vi "LS Durability Main (RT).vi"() -> ()   [LabVIEW 2018]
uses:
  Type Defs/App Config.ctl
  Type Defs/Controller Names.ctl
  SubVIs/Data Logger/Data Log Init.ctl
  Controls/Alarm Config.ctl
  Controls/Alarm Definition.ctl
  Controls/Alarm Profile Config.ctl
  Type Defs/Controller List.ctl
  Controls/Tank CMDs.ctl
  Controls/Controller Config.ctl
  Controls/Pump Data.ctl
  Controls/Tank Data.ctl
  Controls/HMI Cluster.ctl
  Controls/HMI Header.ctl
  Controls/HMI Tog Buttons.ctl
  Controls/HMI Mom Buttons.ctl
  Type Defs/LS Data.ctl
  Type Defs/Sequence States.ctl
  Controls/App Global Mode.ctl
  Controls/RPi HMI Mode.ctl
  Controls/Email Mode.ctl
  Type Defs/Pump Data Mode.ctl
  SubVIs/Watlow Modbus/Modbus Mode.ctl
  SubVIs/Watlow Modbus/Modbus Variable.ctl
  Controls/HMI Global Mode.ctl
  <vilib>/FPGAPlugInAG/sbRIO-9627/niLvFpga_Open_sbRIO-9627.vi
  <vilib>/Utility/error.llb/Error Cluster From Error Code.vi
  <vilib>/rvi/errors/niLvFpgaAdjustHostInterfaceError.vi
  <vilib>/Utility/file.llb/Write To Spreadsheet File (string).vi
  <vilib>/rvi/interface/nirviOpenFPGA/nirviOpenFPGA.xnode
  Controls/FPGA_Reference.ctl
  FPGA Bitfiles/LS_Durability_FPGA_9627.lvbitx
  <vilib>/rvi/interface/nirviReadWriteControl/nirviReadWriteControl.xnode
  <vilib>/Utility/config.llb/NI_LVConfig.lvlib
  Controls/Power Supply Global Mode.ctl
  SubVIs/Data Logger/Data Logger Mode.ctl
  SubVIs/Data Logger/Data Log Start.ctl
  NiFpgaLv.dll
  <vilib>/rvi/errors/niLvFpgaMergeErrorWithErrorCode.vi
panel:
  in  "pb.Run Profile":bool
  in  "Bank 2":T1={"7"=TRUE, "8"=TRUE, "9"=TRUE, "10"=TRUE, "11"=TRUE, "11 2"=TRUE}
  in  "Bank 1":T2={"1"=TRUE, "2"=TRUE, "3"=TRUE, "4"=TRUE, "5"=TRUE, "5 2"=TRUE} caption="Present"
  out "Email Alarms Disabled":bool
  out "Recording":bool
  in  "Disable Alarm Email":bool
  in  "Temp Tolerance":dbl=3.0 min=0.0 max=999999.0 step=1.0
  in  "Thermocouple":enum16{"2 TC/2 Tanks", "1 TC/1 Tank"}(ring)
  out "ADC Errors":i32
  in  "pb.Tare Pressure":bool
  in  "Data Log Enabled":bool=TRUE
  in  "RPMhyst":fxp<+,25,6>=1.0
  in  "pb.FuelChange":bool
  in  "Controller Type:":T3
  in  "Target Pressure:":dbl
  in  "Target Voltage:":dbl
  in  "Tank 1 Fuel Type:":string
  in  "Tank 2 Fuel Type:":string
  in  "Stagger Time (ms):":i32
  out "Cycles Completed:":u32=17
  in  "pb.Cycle Reset":bool
  in  "Serial Numbers":T4
  out "Read Inputs (ms)":u32
  out "Update Screen (ms)":u32
  out "Run Step (ms)":u32
  in  "Fuel Change Tab":enum32{"Page 1", "Page 2"}(tab)
  in  "pb.Fuel Change OK":bool
  in  "Reset Tab":enum32{"Page 1", "Page 2"}(tab)
  in  "pb.Reset OK":bool
  in  "pb.Reset Cancel":bool
  in  "Save As Tab":enum32{"Page 1", "Page 2"}(tab)
  in  "New Profile Name:":string
  in  "pb.Save As OK":bool
  in  "pb.Save As Cancel":bool
  in  "Alarm Tab":enum32{"Page 1", "Page 2"}(tab)
  out "Alarm Message":string
  in  "pb.Alarm OK":bool
  in  "Set Time Tab":enum32{"Page 1", "Page 2"}(tab)
  in  "pb.Set Time OK":bool
  in  "pb.Set Time Cancel":bool
  in  "New Time":dbl format="%<%H:%M:%S>t"
  in  "Pump Timers Tab":enum32{"Page 1", "Page 2"}(tab)=enum."Page 2"
  in  "Stop Time Enable":bool
  in  "Stop Time:":dbl format="%<%H:%M:%S>t"
  in  "pb.Time Reset All":bool
  out "Elapsed Time:":dbl[](array[numeric]) format="%<%H:%M:%S>t"
  in  "pb.Resets":bool[](array[boolean])=[FALSE, FALSE, FALSE, FALSE, FALSE, FALSE]
  in  "pb.Sets":bool[](array[boolean])=[FALSE, FALSE, FALSE, FALSE, FALSE, FALSE]
  in  "LS Serial Numbers":T5 caption="Serial Numbers"
  out "CPU Usage:":dbl=7.74131899555212 format="%.1f"
  in  "Live Data Tab":enum32{"Page 1", "Page 2", "Page 3"}(tab)=enum."Page 2"
  in  "Controller\nCMD":dbl[](array[numeric])=[0.0, 0.0, 0.0, 0.0, 0.0, 0.0] format="%#.2f"
  out "Speed":dbl[](array[numeric]) caption="Speed\n(RPM)" format="%#.0f"
  out "ControllerCurrent":dbl[](array[numeric])=[0.015201568603515625, 0.00335693359375, 0.003021240234375, 0.12260055541992188, 0.06085968017578125, 0.052234649658203125] caption="Controller\nCurrent\n(DC)" format="%.1f"
  out "PumpCurrent":dbl[](array[numeric])=[0.015201568603515625, 0.00335693359375, 0.003021240234375, 0.12260055541992188, 0.06085968017578125, 0.052234649658203125] caption="Pump\nCurrent\n(RMS)" format="%.1f"
  out "Flow":dbl[](array[numeric])=[0.0, 0.0, 0.0, 0.125, 0.0625, 0.0625] caption="Flow\n(L/H)" format="%#.0f"
  out "Pressure":dbl[](array[numeric])=[0.015201568603515625, 0.00335693359375, 0.003021240234375, 0.12260055541992188, 0.06085968017578125, 0.052234649658203125] caption="Pressure\n(kPa)" format="%#.0f"
  out "Ave. Speed":dbl=7.74131899555212 format="%.1f"
  out "Voltages":dbl[](array[numeric])=[0.015201568603515625, 0.00335693359375, 0.003021240234375, 0.12260055541992188, 0.06085968017578125, 0.052234649658203125] caption="Pump\nVoltage\n(V)" format="%.1f"
  in  "Reset Anomalies":bool
  in  "Reset Total Cycles":bool
  out "Anomalies (Last Cycle)":i32[](array[numeric]) caption="Anomalies\n(Last Cycle)" format="%#.0f"
  out "Anomalies/Cycle":i32[](array[numeric]) caption="Anomalies/\nCycle" format="%#.0f"
  out "Cycles":u32[](array[numeric]) caption="Powered\nCycles" format="%#.0f"
  out "Anomalies Total":i32[](array[numeric]) caption="Anomalies\nTotal" format="%#.0f"
  out "Steps":u32[](array[numeric]) format="%#.0f"
  out "Total Cycles":u32[](array[numeric]) caption="Total\nPowered\nCycles" format="%#.0f"
  in  "Reset Opens":bool
  out "Opens":i32[](array[numeric]) format="%#.0f"
  in  "App Config":T6={"Location"="Tanks 162-163", "Profiles Path"=path "c:/Profiles", "Current Profile"="", "CA Number"="", "Cycles Completed"=0, "Controller Type:"=enum."Kuhnke", "Stagger Time (ms)"=0, "Tank 1 Fuel"="", "Tank 2 Fuel"="", "Serial Numbers"={"Position 1 SN"="", "Position 2 SN"="", "Poaition 3 SN"="", "Position 4 SN"="", "Position 5 SN"="", "Position 6 SN"=""}, "Pumps Present"={"Pump 1"=FALSE, "Pump 2"=FALSE, "Pump 3"=FALSE, "Pump 4"=FALSE, "Pump 5"=FALSE, "Pump 6"=FALSE}, "VoltCtrlRef"="", "VoltageSelect"=FALSE, "Watlow Present"=TRUE, "Temp 1"=0.0, "Temp 2"=0.0, "V_Run PI?"=FALSE, "Voltage Limits"={"V_Step"=1e-05, "V_CmdMax"=0.0, "V_CmdMin"=0.0}, "Voltage Far PI"={"V_FarSlew"=10.0, "V_FarKp"=0.0, "V_FarKi"=0.0}, "Voltage Mid PI"={"V_MidSlew"=10.0, "V_MidKp"=0.0, "V_MidKi"=0.0}, "Voltage Close PI"={"V_CloseSlew"=10.0, "V_CloseKp"=0.0, "V_CloseKi"=0.0}, "Voltage Scale"={"V_FFm"=0.0, "V_FFb"=0.0}, "Voltage Cutoffs"={"V_MidCutoff"=0.0, "V_CloseCutoff"=0.0}, "Pressure Scale"={"Pres_FFm"=1e-05, "Pres_FFb"=0.0}, "Temp Format"=0, "Temp Tolerance"=0.0, "Target Voltage"=0.0, "Target Pressure"=0.0, "Data Log Init"={"Data Path"=path "u:/Data", "Data Log Rate (S/s)"=1, "AKLH Rate (Hours/S)"=0.1, "Sync Time Offset (min)"=180, "IP Last 3"=0, "WebDAV IP"="10.31.176.36"}, "Email Handler IP"="10.30.189.34", "ADC Check"=FALSE, "3 Pump Tank"=TRUE, "Cycle Threshold:"=3.0, "Cycle Pts to Avg:"=3, "Anomaly Threshold:"=3.0, "Normal Steps:"=3, "Step Threshold:"=3.0, "Network Drive IP"="", "Network Drive Password"="", "Bank 1 Offset"=0.0, "Bank 2 Offset"=0.0} {"Bank 2 Offset" min=0.0 max=999999.0 step=1.0; "Bank 1 Offset" min=0.0 max=999999.0 step=1.0; "Step Threshold:" min=0.0 max=999999.0 step=1.0; "Normal Steps:" max=999999 step=1; "Anomaly Threshold:" min=0.0 max=999999.0 step=1.0; "Cycle Pts to Avg:" max=999999 step=1; "Cycle Threshold:" min=0.0 max=999999.0 step=1.0}
  in  "Monitoring Tab":enum32{"Page 1", "Page 2"}(tab)
  out "Avg Press:":dbl=7.74131899555212
  in  "pb.E Stop":bool
  in  "Ignition Relay":T8
  in  "Power Relay":T8
  out "Temp2":dbl caption="Tank 2 Temp (C):" format="%.1f"
  out "Temp1":dbl caption="Tank 1 Temp (C):" format="%.1f"
  out "PS Actual (V):":dbl format="%.2f"
  in  "Power Supply Cmd:":dbl min=0.0 max=20.0 format="%#.2f"
  in  "PressureCMD":dbl caption="Pressure Cmd:" min=0.0 max=825.0 format="%#.2f"
  in  "Pumps Present":T8={"Pump 1"=TRUE, "Pump 2"=TRUE, "Pump 3"=TRUE, "Pump 4"=TRUE, "Pump 5"=TRUE, "Pump 6"=TRUE}
  in  "Tank 1 Temp Cmd:":dbl caption="deg C"
  in  "Tank 2 Temp Cmd:":dbl caption="deg C"
  in  "Title Tab":enum32{"Page 1", "Page 2"}(tab)
  out "Title":string="LS-12 Durability Tester, v2.0"
  out "Time/Date":string
  in  "Login":bool
  in  "pb.Stop Profile":bool
  in  "Main Tab":T9(tab)
  out "ARclock":i32 caption="Auto-resume\nClock"
  in  "ARtiming":i32=1800 caption="Auto-resume\nTime (s)"
  in  "pb.Pause/Resume":bool
  out "Transferring":bool
  in  "Recording\nFrequency (Hz): 2":i32=1000
  in  "Recording\nDuration (s): 2":i32=3600
  in  "Record Constant":bool
  in  "Detection Mode:":u16(ring) items=["Anomalies", "Opens"]
  in  "Record During Profile":bool
  in  "Recording\nFrequency (Hz):":i32=1000
  in  "Recording\nDuration (s):":i32=10
  in  "Interval Between\nRecordings (s):":i32=600
  in  "LS Cycle Time (ms):":dbl=244.0 min=0.1 max=1000.0 step=0.1
  in  "LS On Time (ms):":dbl=4.0 min=0.0 max=1000.0 step=0.01
  in  "Bank 2 Power State:":u16(ring) items=["0 - Off", "1 - On", "2 - Pulsing"]
  in  "Bank 1 Power State:":u16(ring) items=["0 - Off", "1 - On", "2 - Pulsing"]
  in  "CA Number:":string
  in  "Profile Name:":string(combo)="test"
  in  "pb.Save As":bool
  out "Location:":string
  in  "Profile:":string[][](table)=[["1", "216000", "1", "2", "244", "4", "1", "67.6"], ["2", "1800", "0", "0", "244", "4", "1", "10.0"], ["3", "39600", "0", "0", "244", "4", "0", ""], ["4", "1800", "0", "0", "244", "4", "1", ""]]
  out "Recording":bool
  in  "Data File Name:":string
  out "Step:":i32=2
  out "Time Left:":dbl=0.21101045608520508
  out "Waveform Chart":dbl(graph)
  in  "Pause":bool
  in  "Position":i32=1 min=1 max=13 step=1
  in  "Bank 2 Voltage Offset:":dbl
  in  "Bank 1 Voltage Offset:":dbl
  in  "Voltage(T)/Resistance(F)":bool=TRUE
  in  "Bias Resistances":dbl[](array[numeric])=[681.0, 681.0, 681.0, 681.0, 681.0, 681.0, 681.0, 681.0, 681.0, 681.0, 681.0, 681.0] caption="Total\nCycles"
  in  "Anomaly Threshold:":dbl=3.0 min=0.0 max=999999.0 step=1.0
  in  "Normal Steps:":u32=3 max=999999 step=1
  in  "Step Threshold:":dbl=3.0 min=0.0 max=999999.0 step=1.0
  in  "Cycle Pts to Avg:":i32=20 min=0 max=999999 step=1
  in  "Cycle Threshold:":dbl=1.6 min=0.0 max=999999.0 step=1.0
  in  "Note Tab":enum32{"Page 1", "Page 2"}(tab)
  in  "Stop Profile Note":string
  in  "pb.Note OK":bool
  in  "pb.Note Cancel":bool
  in  "Alarm Config":T10
  in  "WebDAV Push":bool
  in  "Concat Data":bool
  in  "Cutoffs":cluster{"Mid Range":dbl, "Close Range":dbl} {"Close Range" min=-100000.0 max=100000.0 step=1e-05 format="%#.5f"; "Mid Range" min=-100000.0 max=100000.0 step=1e-05 format="%#.5f"}
  in  "Mid PI":cluster{"Slew Rate":dbl, "Kp":dbl, "Ki":dbl}={"Slew Rate"=10.0, "Kp"=0.0, "Ki"=0.0} {"Ki" min=-100000.0 max=100000.0 step=1e-05 format="%#.5f"; "Kp" min=-100000.0 max=100000.0 step=1e-05 format="%#.5f"; "Slew Rate" min=0.0 max=1000000.0 step=0.01 format="%#.5f"}
  in  "Close PI":cluster{"Slew Rate":dbl, "Kp":dbl, "Ki":dbl}={"Slew Rate"=10.0, "Kp"=0.0, "Ki"=0.0} {"Ki" min=-100000.0 max=100000.0 step=1e-05 format="%#.5f"; "Kp" min=-100000.0 max=100000.0 step=1e-05 format="%#.5f"; "Slew Rate" min=0.0 max=1000000.0 step=0.01 format="%#.5f"}
  in  "Pressure Scale":cluster{"M":dbl, "B":dbl}={"M"=1e-05, "B"=0.0} {"B" min=-100000.0 max=100000.0 step=1e-05 format="%#.5f"; "M" min=-100000.0 max=100000.0 step=1e-05 format="%#.5f"}
  in  "Closed Loop Voltage":bool
  in  "Voltage Limits":cluster{"Step":dbl, "Max":dbl, "Min":dbl}={"Step"=1e-05, "Max"=0.0, "Min"=0.0} {"Min" min=0.0 max=10.0 step=1e-05 format="%#.5f"; "Max" min=0.0 max=10.0 step=1e-05 format="%#.5f"; "Step" min=0.0 max=100.0 step=1e-05 format="%#.5f"}
  in  "Far PI":cluster{"Slew Rate":dbl, "Kp":dbl, "Ki":dbl}={"Slew Rate"=10.0, "Kp"=0.0, "Ki"=0.0} {"Ki" min=-100000.0 max=100000.0 step=1e-05 format="%#.5f"; "Kp" min=-100000.0 max=100000.0 step=1e-05 format="%#.5f"; "Slew Rate" min=0.0 max=1000000.0 step=0.01 format="%#.5f"}
  in  "Voltage Scale":cluster{"M":dbl, "B":dbl} {"B" min=-100000.0 max=100000.0 step=1e-05 format="%#.5f"; "M" min=-100000.0 max=100000.0 step=1e-05 format="%#.5f"}
  # "Fuel Change was logged."
  # "Are you sure you want to reset?"
  # "Enter a new elapsed time."
  # "Pump Timers"
  # "Live Data"
  # "Level Sensor Monitor"
  # "Level Sensor Monitor"
  # "Manual Control"
  # "V"
  # "kPa"
  # "degC"
  # "degC"
  # "Data file note as to reason for stopping profile:"
  # "Voltage Control"
  # "Pressure Control"
  # "Data Server"
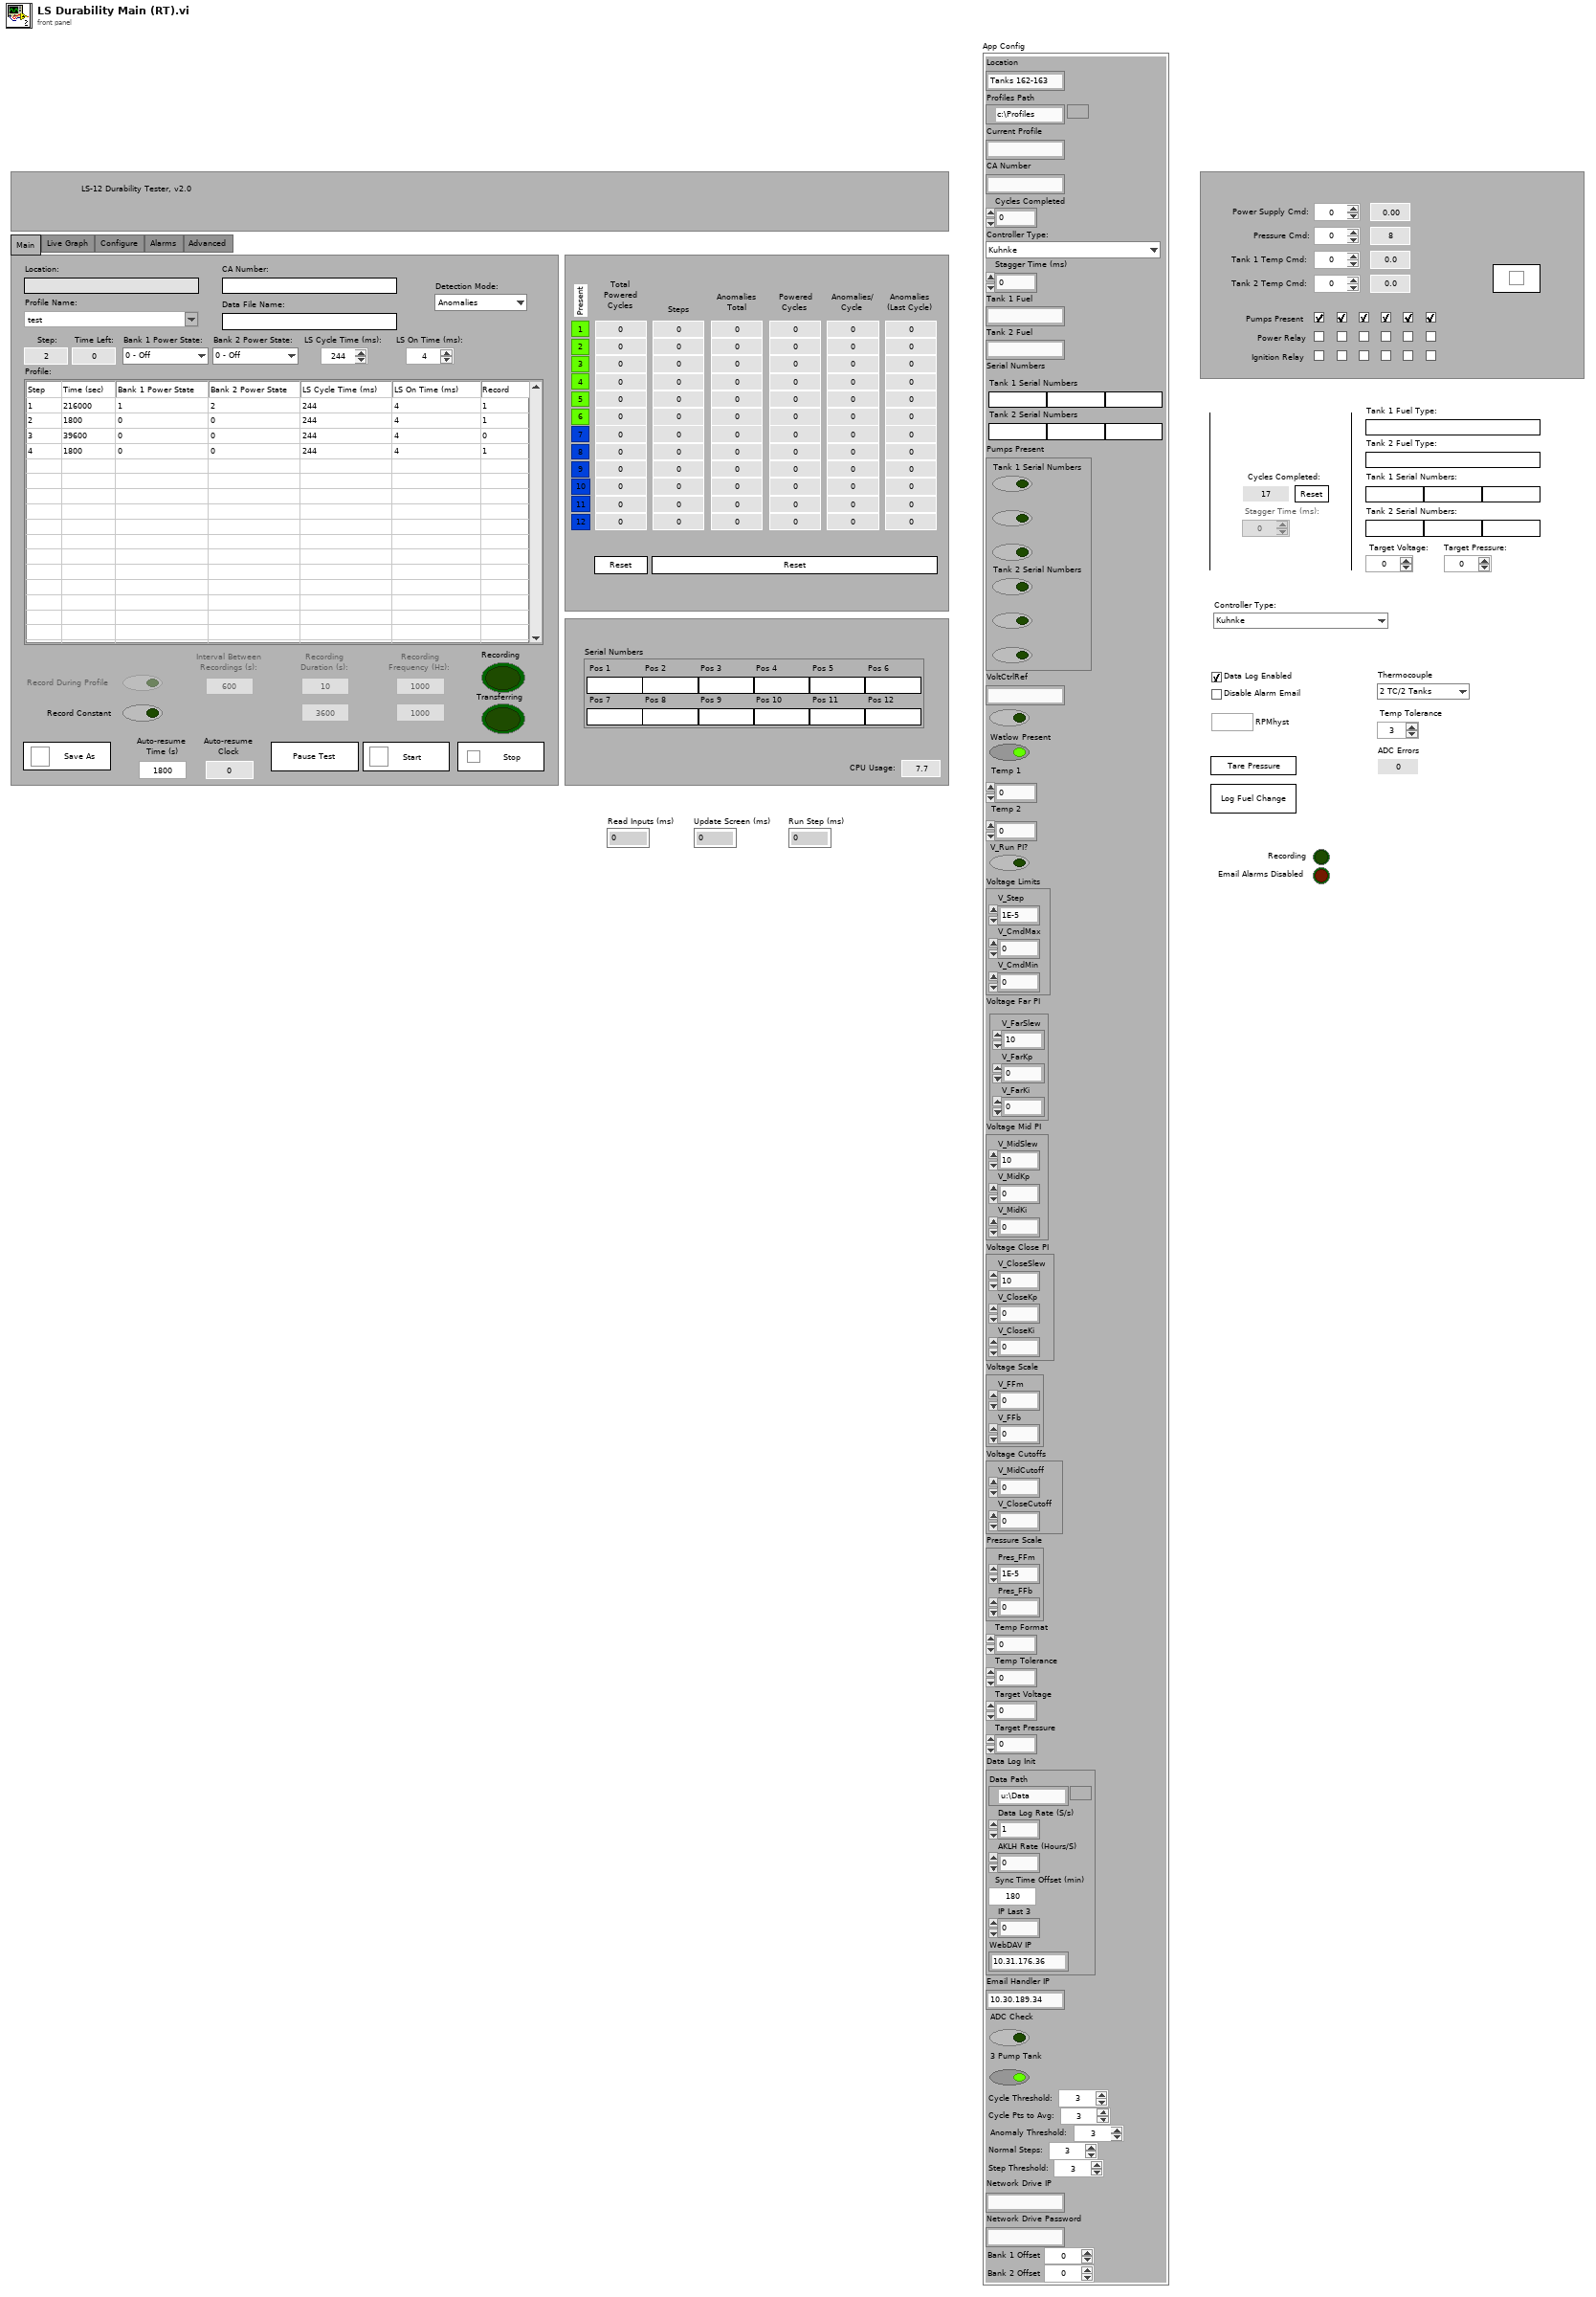
[diagram p1: front panel]
types:
  T1 = cluster{"7":bool, "8":bool, "9":bool, "10":bool, "11":bool, "11 2":bool}
  T2 = cluster{"1":bool, "2":bool, "3":bool, "4":bool, "5":bool, "5 2":bool}
  T3 = typedef "Controller Names.ctl" = enum16{"Kuhnke", "Helbako BLDC", "Conti", "Hella BLDC OL PWM", "Hella BLDC Turbine OL PWM", "Hella BLDC Pressure", "Helbako (old)", "TI PWM", "PSA", "Hella Gas", "Hella Diesel", "8 Comm", "10 Comm", "8 Comm Hella", "10 Comm Hella", "8 Comm Omron", "10 Comm Omron", "8 Comm Nissan", "10 Comm Nissan"}
  T4 = cluster{"Position 1 SN":string, "Position 2 SN":string, "Position 3 SN":string, "Position 4 SN":string, "Position 5 SN":string, "Position 6 SN":string}
  T5 = cluster{"Pos 1":string, "Pos 2":string, "Pos 3":string, "Pos 4":string, "Pos 5":string, "Pos 6":string, "Pos 7":string, "Pos 8":string, "Pos 9":string, "Pos 10":string, "Pos 11":string, "Pos 12":string}
  T6 = typedef "App Config.ctl" = cluster{"Location":string, "Profiles Path":path, "Current Profile":string, "CA Number":string, "Cycles Completed":u32, "Controller Type:":T3, "Stagger Time (ms)":i32, "Tank 1 Fuel":string, "Tank 2 Fuel":string, "Serial Numbers":cluster{"Position 1 SN":string, "Position 2 SN":string, "Poaition 3 SN":string, "Position 4 SN":string, "Position 5 SN":string, "Position 6 SN":string}, "Pumps Present":cluster{"Pump 1":bool, "Pump 2":bool, "Pump 3":bool, "Pump 4":bool, "Pump 5":bool, "Pump 6":bool}, "VoltCtrlRef":string, "VoltageSelect":bool, "Watlow Present":bool, "Temp 1":dbl, "Temp 2":dbl, "V_Run PI?":bool, "Voltage Limits":cluster{"V_Step":dbl, "V_CmdMax":dbl, "V_CmdMin":dbl}, "Voltage Far PI":cluster{"V_FarSlew":dbl, "V_FarKp":dbl, "V_FarKi":dbl}, "Voltage Mid PI":cluster{"V_MidSlew":dbl, "V_MidKp":dbl, "V_MidKi":dbl}, "Voltage Close PI":cluster{"V_CloseSlew":dbl, "V_CloseKp":dbl, "V_CloseKi":dbl}, "Voltage Scale":cluster{"V_FFm":dbl, "V_FFb":dbl}, "Voltage Cutoffs":cluster{"V_MidCutoff":dbl, "V_CloseCutoff":dbl}, "Pressure Scale":cluster{"Pres_FFm":dbl, "Pres_FFb":dbl}, "Temp Format":i32, "Temp Tolerance":dbl, "Target Voltage":dbl, "Target Pressure":dbl, "Data Log Init":T7, "Email Handler IP":string, "ADC Check":bool, "3 Pump Tank":bool, "Cycle Threshold:":dbl, "Cycle Pts to Avg:":i32, "Anomaly Threshold:":dbl, "Normal Steps:":u32, "Step Threshold:":dbl, "Network Drive IP":string, "Network Drive Password":string, "Bank 1 Offset":dbl, "Bank 2 Offset":dbl}
  T7 = typedef "Data Log Init.ctl" = cluster{"Data Path":path, "Data Log Rate (S/s)":u32, "AKLH Rate (Hours/S)":dbl, "Sync Time Offset (min)":i32, "IP Last 3":i32, "WebDAV IP":string}
  T8 = cluster{"Pump 1":bool, "Pump 2":bool, "Pump 3":bool, "Pump 4":bool, "Pump 5":bool, "Pump 6":bool}
  T9 = enum32{"Main", "Live Graph", "Configure", "Alarms", "Advanced"}
  T10 = typedef "Alarm Config.ctl" = cluster{"Alarms:":T11[], "Profile Sync:":T12}
  T11 = typedef "Alarm Definition.ctl" = cluster{"Description:":string, "Enabled:":bool, "Data Index:":i32, "Data Type:":string, "Low Limit:":dbl, "High Limit:":dbl, "Trip Time:":u32, "Profile Sync:":bool}
  T12 = typedef "Alarm Profile Config.ctl" = cluster{"Trip Time:":u32, "Consecutive Trips:":i32}
  T13 = cluster{"LS Power (Freq):":dbl, "LS Power (Duty):":dbl, "Bank 1 Present":cluster{"1":bool, "2":bool, "3":bool, "4":bool, "5":bool, "5 2":bool}, "Bank 2 Present":cluster{"7":bool, "8":bool, "9":bool, "10":bool, "11":bool, "11 2":bool}, "Data File Name:":string, "Record Bursts":bool, "RecInterval(s)":i32, "RecDuration(s)":i32, "RecFrequeny (Hz)":i32, "DetectionMode":i32, "Serial Numbers":string[], "Record Constant":bool, "2nd Step Check":bool, "Bias Resistances":dbl[], "Voltage(T)/Resistance(F)":bool}
  T14 = typedef "Sequence States.ctl" = enum16{"Main", "Init Files", "Init", "Unused", "Save As", "Start Profile", "Check Step Time", "Alarm", "Alarm Dismiss", "Run Step", "Stop Profile", "Cycle Reset", "Time Reset", "Time Reset All", "Time Set", "Tare CTs", "Save Profile", "Open Profile", "Get Profiles", "Update Screen", "Update Controls", "Save App Config", "Write Outputs", "Disable Background", "Enable Background", "Get/Release Control", "Log Fuel Change", "Fuel Change Popup", "Read Inputs", "Remote Timer Reset", "Controller Change", "Get Alarms", "Init Alarms", "Save Alarms", "Voltage Selection", "Set Watlow Temp 1", "Set Watlow Temp 2", "Get Pressure", "Write Tare Pressure", "Adjust Controls", "Reinit ADC", "Write Initial Times", "Write Pumps Present", "HMI Command", "Save Pump Times", "Check Pump Stop Time", "Save LS App Config", "Init Data File", "Reset LS Cycles", "Reset Anomalies", "Reset Opens", "Save LS Data", "Save LS Test Data", "Check Serial Numbers", "Main Tab", "Allow Data Note", "Resume Profile", "Pause Profile", "Allow Pause Note", "Clear Graph"}
  T15 = typedef "LS Data.ctl" = cluster{"Total Cycles":u32[], "Steps":u32[], "Anomalies Total":i32[], "Cycles":u32[], "Anomalies/Cycle":i32[], "Anomalies (Last Cycle)":i32[], "Opens":i32[]}
  T16 = typedef "HMI Cluster.ctl" = cluster{"Error":errorcluster, "COM Ref":refnum<visa-resource-name>, "Pump Data":T17, "Tank Data":cluster{"PS Actual (V):":dbl, "Temp1":dbl, "Temp2":dbl}, "Power Relays":cluster{"Pump 1":bool, "Pump 2":bool, "Pump 3":bool, "Pump 4":bool, "Pump 5":bool, "Pump 6":bool}, "Pump CMDs":dbl[], "HMI Header":T18, "Tank CMDs":T19, "HMI Tog Buttons":T20, "In Test":bool, "HMI Command":bool, "HMI Mom Buttons":T21, "Controller Config":T22, "Alarm":bool, "Alarm Message 1":string, "Alarm Message 2":string, "Recording":bool, "Serial Numbers":string[], "Pumps Present":bool[]}
  T17 = typedef "Pump Data.ctl" = cluster{"Voltages":dbl[], "PumpCurrent":dbl[], "Speed":dbl[], "ControllerCurrent":dbl[], "Pressure":dbl[], "Flow":dbl[], "Elapsed Time (Display)":dbl[], "Avg Pressure":dbl, "Avg Speed":dbl, "Elapsed Time":dbl[]}
  T18 = typedef "HMI Header.ctl" = cluster{"Line 1":string, "Line 2":string, "Line 3":string, "Line 4":string}
  T19 = typedef "Tank CMDs.ctl" = cluster{"PS CMD":dbl, "Press CMD":dbl, "Temp 1 CMD":dbl, "Temp 2 CMD":dbl}
  T20 = typedef "HMI Tog Buttons.ctl" = cluster{"Start Test":bool, "Toggle Spare 1":bool, "Toggle Spare 2":bool, "Toggle Spare 3":bool, "Toggle Spare 4":bool, "Toggle Spare 5":bool}
  T21 = typedef "HMI Mom Buttons.ctl" = cluster{"Stop":bool, "Reset Timers":bool, "Log Fuel Change":bool, "Alarm Dismiss":bool}
  T22 = typedef "Controller Config.ctl" = cluster{"Controller Name":T3, "CommSeg":i32, "PWM?":bool, "Frequency":i32, "Low Command":dbl, "High Command":dbl, "Stop Command":dbl, "Command Step":dbl, "Solenoid Stop?":bool, "Controller?":bool, "Invert PWM":bool}
  T23 = typedef "Tank Data.ctl" = cluster{"PS Actual (V):":dbl, "Temp1":dbl, "Temp2":dbl}
  T24 = typedef "Controller List.ctl" = cluster{"Controller Name":T3, "CommSeg":i32, "PWM?":bool, "Frequency":i32, "Low Command":dbl, "High Command":dbl, "Stop Command":dbl, "Command Step":dbl, "Solenoid Stop?":bool, "Controller?":bool, "Invert PWM":bool}[]
  T25 = cluster{"Error":errorcluster, "Profile":string[][], "App Config":T6, "Profiles":string[], "Current Step":i32, "Step Time Left":dbl, "Run Profile":bool, "Step Start Time":dbl, "Step Time":dbl, " # of Steps":i32, "Screen Timer":u32, "Last Profile Time":dbl, "Controller CMDs":dbl[], "Client?":bool, "pb.Run Profile":bool, "pb.Resets":bool[], "pb.Sets":bool[], "Initial Times":dbl[], "Pressure Offsets":dbl[], "Login":bool, "Stagger Counter":i32, "New Step":bool, "Inputs Timer":u32, "Tank Data":T23, "Voltage Enable":bool, "Power Relay":cluster{"Pump 1":bool, "Pump 2":bool, "Pump 3":bool, "Pump 4":bool, "Pump 5":bool, "Pump 6":bool}, "Ignition Relay":cluster{"Pump 1":bool, "Pump 2":bool, "Pump 3":bool, "Pump 4":bool, "Pump 5":bool, "Pump 6":bool}, "Controller List":T24, "Alarm Config":T10, "Alarm Config Path":path, "Trip Counters":i32[], "Previous Times":u32[], "Alarm Message 1":string, "Alarm Message 2":string, "Prev ON Times":u32[], "CalArray":dbl[][], "Tank CMDs":T19, "Controller Config":T22, "Fuel Log Path":path, "Pump Data":T17, "Alarm Latch":bool, "Time/Date":string, "Recording":bool, "HMI":T16, "WebDAV Push":bool, "Email Alarms Disabled":bool, "Concat Data":bool, "LS Data":T15, "Main Tab":enum32{"Main", "Live Graph", "Configure", "Alarms", "Advanced"}, "LS App Config":cluster{"LS Power (Freq):":dbl, "LS Power (Duty):":dbl, "Bank 1 Present":cluster{"1":bool, "2":bool, "3":bool, "4":bool, "5":bool, "5 2":bool}, "Bank 2 Present":cluster{"7":bool, "8":bool, "9":bool, "10":bool, "11":bool, "11 2":bool}, "Data File Name:":string, "Record Bursts":bool, "RecInterval(s)":i32, "RecDuration(s)":i32, "RecFrequeny (Hz)":i32, "DetectionMode":i32, "Serial Numbers":string[], "Record Constant":bool, "2nd Step Check":bool, "Bias Resistances":dbl[], "Voltage(T)/Resistance(F)":bool}, "Bank 1 State:":u16, "Bank 2 State:":u16, "LS Data Filepath":path, "Initial LS Data":T15, "day of month":i32, "Pause Test":bool, "ProfileMinute":i32, "ARtime":dbl, "ARactive":bool}
  T26 = typedef "FPGA_Reference.ctl" = refnum<k20>
  T27 = typedef "App Global Mode.ctl" = enum16{"Read", "Write Client", "Write Login"}
  T28 = enum16{"Read", "Engine Writes", "Main Writes", "Write Anomalies", "Write Init Data"}
  T29 = typedef "Data Logger Mode.ctl" = enum16{"Init", "Main", "Start", "Stop"}
  T30 = cluster{"Running?":bool, "Profile Record":bool, "RecordInterval":i32, "RecordDuration":i32, "RecordFreq":i32, "Data Filepath":path, "Hr Record":bool, "Serial Numbers":string[]}
  T31 = enum8{"Enabled", "Disabled", "Disabled and Grayed Out"}
  T32 = enum16{"open", "replace", "create", "open or create", "replace or create", "replace or create with confirmation"}
  T33 = typedef "Data Log Start.ctl" = cluster{"App Config":T6, "Profile":string[][], "Controller Type":string, "Tank CMDs":T19}
  T34 = typedef "Power Supply Global Mode.ctl" = enum16{"Write Setpoint", "Write FreezePID", "Read"}
  T35 = typedef "RPi HMI Mode.ctl" = enum16{"Init", "Write Data", "Read from RPi", "Write to RPi"}
  T36 = typedef "Email Mode.ctl" = enum16{"Trigger Email", "Send Email"}
  T37 = typedef "Pump Data Mode.ctl" = enum16{"Read", "Write Data", "Write Cal", "Write Watlow Data", "Write Pressure Offsets", "Write Initial Times", "Write Pumps Present"}
  T38 = typedef "Modbus Variable.ctl" = enum16{"Temperature", "Setpoint"}
  T39 = typedef "Modbus Mode.ctl" = enum16{"Init", "Tank 1 Write", "Tank 2 Write", "Tank 1 Read", "Tank 2 Read"}
  T40 = typedef "HMI Global Mode.ctl" = enum16{"Read", "Write Cluster", "Reset Cmd"}
  T41 = cluster{"Position 1 SN":string, "Position 2 SN":string, "Poaition 3 SN":string, "Position 4 SN":string, "Position 5 SN":string, "Position 6 SN":string}
  T42 = cluster{"V_Step":dbl, "V_CmdMax":dbl, "V_CmdMin":dbl}
  T43 = cluster{"V_FarSlew":dbl, "V_FarKp":dbl, "V_FarKi":dbl}
  T44 = cluster{"V_MidSlew":dbl, "V_MidKp":dbl, "V_MidKi":dbl}
  T45 = cluster{"V_CloseSlew":dbl, "V_CloseKp":dbl, "V_CloseKi":dbl}
  T46 = typedef "LVDateTimeRec.ctl" = cluster{"fractional second":dbl, "second":i32, "minute":i32, "hour":i32, "day of month":i32, "month":i32, "year":i32, "day of week":i32, "day of year":i32, "DST":i32}
  T47 = typedef "NI_LVConfig.lvlib/Config Data RefNum.ctl" = refnum<k1>
  T48 = cluster{"LS Power (Freq):":dbl, "LS Power (Duty):":dbl, "Bank 1 Present":cluster{"1":bool, "2":bool, "3":bool, "4":bool, "5":bool, "6":bool}, "Bank 2 Present":cluster{"7":bool, "8":bool, "9":bool, "10":bool, "11":bool, "12":bool}, "Data File Name:":string, "Record Bursts":bool, "RecInterval(s)":i32, "RecDuration(s)":i32, "RecFrequeny (Hz)":i32, "DetectionMode":i32, "Serial Numbers":string[], "Record Constant":bool, "2nd Step Check":bool, "Bias Resistances":dbl[], "Voltage(T)/Resistance(F)":bool}
  T49 = cluster{"Serial Numbers[0]":string, "Serial Numbers[1]":string, "Serial Numbers[2]":string, "Serial Numbers[3]":string, "Serial Numbers[4]":string, "Serial Numbers[5]":string, "Serial Numbers[6]":string, "Serial Numbers[7]":string, "Serial Numbers[8]":string, "Serial Numbers[9]":string, "Serial Numbers[10]":string, "Serial Numbers[11]":string}
  T50 = cluster{"Controller Name":T3, "CommSeg":i32, "PWM?":bool, "Frequency":i32, "Low Command":dbl, "High Command":dbl, "Stop Command":dbl, "Command Step":dbl, "Solenoid Stop?":bool, "Controller?":bool, "Invert PWM":bool}
  T51 = cluster{"[0]":bool, "[1]":bool, "[2]":bool, "[3]":bool, "[4]":bool, "[5]":bool}
  T52 = cluster{"[0]":string, "[1]":string, "[2]":string, "[3]":string, "[4]":string, "[5]":string, "[6]":string, "[7]":string, "[8]":string, "[9]":string, "[10]":string, "[11]":string}
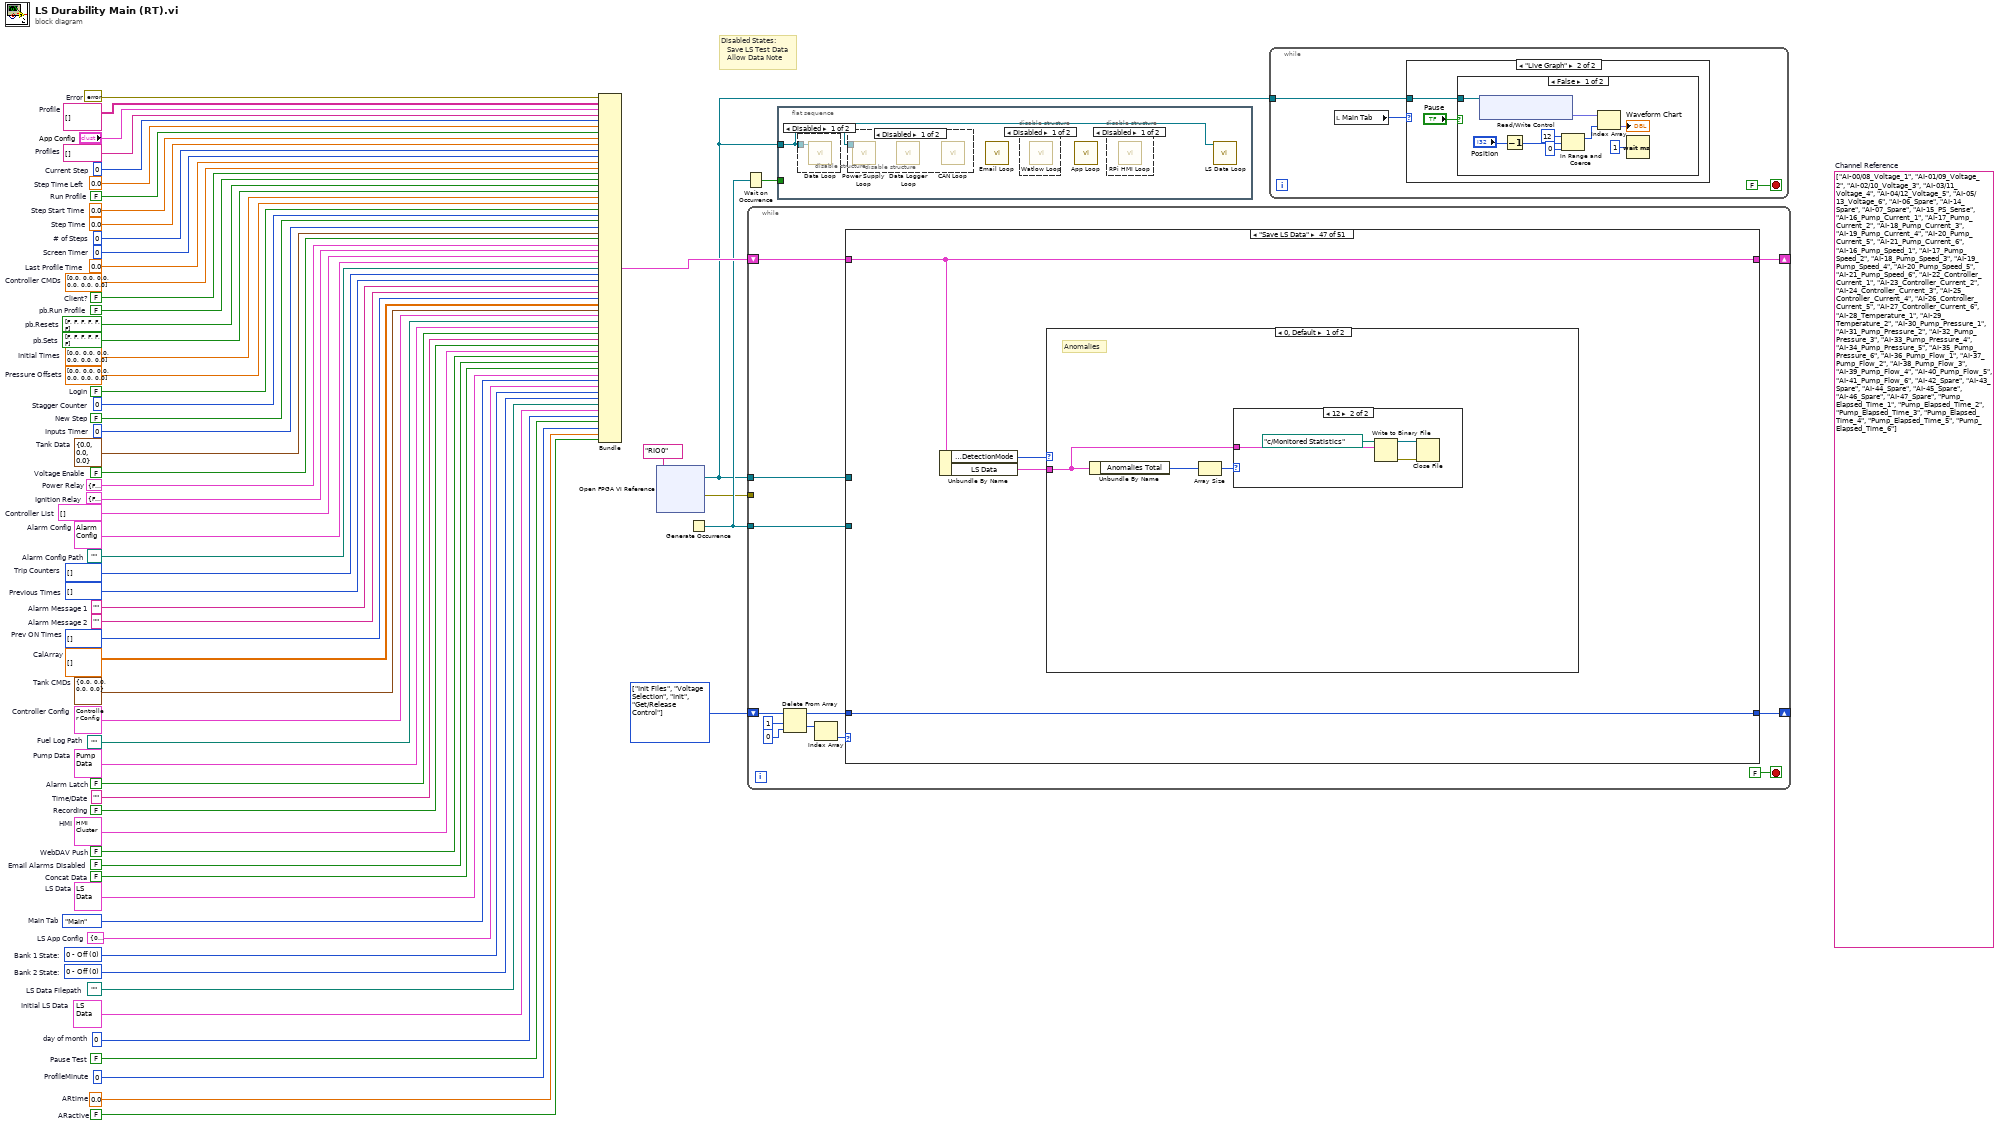
[diagram p0: block diagram]
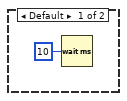
[diagram p2: hidden frame]
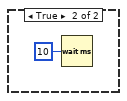
[diagram p3: hidden frame]
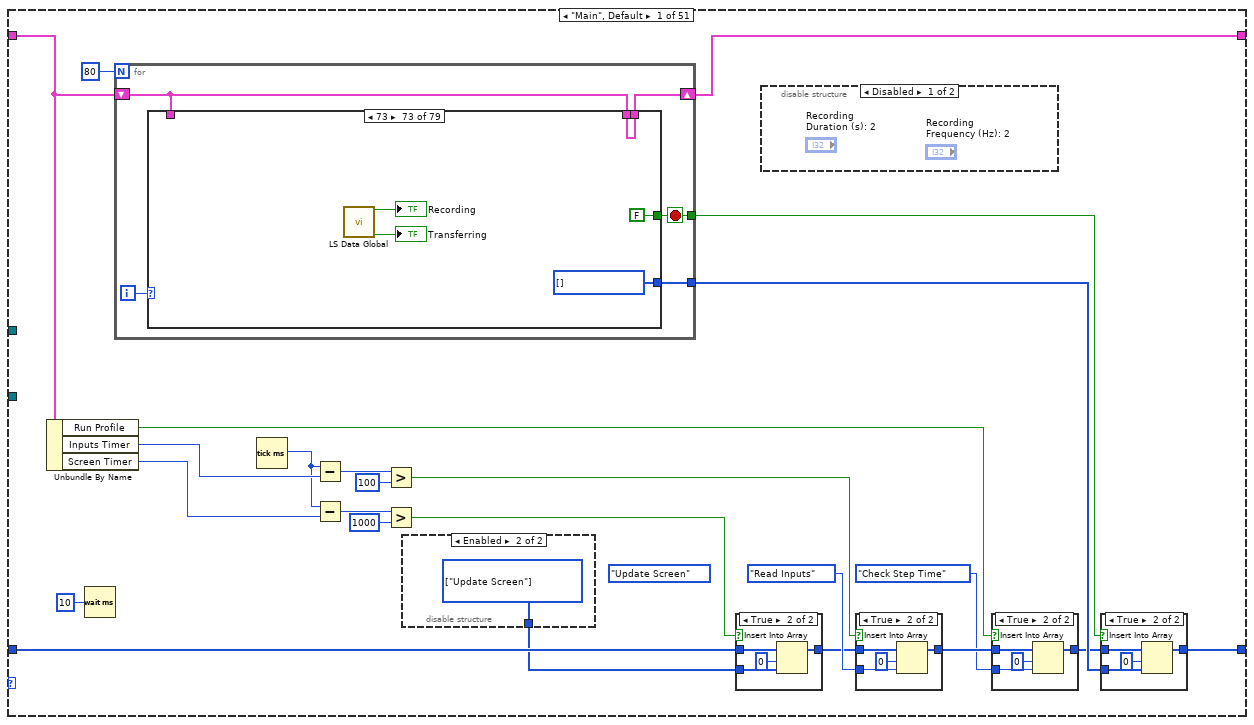
[diagram p8: hidden frame]
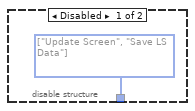
[diagram p9: hidden frame]
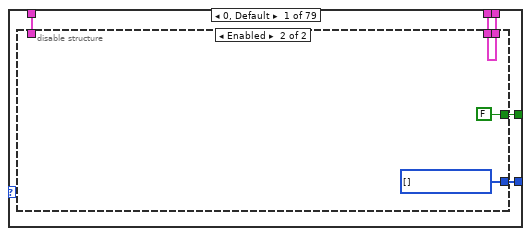
[diagram p15: hidden frame]
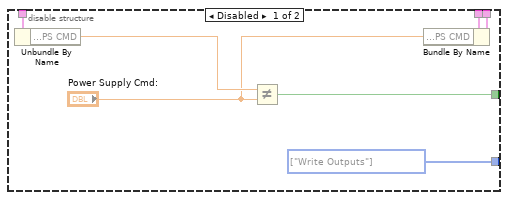
[diagram p16: hidden frame]
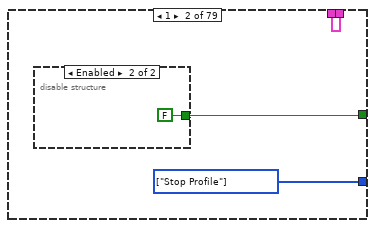
[diagram p17: hidden frame]
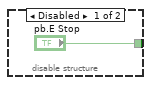
[diagram p18: hidden frame]
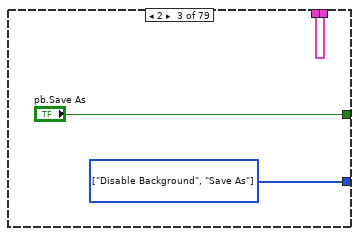
[diagram p19: hidden frame]
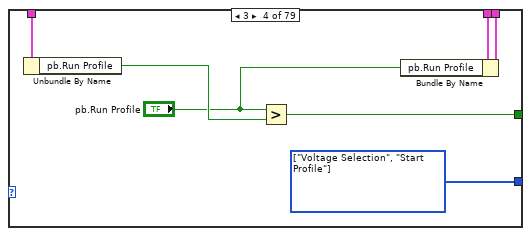
[diagram p20: hidden frame]
diagram:
  w5 = 0.0  # ARtime
  w4 = FALSE  # ARactive
  w6 = 0  # ProfileMinute
  w7 = FALSE  # Pause Test
  w8 = T13 {"LS Power (Freq):"=0.0, "LS Power (Duty):"=0.0, "Bank 1 Present"={"1"=TRUE, "2"=TRUE, "3"=TRUE, "4"=TRUE, "5"=TRUE, "5 2"=TRUE}, "Bank 2 Present"={"7"=TRUE, "8"=TRUE, "9"=TRUE, "10"=TRUE, "11"=TRUE, "11 2"=TRUE}, "Data File Name:"="", "Record Bursts"=FALSE, "RecInterval(s)"=600, "RecDuration(s)"=10, "RecFrequeny (Hz)"=1000, "DetectionMode"=0, "Serial Numbers"=["", "", "", "", "", "", "", "", "", "", "", " "], "Record Constant"=FALSE, "2nd Step Check"=FALSE, "Bias Resistances"=[681.0, 681.0, 681.0, 681.0, 681.0, 681.0, 681.0, 681.0, 681.0, 681.0, 681.0, 681.0], "Voltage(T)/Resistance(F)"=TRUE}  # LS App Config
  w9 = 0  # day of month
  (unwired) string[] ["AI-00/08_Voltage_1", "AI-01/09_Voltage_2", "AI-02/10_Voltage_3", "AI-03/11_Voltage_4", "AI-04/12_Voltage_5", "AI-05/13_Voltage_6", "AI-06_Spare", "AI-14_Spare", "AI-07_Spare", "AI-15_PS_Sense", "AI-16_Pump_Current_1", "AI-17_Pump_Current_2", "AI-18_Pump_Current_3", "AI-19_Pump_Current_4", "AI-20_Pump_Current_5", "AI-21_Pump_Current_6", "AI-16_Pump_Speed_1", "AI-17_Pump_Speed_2", "AI-18_Pump_Speed_3", "AI-19_Pump_Speed_4", "AI-20_Pump_Speed_5", "AI-21_Pump_Speed_6", "AI-22_Controller_Current_1", "AI-23_Controller_Current_2", "AI-24_Controller_Current_3", "AI-25_Controller_Current_4", "AI-26_Controller_Current_5", "AI-27_Controller_Current_6", "AI-28_Temperature_1", "AI-29_Temperature_2", "AI-30_Pump_Pressure_1", "AI-31_Pump_Pressure_2", "AI-32_Pump_Pressure_3", "AI-33_Pump_Pressure_4", "AI-34_Pump_Pressure_5", "AI-35_Pump_Pressure_6", "AI-36_Pump_Flow_1", "AI-37_Pump_Flow_2", "AI-38_Pump_Flow_3", "AI-39_Pump_Flow_4", "AI-40_Pump_Flow_5", "AI-41_Pump_Flow_6", "AI-42_Spare", "AI-43_Spare", "AI-44_Spare", "AI-45_Spare", "AI-46_Spare", "AI-47_Spare", "Pump_Elapsed_Time_1", "Pump_Elapsed_Time_2", "Pump_Elapsed_Time_3", "Pump_Elapsed_Time_4", "Pump_Elapsed_Time_5", "Pump_Elapsed_Time_6"]  # Channel Reference
  w12 = T14[] [enum."Init Files", enum."Voltage Selection", enum."Init", enum."Get/Release Control"] items=["Main", "Init Files", "Init", "Unused", "Save As", "Start Profile", "Check Step Time", "Alarm", "Alarm Dismiss", "Run Step", "Stop Profile", "Cycle Reset", "Time Reset", "Time Reset All", "Time Set", "Tare CTs", "Save Profile", "Open Profile", "Get Profiles", "Update Screen", "Update Controls", "Save App Config", "Write Outputs", "Disable Background", "Enable Background", "Get/Release Control", "Log Fuel Change", "Fuel Change Popup", "Read Inputs", "Remote Timer Reset", "Controller Change", "Get Alarms", "Init Alarms", "Save Alarms", "Voltage Selection", "Set Watlow Temp 1", "Set Watlow Temp 2", "Get Pressure", "Write Tare Pressure", "Adjust Controls", "Reinit ADC", "Write Initial Times", "Write Pumps Present", "HMI Command", "Save Pump Times", "Check Pump Stop Time", "Save LS App Config", "Init Data File", "Reset LS Cycles", "Reset Anomalies", "Reset Opens", "Save LS Data", "Save LS Test Data", "Check Serial Numbers", "Main Tab", "Allow Data Note", "Resume Profile", "Pause Profile", "Allow Pause Note", "Clear Graph"]
  w13 = T15 {"Total Cycles"=[0, 0, 0, 0, 0, 0, 0, 0, 0, 0, 0, 0], "Steps"=[0, 0, 0, 0, 0, 0, 0, 0, 0, 0, 0, 0], "Anomalies Total"=[0, 0, 0, 0, 0, 0, 0, 0, 0, 0, 0, 0], "Cycles"=[0, 0, 0, 0, 0, 0, 0, 0, 0, 0, 0, 0], "Anomalies/Cycle"=[0, 0, 0, 0, 0, 0, 0, 0, 0, 0, 0, 0], "Anomalies (Last Cycle)"=[0, 0, 0, 0, 0, 0, 0, 0, 0, 0, 0, 0], "Opens"=[0, 0, 0, 0, 0, 0, 0, 0, 0, 0, 0, 0]}  # Initial LS Data
  w14 = path ""  # LS Data Filepath
  w16 = u16 0 items=["0 - Off", "1 - On", "2 - Pulsing"]  # Bank 1 State:
  w15 = u16 0 items=["0 - Off", "1 - On", "2 - Pulsing"]  # Bank 2 State:
  w17 = T9."Main"  # Main Tab
  w18 = T15 {"Total Cycles"=[0, 0, 0, 0, 0, 0, 0, 0, 0, 0, 0, 0], "Steps"=[0, 0, 0, 0, 0, 0, 0, 0, 0, 0, 0, 0], "Anomalies Total"=[0, 0, 0, 0, 0, 0, 0, 0, 0, 0, 0, 0], "Cycles"=[0, 0, 0, 0, 0, 0, 0, 0, 0, 0, 0, 0], "Anomalies/Cycle"=[0, 0, 0, 0, 0, 0, 0, 0, 0, 0, 0, 0], "Anomalies (Last Cycle)"=[0, 0, 0, 0, 0, 0, 0, 0, 0, 0, 0, 0], "Opens"=[]}  # LS Data
  w19 = FALSE  # Concat Data
  w20 = FALSE  # Email Alarms Disabled
  w21 = FALSE  # WebDAV Push
  w22 = T16 {"Error"={"status"=FALSE, "code"=0, "source"=""}, "COM Ref"="", "Pump Data"={"Voltages"=[], "PumpCurrent"=[], "Speed"=[], "ControllerCurrent"=[], "Pressure"=[], "Flow"=[], "Elapsed Time (Display)"=[], "Avg Pressure"=0.0, "Avg Speed"=0.0, "Elapsed Time"=[]}, "Tank Data"={"PS Actual (V):"=0.0, "Temp1"=0.0, "Temp2"=0.0}, "Power Relays"={"Pump 1"=FALSE, "Pump 2"=FALSE, "Pump 3"=FALSE, "Pump 4"=FALSE, "Pump 5"=FALSE, "Pump 6"=FALSE}, "Pump CMDs"=[], "HMI Header"={"Line 1"="", "Line 2"="", "Line 3"="", "Line 4"=""}, "Tank CMDs"={"PS CMD"=0.0, "Press CMD"=0.0, "Temp 1 CMD"=0.0, "Temp 2 CMD"=0.0}, "HMI Tog Buttons"={"Start Test"=FALSE, "Toggle Spare 1"=FALSE, "Toggle Spare 2"=FALSE, "Toggle Spare 3"=FALSE, "Toggle Spare 4"=FALSE, "Toggle Spare 5"=FALSE}, "In Test"=FALSE, "HMI Command"=FALSE, "HMI Mom Buttons"={"Stop"=FALSE, "Reset Timers"=FALSE, "Log Fuel Change"=FALSE, "Alarm Dismiss"=FALSE}, "Controller Config"={"Controller Name"=enum."Kuhnke", "CommSeg"=0, "PWM?"=FALSE, "Frequency"=0, "Low Command"=0.0, "High Command"=0.0, "Stop Command"=0.0, "Command Step"=0.0, "Solenoid Stop?"=FALSE, "Controller?"=FALSE, "Invert PWM"=FALSE}, "Alarm"=FALSE, "Alarm Message 1"="", "Alarm Message 2"="", "Recording"=FALSE, "Serial Numbers"=[], "Pumps Present"=[]}  # HMI
  w23 = T23 {"PS Actual (V):"=0.0, "Temp1"=0.0, "Temp2"=0.0}  # Tank Data
  w24 = FALSE  # Recording
  w25 = ""  # Time/Date
  w26 = ""  # Alarm Message 2
  w27 = FALSE  # Alarm Latch
  w28 = T17 {"Voltages"=[0.015201568603515625, 0.00335693359375, 0.003021240234375, 0.12260055541992188, 0.06085968017578125, 0.052234649658203125], "PumpCurrent"=[0.015201568603515625, 0.00335693359375, 0.003021240234375, 0.12260055541992188, 0.06085968017578125, 0.052234649658203125], "Speed"=[0.0, 0.0, 0.0, 0.0, 0.0, 0.0], "ControllerCurrent"=[0.015201568603515625, 0.00335693359375, 0.003021240234375, 0.12260055541992188, 0.06085968017578125, 0.052234649658203125], "Pressure"=[0.015201568603515625, 0.00335693359375, 0.003021240234375, 0.12260055541992188, 0.06085968017578125, 0.052234649658203125], "Flow"=[0.0, 0.0, 0.0, 0.125, 0.0625, 0.0625], "Elapsed Time (Display)"=[7.1, 7.1, 7.1, 458133.45, 458138.85000000003, 458126.75], "Avg Pressure"=0.0, "Avg Speed"=0.0, "Elapsed Time"=[]}  # Pump Data
  w29 = path ""  # Fuel Log Path
  w30 = T22 {"Controller Name"=enum."Kuhnke", "CommSeg"=0, "PWM?"=FALSE, "Frequency"=0, "Low Command"=0.0, "High Command"=0.0, "Stop Command"=0.0, "Command Step"=0.0, "Solenoid Stop?"=FALSE, "Controller?"=FALSE, "Invert PWM"=FALSE}  # Controller Config
  w31 = T19 {"PS CMD"=0.0, "Press CMD"=0.0, "Temp 1 CMD"=0.0, "Temp 2 CMD"=0.0}  # Tank CMDs
  w32 = dbl[][] []  # CalArray
  w33 = u32[] []  # Prev ON Times
  w34 = ""  # Alarm Message 1
  w35 = u32[] []  # Previous Times
  w36 = i32[] []  # Trip Counters
  w37 = path ""  # Alarm Config Path
  w38 = T10 {"Alarms:"=[{"Description:"="", "Enabled:"=FALSE, "Data Index:"=0, "Data Type:"="", "Low Limit:"=0.0, "High Limit:"=0.0, "Trip Time:"=0, "Profile Sync:"=FALSE}, {"Description:"="", "Enabled:"=FALSE, "Data Index:"=0, "Data Type:"="", "Low Limit:"=0.0, "High Limit:"=0.0, "Trip Time:"=0, "Profile Sync:"=FALSE}, {"Description:"="", "Enabled:"=FALSE, "Data Index:"=0, "Data Type:"="", "Low Limit:"=0.0, "High Limit:"=0.0, "Trip Time:"=0, "Profile Sync:"=FALSE}, {"Description:"="", "Enabled:"=FALSE, "Data Index:"=0, "Data Type:"="", "Low Limit:"=0.0, "High Limit:"=0.0, "Trip Time:"=0, "Profile Sync:"=FALSE}, {"Description:"="", "Enabled:"=FALSE, "Data Index:"=0, "Data Type:"="", "Low Limit:"=0.0, "High Limit:"=0.0, "Trip Time:"=0, "Profile Sync:"=FALSE}, {"Description:"="", "Enabled:"=FALSE, "Data Index:"=0, "Data Type:"="", "Low Limit:"=0.0, "High Limit:"=0.0, "Trip Time:"=0, "Profile Sync:"=FALSE}, {"Description:"="", "Enabled:"=FALSE, "Data Index:"=0, "Data Type:"="", "Low Limit:"=0.0, "High Limit:"=0.0, "Trip Time:"=0, "Profile Sync:"=FALSE}, {"Description:"="", "Enabled:"=FALSE, "Data Index:"=0, "Data Type:"="", "Low Limit:"=0.0, "High Limit:"=0.0, "Trip Time:"=0, "Profile Sync:"=FALSE}], "Profile Sync:"={"Trip Time:"=0, "Consecutive Trips:"=0}}  # Alarm Config
  w39 = T24 []  # Controller List
  w40 = T8 {"Pump 1"=FALSE, "Pump 2"=FALSE, "Pump 3"=FALSE, "Pump 4"=FALSE, "Pump 5"=FALSE, "Pump 6"=FALSE}  # Ignition Relay
  w41 = T8 {"Pump 1"=FALSE, "Pump 2"=FALSE, "Pump 3"=FALSE, "Pump 4"=FALSE, "Pump 5"=FALSE, "Pump 6"=FALSE}  # Power Relay
  w42 = FALSE  # Voltage Enable
  w43 = u32 0  # Inputs Timer
  w44 = dbl[] [0.0, 0.0, 0.0, 0.0, 0.0, 0.0]  # Pressure Offsets
  w46 = FALSE  # New Step
  w47 = 0  # Stagger Counter
  w48 = FALSE  # Login
  w49 = dbl[] [0.0, 0.0, 0.0, 0.0, 0.0, 0.0]  # Initial Times
  w50 = bool[] [FALSE, FALSE, FALSE, FALSE, FALSE, FALSE]  # pb.Sets
  w51 = bool[] [FALSE, FALSE, FALSE, FALSE, FALSE, FALSE]  # pb.Resets
  w52 = FALSE  # pb.Run Profile
  w53 = FALSE  # Client?
  w54 = dbl[] [0.0, 0.0, 0.0, 0.0, 0.0, 0.0]  # Controller CMDs
  w55 = 0.0  # Last Profile Time
  w56 = u32 0  # Screen Timer
  w57 = 0  # # of Steps
  w58 = 0.0  # Step Time
  w59 = 0.0  # Step Start Time
  w60 = FALSE  # Run Profile
  w62 = 0  # Current Step
  w61 = 0.0  # Step Time Left
  w63 = string[] []  # Profiles
  w65 = string[][] []  # Profile
  w66 = errorcluster {"status"=FALSE, "code"=0, "source"=""}  # Error
  # "Disabled States:\n   Save LS Test Data\n   Allow Data Note"
  n1 = Bundle("Error"=w66, "Profile"=w65, "App Config"="App Config", "Profiles"=w63, "Current Step"=w62, "Step Time Left"=w61, "Run Profile"=w60, "Step Start Time"=w59, "Step Time"=w58, "# of Steps"=w57, "Screen Timer"=w56, "Last Profile Time"=w55, "Controller CMDs"=w54, "Client?"=w53, "pb.Run Profile"=w52, "pb.Resets"=w51, "pb.Sets"=w50, "Initial Times"=w49, "Pressure Offsets"=w44, "Login"=w48, "Stagger Counter"=w47, "New Step"=w46, "Inputs Timer"=w43, "Tank Data"=w23, "Voltage Enable"=w42, "Power Relay"=w41, "Ignition Relay"=w40, "Controller List"=w39, "Alarm Config"=w38, "Alarm Config Path"=w37, "Trip Counters"=w36, "Previous Times"=w35, "Alarm Message 1"=w34, "Alarm Message 2"=w26, "Prev ON Times"=w33, "CalArray"=w32, "Tank CMDs"=w31, "Controller Config"=w30, "Fuel Log Path"=w29, "Pump Data"=w28, "Alarm Latch"=w27, "Time/Date"=w25, "Recording"=w24, "HMI"=w22, "WebDAV Push"=w21, "Email Alarms Disabled"=w20, "Concat Data"=w19, "LS Data"=w18, "Main Tab"=w17, "LS App Config"=w8, "Bank 1 State:"=w16, "Bank 2 State:"=w15, "LS Data Filepath"=w14, "Initial LS Data"=w13, "day of month"=w9, "Pause Test"=w7, "ProfileMinute"=w6, "ARtime"=w5, "ARactive"=w4) -> (w45:T25)  [unwired: 1 in]
  n2 = xnode "Open FPGA VI Reference"("resource name"=tag "RIO0") -> ("FPGA VI Reference Out"=w3:T26, "error out"=w1:errorcluster)  [unwired: 1 in]
  n3 = Generate Occurrence() -> (w11:refnum<k4>)
  n4 = Wait on Occurrence(2:w11) -> (0:w10:bool)  [unwired: 2 in]
  n5 = while {
    shift-right: [w75] -> _
    shift-left: w12 -> [w73]
    shift-right: [w76] -> _
    shift-left: w45 -> [w77]
    tunnel: w3 -> [w74]
    tunnel: w11 -> [w68]
    tunnel: w1 -> [_]
    stop <- FALSE stop-if-true
    n6 = Delete From Array(array=w73, length=1, index=0 ("length")) -> (deleted portion=w69:T14[], array with subset deleted=w72:T14[])
    n7 = Index Array(array=w69) -> (element=w67:T14)  [unwired: 1 in]
    n8 = case shown="\"Save LS Data\"" w67 {
      selector: w67 -> [_ _ _ _ _ _ _ _ _ _ _ _ _ _ _ _ _ _ _ _ _ _ _ _ _ _ _ w1926 _ _ _ _ _ _ _ _ _ w2183 _ _ _ _ _ _ _ _ _ _ _ _ _]
      tunnel: [w83 w953 w1081 w1116 w1123 w1145 w1165 w1173 w1188 w1202 w1239 w1291 w1322 w1384 w1445 w1539 w1610 w1688 w1723 w1752 w1788 w1809 w1836 w1868 w1898 w1906 w1911 w1917 w2000 w2026 w2038 w2075 w2087 w2098 w2101 w2111 w2168 w2188 w2206 w2220 w2229 w2238 w2246 w2251 w2268 w2296 w2387 w2403 w2471 w2478 w2484] -> w76
      tunnel: w77 -> [w102 w954 w1080 w1116 w1124 w1146 w1165 w1174 w1189 w1203 w1218 w1273 w1323 w1349 w1446 w1564 w1611 w1688 w1723 w1758 w1794 w1810 w1836 w1868 w1898 w1906 w1911 w1927 w2000 w2027 w2037 w2073 w2087 w2098 w2101 w2112 w2168 w2188 w2205 w2220 w2229 w2238 w2246 w2252 w2269 w2297 w2387 w2403 w2472 w2478 w2484]
      tunnel: [w96 w937 w1062 w1115 w1120 w1149 w1166 w1167 w1178 w1198 w1232 w1286 w1292 w1364 w1433 w1534 w1588 w1701 w1719 w1761 w1797 w1804 w1837 w1867 w1899 w1905 w1909 w1924 w2006 w2028 w2032 w2069 w2086 w2097 w2102 w2109 w2167 w2189 w2209 w2221 w2230 w2237 w2241 w2260 w2265 w2298 w2386 w2402 w2470 w2479 w2487] -> w75
      tunnel: w74 -> [_ _ w1036 _ _ _ _ _ _ _ _ _ _ _ w1409 w1517 _ _ _ _ _ _ w1828 _ _ _ w1910 w1928 _ _ w2036 w2074 _ _ _ w2113 _ _ _ _ _ w2233 _ _ _ _ _ _ _ _ _]
      tunnel: w72 -> [w90 w935 w1065 w1115 w1119 w1149 w1166 w1168 w1179 w1198 w1233 w1287 w1304 w1380 w1401 w1549 w1631 w1700 w1720 w1762 w1798 w1805 w1837 w1867 w1899 w1905 w1909 w1925 w2007 w2029 w2033 w2068 w2086 w2097 w2103 w2110 w2167 w2189 w2210 w2221 w2230 w2237 w2242 w2261 w2277 w2298 w2386 w2402 w2470 w2479 w2488]
      tunnel: w68 -> [_ _ w1074 _ _ _ _ _ _ _ _ _ _ _ _ _ _ _ _ _ _ _ _ _ _ _ _ _ _ _ _ _ _ _ _ _ _ _ _ _ _ _ _ _ _ _ _ _ _ _ _]
      frame "Main", Default {
        (unwired) Sequence_States."Update Screen"
        n9 = Unbundle By Name(w102) -> ("Run Profile"=w82:bool, "Inputs Timer"=w89:u32, "Screen Timer"=w88:u32)
        n10 = Wait (ms)(milliseconds to wait=u32 10) -> ()  [unwired: 1 out]
        n11 = for {
          N: 80 -> [_]
          shift-right: [w129] -> w83
          shift-left: w102 -> [w128]
          tunnel: [w127] -> w98
          tunnel: [w126] -> w97
          i -> [w125]
          stop <- w126 stop-if-true
          n12 = case shown="73" w125 {
            tunnel: w128 -> [w134 w146 w150 w159 w166 w167 w178 w193 w210 w217 w222 w241 w249 w254 w267 w268 w280 w288 w294 w309 w320 w326 w341 w358 w364 w376 w392 w406 w422 w437 w451 w454 w461 w476 w493 w510 w527 w544 w561 w578 w595 w611 w626 w641 w654 w661 w667 w672 w679 w686 w693 w700 w714 w722 w729 w738 w747 w754 w761 w768 w775 w782 w789 w801 w808 w815 w818 w821 w824 w832 w839 w846 w853 w856 w864 w871 w880 w887 w894]
            tunnel: [w133 w146 w150 w158 w166 w167 w177 w192 w209 w216 w221 w240 w248 w253 w267 w268 w279 w287 w293 w308 w320 w325 w340 w357 w363 w375 w391 w405 w421 w436 w451 w454 w460 w475 w492 w509 w526 w543 w560 w577 w594 w610 w625 w640 w654 w660 w666 w671 w678 w685 w692 w699 w713 w721 w728 w737 w746 w753 w760 w767 w774 w781 w788 w800 w807 w814 w818 w821 w824 w831 w838 w845 w853 w856 w863 w870 w879 w886 w893] -> w129
            tunnel: w128 -> [w132 _ _ w157 w164 _ w175 w190 w208 w215 w220 w239 w247 w252 _ _ w277 w285 w291 w307 _ w324 w339 w356 w362 w377 w394 w407 w423 w438 _ _ w462 w477 w494 w511 w528 w545 w562 w579 w596 w612 w624 w639 _ w662 _ _ w677 w684 w691 w698 w715 w723 w730 w739 w748 w755 w762 w769 w776 w783 w790 w802 w809 w816 _ _ _ w830 w840 w847 _ _ w862 w869 w878 w885 w892]
            tunnel: [w131 w147 w151 w156 w161 w169 w174 w189 w205 w211 w219 w237 w243 w250 w266 w270 w276 w284 w290 w306 w322 w327 w342 w359 w361 w379 w399 w409 w424 w439 w452 w455 w458 w474 w490 w507 w524 w541 w558 w576 w593 w609 w627 w642 w656 w663 w668 w673 w680 w687 w694 w701 w710 w720 w727 w736 w745 w752 w759 w766 w773 w780 w787 w799 w806 w813 w819 w822 w825 w827 w835 w842 w851 w855 w860 w867 w872 w881 w889] -> w127
            tunnel: [w130 w145 "pb.Save As" w153 "pb.Stop Profile" w168 w176 w191 w206 w213 w218 w235 w245 w251 FALSE ("pb.Tare Pressure") w269 w278 w286 w292 w305 "pb.FuelChange" w323 w338 w353 w360 w378 w395 w408 w420 w435 "pb.Alarm OK" w453 w459 w473 w491 w508 w525 w542 w559 w575 w592 w608 w623 w638 w653 w657 FALSE ("HMI Command") FALSE ("HMI Command") w676 w683 w690 w697 w709 w717 w725 w731 w741 w750 w757 w764 w771 w778 w785 w794 w803 w811 "Reset Total Cycles" "Reset Anomalies" "Reset Opens" w828 w837 w844 FALSE ("Reset Opens") FALSE ("Reset Opens") w857 w866 w876 w883 w890] -> w126
            frame 0, Default {
              n13 = disable-structure shown="Enabled" {
                disable-tunnel: w134 -> [w141 w144]
                disable-tunnel: [w140 w144] -> w133
                disable-tunnel: w132 -> [w139 _]
                disable-tunnel: [w138 w142] -> w131
                disable-tunnel: [w135 FALSE] -> w130
                frame Disabled {
                  w138 = T14[] [enum."Write Outputs"] items=["Main", "Init Files", "Init", "Unused", "Save As", "Start Profile", "Check Step Time", "Alarm", "Alarm Dismiss", "Run Step", "Stop Profile", "Cycle Reset", "Time Reset", "Time Reset All", "Time Set", "Tare CTs", "Save Profile", "Open Profile", "Get Profiles", "Update Screen", "Update Controls", "Save App Config", "Write Outputs", "Disable Background", "Enable Background", "Get/Release Control", "Log Fuel Change", "Fuel Change Popup", "Read Inputs", "Remote Timer Reset", "Controller Change", "Get Alarms", "Init Alarms", "Save Alarms", "Voltage Selection", "Set Watlow Temp 1", "Set Watlow Temp 2", "Get Pressure", "Write Tare Pressure", "Adjust Controls", "Reinit ADC", "Write Initial Times", "Write Pumps Present", "HMI Command", "Save Pump Times", "Check Pump Stop Time", "Save LS App Config", "Init Data File", "Reset LS Cycles", "Reset Anomalies", "Reset Opens", "Save LS Data", "Save LS Test Data", "Check Serial Numbers", "Main Tab", "Allow Data Note", "Resume Profile", "Pause Profile", "Allow Pause Note", "Clear Graph"]
                  n14 = Unbundle By Name(w139) -> ("Tank CMDs.PS CMD"=w137:dbl)
                  n15 = Not Equal?(x=w137, y="Power Supply Cmd:") -> (x != y?=w135:bool)
                  n16 = Bundle By Name(cluster=w141, "Tank CMDs.PS CMD"="Power Supply Cmd:") -> (w140:T25)
                }
                frame Enabled {
                  w142 = T14[] [] items=["Main", "Init Files", "Init", "Unused", "Save As", "Start Profile", "Check Step Time", "Alarm", "Alarm Dismiss", "Run Step", "Stop Profile", "Cycle Reset", "Time Reset", "Time Reset All", "Time Set", "Tare CTs", "Save Profile", "Open Profile", "Get Profiles", "Update Screen", "Update Controls", "Save App Config", "Write Outputs", "Disable Background", "Enable Background", "Get/Release Control", "Log Fuel Change", "Fuel Change Popup", "Read Inputs", "Remote Timer Reset", "Controller Change", "Get Alarms", "Init Alarms", "Save Alarms", "Voltage Selection", "Set Watlow Temp 1", "Set Watlow Temp 2", "Get Pressure", "Write Tare Pressure", "Adjust Controls", "Reinit ADC", "Write Initial Times", "Write Pumps Present", "HMI Command", "Save Pump Times", "Check Pump Stop Time", "Save LS App Config", "Init Data File", "Reset LS Cycles", "Reset Anomalies", "Reset Opens", "Save LS Data", "Save LS Test Data", "Check Serial Numbers", "Main Tab", "Allow Data Note", "Resume Profile", "Pause Profile", "Allow Pause Note", "Clear Graph"]
                }
              }
            }
            frame 1 {
              w147 = T14[] [enum."Stop Profile"] items=["Main", "Init Files", "Init", "Unused", "Save As", "Start Profile", "Check Step Time", "Alarm", "Alarm Dismiss", "Run Step", "Stop Profile", "Cycle Reset", "Time Reset", "Time Reset All", "Time Set", "Tare CTs", "Save Profile", "Open Profile", "Get Profiles", "Update Screen", "Update Controls", "Save App Config", "Write Outputs", "Disable Background", "Enable Background", "Get/Release Control", "Log Fuel Change", "Fuel Change Popup", "Read Inputs", "Remote Timer Reset", "Controller Change", "Get Alarms", "Init Alarms", "Save Alarms", "Voltage Selection", "Set Watlow Temp 1", "Set Watlow Temp 2", "Get Pressure", "Write Tare Pressure", "Adjust Controls", "Reinit ADC", "Write Initial Times", "Write Pumps Present", "HMI Command", "Save Pump Times", "Check Pump Stop Time", "Save LS App Config", "Init Data File", "Reset LS Cycles", "Reset Anomalies", "Reset Opens", "Save LS Data", "Save LS Test Data", "Check Serial Numbers", "Main Tab", "Allow Data Note", "Resume Profile", "Pause Profile", "Allow Pause Note", "Clear Graph"]
              n17 = disable-structure shown="Enabled" {
                disable-tunnel: ["pb.E Stop" FALSE ("pb.E Stop")] -> w145
                frame Disabled {
                }
                frame Enabled {
                }
              }
            }
            frame 2 {
              w151 = T14[] [enum."Disable Background", enum."Save As"] items=["Main", "Init Files", "Init", "Unused", "Save As", "Start Profile", "Check Step Time", "Alarm", "Alarm Dismiss", "Run Step", "Stop Profile", "Cycle Reset", "Time Reset", "Time Reset All", "Time Set", "Tare CTs", "Save Profile", "Open Profile", "Get Profiles", "Update Screen", "Update Controls", "Save App Config", "Write Outputs", "Disable Background", "Enable Background", "Get/Release Control", "Log Fuel Change", "Fuel Change Popup", "Read Inputs", "Remote Timer Reset", "Controller Change", "Get Alarms", "Init Alarms", "Save Alarms", "Voltage Selection", "Set Watlow Temp 1", "Set Watlow Temp 2", "Get Pressure", "Write Tare Pressure", "Adjust Controls", "Reinit ADC", "Write Initial Times", "Write Pumps Present", "HMI Command", "Save Pump Times", "Check Pump Stop Time", "Save LS App Config", "Init Data File", "Reset LS Cycles", "Reset Anomalies", "Reset Opens", "Save LS Data", "Save LS Test Data", "Check Serial Numbers", "Main Tab", "Allow Data Note", "Resume Profile", "Pause Profile", "Allow Pause Note", "Clear Graph"]
            }
            frame 3 {
              w156 = T14[] [enum."Voltage Selection", enum."Start Profile"] items=["Main", "Init Files", "Init", "Unused", "Save As", "Start Profile", "Check Step Time", "Alarm", "Alarm Dismiss", "Run Step", "Stop Profile", "Cycle Reset", "Time Reset", "Time Reset All", "Time Set", "Tare CTs", "Save Profile", "Open Profile", "Get Profiles", "Update Screen", "Update Controls", "Save App Config", "Write Outputs", "Disable Background", "Enable Background", "Get/Release Control", "Log Fuel Change", "Fuel Change Popup", "Read Inputs", "Remote Timer Reset", "Controller Change", "Get Alarms", "Init Alarms", "Save Alarms", "Voltage Selection", "Set Watlow Temp 1", "Set Watlow Temp 2", "Get Pressure", "Write Tare Pressure", "Adjust Controls", "Reinit ADC", "Write Initial Times", "Write Pumps Present", "HMI Command", "Save Pump Times", "Check Pump Stop Time", "Save LS App Config", "Init Data File", "Reset LS Cycles", "Reset Anomalies", "Reset Opens", "Save LS Data", "Save LS Test Data", "Check Serial Numbers", "Main Tab", "Allow Data Note", "Resume Profile", "Pause Profile", "Allow Pause Note", "Clear Graph"]
              n18 = Unbundle By Name(w157) -> ("pb.Run Profile"=w155:bool)
              n19 = Greater?(x="pb.Run Profile", y=w155) -> (0:w153:bool)
              n20 = Bundle By Name(cluster=w159, "pb.Run Profile"="pb.Run Profile") -> (w158:T25)
            }
            frame 4 {
              w160 = T14[] [enum."Stop Profile", enum."Save LS Data"] items=["Main", "Init Files", "Init", "Unused", "Save As", "Start Profile", "Check Step Time", "Alarm", "Alarm Dismiss", "Run Step", "Stop Profile", "Cycle Reset", "Time Reset", "Time Reset All", "Time Set", "Tare CTs", "Save Profile", "Open Profile", "Get Profiles", "Update Screen", "Update Controls", "Save App Config", "Write Outputs", "Disable Background", "Enable Background", "Get/Release Control", "Log Fuel Change", "Fuel Change Popup", "Read Inputs", "Remote Timer Reset", "Controller Change", "Get Alarms", "Init Alarms", "Save Alarms", "Voltage Selection", "Set Watlow Temp 1", "Set Watlow Temp 2", "Get Pressure", "Write Tare Pressure", "Adjust Controls", "Reinit ADC", "Write Initial Times", "Write Pumps Present", "HMI Command", "Save Pump Times", "Check Pump Stop Time", "Save LS App Config", "Init Data File", "Reset LS Cycles", "Reset Anomalies", "Reset Opens", "Save LS Data", "Save LS Test Data", "Check Serial Numbers", "Main Tab", "Allow Data Note", "Resume Profile", "Pause Profile", "Allow Pause Note", "Clear Graph"]
              w162 = T14[] [enum."Stop Profile", enum."Save LS Data", enum."Allow Data Note"] items=["Main", "Init Files", "Init", "Unused", "Save As", "Start Profile", "Check Step Time", "Alarm", "Alarm Dismiss", "Run Step", "Stop Profile", "Cycle Reset", "Time Reset", "Time Reset All", "Time Set", "Tare CTs", "Save Profile", "Open Profile", "Get Profiles", "Update Screen", "Update Controls", "Save App Config", "Write Outputs", "Disable Background", "Enable Background", "Get/Release Control", "Log Fuel Change", "Fuel Change Popup", "Read Inputs", "Remote Timer Reset", "Controller Change", "Get Alarms", "Init Alarms", "Save Alarms", "Voltage Selection", "Set Watlow Temp 1", "Set Watlow Temp 2", "Get Pressure", "Write Tare Pressure", "Adjust Controls", "Reinit ADC", "Write Initial Times", "Write Pumps Present", "HMI Command", "Save Pump Times", "Check Pump Stop Time", "Save LS App Config", "Init Data File", "Reset LS Cycles", "Reset Anomalies", "Reset Opens", "Save LS Data", "Save LS Test Data", "Check Serial Numbers", "Main Tab", "Allow Data Note", "Resume Profile", "Pause Profile", "Allow Pause Note", "Clear Graph"]
              n21 = Unbundle By Name(w164) -> ("pb.Run Profile"=w163:bool)
              n22 = Select(t=w162, s=w163, f=w160) -> (s? t:f=w161:T14[])
            }
            frame 5 {
              n23 = disable-structure shown="Enabled" {
                disable-tunnel: [w171 w172] -> w169
                disable-tunnel: ["pb.Cycle Reset" FALSE ("pb.Cycle Reset")] -> w168
                frame Disabled {
                  w171 = T14[] [enum."Disable Background", enum."Cycle Reset"] items=["Main", "Init Files", "Init", "Unused", "Save As", "Start Profile", "Check Step Time", "Alarm", "Alarm Dismiss", "Run Step", "Stop Profile", "Cycle Reset", "Time Reset", "Time Reset All", "Time Set", "Tare CTs", "Save Profile", "Open Profile", "Get Profiles", "Update Screen", "Update Controls", "Save App Config", "Write Outputs", "Disable Background", "Enable Background", "Get/Release Control", "Log Fuel Change", "Fuel Change Popup", "Read Inputs", "Remote Timer Reset", "Controller Change", "Get Alarms", "Init Alarms", "Save Alarms", "Voltage Selection", "Set Watlow Temp 1", "Set Watlow Temp 2", "Get Pressure", "Write Tare Pressure", "Adjust Controls", "Reinit ADC", "Write Initial Times", "Write Pumps Present", "HMI Command", "Save Pump Times", "Check Pump Stop Time", "Save LS App Config", "Init Data File", "Reset LS Cycles", "Reset Anomalies", "Reset Opens", "Save LS Data", "Save LS Test Data", "Check Serial Numbers", "Main Tab", "Allow Data Note", "Resume Profile", "Pause Profile", "Allow Pause Note", "Clear Graph"]
                }
                frame Enabled {
                  w172 = T14[] [] items=["Main", "Init Files", "Init", "Unused", "Save As", "Start Profile", "Check Step Time", "Alarm", "Alarm Dismiss", "Run Step", "Stop Profile", "Cycle Reset", "Time Reset", "Time Reset All", "Time Set", "Tare CTs", "Save Profile", "Open Profile", "Get Profiles", "Update Screen", "Update Controls", "Save App Config", "Write Outputs", "Disable Background", "Enable Background", "Get/Release Control", "Log Fuel Change", "Fuel Change Popup", "Read Inputs", "Remote Timer Reset", "Controller Change", "Get Alarms", "Init Alarms", "Save Alarms", "Voltage Selection", "Set Watlow Temp 1", "Set Watlow Temp 2", "Get Pressure", "Write Tare Pressure", "Adjust Controls", "Reinit ADC", "Write Initial Times", "Write Pumps Present", "HMI Command", "Save Pump Times", "Check Pump Stop Time", "Save LS App Config", "Init Data File", "Reset LS Cycles", "Reset Anomalies", "Reset Opens", "Save LS Data", "Save LS Test Data", "Check Serial Numbers", "Main Tab", "Allow Data Note", "Resume Profile", "Pause Profile", "Allow Pause Note", "Clear Graph"]
                }
              }
            }
            frame 6 {
              n24 = disable-structure shown="Enabled" {
                disable-tunnel: w178 -> [w184 w188]
                disable-tunnel: [w183 w188] -> w177
                disable-tunnel: [w182 FALSE] -> w176
                disable-tunnel: w175 -> [w181 _]
                disable-tunnel: [w179 w186] -> w174
                frame Disabled {
                  w179 = T14[] [enum."Disable Background", enum."Time Reset", enum."Update Controls"] items=["Main", "Init Files", "Init", "Unused", "Save As", "Start Profile", "Check Step Time", "Alarm", "Alarm Dismiss", "Run Step", "Stop Profile", "Cycle Reset", "Time Reset", "Time Reset All", "Time Set", "Tare CTs", "Save Profile", "Open Profile", "Get Profiles", "Update Screen", "Update Controls", "Save App Config", "Write Outputs", "Disable Background", "Enable Background", "Get/Release Control", "Log Fuel Change", "Fuel Change Popup", "Read Inputs", "Remote Timer Reset", "Controller Change", "Get Alarms", "Init Alarms", "Save Alarms", "Voltage Selection", "Set Watlow Temp 1", "Set Watlow Temp 2", "Get Pressure", "Write Tare Pressure", "Adjust Controls", "Reinit ADC", "Write Initial Times", "Write Pumps Present", "HMI Command", "Save Pump Times", "Check Pump Stop Time", "Save LS App Config", "Init Data File", "Reset LS Cycles", "Reset Anomalies", "Reset Opens", "Save LS Data", "Save LS Test Data", "Check Serial Numbers", "Main Tab", "Allow Data Note", "Resume Profile", "Pause Profile", "Allow Pause Note", "Clear Graph"]
                  n25 = Unbundle By Name(w181) -> ("pb.Resets"=w185:bool[])
                  n26 = Greater?(x="pb.Resets", y=w185) -> (0:w182:bool)
                  n27 = Bundle By Name(cluster=w184, "pb.Resets"="pb.Resets") -> (w183:T25)
                }
                frame Enabled {
                  w186 = T14[] [] items=["Main", "Init Files", "Init", "Unused", "Save As", "Start Profile", "Check Step Time", "Alarm", "Alarm Dismiss", "Run Step", "Stop Profile", "Cycle Reset", "Time Reset", "Time Reset All", "Time Set", "Tare CTs", "Save Profile", "Open Profile", "Get Profiles", "Update Screen", "Update Controls", "Save App Config", "Write Outputs", "Disable Background", "Enable Background", "Get/Release Control", "Log Fuel Change", "Fuel Change Popup", "Read Inputs", "Remote Timer Reset", "Controller Change", "Get Alarms", "Init Alarms", "Save Alarms", "Voltage Selection", "Set Watlow Temp 1", "Set Watlow Temp 2", "Get Pressure", "Write Tare Pressure", "Adjust Controls", "Reinit ADC", "Write Initial Times", "Write Pumps Present", "HMI Command", "Save Pump Times", "Check Pump Stop Time", "Save LS App Config", "Init Data File", "Reset LS Cycles", "Reset Anomalies", "Reset Opens", "Save LS Data", "Save LS Test Data", "Check Serial Numbers", "Main Tab", "Allow Data Note", "Resume Profile", "Pause Profile", "Allow Pause Note", "Clear Graph"]
                }
              }
            }
            frame 7 {
              n28 = disable-structure shown="Enabled" {
                disable-tunnel: w193 -> [w199 w203]
                disable-tunnel: [w198 w203] -> w192
                disable-tunnel: [w197 FALSE] -> w191
                disable-tunnel: w190 -> [w196 _]
                disable-tunnel: [w194 w201] -> w189
                frame Disabled {
                  w194 = T14[] [enum."Disable Background", enum."Time Set", enum."Update Controls"] items=["Main", "Init Files", "Init", "Unused", "Save As", "Start Profile", "Check Step Time", "Alarm", "Alarm Dismiss", "Run Step", "Stop Profile", "Cycle Reset", "Time Reset", "Time Reset All", "Time Set", "Tare CTs", "Save Profile", "Open Profile", "Get Profiles", "Update Screen", "Update Controls", "Save App Config", "Write Outputs", "Disable Background", "Enable Background", "Get/Release Control", "Log Fuel Change", "Fuel Change Popup", "Read Inputs", "Remote Timer Reset", "Controller Change", "Get Alarms", "Init Alarms", "Save Alarms", "Voltage Selection", "Set Watlow Temp 1", "Set Watlow Temp 2", "Get Pressure", "Write Tare Pressure", "Adjust Controls", "Reinit ADC", "Write Initial Times", "Write Pumps Present", "HMI Command", "Save Pump Times", "Check Pump Stop Time", "Save LS App Config", "Init Data File", "Reset LS Cycles", "Reset Anomalies", "Reset Opens", "Save LS Data", "Save LS Test Data", "Check Serial Numbers", "Main Tab", "Allow Data Note", "Resume Profile", "Pause Profile", "Allow Pause Note", "Clear Graph"]
                  n29 = Unbundle By Name(w196) -> ("pb.Sets"=w200:bool[])
                  n30 = Greater?(x="pb.Sets", y=w200) -> (0:w197:bool)
                  n31 = Bundle By Name(cluster=w199, "pb.Sets"="pb.Sets") -> (w198:T25)
                }
                frame Enabled {
                  w201 = T14[] [] items=["Main", "Init Files", "Init", "Unused", "Save As", "Start Profile", "Check Step Time", "Alarm", "Alarm Dismiss", "Run Step", "Stop Profile", "Cycle Reset", "Time Reset", "Time Reset All", "Time Set", "Tare CTs", "Save Profile", "Open Profile", "Get Profiles", "Update Screen", "Update Controls", "Save App Config", "Write Outputs", "Disable Background", "Enable Background", "Get/Release Control", "Log Fuel Change", "Fuel Change Popup", "Read Inputs", "Remote Timer Reset", "Controller Change", "Get Alarms", "Init Alarms", "Save Alarms", "Voltage Selection", "Set Watlow Temp 1", "Set Watlow Temp 2", "Get Pressure", "Write Tare Pressure", "Adjust Controls", "Reinit ADC", "Write Initial Times", "Write Pumps Present", "HMI Command", "Save Pump Times", "Check Pump Stop Time", "Save LS App Config", "Init Data File", "Reset LS Cycles", "Reset Anomalies", "Reset Opens", "Save LS Data", "Save LS Test Data", "Check Serial Numbers", "Main Tab", "Allow Data Note", "Resume Profile", "Pause Profile", "Allow Pause Note", "Clear Graph"]
                }
              }
            }
            frame 8 {
              w205 = T14[] [enum."Save Profile", enum."Update Controls"] items=["Main", "Init Files", "Init", "Unused", "Save As", "Start Profile", "Check Step Time", "Alarm", "Alarm Dismiss", "Run Step", "Stop Profile", "Cycle Reset", "Time Reset", "Time Reset All", "Time Set", "Tare CTs", "Save Profile", "Open Profile", "Get Profiles", "Update Screen", "Update Controls", "Save App Config", "Write Outputs", "Disable Background", "Enable Background", "Get/Release Control", "Log Fuel Change", "Fuel Change Popup", "Read Inputs", "Remote Timer Reset", "Controller Change", "Get Alarms", "Init Alarms", "Save Alarms", "Voltage Selection", "Set Watlow Temp 1", "Set Watlow Temp 2", "Get Pressure", "Write Tare Pressure", "Adjust Controls", "Reinit ADC", "Write Initial Times", "Write Pumps Present", "HMI Command", "Save Pump Times", "Check Pump Stop Time", "Save LS App Config", "Init Data File", "Reset LS Cycles", "Reset Anomalies", "Reset Opens", "Save LS Data", "Save LS Test Data", "Check Serial Numbers", "Main Tab", "Allow Data Note", "Resume Profile", "Pause Profile", "Allow Pause Note", "Clear Graph"]
              n32 = Unbundle By Name(w208) -> ("Profile"=w207:string[][])
              n33 = Not Equal?(x=w207, y="Profile:") -> (x != y?=w206:bool)
              n34 = Bundle By Name(cluster=w210, "Profile"="Profile:") -> (w209:T25)
            }
            frame 9 {
              w211 = T14[] [enum."Open Profile", enum."Update Controls"] items=["Main", "Init Files", "Init", "Unused", "Save As", "Start Profile", "Check Step Time", "Alarm", "Alarm Dismiss", "Run Step", "Stop Profile", "Cycle Reset", "Time Reset", "Time Reset All", "Time Set", "Tare CTs", "Save Profile", "Open Profile", "Get Profiles", "Update Screen", "Update Controls", "Save App Config", "Write Outputs", "Disable Background", "Enable Background", "Get/Release Control", "Log Fuel Change", "Fuel Change Popup", "Read Inputs", "Remote Timer Reset", "Controller Change", "Get Alarms", "Init Alarms", "Save Alarms", "Voltage Selection", "Set Watlow Temp 1", "Set Watlow Temp 2", "Get Pressure", "Write Tare Pressure", "Adjust Controls", "Reinit ADC", "Write Initial Times", "Write Pumps Present", "HMI Command", "Save Pump Times", "Check Pump Stop Time", "Save LS App Config", "Init Data File", "Reset LS Cycles", "Reset Anomalies", "Reset Opens", "Save LS Data", "Save LS Test Data", "Check Serial Numbers", "Main Tab", "Allow Data Note", "Resume Profile", "Pause Profile", "Allow Pause Note", "Clear Graph"]
              n35 = Unbundle By Name(w215) -> ("App Config.Current Profile"=w214:string)
              n36 = Not Equal?(x=w214, y="Profile Name:") -> (x != y?=w213:bool)
              n37 = Bundle By Name(cluster=w217, "App Config.Current Profile"="Profile Name:") -> (w216:T25)
            }
            frame 10 {
              n38 = disable-structure shown="Enabled" {
                disable-tunnel: w222 -> [w230 w233]
                disable-tunnel: [w229 w233] -> w221
                disable-tunnel: w220 -> [w228 _]
                disable-tunnel: [w227 w231] -> w219
                disable-tunnel: [w223 FALSE] -> w218
                frame Disabled {
                  w227 = T14[] [enum."Write Outputs"] items=["Main", "Init Files", "Init", "Unused", "Save As", "Start Profile", "Check Step Time", "Alarm", "Alarm Dismiss", "Run Step", "Stop Profile", "Cycle Reset", "Time Reset", "Time Reset All", "Time Set", "Tare CTs", "Save Profile", "Open Profile", "Get Profiles", "Update Screen", "Update Controls", "Save App Config", "Write Outputs", "Disable Background", "Enable Background", "Get/Release Control", "Log Fuel Change", "Fuel Change Popup", "Read Inputs", "Remote Timer Reset", "Controller Change", "Get Alarms", "Init Alarms", "Save Alarms", "Voltage Selection", "Set Watlow Temp 1", "Set Watlow Temp 2", "Get Pressure", "Write Tare Pressure", "Adjust Controls", "Reinit ADC", "Write Initial Times", "Write Pumps Present", "HMI Command", "Save Pump Times", "Check Pump Stop Time", "Save LS App Config", "Init Data File", "Reset LS Cycles", "Reset Anomalies", "Reset Opens", "Save LS Data", "Save LS Test Data", "Check Serial Numbers", "Main Tab", "Allow Data Note", "Resume Profile", "Pause Profile", "Allow Pause Note", "Clear Graph"]
                  n39 = Unbundle By Name(w228) -> ("Controller CMDs"=w226:dbl[])
                  n40 = Not Equal?(x="Controller\nCMD", y=w226) -> (x != y?=w224:bool[])
                  n41 = Or Array Elements(Boolean array=w224) -> (logical OR=w223:bool)
                  n42 = Bundle By Name(cluster=w230, "Controller CMDs"="Controller\nCMD") -> (w229:T25)
                }
                frame Enabled {
                  w231 = T14[] [] items=["Main", "Init Files", "Init", "Unused", "Save As", "Start Profile", "Check Step Time", "Alarm", "Alarm Dismiss", "Run Step", "Stop Profile", "Cycle Reset", "Time Reset", "Time Reset All", "Time Set", "Tare CTs", "Save Profile", "Open Profile", "Get Profiles", "Update Screen", "Update Controls", "Save App Config", "Write Outputs", "Disable Background", "Enable Background", "Get/Release Control", "Log Fuel Change", "Fuel Change Popup", "Read Inputs", "Remote Timer Reset", "Controller Change", "Get Alarms", "Init Alarms", "Save Alarms", "Voltage Selection", "Set Watlow Temp 1", "Set Watlow Temp 2", "Get Pressure", "Write Tare Pressure", "Adjust Controls", "Reinit ADC", "Write Initial Times", "Write Pumps Present", "HMI Command", "Save Pump Times", "Check Pump Stop Time", "Save LS App Config", "Init Data File", "Reset LS Cycles", "Reset Anomalies", "Reset Opens", "Save LS Data", "Save LS Test Data", "Check Serial Numbers", "Main Tab", "Allow Data Note", "Resume Profile", "Pause Profile", "Allow Pause Note", "Clear Graph"]
                }
              }
            }
            frame 11 {
              w237 = T14[] [enum."Get/Release Control"] items=["Main", "Init Files", "Init", "Unused", "Save As", "Start Profile", "Check Step Time", "Alarm", "Alarm Dismiss", "Run Step", "Stop Profile", "Cycle Reset", "Time Reset", "Time Reset All", "Time Set", "Tare CTs", "Save Profile", "Open Profile", "Get Profiles", "Update Screen", "Update Controls", "Save App Config", "Write Outputs", "Disable Background", "Enable Background", "Get/Release Control", "Log Fuel Change", "Fuel Change Popup", "Read Inputs", "Remote Timer Reset", "Controller Change", "Get Alarms", "Init Alarms", "Save Alarms", "Voltage Selection", "Set Watlow Temp 1", "Set Watlow Temp 2", "Get Pressure", "Write Tare Pressure", "Adjust Controls", "Reinit ADC", "Write Initial Times", "Write Pumps Present", "HMI Command", "Save Pump Times", "Check Pump Stop Time", "Save LS App Config", "Init Data File", "Reset LS Cycles", "Reset Anomalies", "Reset Opens", "Save LS Data", "Save LS Test Data", "Check Serial Numbers", "Main Tab", "Allow Data Note", "Resume Profile", "Pause Profile", "Allow Pause Note", "Clear Graph"]
              n43 = Unbundle By Name(w239) -> ("Client?"=w236:bool, "Profiles"=w238:string[])
              n44 = call "App Global.vi"() -> ("Client? OUT"=w234:bool)  [unwired: 9 in, 2 out]
              n45 = Greater?(x=w234, y=w236) -> (0:w235:bool)
              n46 = case shown="True" w235 {
                tunnel: w238 -> [_ w242]
                frame False {
                }
                frame True {
                  n47 = property on="Profile Name:" class="CmbBox"("Strings[]"=w242) -> ()  [unwired: 2 in, 2 out]
                }
              }
              n48 = Bundle By Name(cluster=w241, "Client?"=w234) -> (w240:T25)
            }
            frame 13 {
              w243 = T14[] [enum."Init Data File", enum."Save LS App Config", enum."Save App Config"] items=["Main", "Init Files", "Init", "Unused", "Save As", "Start Profile", "Check Step Time", "Alarm", "Alarm Dismiss", "Run Step", "Stop Profile", "Cycle Reset", "Time Reset", "Time Reset All", "Time Set", "Tare CTs", "Save Profile", "Open Profile", "Get Profiles", "Update Screen", "Update Controls", "Save App Config", "Write Outputs", "Disable Background", "Enable Background", "Get/Release Control", "Log Fuel Change", "Fuel Change Popup", "Read Inputs", "Remote Timer Reset", "Controller Change", "Get Alarms", "Init Alarms", "Save Alarms", "Voltage Selection", "Set Watlow Temp 1", "Set Watlow Temp 2", "Get Pressure", "Write Tare Pressure", "Adjust Controls", "Reinit ADC", "Write Initial Times", "Write Pumps Present", "HMI Command", "Save Pump Times", "Check Pump Stop Time", "Save LS App Config", "Init Data File", "Reset LS Cycles", "Reset Anomalies", "Reset Opens", "Save LS Data", "Save LS Test Data", "Check Serial Numbers", "Main Tab", "Allow Data Note", "Resume Profile", "Pause Profile", "Allow Pause Note", "Clear Graph"]
              n49 = Unbundle By Name(w247) -> ("App Config.CA Number"=w246:string)
              n50 = Not Equal?(x=w246, y="CA Number:") -> (x != y?=w245:bool)
              n51 = Bundle By Name(cluster=w249, "App Config.CA Number"="CA Number:") -> (w248:T25)
            }
            frame 14 {
              n52 = disable-structure shown="Enabled" {
                disable-tunnel: w254 -> [w261 w264]
                disable-tunnel: [w260 w264] -> w253
                disable-tunnel: w252 -> [w259 _]
                disable-tunnel: [w257 FALSE] -> w251
                disable-tunnel: [w256 w262] -> w250
                frame Disabled {
                  w256 = T14[] [enum."Save App Config", enum."Controller Change", enum."Write Outputs"] items=["Main", "Init Files", "Init", "Unused", "Save As", "Start Profile", "Check Step Time", "Alarm", "Alarm Dismiss", "Run Step", "Stop Profile", "Cycle Reset", "Time Reset", "Time Reset All", "Time Set", "Tare CTs", "Save Profile", "Open Profile", "Get Profiles", "Update Screen", "Update Controls", "Save App Config", "Write Outputs", "Disable Background", "Enable Background", "Get/Release Control", "Log Fuel Change", "Fuel Change Popup", "Read Inputs", "Remote Timer Reset", "Controller Change", "Get Alarms", "Init Alarms", "Save Alarms", "Voltage Selection", "Set Watlow Temp 1", "Set Watlow Temp 2", "Get Pressure", "Write Tare Pressure", "Adjust Controls", "Reinit ADC", "Write Initial Times", "Write Pumps Present", "HMI Command", "Save Pump Times", "Check Pump Stop Time", "Save LS App Config", "Init Data File", "Reset LS Cycles", "Reset Anomalies", "Reset Opens", "Save LS Data", "Save LS Test Data", "Check Serial Numbers", "Main Tab", "Allow Data Note", "Resume Profile", "Pause Profile", "Allow Pause Note", "Clear Graph"]
                  n53 = Unbundle By Name(w259) -> ("App Config.Controller Type:"=w258:T3)
                  n54 = Not Equal?(x=w258, y="Controller Type:") -> (x != y?=w257:bool)
                  n55 = Bundle By Name(cluster=w261, "App Config.Controller Type:"="Controller Type:") -> (w260:T25)
                }
                frame Enabled {
                  w262 = T14[] [] items=["Main", "Init Files", "Init", "Unused", "Save As", "Start Profile", "Check Step Time", "Alarm", "Alarm Dismiss", "Run Step", "Stop Profile", "Cycle Reset", "Time Reset", "Time Reset All", "Time Set", "Tare CTs", "Save Profile", "Open Profile", "Get Profiles", "Update Screen", "Update Controls", "Save App Config", "Write Outputs", "Disable Background", "Enable Background", "Get/Release Control", "Log Fuel Change", "Fuel Change Popup", "Read Inputs", "Remote Timer Reset", "Controller Change", "Get Alarms", "Init Alarms", "Save Alarms", "Voltage Selection", "Set Watlow Temp 1", "Set Watlow Temp 2", "Get Pressure", "Write Tare Pressure", "Adjust Controls", "Reinit ADC", "Write Initial Times", "Write Pumps Present", "HMI Command", "Save Pump Times", "Check Pump Stop Time", "Save LS App Config", "Init Data File", "Reset LS Cycles", "Reset Anomalies", "Reset Opens", "Save LS Data", "Save LS Test Data", "Check Serial Numbers", "Main Tab", "Allow Data Note", "Resume Profile", "Pause Profile", "Allow Pause Note", "Clear Graph"]
                }
              }
            }
            frame 15 {
              w266 = T14[] [] items=["Main", "Init Files", "Init", "Unused", "Save As", "Start Profile", "Check Step Time", "Alarm", "Alarm Dismiss", "Run Step", "Stop Profile", "Cycle Reset", "Time Reset", "Time Reset All", "Time Set", "Tare CTs", "Save Profile", "Open Profile", "Get Profiles", "Update Screen", "Update Controls", "Save App Config", "Write Outputs", "Disable Background", "Enable Background", "Get/Release Control", "Log Fuel Change", "Fuel Change Popup", "Read Inputs", "Remote Timer Reset", "Controller Change", "Get Alarms", "Init Alarms", "Save Alarms", "Voltage Selection", "Set Watlow Temp 1", "Set Watlow Temp 2", "Get Pressure", "Write Tare Pressure", "Adjust Controls", "Reinit ADC", "Write Initial Times", "Write Pumps Present", "HMI Command", "Save Pump Times", "Check Pump Stop Time", "Save LS App Config", "Init Data File", "Reset LS Cycles", "Reset Anomalies", "Reset Opens", "Save LS Data", "Save LS Test Data", "Check Serial Numbers", "Main Tab", "Allow Data Note", "Resume Profile", "Pause Profile", "Allow Pause Note", "Clear Graph"]
            }
            frame 16 {
              n56 = disable-structure shown="Enabled" {
                disable-tunnel: [w272 w273] -> w270
                disable-tunnel: ["pb.Time Reset All" FALSE ("pb.Time Reset All")] -> w269
                frame Disabled {
                  w272 = T14[] [enum."Disable Background", enum."Time Reset All", enum."Update Controls"] items=["Main", "Init Files", "Init", "Unused", "Save As", "Start Profile", "Check Step Time", "Alarm", "Alarm Dismiss", "Run Step", "Stop Profile", "Cycle Reset", "Time Reset", "Time Reset All", "Time Set", "Tare CTs", "Save Profile", "Open Profile", "Get Profiles", "Update Screen", "Update Controls", "Save App Config", "Write Outputs", "Disable Background", "Enable Background", "Get/Release Control", "Log Fuel Change", "Fuel Change Popup", "Read Inputs", "Remote Timer Reset", "Controller Change", "Get Alarms", "Init Alarms", "Save Alarms", "Voltage Selection", "Set Watlow Temp 1", "Set Watlow Temp 2", "Get Pressure", "Write Tare Pressure", "Adjust Controls", "Reinit ADC", "Write Initial Times", "Write Pumps Present", "HMI Command", "Save Pump Times", "Check Pump Stop Time", "Save LS App Config", "Init Data File", "Reset LS Cycles", "Reset Anomalies", "Reset Opens", "Save LS Data", "Save LS Test Data", "Check Serial Numbers", "Main Tab", "Allow Data Note", "Resume Profile", "Pause Profile", "Allow Pause Note", "Clear Graph"]
                }
                frame Enabled {
                  w273 = T14[] [] items=["Main", "Init Files", "Init", "Unused", "Save As", "Start Profile", "Check Step Time", "Alarm", "Alarm Dismiss", "Run Step", "Stop Profile", "Cycle Reset", "Time Reset", "Time Reset All", "Time Set", "Tare CTs", "Save Profile", "Open Profile", "Get Profiles", "Update Screen", "Update Controls", "Save App Config", "Write Outputs", "Disable Background", "Enable Background", "Get/Release Control", "Log Fuel Change", "Fuel Change Popup", "Read Inputs", "Remote Timer Reset", "Controller Change", "Get Alarms", "Init Alarms", "Save Alarms", "Voltage Selection", "Set Watlow Temp 1", "Set Watlow Temp 2", "Get Pressure", "Write Tare Pressure", "Adjust Controls", "Reinit ADC", "Write Initial Times", "Write Pumps Present", "HMI Command", "Save Pump Times", "Check Pump Stop Time", "Save LS App Config", "Init Data File", "Reset LS Cycles", "Reset Anomalies", "Reset Opens", "Save LS Data", "Save LS Test Data", "Check Serial Numbers", "Main Tab", "Allow Data Note", "Resume Profile", "Pause Profile", "Allow Pause Note", "Clear Graph"]
                }
              }
            }
            frame 17 {
              w276 = T14[] [enum."Save App Config", enum."Write Pumps Present"] items=["Main", "Init Files", "Init", "Unused", "Save As", "Start Profile", "Check Step Time", "Alarm", "Alarm Dismiss", "Run Step", "Stop Profile", "Cycle Reset", "Time Reset", "Time Reset All", "Time Set", "Tare CTs", "Save Profile", "Open Profile", "Get Profiles", "Update Screen", "Update Controls", "Save App Config", "Write Outputs", "Disable Background", "Enable Background", "Get/Release Control", "Log Fuel Change", "Fuel Change Popup", "Read Inputs", "Remote Timer Reset", "Controller Change", "Get Alarms", "Init Alarms", "Save Alarms", "Voltage Selection", "Set Watlow Temp 1", "Set Watlow Temp 2", "Get Pressure", "Write Tare Pressure", "Adjust Controls", "Reinit ADC", "Write Initial Times", "Write Pumps Present", "HMI Command", "Save Pump Times", "Check Pump Stop Time", "Save LS App Config", "Init Data File", "Reset LS Cycles", "Reset Anomalies", "Reset Opens", "Save LS Data", "Save LS Test Data", "Check Serial Numbers", "Main Tab", "Allow Data Note", "Resume Profile", "Pause Profile", "Allow Pause Note", "Clear Graph"]
              n57 = Unbundle By Name(w277) -> ("App Config.Pumps Present"=w281:T8)
              n58 = Not Equal?(x="Pumps Present", y=w281) -> (x != y?=w278:bool)
              n59 = Bundle By Name(cluster=w280, "App Config.Pumps Present"="Pumps Present") -> (w279:T25)
            }
            frame 18 {
              w284 = T14[] [enum."Get/Release Control"] items=["Main", "Init Files", "Init", "Unused", "Save As", "Start Profile", "Check Step Time", "Alarm", "Alarm Dismiss", "Run Step", "Stop Profile", "Cycle Reset", "Time Reset", "Time Reset All", "Time Set", "Tare CTs", "Save Profile", "Open Profile", "Get Profiles", "Update Screen", "Update Controls", "Save App Config", "Write Outputs", "Disable Background", "Enable Background", "Get/Release Control", "Log Fuel Change", "Fuel Change Popup", "Read Inputs", "Remote Timer Reset", "Controller Change", "Get Alarms", "Init Alarms", "Save Alarms", "Voltage Selection", "Set Watlow Temp 1", "Set Watlow Temp 2", "Get Pressure", "Write Tare Pressure", "Adjust Controls", "Reinit ADC", "Write Initial Times", "Write Pumps Present", "HMI Command", "Save Pump Times", "Check Pump Stop Time", "Save LS App Config", "Init Data File", "Reset LS Cycles", "Reset Anomalies", "Reset Opens", "Save LS Data", "Save LS Test Data", "Check Serial Numbers", "Main Tab", "Allow Data Note", "Resume Profile", "Pause Profile", "Allow Pause Note", "Clear Graph"]
              n60 = Unbundle By Name(w285) -> ("Login"=w289:bool)
              n61 = call "App Global.vi"("Mode"=App_Global_Mode."Write Login", "Login"="Login") -> ()  [unwired: 7 in, 3 out]
              n62 = Not Equal?(x="Login", y=w289) -> (x != y?=w286:bool)
              n63 = Bundle By Name(cluster=w288, "Login"="Login") -> (w287:T25)
            }
            frame 19 {
              n64 = disable-structure shown="Enabled" {
                disable-tunnel: w294 -> [w300 w304]
                disable-tunnel: [w299 w304] -> w293
                disable-tunnel: [w298 FALSE] -> w292
                disable-tunnel: w291 -> [w297 _]
                disable-tunnel: [w296 w302] -> w290
                frame Disabled {
                  w296 = T14[] [enum."Save App Config"] items=["Main", "Init Files", "Init", "Unused", "Save As", "Start Profile", "Check Step Time", "Alarm", "Alarm Dismiss", "Run Step", "Stop Profile", "Cycle Reset", "Time Reset", "Time Reset All", "Time Set", "Tare CTs", "Save Profile", "Open Profile", "Get Profiles", "Update Screen", "Update Controls", "Save App Config", "Write Outputs", "Disable Background", "Enable Background", "Get/Release Control", "Log Fuel Change", "Fuel Change Popup", "Read Inputs", "Remote Timer Reset", "Controller Change", "Get Alarms", "Init Alarms", "Save Alarms", "Voltage Selection", "Set Watlow Temp 1", "Set Watlow Temp 2", "Get Pressure", "Write Tare Pressure", "Adjust Controls", "Reinit ADC", "Write Initial Times", "Write Pumps Present", "HMI Command", "Save Pump Times", "Check Pump Stop Time", "Save LS App Config", "Init Data File", "Reset LS Cycles", "Reset Anomalies", "Reset Opens", "Save LS Data", "Save LS Test Data", "Check Serial Numbers", "Main Tab", "Allow Data Note", "Resume Profile", "Pause Profile", "Allow Pause Note", "Clear Graph"]
                  n65 = Unbundle By Name(w297) -> ("App Config.Stagger Time (ms)"=w301:i32)
                  n66 = Not Equal?(x="Stagger Time (ms):", y=w301) -> (x != y?=w298:bool)
                  n67 = Bundle By Name(cluster=w300, "App Config.Stagger Time (ms)"="Stagger Time (ms):") -> (w299:T25)
                }
                frame Enabled {
                  w302 = T14[] [] items=["Main", "Init Files", "Init", "Unused", "Save As", "Start Profile", "Check Step Time", "Alarm", "Alarm Dismiss", "Run Step", "Stop Profile", "Cycle Reset", "Time Reset", "Time Reset All", "Time Set", "Tare CTs", "Save Profile", "Open Profile", "Get Profiles", "Update Screen", "Update Controls", "Save App Config", "Write Outputs", "Disable Background", "Enable Background", "Get/Release Control", "Log Fuel Change", "Fuel Change Popup", "Read Inputs", "Remote Timer Reset", "Controller Change", "Get Alarms", "Init Alarms", "Save Alarms", "Voltage Selection", "Set Watlow Temp 1", "Set Watlow Temp 2", "Get Pressure", "Write Tare Pressure", "Adjust Controls", "Reinit ADC", "Write Initial Times", "Write Pumps Present", "HMI Command", "Save Pump Times", "Check Pump Stop Time", "Save LS App Config", "Init Data File", "Reset LS Cycles", "Reset Anomalies", "Reset Opens", "Save LS Data", "Save LS Test Data", "Check Serial Numbers", "Main Tab", "Allow Data Note", "Resume Profile", "Pause Profile", "Allow Pause Note", "Clear Graph"]
                }
              }
            }
            frame 20 {
              n68 = disable-structure shown="Enabled" {
                disable-tunnel: w309 -> [w316 w319]
                disable-tunnel: [w315 w319] -> w308
                disable-tunnel: w307 -> [w314 _]
                disable-tunnel: [w313 w317] -> w306
                disable-tunnel: [w310 FALSE] -> w305
                frame Disabled {
                  w313 = T14[] [enum."Write Outputs"] items=["Main", "Init Files", "Init", "Unused", "Save As", "Start Profile", "Check Step Time", "Alarm", "Alarm Dismiss", "Run Step", "Stop Profile", "Cycle Reset", "Time Reset", "Time Reset All", "Time Set", "Tare CTs", "Save Profile", "Open Profile", "Get Profiles", "Update Screen", "Update Controls", "Save App Config", "Write Outputs", "Disable Background", "Enable Background", "Get/Release Control", "Log Fuel Change", "Fuel Change Popup", "Read Inputs", "Remote Timer Reset", "Controller Change", "Get Alarms", "Init Alarms", "Save Alarms", "Voltage Selection", "Set Watlow Temp 1", "Set Watlow Temp 2", "Get Pressure", "Write Tare Pressure", "Adjust Controls", "Reinit ADC", "Write Initial Times", "Write Pumps Present", "HMI Command", "Save Pump Times", "Check Pump Stop Time", "Save LS App Config", "Init Data File", "Reset LS Cycles", "Reset Anomalies", "Reset Opens", "Save LS Data", "Save LS Test Data", "Check Serial Numbers", "Main Tab", "Allow Data Note", "Resume Profile", "Pause Profile", "Allow Pause Note", "Clear Graph"]
                  n69 = Unbundle By Name(w314) -> ("Tank CMDs.Press CMD"=w312:dbl)
                  n70 = Not Equal?(x="PressureCMD", y=w312) -> (x != y?=w310:bool)
                  n71 = Bundle By Name(cluster=w316, "Tank CMDs.Press CMD"="PressureCMD") -> (w315:T25)
                }
                frame Enabled {
                  w317 = T14[] [] items=["Main", "Init Files", "Init", "Unused", "Save As", "Start Profile", "Check Step Time", "Alarm", "Alarm Dismiss", "Run Step", "Stop Profile", "Cycle Reset", "Time Reset", "Time Reset All", "Time Set", "Tare CTs", "Save Profile", "Open Profile", "Get Profiles", "Update Screen", "Update Controls", "Save App Config", "Write Outputs", "Disable Background", "Enable Background", "Get/Release Control", "Log Fuel Change", "Fuel Change Popup", "Read Inputs", "Remote Timer Reset", "Controller Change", "Get Alarms", "Init Alarms", "Save Alarms", "Voltage Selection", "Set Watlow Temp 1", "Set Watlow Temp 2", "Get Pressure", "Write Tare Pressure", "Adjust Controls", "Reinit ADC", "Write Initial Times", "Write Pumps Present", "HMI Command", "Save Pump Times", "Check Pump Stop Time", "Save LS App Config", "Init Data File", "Reset LS Cycles", "Reset Anomalies", "Reset Opens", "Save LS Data", "Save LS Test Data", "Check Serial Numbers", "Main Tab", "Allow Data Note", "Resume Profile", "Pause Profile", "Allow Pause Note", "Clear Graph"]
                }
              }
            }
            frame 21 {
              w322 = T14[] [enum."Disable Background", enum."Log Fuel Change", enum."Fuel Change Popup"] items=["Main", "Init Files", "Init", "Unused", "Save As", "Start Profile", "Check Step Time", "Alarm", "Alarm Dismiss", "Run Step", "Stop Profile", "Cycle Reset", "Time Reset", "Time Reset All", "Time Set", "Tare CTs", "Save Profile", "Open Profile", "Get Profiles", "Update Screen", "Update Controls", "Save App Config", "Write Outputs", "Disable Background", "Enable Background", "Get/Release Control", "Log Fuel Change", "Fuel Change Popup", "Read Inputs", "Remote Timer Reset", "Controller Change", "Get Alarms", "Init Alarms", "Save Alarms", "Voltage Selection", "Set Watlow Temp 1", "Set Watlow Temp 2", "Get Pressure", "Write Tare Pressure", "Adjust Controls", "Reinit ADC", "Write Initial Times", "Write Pumps Present", "HMI Command", "Save Pump Times", "Check Pump Stop Time", "Save LS App Config", "Init Data File", "Reset LS Cycles", "Reset Anomalies", "Reset Opens", "Save LS Data", "Save LS Test Data", "Check Serial Numbers", "Main Tab", "Allow Data Note", "Resume Profile", "Pause Profile", "Allow Pause Note", "Clear Graph"]
            }
            frame 22 {
              n72 = disable-structure shown="Enabled" {
                disable-tunnel: [w334 w335] -> w327
                disable-tunnel: w326 -> [w333 w337]
                disable-tunnel: [w332 w337] -> w325
                disable-tunnel: w324 -> [w331 _]
                disable-tunnel: [w328 FALSE] -> w323
                frame Disabled {
                  w334 = T14[] [enum."Save App Config"] items=["Main", "Init Files", "Init", "Unused", "Save As", "Start Profile", "Check Step Time", "Alarm", "Alarm Dismiss", "Run Step", "Stop Profile", "Cycle Reset", "Time Reset", "Time Reset All", "Time Set", "Tare CTs", "Save Profile", "Open Profile", "Get Profiles", "Update Screen", "Update Controls", "Save App Config", "Write Outputs", "Disable Background", "Enable Background", "Get/Release Control", "Log Fuel Change", "Fuel Change Popup", "Read Inputs", "Remote Timer Reset", "Controller Change", "Get Alarms", "Init Alarms", "Save Alarms", "Voltage Selection", "Set Watlow Temp 1", "Set Watlow Temp 2", "Get Pressure", "Write Tare Pressure", "Adjust Controls", "Reinit ADC", "Write Initial Times", "Write Pumps Present", "HMI Command", "Save Pump Times", "Check Pump Stop Time", "Save LS App Config", "Init Data File", "Reset LS Cycles", "Reset Anomalies", "Reset Opens", "Save LS Data", "Save LS Test Data", "Check Serial Numbers", "Main Tab", "Allow Data Note", "Resume Profile", "Pause Profile", "Allow Pause Note", "Clear Graph"]
                  n73 = Unbundle By Name(w331) -> ("App Config.Tank 1 Fuel"=w330:string)
                  n74 = Not Equal?(x=w330, y="Tank 1 Fuel Type:") -> (x != y?=w328:bool)
                  n75 = Bundle By Name(cluster=w333, "App Config.Tank 1 Fuel"="Tank 1 Fuel Type:") -> (w332:T25)
                }
                frame Enabled {
                  w335 = T14[] [] items=["Main", "Init Files", "Init", "Unused", "Save As", "Start Profile", "Check Step Time", "Alarm", "Alarm Dismiss", "Run Step", "Stop Profile", "Cycle Reset", "Time Reset", "Time Reset All", "Time Set", "Tare CTs", "Save Profile", "Open Profile", "Get Profiles", "Update Screen", "Update Controls", "Save App Config", "Write Outputs", "Disable Background", "Enable Background", "Get/Release Control", "Log Fuel Change", "Fuel Change Popup", "Read Inputs", "Remote Timer Reset", "Controller Change", "Get Alarms", "Init Alarms", "Save Alarms", "Voltage Selection", "Set Watlow Temp 1", "Set Watlow Temp 2", "Get Pressure", "Write Tare Pressure", "Adjust Controls", "Reinit ADC", "Write Initial Times", "Write Pumps Present", "HMI Command", "Save Pump Times", "Check Pump Stop Time", "Save LS App Config", "Init Data File", "Reset LS Cycles", "Reset Anomalies", "Reset Opens", "Save LS Data", "Save LS Test Data", "Check Serial Numbers", "Main Tab", "Allow Data Note", "Resume Profile", "Pause Profile", "Allow Pause Note", "Clear Graph"]
                }
              }
            }
            frame 23 {
              n76 = disable-structure shown="Enabled" {
                disable-tunnel: [w349 w350] -> w342
                disable-tunnel: w341 -> [w348 w352]
                disable-tunnel: [w347 w352] -> w340
                disable-tunnel: w339 -> [w346 _]
                disable-tunnel: [w345 FALSE] -> w338
                frame Disabled {
                  w349 = T14[] [enum."Save App Config"] items=["Main", "Init Files", "Init", "Unused", "Save As", "Start Profile", "Check Step Time", "Alarm", "Alarm Dismiss", "Run Step", "Stop Profile", "Cycle Reset", "Time Reset", "Time Reset All", "Time Set", "Tare CTs", "Save Profile", "Open Profile", "Get Profiles", "Update Screen", "Update Controls", "Save App Config", "Write Outputs", "Disable Background", "Enable Background", "Get/Release Control", "Log Fuel Change", "Fuel Change Popup", "Read Inputs", "Remote Timer Reset", "Controller Change", "Get Alarms", "Init Alarms", "Save Alarms", "Voltage Selection", "Set Watlow Temp 1", "Set Watlow Temp 2", "Get Pressure", "Write Tare Pressure", "Adjust Controls", "Reinit ADC", "Write Initial Times", "Write Pumps Present", "HMI Command", "Save Pump Times", "Check Pump Stop Time", "Save LS App Config", "Init Data File", "Reset LS Cycles", "Reset Anomalies", "Reset Opens", "Save LS Data", "Save LS Test Data", "Check Serial Numbers", "Main Tab", "Allow Data Note", "Resume Profile", "Pause Profile", "Allow Pause Note", "Clear Graph"]
                  n77 = Unbundle By Name(w346) -> ("App Config.Tank 2 Fuel"=w344:string)
                  n78 = Not Equal?(x=w344, y="Tank 2 Fuel Type:") -> (x != y?=w345:bool)
                  n79 = Bundle By Name(cluster=w348, "App Config.Tank 2 Fuel"="Tank 2 Fuel Type:") -> (w347:T25)
                }
                frame Enabled {
                  w350 = T14[] [] items=["Main", "Init Files", "Init", "Unused", "Save As", "Start Profile", "Check Step Time", "Alarm", "Alarm Dismiss", "Run Step", "Stop Profile", "Cycle Reset", "Time Reset", "Time Reset All", "Time Set", "Tare CTs", "Save Profile", "Open Profile", "Get Profiles", "Update Screen", "Update Controls", "Save App Config", "Write Outputs", "Disable Background", "Enable Background", "Get/Release Control", "Log Fuel Change", "Fuel Change Popup", "Read Inputs", "Remote Timer Reset", "Controller Change", "Get Alarms", "Init Alarms", "Save Alarms", "Voltage Selection", "Set Watlow Temp 1", "Set Watlow Temp 2", "Get Pressure", "Write Tare Pressure", "Adjust Controls", "Reinit ADC", "Write Initial Times", "Write Pumps Present", "HMI Command", "Save Pump Times", "Check Pump Stop Time", "Save LS App Config", "Init Data File", "Reset LS Cycles", "Reset Anomalies", "Reset Opens", "Save LS Data", "Save LS Test Data", "Check Serial Numbers", "Main Tab", "Allow Data Note", "Resume Profile", "Pause Profile", "Allow Pause Note", "Clear Graph"]
                }
              }
            }
            frame 24 {
              w359 = T14[] [enum."Save App Config"] items=["Main", "Init Files", "Init", "Unused", "Save As", "Start Profile", "Check Step Time", "Alarm", "Alarm Dismiss", "Run Step", "Stop Profile", "Cycle Reset", "Time Reset", "Time Reset All", "Time Set", "Tare CTs", "Save Profile", "Open Profile", "Get Profiles", "Update Screen", "Update Controls", "Save App Config", "Write Outputs", "Disable Background", "Enable Background", "Get/Release Control", "Log Fuel Change", "Fuel Change Popup", "Read Inputs", "Remote Timer Reset", "Controller Change", "Get Alarms", "Init Alarms", "Save Alarms", "Voltage Selection", "Set Watlow Temp 1", "Set Watlow Temp 2", "Get Pressure", "Write Tare Pressure", "Adjust Controls", "Reinit ADC", "Write Initial Times", "Write Pumps Present", "HMI Command", "Save Pump Times", "Check Pump Stop Time", "Save LS App Config", "Init Data File", "Reset LS Cycles", "Reset Anomalies", "Reset Opens", "Save LS Data", "Save LS Test Data", "Check Serial Numbers", "Main Tab", "Allow Data Note", "Resume Profile", "Pause Profile", "Allow Pause Note", "Clear Graph"]
              n80 = Unbundle By Name(w356) -> ("App Config.Serial Numbers"=w355:T41)
              n81 = Not Equal?(x=w355, y="Serial Numbers") -> (x != y?=w353:bool)
              n82 = Bundle By Name(cluster=w358, "App Config.Serial Numbers"="Serial Numbers") -> (w357:T25)
            }
            frame 25 {
              n83 = disable-structure shown="Enabled" {
                disable-tunnel: w364 -> [w371 w374]
                disable-tunnel: [w370 w374] -> w363
                disable-tunnel: w362 -> [w369 _]
                disable-tunnel: [w368 w372] -> w361
                disable-tunnel: [w365 FALSE] -> w360
                frame Disabled {
                  w368 = T14[] [enum."Write Pumps Present", enum."Save App Config"] items=["Main", "Init Files", "Init", "Unused", "Save As", "Start Profile", "Check Step Time", "Alarm", "Alarm Dismiss", "Run Step", "Stop Profile", "Cycle Reset", "Time Reset", "Time Reset All", "Time Set", "Tare CTs", "Save Profile", "Open Profile", "Get Profiles", "Update Screen", "Update Controls", "Save App Config", "Write Outputs", "Disable Background", "Enable Background", "Get/Release Control", "Log Fuel Change", "Fuel Change Popup", "Read Inputs", "Remote Timer Reset", "Controller Change", "Get Alarms", "Init Alarms", "Save Alarms", "Voltage Selection", "Set Watlow Temp 1", "Set Watlow Temp 2", "Get Pressure", "Write Tare Pressure", "Adjust Controls", "Reinit ADC", "Write Initial Times", "Write Pumps Present", "HMI Command", "Save Pump Times", "Check Pump Stop Time", "Save LS App Config", "Init Data File", "Reset LS Cycles", "Reset Anomalies", "Reset Opens", "Save LS Data", "Save LS Test Data", "Check Serial Numbers", "Main Tab", "Allow Data Note", "Resume Profile", "Pause Profile", "Allow Pause Note", "Clear Graph"]
                  n84 = Unbundle By Name(w369) -> ("Power Relay"=w367:T8)
                  n85 = Not Equal?(x="Power Relay", y=w367) -> (x != y?=w365:bool)
                  n86 = Bundle By Name(cluster=w371, "Power Relay"="Power Relay") -> (w370:T25)
                }
                frame Enabled {
                  w372 = T14[] [] items=["Main", "Init Files", "Init", "Unused", "Save As", "Start Profile", "Check Step Time", "Alarm", "Alarm Dismiss", "Run Step", "Stop Profile", "Cycle Reset", "Time Reset", "Time Reset All", "Time Set", "Tare CTs", "Save Profile", "Open Profile", "Get Profiles", "Update Screen", "Update Controls", "Save App Config", "Write Outputs", "Disable Background", "Enable Background", "Get/Release Control", "Log Fuel Change", "Fuel Change Popup", "Read Inputs", "Remote Timer Reset", "Controller Change", "Get Alarms", "Init Alarms", "Save Alarms", "Voltage Selection", "Set Watlow Temp 1", "Set Watlow Temp 2", "Get Pressure", "Write Tare Pressure", "Adjust Controls", "Reinit ADC", "Write Initial Times", "Write Pumps Present", "HMI Command", "Save Pump Times", "Check Pump Stop Time", "Save LS App Config", "Init Data File", "Reset LS Cycles", "Reset Anomalies", "Reset Opens", "Save LS Data", "Save LS Test Data", "Check Serial Numbers", "Main Tab", "Allow Data Note", "Resume Profile", "Pause Profile", "Allow Pause Note", "Clear Graph"]
                }
              }
            }
            frame 26 {
              n87 = disable-structure shown="Enabled" {
                disable-tunnel: [w386 w387] -> w379
                disable-tunnel: [w385 FALSE] -> w378
                disable-tunnel: w377 -> [w384 _]
                disable-tunnel: w376 -> [w383 w389]
                disable-tunnel: [w382 w389] -> w375
                frame Disabled {
                  w386 = T14[] [enum."Write Pumps Present", enum."Save App Config"] items=["Main", "Init Files", "Init", "Unused", "Save As", "Start Profile", "Check Step Time", "Alarm", "Alarm Dismiss", "Run Step", "Stop Profile", "Cycle Reset", "Time Reset", "Time Reset All", "Time Set", "Tare CTs", "Save Profile", "Open Profile", "Get Profiles", "Update Screen", "Update Controls", "Save App Config", "Write Outputs", "Disable Background", "Enable Background", "Get/Release Control", "Log Fuel Change", "Fuel Change Popup", "Read Inputs", "Remote Timer Reset", "Controller Change", "Get Alarms", "Init Alarms", "Save Alarms", "Voltage Selection", "Set Watlow Temp 1", "Set Watlow Temp 2", "Get Pressure", "Write Tare Pressure", "Adjust Controls", "Reinit ADC", "Write Initial Times", "Write Pumps Present", "HMI Command", "Save Pump Times", "Check Pump Stop Time", "Save LS App Config", "Init Data File", "Reset LS Cycles", "Reset Anomalies", "Reset Opens", "Save LS Data", "Save LS Test Data", "Check Serial Numbers", "Main Tab", "Allow Data Note", "Resume Profile", "Pause Profile", "Allow Pause Note", "Clear Graph"]
                  n88 = Unbundle By Name(w384) -> ("Ignition Relay"=w381:T8)
                  n89 = Not Equal?(x="Ignition Relay", y=w381) -> (x != y?=w385:bool)
                  n90 = Bundle By Name(cluster=w383, "Ignition Relay"="Ignition Relay") -> (w382:T25)
                }
                frame Enabled {
                  w387 = T14[] [] items=["Main", "Init Files", "Init", "Unused", "Save As", "Start Profile", "Check Step Time", "Alarm", "Alarm Dismiss", "Run Step", "Stop Profile", "Cycle Reset", "Time Reset", "Time Reset All", "Time Set", "Tare CTs", "Save Profile", "Open Profile", "Get Profiles", "Update Screen", "Update Controls", "Save App Config", "Write Outputs", "Disable Background", "Enable Background", "Get/Release Control", "Log Fuel Change", "Fuel Change Popup", "Read Inputs", "Remote Timer Reset", "Controller Change", "Get Alarms", "Init Alarms", "Save Alarms", "Voltage Selection", "Set Watlow Temp 1", "Set Watlow Temp 2", "Get Pressure", "Write Tare Pressure", "Adjust Controls", "Reinit ADC", "Write Initial Times", "Write Pumps Present", "HMI Command", "Save Pump Times", "Check Pump Stop Time", "Save LS App Config", "Init Data File", "Reset LS Cycles", "Reset Anomalies", "Reset Opens", "Save LS Data", "Save LS Test Data", "Check Serial Numbers", "Main Tab", "Allow Data Note", "Resume Profile", "Pause Profile", "Allow Pause Note", "Clear Graph"]
                }
              }
            }
            frame 27 {
              n91 = Unbundle By Name(w394) -> ("HMI.HMI Mom Buttons"=w393:T21)
              n92 = Cluster To Array(cluster=w393) -> (array=w398:bool[])
              n93 = Search 1D Array(1D array=w398, element=TRUE) -> (index of element=w396:i32)  [unwired: 1 in]
              n94 = case shown="1" w396 {
                tunnel: [w400 w401 w402 w403 w404] -> w399
                frame -1, Default {
                  w400 = T14[] [] items=["Main", "Init Files", "Init", "Unused", "Save As", "Start Profile", "Check Step Time", "Alarm", "Alarm Dismiss", "Run Step", "Stop Profile", "Cycle Reset", "Time Reset", "Time Reset All", "Time Set", "Tare CTs", "Save Profile", "Open Profile", "Get Profiles", "Update Screen", "Update Controls", "Save App Config", "Write Outputs", "Disable Background", "Enable Background", "Get/Release Control", "Log Fuel Change", "Fuel Change Popup", "Read Inputs", "Remote Timer Reset", "Controller Change", "Get Alarms", "Init Alarms", "Save Alarms", "Voltage Selection", "Set Watlow Temp 1", "Set Watlow Temp 2", "Get Pressure", "Write Tare Pressure", "Adjust Controls", "Reinit ADC", "Write Initial Times", "Write Pumps Present", "HMI Command", "Save Pump Times", "Check Pump Stop Time", "Save LS App Config", "Init Data File", "Reset LS Cycles", "Reset Anomalies", "Reset Opens", "Save LS Data", "Save LS Test Data", "Check Serial Numbers", "Main Tab", "Allow Data Note", "Resume Profile", "Pause Profile", "Allow Pause Note", "Clear Graph"]
                }
                frame 0 {
                  w401 = T14[] [enum."Stop Profile"] items=["Main", "Init Files", "Init", "Unused", "Save As", "Start Profile", "Check Step Time", "Alarm", "Alarm Dismiss", "Run Step", "Stop Profile", "Cycle Reset", "Time Reset", "Time Reset All", "Time Set", "Tare CTs", "Save Profile", "Open Profile", "Get Profiles", "Update Screen", "Update Controls", "Save App Config", "Write Outputs", "Disable Background", "Enable Background", "Get/Release Control", "Log Fuel Change", "Fuel Change Popup", "Read Inputs", "Remote Timer Reset", "Controller Change", "Get Alarms", "Init Alarms", "Save Alarms", "Voltage Selection", "Set Watlow Temp 1", "Set Watlow Temp 2", "Get Pressure", "Write Tare Pressure", "Adjust Controls", "Reinit ADC", "Write Initial Times", "Write Pumps Present", "HMI Command", "Save Pump Times", "Check Pump Stop Time", "Save LS App Config", "Init Data File", "Reset LS Cycles", "Reset Anomalies", "Reset Opens", "Save LS Data", "Save LS Test Data", "Check Serial Numbers", "Main Tab", "Allow Data Note", "Resume Profile", "Pause Profile", "Allow Pause Note", "Clear Graph"]
                }
                frame 1 {
                  w402 = T14[] [enum."Remote Timer Reset"] items=["Main", "Init Files", "Init", "Unused", "Save As", "Start Profile", "Check Step Time", "Alarm", "Alarm Dismiss", "Run Step", "Stop Profile", "Cycle Reset", "Time Reset", "Time Reset All", "Time Set", "Tare CTs", "Save Profile", "Open Profile", "Get Profiles", "Update Screen", "Update Controls", "Save App Config", "Write Outputs", "Disable Background", "Enable Background", "Get/Release Control", "Log Fuel Change", "Fuel Change Popup", "Read Inputs", "Remote Timer Reset", "Controller Change", "Get Alarms", "Init Alarms", "Save Alarms", "Voltage Selection", "Set Watlow Temp 1", "Set Watlow Temp 2", "Get Pressure", "Write Tare Pressure", "Adjust Controls", "Reinit ADC", "Write Initial Times", "Write Pumps Present", "HMI Command", "Save Pump Times", "Check Pump Stop Time", "Save LS App Config", "Init Data File", "Reset LS Cycles", "Reset Anomalies", "Reset Opens", "Save LS Data", "Save LS Test Data", "Check Serial Numbers", "Main Tab", "Allow Data Note", "Resume Profile", "Pause Profile", "Allow Pause Note", "Clear Graph"]
                }
                frame 2 {
                  w403 = T14[] [enum."Log Fuel Change"] items=["Main", "Init Files", "Init", "Unused", "Save As", "Start Profile", "Check Step Time", "Alarm", "Alarm Dismiss", "Run Step", "Stop Profile", "Cycle Reset", "Time Reset", "Time Reset All", "Time Set", "Tare CTs", "Save Profile", "Open Profile", "Get Profiles", "Update Screen", "Update Controls", "Save App Config", "Write Outputs", "Disable Background", "Enable Background", "Get/Release Control", "Log Fuel Change", "Fuel Change Popup", "Read Inputs", "Remote Timer Reset", "Controller Change", "Get Alarms", "Init Alarms", "Save Alarms", "Voltage Selection", "Set Watlow Temp 1", "Set Watlow Temp 2", "Get Pressure", "Write Tare Pressure", "Adjust Controls", "Reinit ADC", "Write Initial Times", "Write Pumps Present", "HMI Command", "Save Pump Times", "Check Pump Stop Time", "Save LS App Config", "Init Data File", "Reset LS Cycles", "Reset Anomalies", "Reset Opens", "Save LS Data", "Save LS Test Data", "Check Serial Numbers", "Main Tab", "Allow Data Note", "Resume Profile", "Pause Profile", "Allow Pause Note", "Clear Graph"]
                }
                frame 3 {
                  w404 = T14[] [enum."Alarm Dismiss"] items=["Main", "Init Files", "Init", "Unused", "Save As", "Start Profile", "Check Step Time", "Alarm", "Alarm Dismiss", "Run Step", "Stop Profile", "Cycle Reset", "Time Reset", "Time Reset All", "Time Set", "Tare CTs", "Save Profile", "Open Profile", "Get Profiles", "Update Screen", "Update Controls", "Save App Config", "Write Outputs", "Disable Background", "Enable Background", "Get/Release Control", "Log Fuel Change", "Fuel Change Popup", "Read Inputs", "Remote Timer Reset", "Controller Change", "Get Alarms", "Init Alarms", "Save Alarms", "Voltage Selection", "Set Watlow Temp 1", "Set Watlow Temp 2", "Get Pressure", "Write Tare Pressure", "Adjust Controls", "Reinit ADC", "Write Initial Times", "Write Pumps Present", "HMI Command", "Save Pump Times", "Check Pump Stop Time", "Save LS App Config", "Init Data File", "Reset LS Cycles", "Reset Anomalies", "Reset Opens", "Save LS Data", "Save LS Test Data", "Check Serial Numbers", "Main Tab", "Allow Data Note", "Resume Profile", "Pause Profile", "Allow Pause Note", "Clear Graph"]
                }
              }
              n95 = Greater Or Equal To 0?(x=w396) -> (x >= 0?=w395:bool)
              n96 = Bundle By Name(cluster=w392, "HMI.HMI Mom Buttons"=T21 {"Stop"=FALSE, "Reset Timers"=FALSE, "Log Fuel Change"=FALSE, "Alarm Dismiss"=FALSE}) -> (w391:T25)
            }
            frame 28 {
              n97 = disable-structure shown="Enabled" {
                disable-tunnel: [w416 w417] -> w409
                disable-tunnel: [w415 FALSE] -> w408
                disable-tunnel: w407 -> [w414 _]
                disable-tunnel: w406 -> [w413 w419]
                disable-tunnel: [w412 w419] -> w405
                frame Disabled {
                  w416 = T14[] [enum."Save Alarms"] items=["Main", "Init Files", "Init", "Unused", "Save As", "Start Profile", "Check Step Time", "Alarm", "Alarm Dismiss", "Run Step", "Stop Profile", "Cycle Reset", "Time Reset", "Time Reset All", "Time Set", "Tare CTs", "Save Profile", "Open Profile", "Get Profiles", "Update Screen", "Update Controls", "Save App Config", "Write Outputs", "Disable Background", "Enable Background", "Get/Release Control", "Log Fuel Change", "Fuel Change Popup", "Read Inputs", "Remote Timer Reset", "Controller Change", "Get Alarms", "Init Alarms", "Save Alarms", "Voltage Selection", "Set Watlow Temp 1", "Set Watlow Temp 2", "Get Pressure", "Write Tare Pressure", "Adjust Controls", "Reinit ADC", "Write Initial Times", "Write Pumps Present", "HMI Command", "Save Pump Times", "Check Pump Stop Time", "Save LS App Config", "Init Data File", "Reset LS Cycles", "Reset Anomalies", "Reset Opens", "Save LS Data", "Save LS Test Data", "Check Serial Numbers", "Main Tab", "Allow Data Note", "Resume Profile", "Pause Profile", "Allow Pause Note", "Clear Graph"]
                  n98 = Unbundle By Name(w414) -> ("Alarm Config"=w411:T10)
                  n99 = Not Equal?(x="Alarm Config", y=w411) -> (x != y?=w415:bool)
                  n100 = Bundle By Name(cluster=w413, "Alarm Config"="Alarm Config") -> (w412:T25)
                }
                frame Enabled {
                  w417 = T14[] [] items=["Main", "Init Files", "Init", "Unused", "Save As", "Start Profile", "Check Step Time", "Alarm", "Alarm Dismiss", "Run Step", "Stop Profile", "Cycle Reset", "Time Reset", "Time Reset All", "Time Set", "Tare CTs", "Save Profile", "Open Profile", "Get Profiles", "Update Screen", "Update Controls", "Save App Config", "Write Outputs", "Disable Background", "Enable Background", "Get/Release Control", "Log Fuel Change", "Fuel Change Popup", "Read Inputs", "Remote Timer Reset", "Controller Change", "Get Alarms", "Init Alarms", "Save Alarms", "Voltage Selection", "Set Watlow Temp 1", "Set Watlow Temp 2", "Get Pressure", "Write Tare Pressure", "Adjust Controls", "Reinit ADC", "Write Initial Times", "Write Pumps Present", "HMI Command", "Save Pump Times", "Check Pump Stop Time", "Save LS App Config", "Init Data File", "Reset LS Cycles", "Reset Anomalies", "Reset Opens", "Save LS Data", "Save LS Test Data", "Check Serial Numbers", "Main Tab", "Allow Data Note", "Resume Profile", "Pause Profile", "Allow Pause Note", "Clear Graph"]
                }
              }
            }
            frame 29 {
              n101 = disable-structure shown="Enabled" {
                disable-tunnel: [w431 w432] -> w424
                disable-tunnel: w423 -> [w430 _]
                disable-tunnel: w422 -> [w429 w434]
                disable-tunnel: [w428 w434] -> w421
                disable-tunnel: [w425 FALSE] -> w420
                frame Disabled {
                  w431 = T14[] [enum."Set Watlow Temp 1", enum."Save App Config"] items=["Main", "Init Files", "Init", "Unused", "Save As", "Start Profile", "Check Step Time", "Alarm", "Alarm Dismiss", "Run Step", "Stop Profile", "Cycle Reset", "Time Reset", "Time Reset All", "Time Set", "Tare CTs", "Save Profile", "Open Profile", "Get Profiles", "Update Screen", "Update Controls", "Save App Config", "Write Outputs", "Disable Background", "Enable Background", "Get/Release Control", "Log Fuel Change", "Fuel Change Popup", "Read Inputs", "Remote Timer Reset", "Controller Change", "Get Alarms", "Init Alarms", "Save Alarms", "Voltage Selection", "Set Watlow Temp 1", "Set Watlow Temp 2", "Get Pressure", "Write Tare Pressure", "Adjust Controls", "Reinit ADC", "Write Initial Times", "Write Pumps Present", "HMI Command", "Save Pump Times", "Check Pump Stop Time", "Save LS App Config", "Init Data File", "Reset LS Cycles", "Reset Anomalies", "Reset Opens", "Save LS Data", "Save LS Test Data", "Check Serial Numbers", "Main Tab", "Allow Data Note", "Resume Profile", "Pause Profile", "Allow Pause Note", "Clear Graph"]
                  n102 = Unbundle By Name(w430) -> ("Tank CMDs.Temp 1 CMD"=w427:dbl)
                  n103 = Not Equal?(x="Tank 1 Temp Cmd:", y=w427) -> (x != y?=w425:bool)
                  n104 = Bundle By Name(cluster=w429, "Tank CMDs.Temp 1 CMD"="Tank 1 Temp Cmd:", "App Config.Temp 1"="Tank 1 Temp Cmd:") -> (w428:T25)
                }
                frame Enabled {
                  w432 = T14[] [] items=["Main", "Init Files", "Init", "Unused", "Save As", "Start Profile", "Check Step Time", "Alarm", "Alarm Dismiss", "Run Step", "Stop Profile", "Cycle Reset", "Time Reset", "Time Reset All", "Time Set", "Tare CTs", "Save Profile", "Open Profile", "Get Profiles", "Update Screen", "Update Controls", "Save App Config", "Write Outputs", "Disable Background", "Enable Background", "Get/Release Control", "Log Fuel Change", "Fuel Change Popup", "Read Inputs", "Remote Timer Reset", "Controller Change", "Get Alarms", "Init Alarms", "Save Alarms", "Voltage Selection", "Set Watlow Temp 1", "Set Watlow Temp 2", "Get Pressure", "Write Tare Pressure", "Adjust Controls", "Reinit ADC", "Write Initial Times", "Write Pumps Present", "HMI Command", "Save Pump Times", "Check Pump Stop Time", "Save LS App Config", "Init Data File", "Reset LS Cycles", "Reset Anomalies", "Reset Opens", "Save LS Data", "Save LS Test Data", "Check Serial Numbers", "Main Tab", "Allow Data Note", "Resume Profile", "Pause Profile", "Allow Pause Note", "Clear Graph"]
                }
              }
            }
            frame 30 {
              n105 = disable-structure shown="Enabled" {
                disable-tunnel: [w446 w447] -> w439
                disable-tunnel: w438 -> [w445 _]
                disable-tunnel: w437 -> [w444 w449]
                disable-tunnel: [w443 w449] -> w436
                disable-tunnel: [w440 FALSE] -> w435
                frame Disabled {
                  w446 = T14[] [enum."Set Watlow Temp 2", enum."Save App Config"] items=["Main", "Init Files", "Init", "Unused", "Save As", "Start Profile", "Check Step Time", "Alarm", "Alarm Dismiss", "Run Step", "Stop Profile", "Cycle Reset", "Time Reset", "Time Reset All", "Time Set", "Tare CTs", "Save Profile", "Open Profile", "Get Profiles", "Update Screen", "Update Controls", "Save App Config", "Write Outputs", "Disable Background", "Enable Background", "Get/Release Control", "Log Fuel Change", "Fuel Change Popup", "Read Inputs", "Remote Timer Reset", "Controller Change", "Get Alarms", "Init Alarms", "Save Alarms", "Voltage Selection", "Set Watlow Temp 1", "Set Watlow Temp 2", "Get Pressure", "Write Tare Pressure", "Adjust Controls", "Reinit ADC", "Write Initial Times", "Write Pumps Present", "HMI Command", "Save Pump Times", "Check Pump Stop Time", "Save LS App Config", "Init Data File", "Reset LS Cycles", "Reset Anomalies", "Reset Opens", "Save LS Data", "Save LS Test Data", "Check Serial Numbers", "Main Tab", "Allow Data Note", "Resume Profile", "Pause Profile", "Allow Pause Note", "Clear Graph"]
                  n106 = Unbundle By Name(w445) -> ("Tank CMDs.Temp 2 CMD"=w442:dbl)
                  n107 = Not Equal?(x="Tank 2 Temp Cmd:", y=w442) -> (x != y?=w440:bool)
                  n108 = Bundle By Name(cluster=w444, "Tank CMDs.Temp 2 CMD"="Tank 2 Temp Cmd:", "App Config.Temp 2"="Tank 2 Temp Cmd:") -> (w443:T25)
                }
                frame Enabled {
                  w447 = T14[] [] items=["Main", "Init Files", "Init", "Unused", "Save As", "Start Profile", "Check Step Time", "Alarm", "Alarm Dismiss", "Run Step", "Stop Profile", "Cycle Reset", "Time Reset", "Time Reset All", "Time Set", "Tare CTs", "Save Profile", "Open Profile", "Get Profiles", "Update Screen", "Update Controls", "Save App Config", "Write Outputs", "Disable Background", "Enable Background", "Get/Release Control", "Log Fuel Change", "Fuel Change Popup", "Read Inputs", "Remote Timer Reset", "Controller Change", "Get Alarms", "Init Alarms", "Save Alarms", "Voltage Selection", "Set Watlow Temp 1", "Set Watlow Temp 2", "Get Pressure", "Write Tare Pressure", "Adjust Controls", "Reinit ADC", "Write Initial Times", "Write Pumps Present", "HMI Command", "Save Pump Times", "Check Pump Stop Time", "Save LS App Config", "Init Data File", "Reset LS Cycles", "Reset Anomalies", "Reset Opens", "Save LS Data", "Save LS Test Data", "Check Serial Numbers", "Main Tab", "Allow Data Note", "Resume Profile", "Pause Profile", "Allow Pause Note", "Clear Graph"]
                }
              }
            }
            frame 31 {
              w452 = T14[] [enum."Alarm Dismiss"] items=["Main", "Init Files", "Init", "Unused", "Save As", "Start Profile", "Check Step Time", "Alarm", "Alarm Dismiss", "Run Step", "Stop Profile", "Cycle Reset", "Time Reset", "Time Reset All", "Time Set", "Tare CTs", "Save Profile", "Open Profile", "Get Profiles", "Update Screen", "Update Controls", "Save App Config", "Write Outputs", "Disable Background", "Enable Background", "Get/Release Control", "Log Fuel Change", "Fuel Change Popup", "Read Inputs", "Remote Timer Reset", "Controller Change", "Get Alarms", "Init Alarms", "Save Alarms", "Voltage Selection", "Set Watlow Temp 1", "Set Watlow Temp 2", "Get Pressure", "Write Tare Pressure", "Adjust Controls", "Reinit ADC", "Write Initial Times", "Write Pumps Present", "HMI Command", "Save Pump Times", "Check Pump Stop Time", "Save LS App Config", "Init Data File", "Reset LS Cycles", "Reset Anomalies", "Reset Opens", "Save LS Data", "Save LS Test Data", "Check Serial Numbers", "Main Tab", "Allow Data Note", "Resume Profile", "Pause Profile", "Allow Pause Note", "Clear Graph"]
            }
            frame 32 {
              w455 = T14[] [enum."Get Pressure"] items=["Main", "Init Files", "Init", "Unused", "Save As", "Start Profile", "Check Step Time", "Alarm", "Alarm Dismiss", "Run Step", "Stop Profile", "Cycle Reset", "Time Reset", "Time Reset All", "Time Set", "Tare CTs", "Save Profile", "Open Profile", "Get Profiles", "Update Screen", "Update Controls", "Save App Config", "Write Outputs", "Disable Background", "Enable Background", "Get/Release Control", "Log Fuel Change", "Fuel Change Popup", "Read Inputs", "Remote Timer Reset", "Controller Change", "Get Alarms", "Init Alarms", "Save Alarms", "Voltage Selection", "Set Watlow Temp 1", "Set Watlow Temp 2", "Get Pressure", "Write Tare Pressure", "Adjust Controls", "Reinit ADC", "Write Initial Times", "Write Pumps Present", "HMI Command", "Save Pump Times", "Check Pump Stop Time", "Save LS App Config", "Init Data File", "Reset LS Cycles", "Reset Anomalies", "Reset Opens", "Save LS Data", "Save LS Test Data", "Check Serial Numbers", "Main Tab", "Allow Data Note", "Resume Profile", "Pause Profile", "Allow Pause Note", "Clear Graph"]
              n109 = disable-structure shown="Enabled" {
                disable-tunnel: ["pb.Tare Pressure" FALSE ("pb.Tare Pressure")] -> w453
                frame Disabled {
                }
                frame Enabled {
                }
              }
            }
            frame 33 {
              n110 = disable-structure shown="Enabled" {
                disable-tunnel: w462 -> [w469 _]
                disable-tunnel: w461 -> [w468 w472]
                disable-tunnel: [w467 w472] -> w460
                disable-tunnel: [w465 FALSE] -> w459
                disable-tunnel: [w464 w470] -> w458
                frame Disabled {
                  w464 = T14[] [enum."Save App Config"] items=["Main", "Init Files", "Init", "Unused", "Save As", "Start Profile", "Check Step Time", "Alarm", "Alarm Dismiss", "Run Step", "Stop Profile", "Cycle Reset", "Time Reset", "Time Reset All", "Time Set", "Tare CTs", "Save Profile", "Open Profile", "Get Profiles", "Update Screen", "Update Controls", "Save App Config", "Write Outputs", "Disable Background", "Enable Background", "Get/Release Control", "Log Fuel Change", "Fuel Change Popup", "Read Inputs", "Remote Timer Reset", "Controller Change", "Get Alarms", "Init Alarms", "Save Alarms", "Voltage Selection", "Set Watlow Temp 1", "Set Watlow Temp 2", "Get Pressure", "Write Tare Pressure", "Adjust Controls", "Reinit ADC", "Write Initial Times", "Write Pumps Present", "HMI Command", "Save Pump Times", "Check Pump Stop Time", "Save LS App Config", "Init Data File", "Reset LS Cycles", "Reset Anomalies", "Reset Opens", "Save LS Data", "Save LS Test Data", "Check Serial Numbers", "Main Tab", "Allow Data Note", "Resume Profile", "Pause Profile", "Allow Pause Note", "Clear Graph"]
                  n111 = Unbundle By Name(w469) -> ("App Config.V_Run PI?"=w466:bool)
                  n112 = Not Equal?(x="Closed Loop Voltage", y=w466) -> (x != y?=w465:bool)
                  n113 = Bundle By Name(cluster=w468, "App Config.V_Run PI?"="Closed Loop Voltage") -> (w467:T25)
                }
                frame Enabled {
                  w470 = T14[] [] items=["Main", "Init Files", "Init", "Unused", "Save As", "Start Profile", "Check Step Time", "Alarm", "Alarm Dismiss", "Run Step", "Stop Profile", "Cycle Reset", "Time Reset", "Time Reset All", "Time Set", "Tare CTs", "Save Profile", "Open Profile", "Get Profiles", "Update Screen", "Update Controls", "Save App Config", "Write Outputs", "Disable Background", "Enable Background", "Get/Release Control", "Log Fuel Change", "Fuel Change Popup", "Read Inputs", "Remote Timer Reset", "Controller Change", "Get Alarms", "Init Alarms", "Save Alarms", "Voltage Selection", "Set Watlow Temp 1", "Set Watlow Temp 2", "Get Pressure", "Write Tare Pressure", "Adjust Controls", "Reinit ADC", "Write Initial Times", "Write Pumps Present", "HMI Command", "Save Pump Times", "Check Pump Stop Time", "Save LS App Config", "Init Data File", "Reset LS Cycles", "Reset Anomalies", "Reset Opens", "Save LS Data", "Save LS Test Data", "Check Serial Numbers", "Main Tab", "Allow Data Note", "Resume Profile", "Pause Profile", "Allow Pause Note", "Clear Graph"]
                }
              }
            }
            frame 34 {
              n114 = disable-structure shown="Enabled" {
                disable-tunnel: w477 -> [w486 _]
                disable-tunnel: w476 -> [w485 w489]
                disable-tunnel: [w484 w489] -> w475
                disable-tunnel: [w482 w487] -> w474
                disable-tunnel: [w478 FALSE] -> w473
                frame Disabled {
                  w482 = T14[] [enum."Adjust Controls", enum."Save App Config"] items=["Main", "Init Files", "Init", "Unused", "Save As", "Start Profile", "Check Step Time", "Alarm", "Alarm Dismiss", "Run Step", "Stop Profile", "Cycle Reset", "Time Reset", "Time Reset All", "Time Set", "Tare CTs", "Save Profile", "Open Profile", "Get Profiles", "Update Screen", "Update Controls", "Save App Config", "Write Outputs", "Disable Background", "Enable Background", "Get/Release Control", "Log Fuel Change", "Fuel Change Popup", "Read Inputs", "Remote Timer Reset", "Controller Change", "Get Alarms", "Init Alarms", "Save Alarms", "Voltage Selection", "Set Watlow Temp 1", "Set Watlow Temp 2", "Get Pressure", "Write Tare Pressure", "Adjust Controls", "Reinit ADC", "Write Initial Times", "Write Pumps Present", "HMI Command", "Save Pump Times", "Check Pump Stop Time", "Save LS App Config", "Init Data File", "Reset LS Cycles", "Reset Anomalies", "Reset Opens", "Save LS Data", "Save LS Test Data", "Check Serial Numbers", "Main Tab", "Allow Data Note", "Resume Profile", "Pause Profile", "Allow Pause Note", "Clear Graph"]
                  n115 = Unbundle By Name(w486) -> ("App Config.Voltage Limits"=w483:T42)
                  n116 = Not Equal?(x="Voltage Limits", y=w483) -> (x != y?=w479:cluster{bool, bool, bool})
                  n117 = Cluster To Array(cluster=w479) -> (array=w480:bool[])
                  n118 = Or Array Elements(Boolean array=w480) -> (logical OR=w478:bool)
                  n119 = Bundle By Name(cluster=w485, "App Config.Voltage Limits"="Voltage Limits") -> (w484:T25)
                }
                frame Enabled {
                  w487 = T14[] [] items=["Main", "Init Files", "Init", "Unused", "Save As", "Start Profile", "Check Step Time", "Alarm", "Alarm Dismiss", "Run Step", "Stop Profile", "Cycle Reset", "Time Reset", "Time Reset All", "Time Set", "Tare CTs", "Save Profile", "Open Profile", "Get Profiles", "Update Screen", "Update Controls", "Save App Config", "Write Outputs", "Disable Background", "Enable Background", "Get/Release Control", "Log Fuel Change", "Fuel Change Popup", "Read Inputs", "Remote Timer Reset", "Controller Change", "Get Alarms", "Init Alarms", "Save Alarms", "Voltage Selection", "Set Watlow Temp 1", "Set Watlow Temp 2", "Get Pressure", "Write Tare Pressure", "Adjust Controls", "Reinit ADC", "Write Initial Times", "Write Pumps Present", "HMI Command", "Save Pump Times", "Check Pump Stop Time", "Save LS App Config", "Init Data File", "Reset LS Cycles", "Reset Anomalies", "Reset Opens", "Save LS Data", "Save LS Test Data", "Check Serial Numbers", "Main Tab", "Allow Data Note", "Resume Profile", "Pause Profile", "Allow Pause Note", "Clear Graph"]
                }
              }
            }
            frame 35 {
              n120 = disable-structure shown="Enabled" {
                disable-tunnel: w494 -> [w503 _]
                disable-tunnel: w493 -> [w502 w506]
                disable-tunnel: [w501 w506] -> w492
                disable-tunnel: [w496 FALSE] -> w491
                disable-tunnel: [w495 w504] -> w490
                frame Disabled {
                  w495 = T14[] [enum."Adjust Controls", enum."Save App Config"] items=["Main", "Init Files", "Init", "Unused", "Save As", "Start Profile", "Check Step Time", "Alarm", "Alarm Dismiss", "Run Step", "Stop Profile", "Cycle Reset", "Time Reset", "Time Reset All", "Time Set", "Tare CTs", "Save Profile", "Open Profile", "Get Profiles", "Update Screen", "Update Controls", "Save App Config", "Write Outputs", "Disable Background", "Enable Background", "Get/Release Control", "Log Fuel Change", "Fuel Change Popup", "Read Inputs", "Remote Timer Reset", "Controller Change", "Get Alarms", "Init Alarms", "Save Alarms", "Voltage Selection", "Set Watlow Temp 1", "Set Watlow Temp 2", "Get Pressure", "Write Tare Pressure", "Adjust Controls", "Reinit ADC", "Write Initial Times", "Write Pumps Present", "HMI Command", "Save Pump Times", "Check Pump Stop Time", "Save LS App Config", "Init Data File", "Reset LS Cycles", "Reset Anomalies", "Reset Opens", "Save LS Data", "Save LS Test Data", "Check Serial Numbers", "Main Tab", "Allow Data Note", "Resume Profile", "Pause Profile", "Allow Pause Note", "Clear Graph"]
                  n121 = Unbundle By Name(w503) -> ("App Config.Voltage Far PI"=w500:T43)
                  n122 = Not Equal?(x="Far PI", y=w500) -> (x != y?=w497:cluster{bool, bool, bool})
                  n123 = Cluster To Array(cluster=w497) -> (array=w498:bool[])
                  n124 = Or Array Elements(Boolean array=w498) -> (logical OR=w496:bool)
                  n125 = Bundle By Name(cluster=w502, "App Config.Voltage Far PI"="Far PI") -> (w501:T25)
                }
                frame Enabled {
                  w504 = T14[] [] items=["Main", "Init Files", "Init", "Unused", "Save As", "Start Profile", "Check Step Time", "Alarm", "Alarm Dismiss", "Run Step", "Stop Profile", "Cycle Reset", "Time Reset", "Time Reset All", "Time Set", "Tare CTs", "Save Profile", "Open Profile", "Get Profiles", "Update Screen", "Update Controls", "Save App Config", "Write Outputs", "Disable Background", "Enable Background", "Get/Release Control", "Log Fuel Change", "Fuel Change Popup", "Read Inputs", "Remote Timer Reset", "Controller Change", "Get Alarms", "Init Alarms", "Save Alarms", "Voltage Selection", "Set Watlow Temp 1", "Set Watlow Temp 2", "Get Pressure", "Write Tare Pressure", "Adjust Controls", "Reinit ADC", "Write Initial Times", "Write Pumps Present", "HMI Command", "Save Pump Times", "Check Pump Stop Time", "Save LS App Config", "Init Data File", "Reset LS Cycles", "Reset Anomalies", "Reset Opens", "Save LS Data", "Save LS Test Data", "Check Serial Numbers", "Main Tab", "Allow Data Note", "Resume Profile", "Pause Profile", "Allow Pause Note", "Clear Graph"]
                }
              }
            }
            frame 36 {
              n126 = disable-structure shown="Enabled" {
                disable-tunnel: w511 -> [w520 _]
                disable-tunnel: w510 -> [w519 w523]
                disable-tunnel: [w518 w523] -> w509
                disable-tunnel: [w514 FALSE] -> w508
                disable-tunnel: [w512 w521] -> w507
                frame Disabled {
                  w512 = T14[] [enum."Adjust Controls", enum."Save App Config"] items=["Main", "Init Files", "Init", "Unused", "Save As", "Start Profile", "Check Step Time", "Alarm", "Alarm Dismiss", "Run Step", "Stop Profile", "Cycle Reset", "Time Reset", "Time Reset All", "Time Set", "Tare CTs", "Save Profile", "Open Profile", "Get Profiles", "Update Screen", "Update Controls", "Save App Config", "Write Outputs", "Disable Background", "Enable Background", "Get/Release Control", "Log Fuel Change", "Fuel Change Popup", "Read Inputs", "Remote Timer Reset", "Controller Change", "Get Alarms", "Init Alarms", "Save Alarms", "Voltage Selection", "Set Watlow Temp 1", "Set Watlow Temp 2", "Get Pressure", "Write Tare Pressure", "Adjust Controls", "Reinit ADC", "Write Initial Times", "Write Pumps Present", "HMI Command", "Save Pump Times", "Check Pump Stop Time", "Save LS App Config", "Init Data File", "Reset LS Cycles", "Reset Anomalies", "Reset Opens", "Save LS Data", "Save LS Test Data", "Check Serial Numbers", "Main Tab", "Allow Data Note", "Resume Profile", "Pause Profile", "Allow Pause Note", "Clear Graph"]
                  n127 = Unbundle By Name(w520) -> ("App Config.Voltage Mid PI"=w517:T44)
                  n128 = Not Equal?(x="Mid PI", y=w517) -> (x != y?=w515:cluster{bool, bool, bool})
                  n129 = Cluster To Array(cluster=w515) -> (array=w516:bool[])
                  n130 = Or Array Elements(Boolean array=w516) -> (logical OR=w514:bool)
                  n131 = Bundle By Name(cluster=w519, "App Config.Voltage Mid PI"="Mid PI") -> (w518:T25)
                }
                frame Enabled {
                  w521 = T14[] [] items=["Main", "Init Files", "Init", "Unused", "Save As", "Start Profile", "Check Step Time", "Alarm", "Alarm Dismiss", "Run Step", "Stop Profile", "Cycle Reset", "Time Reset", "Time Reset All", "Time Set", "Tare CTs", "Save Profile", "Open Profile", "Get Profiles", "Update Screen", "Update Controls", "Save App Config", "Write Outputs", "Disable Background", "Enable Background", "Get/Release Control", "Log Fuel Change", "Fuel Change Popup", "Read Inputs", "Remote Timer Reset", "Controller Change", "Get Alarms", "Init Alarms", "Save Alarms", "Voltage Selection", "Set Watlow Temp 1", "Set Watlow Temp 2", "Get Pressure", "Write Tare Pressure", "Adjust Controls", "Reinit ADC", "Write Initial Times", "Write Pumps Present", "HMI Command", "Save Pump Times", "Check Pump Stop Time", "Save LS App Config", "Init Data File", "Reset LS Cycles", "Reset Anomalies", "Reset Opens", "Save LS Data", "Save LS Test Data", "Check Serial Numbers", "Main Tab", "Allow Data Note", "Resume Profile", "Pause Profile", "Allow Pause Note", "Clear Graph"]
                }
              }
            }
            frame 37 {
              n132 = disable-structure shown="Enabled" {
                disable-tunnel: w528 -> [w537 _]
                disable-tunnel: w527 -> [w536 w540]
                disable-tunnel: [w535 w540] -> w526
                disable-tunnel: [w531 FALSE] -> w525
                disable-tunnel: [w529 w538] -> w524
                frame Disabled {
                  w529 = T14[] [enum."Adjust Controls", enum."Save App Config"] items=["Main", "Init Files", "Init", "Unused", "Save As", "Start Profile", "Check Step Time", "Alarm", "Alarm Dismiss", "Run Step", "Stop Profile", "Cycle Reset", "Time Reset", "Time Reset All", "Time Set", "Tare CTs", "Save Profile", "Open Profile", "Get Profiles", "Update Screen", "Update Controls", "Save App Config", "Write Outputs", "Disable Background", "Enable Background", "Get/Release Control", "Log Fuel Change", "Fuel Change Popup", "Read Inputs", "Remote Timer Reset", "Controller Change", "Get Alarms", "Init Alarms", "Save Alarms", "Voltage Selection", "Set Watlow Temp 1", "Set Watlow Temp 2", "Get Pressure", "Write Tare Pressure", "Adjust Controls", "Reinit ADC", "Write Initial Times", "Write Pumps Present", "HMI Command", "Save Pump Times", "Check Pump Stop Time", "Save LS App Config", "Init Data File", "Reset LS Cycles", "Reset Anomalies", "Reset Opens", "Save LS Data", "Save LS Test Data", "Check Serial Numbers", "Main Tab", "Allow Data Note", "Resume Profile", "Pause Profile", "Allow Pause Note", "Clear Graph"]
                  n133 = Unbundle By Name(w537) -> ("App Config.Voltage Close PI"=w534:T45)
                  n134 = Not Equal?(x="Close PI", y=w534) -> (x != y?=w532:cluster{bool, bool, bool})
                  n135 = Cluster To Array(cluster=w532) -> (array=w533:bool[])
                  n136 = Or Array Elements(Boolean array=w533) -> (logical OR=w531:bool)
                  n137 = Bundle By Name(cluster=w536, "App Config.Voltage Close PI"="Close PI") -> (w535:T25)
                }
                frame Enabled {
                  w538 = T14[] [] items=["Main", "Init Files", "Init", "Unused", "Save As", "Start Profile", "Check Step Time", "Alarm", "Alarm Dismiss", "Run Step", "Stop Profile", "Cycle Reset", "Time Reset", "Time Reset All", "Time Set", "Tare CTs", "Save Profile", "Open Profile", "Get Profiles", "Update Screen", "Update Controls", "Save App Config", "Write Outputs", "Disable Background", "Enable Background", "Get/Release Control", "Log Fuel Change", "Fuel Change Popup", "Read Inputs", "Remote Timer Reset", "Controller Change", "Get Alarms", "Init Alarms", "Save Alarms", "Voltage Selection", "Set Watlow Temp 1", "Set Watlow Temp 2", "Get Pressure", "Write Tare Pressure", "Adjust Controls", "Reinit ADC", "Write Initial Times", "Write Pumps Present", "HMI Command", "Save Pump Times", "Check Pump Stop Time", "Save LS App Config", "Init Data File", "Reset LS Cycles", "Reset Anomalies", "Reset Opens", "Save LS Data", "Save LS Test Data", "Check Serial Numbers", "Main Tab", "Allow Data Note", "Resume Profile", "Pause Profile", "Allow Pause Note", "Clear Graph"]
                }
              }
            }
            frame 38 {
              n138 = disable-structure shown="Enabled" {
                disable-tunnel: w545 -> [w554 _]
                disable-tunnel: w544 -> [w553 w557]
                disable-tunnel: [w552 w557] -> w543
                disable-tunnel: [w547 FALSE] -> w542
                disable-tunnel: [w546 w555] -> w541
                frame Disabled {
                  w546 = T14[] [enum."Adjust Controls", enum."Save App Config"] items=["Main", "Init Files", "Init", "Unused", "Save As", "Start Profile", "Check Step Time", "Alarm", "Alarm Dismiss", "Run Step", "Stop Profile", "Cycle Reset", "Time Reset", "Time Reset All", "Time Set", "Tare CTs", "Save Profile", "Open Profile", "Get Profiles", "Update Screen", "Update Controls", "Save App Config", "Write Outputs", "Disable Background", "Enable Background", "Get/Release Control", "Log Fuel Change", "Fuel Change Popup", "Read Inputs", "Remote Timer Reset", "Controller Change", "Get Alarms", "Init Alarms", "Save Alarms", "Voltage Selection", "Set Watlow Temp 1", "Set Watlow Temp 2", "Get Pressure", "Write Tare Pressure", "Adjust Controls", "Reinit ADC", "Write Initial Times", "Write Pumps Present", "HMI Command", "Save Pump Times", "Check Pump Stop Time", "Save LS App Config", "Init Data File", "Reset LS Cycles", "Reset Anomalies", "Reset Opens", "Save LS Data", "Save LS Test Data", "Check Serial Numbers", "Main Tab", "Allow Data Note", "Resume Profile", "Pause Profile", "Allow Pause Note", "Clear Graph"]
                  n139 = Unbundle By Name(w554) -> ("App Config.Voltage Scale"=w551:cluster{"V_FFm":dbl, "V_FFb":dbl})
                  n140 = Not Equal?(x="Voltage Scale", y=w551) -> (x != y?=w549:cluster{bool, bool})
                  n141 = Cluster To Array(cluster=w549) -> (array=w548:bool[])
                  n142 = Or Array Elements(Boolean array=w548) -> (logical OR=w547:bool)
                  n143 = Bundle By Name(cluster=w553, "App Config.Voltage Scale"="Voltage Scale") -> (w552:T25)
                }
                frame Enabled {
                  w555 = T14[] [] items=["Main", "Init Files", "Init", "Unused", "Save As", "Start Profile", "Check Step Time", "Alarm", "Alarm Dismiss", "Run Step", "Stop Profile", "Cycle Reset", "Time Reset", "Time Reset All", "Time Set", "Tare CTs", "Save Profile", "Open Profile", "Get Profiles", "Update Screen", "Update Controls", "Save App Config", "Write Outputs", "Disable Background", "Enable Background", "Get/Release Control", "Log Fuel Change", "Fuel Change Popup", "Read Inputs", "Remote Timer Reset", "Controller Change", "Get Alarms", "Init Alarms", "Save Alarms", "Voltage Selection", "Set Watlow Temp 1", "Set Watlow Temp 2", "Get Pressure", "Write Tare Pressure", "Adjust Controls", "Reinit ADC", "Write Initial Times", "Write Pumps Present", "HMI Command", "Save Pump Times", "Check Pump Stop Time", "Save LS App Config", "Init Data File", "Reset LS Cycles", "Reset Anomalies", "Reset Opens", "Save LS Data", "Save LS Test Data", "Check Serial Numbers", "Main Tab", "Allow Data Note", "Resume Profile", "Pause Profile", "Allow Pause Note", "Clear Graph"]
                }
              }
            }
            frame 39 {
              n144 = disable-structure shown="Enabled" {
                disable-tunnel: w562 -> [w571 _]
                disable-tunnel: w561 -> [w570 w574]
                disable-tunnel: [w569 w574] -> w560
                disable-tunnel: [w565 FALSE] -> w559
                disable-tunnel: [w563 w572] -> w558
                frame Disabled {
                  w563 = T14[] [enum."Adjust Controls", enum."Save App Config"] items=["Main", "Init Files", "Init", "Unused", "Save As", "Start Profile", "Check Step Time", "Alarm", "Alarm Dismiss", "Run Step", "Stop Profile", "Cycle Reset", "Time Reset", "Time Reset All", "Time Set", "Tare CTs", "Save Profile", "Open Profile", "Get Profiles", "Update Screen", "Update Controls", "Save App Config", "Write Outputs", "Disable Background", "Enable Background", "Get/Release Control", "Log Fuel Change", "Fuel Change Popup", "Read Inputs", "Remote Timer Reset", "Controller Change", "Get Alarms", "Init Alarms", "Save Alarms", "Voltage Selection", "Set Watlow Temp 1", "Set Watlow Temp 2", "Get Pressure", "Write Tare Pressure", "Adjust Controls", "Reinit ADC", "Write Initial Times", "Write Pumps Present", "HMI Command", "Save Pump Times", "Check Pump Stop Time", "Save LS App Config", "Init Data File", "Reset LS Cycles", "Reset Anomalies", "Reset Opens", "Save LS Data", "Save LS Test Data", "Check Serial Numbers", "Main Tab", "Allow Data Note", "Resume Profile", "Pause Profile", "Allow Pause Note", "Clear Graph"]
                  n145 = Unbundle By Name(w571) -> ("App Config.Voltage Cutoffs"=w568:cluster{"V_MidCutoff":dbl, "V_CloseCutoff":dbl})
                  n146 = Not Equal?(x="Cutoffs", y=w568) -> (x != y?=w567:cluster{bool, bool})
                  n147 = Cluster To Array(cluster=w567) -> (array=w566:bool[])
                  n148 = Or Array Elements(Boolean array=w566) -> (logical OR=w565:bool)
                  n149 = Bundle By Name(cluster=w570, "App Config.Voltage Cutoffs"="Cutoffs") -> (w569:T25)
                }
                frame Enabled {
                  w572 = T14[] [] items=["Main", "Init Files", "Init", "Unused", "Save As", "Start Profile", "Check Step Time", "Alarm", "Alarm Dismiss", "Run Step", "Stop Profile", "Cycle Reset", "Time Reset", "Time Reset All", "Time Set", "Tare CTs", "Save Profile", "Open Profile", "Get Profiles", "Update Screen", "Update Controls", "Save App Config", "Write Outputs", "Disable Background", "Enable Background", "Get/Release Control", "Log Fuel Change", "Fuel Change Popup", "Read Inputs", "Remote Timer Reset", "Controller Change", "Get Alarms", "Init Alarms", "Save Alarms", "Voltage Selection", "Set Watlow Temp 1", "Set Watlow Temp 2", "Get Pressure", "Write Tare Pressure", "Adjust Controls", "Reinit ADC", "Write Initial Times", "Write Pumps Present", "HMI Command", "Save Pump Times", "Check Pump Stop Time", "Save LS App Config", "Init Data File", "Reset LS Cycles", "Reset Anomalies", "Reset Opens", "Save LS Data", "Save LS Test Data", "Check Serial Numbers", "Main Tab", "Allow Data Note", "Resume Profile", "Pause Profile", "Allow Pause Note", "Clear Graph"]
                }
              }
            }
            frame 40 {
              n150 = disable-structure shown="Enabled" {
                disable-tunnel: w579 -> [w588 _]
                disable-tunnel: w578 -> [w587 w591]
                disable-tunnel: [w586 w591] -> w577
                disable-tunnel: [w584 w589] -> w576
                disable-tunnel: [w581 FALSE] -> w575
                frame Disabled {
                  w584 = T14[] [enum."Save App Config"] items=["Main", "Init Files", "Init", "Unused", "Save As", "Start Profile", "Check Step Time", "Alarm", "Alarm Dismiss", "Run Step", "Stop Profile", "Cycle Reset", "Time Reset", "Time Reset All", "Time Set", "Tare CTs", "Save Profile", "Open Profile", "Get Profiles", "Update Screen", "Update Controls", "Save App Config", "Write Outputs", "Disable Background", "Enable Background", "Get/Release Control", "Log Fuel Change", "Fuel Change Popup", "Read Inputs", "Remote Timer Reset", "Controller Change", "Get Alarms", "Init Alarms", "Save Alarms", "Voltage Selection", "Set Watlow Temp 1", "Set Watlow Temp 2", "Get Pressure", "Write Tare Pressure", "Adjust Controls", "Reinit ADC", "Write Initial Times", "Write Pumps Present", "HMI Command", "Save Pump Times", "Check Pump Stop Time", "Save LS App Config", "Init Data File", "Reset LS Cycles", "Reset Anomalies", "Reset Opens", "Save LS Data", "Save LS Test Data", "Check Serial Numbers", "Main Tab", "Allow Data Note", "Resume Profile", "Pause Profile", "Allow Pause Note", "Clear Graph"]
                  n151 = Unbundle By Name(w588) -> ("App Config.Pressure Scale"=w585:cluster{"Pres_FFm":dbl, "Pres_FFb":dbl})
                  n152 = Not Equal?(x="Pressure Scale", y=w585) -> (x != y?=w583:cluster{bool, bool})
                  n153 = Cluster To Array(cluster=w583) -> (array=w582:bool[])
                  n154 = Or Array Elements(Boolean array=w582) -> (logical OR=w581:bool)
                  n155 = Bundle By Name(cluster=w587, "App Config.Pressure Scale"="Pressure Scale") -> (w586:T25)
                }
                frame Enabled {
                  w589 = T14[] [] items=["Main", "Init Files", "Init", "Unused", "Save As", "Start Profile", "Check Step Time", "Alarm", "Alarm Dismiss", "Run Step", "Stop Profile", "Cycle Reset", "Time Reset", "Time Reset All", "Time Set", "Tare CTs", "Save Profile", "Open Profile", "Get Profiles", "Update Screen", "Update Controls", "Save App Config", "Write Outputs", "Disable Background", "Enable Background", "Get/Release Control", "Log Fuel Change", "Fuel Change Popup", "Read Inputs", "Remote Timer Reset", "Controller Change", "Get Alarms", "Init Alarms", "Save Alarms", "Voltage Selection", "Set Watlow Temp 1", "Set Watlow Temp 2", "Get Pressure", "Write Tare Pressure", "Adjust Controls", "Reinit ADC", "Write Initial Times", "Write Pumps Present", "HMI Command", "Save Pump Times", "Check Pump Stop Time", "Save LS App Config", "Init Data File", "Reset LS Cycles", "Reset Anomalies", "Reset Opens", "Save LS Data", "Save LS Test Data", "Check Serial Numbers", "Main Tab", "Allow Data Note", "Resume Profile", "Pause Profile", "Allow Pause Note", "Clear Graph"]
                }
              }
            }
            frame 41 {
              n156 = disable-structure shown="Enabled" {
                disable-tunnel: w596 -> [w604 _]
                disable-tunnel: w595 -> [w603 w607]
                disable-tunnel: [w602 w607] -> w594
                disable-tunnel: [w600 w605] -> w593
                disable-tunnel: [w599 FALSE] -> w592
                frame Disabled {
                  w600 = T14[] [enum."Save App Config"] items=["Main", "Init Files", "Init", "Unused", "Save As", "Start Profile", "Check Step Time", "Alarm", "Alarm Dismiss", "Run Step", "Stop Profile", "Cycle Reset", "Time Reset", "Time Reset All", "Time Set", "Tare CTs", "Save Profile", "Open Profile", "Get Profiles", "Update Screen", "Update Controls", "Save App Config", "Write Outputs", "Disable Background", "Enable Background", "Get/Release Control", "Log Fuel Change", "Fuel Change Popup", "Read Inputs", "Remote Timer Reset", "Controller Change", "Get Alarms", "Init Alarms", "Save Alarms", "Voltage Selection", "Set Watlow Temp 1", "Set Watlow Temp 2", "Get Pressure", "Write Tare Pressure", "Adjust Controls", "Reinit ADC", "Write Initial Times", "Write Pumps Present", "HMI Command", "Save Pump Times", "Check Pump Stop Time", "Save LS App Config", "Init Data File", "Reset LS Cycles", "Reset Anomalies", "Reset Opens", "Save LS Data", "Save LS Test Data", "Check Serial Numbers", "Main Tab", "Allow Data Note", "Resume Profile", "Pause Profile", "Allow Pause Note", "Clear Graph"]
                  n157 = Unbundle By Name(w604) -> ("App Config.Temp Format"=w601:i32)
                  n158 = To Long Integer(number="Thermocouple") -> (32bit integer=w597:i32)
                  n159 = Not Equal?(x=w597, y=w601) -> (x != y?=w599:bool)
                  n160 = Bundle By Name(cluster=w603, "App Config.Temp Format"=w597) -> (w602:T25)
                }
                frame Enabled {
                  w605 = T14[] [] items=["Main", "Init Files", "Init", "Unused", "Save As", "Start Profile", "Check Step Time", "Alarm", "Alarm Dismiss", "Run Step", "Stop Profile", "Cycle Reset", "Time Reset", "Time Reset All", "Time Set", "Tare CTs", "Save Profile", "Open Profile", "Get Profiles", "Update Screen", "Update Controls", "Save App Config", "Write Outputs", "Disable Background", "Enable Background", "Get/Release Control", "Log Fuel Change", "Fuel Change Popup", "Read Inputs", "Remote Timer Reset", "Controller Change", "Get Alarms", "Init Alarms", "Save Alarms", "Voltage Selection", "Set Watlow Temp 1", "Set Watlow Temp 2", "Get Pressure", "Write Tare Pressure", "Adjust Controls", "Reinit ADC", "Write Initial Times", "Write Pumps Present", "HMI Command", "Save Pump Times", "Check Pump Stop Time", "Save LS App Config", "Init Data File", "Reset LS Cycles", "Reset Anomalies", "Reset Opens", "Save LS Data", "Save LS Test Data", "Check Serial Numbers", "Main Tab", "Allow Data Note", "Resume Profile", "Pause Profile", "Allow Pause Note", "Clear Graph"]
                }
              }
            }
            frame 42 {
              n161 = disable-structure shown="Enabled" {
                disable-tunnel: w612 -> [w619 _]
                disable-tunnel: w611 -> [w618 w622]
                disable-tunnel: [w617 w622] -> w610
                disable-tunnel: [w615 w620] -> w609
                disable-tunnel: [w613 FALSE] -> w608
                frame Disabled {
                  w615 = T14[] [enum."Save App Config"] items=["Main", "Init Files", "Init", "Unused", "Save As", "Start Profile", "Check Step Time", "Alarm", "Alarm Dismiss", "Run Step", "Stop Profile", "Cycle Reset", "Time Reset", "Time Reset All", "Time Set", "Tare CTs", "Save Profile", "Open Profile", "Get Profiles", "Update Screen", "Update Controls", "Save App Config", "Write Outputs", "Disable Background", "Enable Background", "Get/Release Control", "Log Fuel Change", "Fuel Change Popup", "Read Inputs", "Remote Timer Reset", "Controller Change", "Get Alarms", "Init Alarms", "Save Alarms", "Voltage Selection", "Set Watlow Temp 1", "Set Watlow Temp 2", "Get Pressure", "Write Tare Pressure", "Adjust Controls", "Reinit ADC", "Write Initial Times", "Write Pumps Present", "HMI Command", "Save Pump Times", "Check Pump Stop Time", "Save LS App Config", "Init Data File", "Reset LS Cycles", "Reset Anomalies", "Reset Opens", "Save LS Data", "Save LS Test Data", "Check Serial Numbers", "Main Tab", "Allow Data Note", "Resume Profile", "Pause Profile", "Allow Pause Note", "Clear Graph"]
                  n162 = Unbundle By Name(w619) -> ("App Config.Temp Tolerance"=w616:dbl)
                  n163 = Not Equal?(x="Temp Tolerance", y=w616) -> (x != y?=w613:bool)
                  n164 = Bundle By Name(cluster=w618, "App Config.Temp Tolerance"="Temp Tolerance") -> (w617:T25)
                }
                frame Enabled {
                  w620 = T14[] [] items=["Main", "Init Files", "Init", "Unused", "Save As", "Start Profile", "Check Step Time", "Alarm", "Alarm Dismiss", "Run Step", "Stop Profile", "Cycle Reset", "Time Reset", "Time Reset All", "Time Set", "Tare CTs", "Save Profile", "Open Profile", "Get Profiles", "Update Screen", "Update Controls", "Save App Config", "Write Outputs", "Disable Background", "Enable Background", "Get/Release Control", "Log Fuel Change", "Fuel Change Popup", "Read Inputs", "Remote Timer Reset", "Controller Change", "Get Alarms", "Init Alarms", "Save Alarms", "Voltage Selection", "Set Watlow Temp 1", "Set Watlow Temp 2", "Get Pressure", "Write Tare Pressure", "Adjust Controls", "Reinit ADC", "Write Initial Times", "Write Pumps Present", "HMI Command", "Save Pump Times", "Check Pump Stop Time", "Save LS App Config", "Init Data File", "Reset LS Cycles", "Reset Anomalies", "Reset Opens", "Save LS Data", "Save LS Test Data", "Check Serial Numbers", "Main Tab", "Allow Data Note", "Resume Profile", "Pause Profile", "Allow Pause Note", "Clear Graph"]
                }
              }
            }
            frame 43 {
              n165 = disable-structure shown="Enabled" {
                disable-tunnel: [w634 w635] -> w627
                disable-tunnel: w626 -> [w633 w637]
                disable-tunnel: [w632 w637] -> w625
                disable-tunnel: w624 -> [w631 _]
                disable-tunnel: [w629 FALSE] -> w623
                frame Disabled {
                  w634 = T14[] [enum."Save App Config"] items=["Main", "Init Files", "Init", "Unused", "Save As", "Start Profile", "Check Step Time", "Alarm", "Alarm Dismiss", "Run Step", "Stop Profile", "Cycle Reset", "Time Reset", "Time Reset All", "Time Set", "Tare CTs", "Save Profile", "Open Profile", "Get Profiles", "Update Screen", "Update Controls", "Save App Config", "Write Outputs", "Disable Background", "Enable Background", "Get/Release Control", "Log Fuel Change", "Fuel Change Popup", "Read Inputs", "Remote Timer Reset", "Controller Change", "Get Alarms", "Init Alarms", "Save Alarms", "Voltage Selection", "Set Watlow Temp 1", "Set Watlow Temp 2", "Get Pressure", "Write Tare Pressure", "Adjust Controls", "Reinit ADC", "Write Initial Times", "Write Pumps Present", "HMI Command", "Save Pump Times", "Check Pump Stop Time", "Save LS App Config", "Init Data File", "Reset LS Cycles", "Reset Anomalies", "Reset Opens", "Save LS Data", "Save LS Test Data", "Check Serial Numbers", "Main Tab", "Allow Data Note", "Resume Profile", "Pause Profile", "Allow Pause Note", "Clear Graph"]
                  n166 = Unbundle By Name(w631) -> ("App Config.Target Voltage"=w630:dbl)
                  n167 = Not Equal?(x=w630, y="Target Voltage:") -> (x != y?=w629:bool)
                  n168 = Bundle By Name(cluster=w633, "App Config.Target Voltage"="Target Voltage:") -> (w632:T25)
                }
                frame Enabled {
                  w635 = T14[] [] items=["Main", "Init Files", "Init", "Unused", "Save As", "Start Profile", "Check Step Time", "Alarm", "Alarm Dismiss", "Run Step", "Stop Profile", "Cycle Reset", "Time Reset", "Time Reset All", "Time Set", "Tare CTs", "Save Profile", "Open Profile", "Get Profiles", "Update Screen", "Update Controls", "Save App Config", "Write Outputs", "Disable Background", "Enable Background", "Get/Release Control", "Log Fuel Change", "Fuel Change Popup", "Read Inputs", "Remote Timer Reset", "Controller Change", "Get Alarms", "Init Alarms", "Save Alarms", "Voltage Selection", "Set Watlow Temp 1", "Set Watlow Temp 2", "Get Pressure", "Write Tare Pressure", "Adjust Controls", "Reinit ADC", "Write Initial Times", "Write Pumps Present", "HMI Command", "Save Pump Times", "Check Pump Stop Time", "Save LS App Config", "Init Data File", "Reset LS Cycles", "Reset Anomalies", "Reset Opens", "Save LS Data", "Save LS Test Data", "Check Serial Numbers", "Main Tab", "Allow Data Note", "Resume Profile", "Pause Profile", "Allow Pause Note", "Clear Graph"]
                }
              }
            }
            frame 44 {
              n169 = disable-structure shown="Enabled" {
                disable-tunnel: [w649 w650] -> w642
                disable-tunnel: w641 -> [w648 w652]
                disable-tunnel: [w647 w652] -> w640
                disable-tunnel: w639 -> [w646 _]
                disable-tunnel: [w644 FALSE] -> w638
                frame Disabled {
                  w649 = T14[] [enum."Save App Config"] items=["Main", "Init Files", "Init", "Unused", "Save As", "Start Profile", "Check Step Time", "Alarm", "Alarm Dismiss", "Run Step", "Stop Profile", "Cycle Reset", "Time Reset", "Time Reset All", "Time Set", "Tare CTs", "Save Profile", "Open Profile", "Get Profiles", "Update Screen", "Update Controls", "Save App Config", "Write Outputs", "Disable Background", "Enable Background", "Get/Release Control", "Log Fuel Change", "Fuel Change Popup", "Read Inputs", "Remote Timer Reset", "Controller Change", "Get Alarms", "Init Alarms", "Save Alarms", "Voltage Selection", "Set Watlow Temp 1", "Set Watlow Temp 2", "Get Pressure", "Write Tare Pressure", "Adjust Controls", "Reinit ADC", "Write Initial Times", "Write Pumps Present", "HMI Command", "Save Pump Times", "Check Pump Stop Time", "Save LS App Config", "Init Data File", "Reset LS Cycles", "Reset Anomalies", "Reset Opens", "Save LS Data", "Save LS Test Data", "Check Serial Numbers", "Main Tab", "Allow Data Note", "Resume Profile", "Pause Profile", "Allow Pause Note", "Clear Graph"]
                  n170 = Unbundle By Name(w646) -> ("App Config.Target Pressure"=w645:dbl)
                  n171 = Not Equal?(x=w645, y="Target Pressure:") -> (x != y?=w644:bool)
                  n172 = Bundle By Name(cluster=w648, "App Config.Target Pressure"="Target Pressure:") -> (w647:T25)
                }
                frame Enabled {
                  w650 = T14[] [] items=["Main", "Init Files", "Init", "Unused", "Save As", "Start Profile", "Check Step Time", "Alarm", "Alarm Dismiss", "Run Step", "Stop Profile", "Cycle Reset", "Time Reset", "Time Reset All", "Time Set", "Tare CTs", "Save Profile", "Open Profile", "Get Profiles", "Update Screen", "Update Controls", "Save App Config", "Write Outputs", "Disable Background", "Enable Background", "Get/Release Control", "Log Fuel Change", "Fuel Change Popup", "Read Inputs", "Remote Timer Reset", "Controller Change", "Get Alarms", "Init Alarms", "Save Alarms", "Voltage Selection", "Set Watlow Temp 1", "Set Watlow Temp 2", "Get Pressure", "Write Tare Pressure", "Adjust Controls", "Reinit ADC", "Write Initial Times", "Write Pumps Present", "HMI Command", "Save Pump Times", "Check Pump Stop Time", "Save LS App Config", "Init Data File", "Reset LS Cycles", "Reset Anomalies", "Reset Opens", "Save LS Data", "Save LS Test Data", "Check Serial Numbers", "Main Tab", "Allow Data Note", "Resume Profile", "Pause Profile", "Allow Pause Note", "Clear Graph"]
                }
              }
            }
            frame 45 {
              w656 = T14[] [enum."HMI Command"] items=["Main", "Init Files", "Init", "Unused", "Save As", "Start Profile", "Check Step Time", "Alarm", "Alarm Dismiss", "Run Step", "Stop Profile", "Cycle Reset", "Time Reset", "Time Reset All", "Time Set", "Tare CTs", "Save Profile", "Open Profile", "Get Profiles", "Update Screen", "Update Controls", "Save App Config", "Write Outputs", "Disable Background", "Enable Background", "Get/Release Control", "Log Fuel Change", "Fuel Change Popup", "Read Inputs", "Remote Timer Reset", "Controller Change", "Get Alarms", "Init Alarms", "Save Alarms", "Voltage Selection", "Set Watlow Temp 1", "Set Watlow Temp 2", "Get Pressure", "Write Tare Pressure", "Adjust Controls", "Reinit ADC", "Write Initial Times", "Write Pumps Present", "HMI Command", "Save Pump Times", "Check Pump Stop Time", "Save LS App Config", "Init Data File", "Reset LS Cycles", "Reset Anomalies", "Reset Opens", "Save LS Data", "Save LS Test Data", "Check Serial Numbers", "Main Tab", "Allow Data Note", "Resume Profile", "Pause Profile", "Allow Pause Note", "Clear Graph"]
              n173 = call "RPi HMI Global.vi"() -> ("HMI Cluster OUT"=w655:T16)  [unwired: 11 in]
              n174 = Unbundle By Name(w655) -> ("HMI Command"=w653:bool)
            }
            frame 46 {
              w663 = T14[] [enum."Update Controls"] items=["Main", "Init Files", "Init", "Unused", "Save As", "Start Profile", "Check Step Time", "Alarm", "Alarm Dismiss", "Run Step", "Stop Profile", "Cycle Reset", "Time Reset", "Time Reset All", "Time Set", "Tare CTs", "Save Profile", "Open Profile", "Get Profiles", "Update Screen", "Update Controls", "Save App Config", "Write Outputs", "Disable Background", "Enable Background", "Get/Release Control", "Log Fuel Change", "Fuel Change Popup", "Read Inputs", "Remote Timer Reset", "Controller Change", "Get Alarms", "Init Alarms", "Save Alarms", "Voltage Selection", "Set Watlow Temp 1", "Set Watlow Temp 2", "Get Pressure", "Write Tare Pressure", "Adjust Controls", "Reinit ADC", "Write Initial Times", "Write Pumps Present", "HMI Command", "Save Pump Times", "Check Pump Stop Time", "Save LS App Config", "Init Data File", "Reset LS Cycles", "Reset Anomalies", "Reset Opens", "Save LS Data", "Save LS Test Data", "Check Serial Numbers", "Main Tab", "Allow Data Note", "Resume Profile", "Pause Profile", "Allow Pause Note", "Clear Graph"]
              n175 = Unbundle By Name(w662) -> ("Email Alarms Disabled"=w659:bool)
              n176 = Greater?(x="Disable Alarm Email", y=w659) -> (0:w657:bool)
              n177 = Bundle By Name(cluster=w661, "Email Alarms Disabled"="Disable Alarm Email") -> (w660:T25)
            }
            frame 47 {
              w668 = T14[] [] items=["Main", "Init Files", "Init", "Unused", "Save As", "Start Profile", "Check Step Time", "Alarm", "Alarm Dismiss", "Run Step", "Stop Profile", "Cycle Reset", "Time Reset", "Time Reset All", "Time Set", "Tare CTs", "Save Profile", "Open Profile", "Get Profiles", "Update Screen", "Update Controls", "Save App Config", "Write Outputs", "Disable Background", "Enable Background", "Get/Release Control", "Log Fuel Change", "Fuel Change Popup", "Read Inputs", "Remote Timer Reset", "Controller Change", "Get Alarms", "Init Alarms", "Save Alarms", "Voltage Selection", "Set Watlow Temp 1", "Set Watlow Temp 2", "Get Pressure", "Write Tare Pressure", "Adjust Controls", "Reinit ADC", "Write Initial Times", "Write Pumps Present", "HMI Command", "Save Pump Times", "Check Pump Stop Time", "Save LS App Config", "Init Data File", "Reset LS Cycles", "Reset Anomalies", "Reset Opens", "Save LS Data", "Save LS Test Data", "Check Serial Numbers", "Main Tab", "Allow Data Note", "Resume Profile", "Pause Profile", "Allow Pause Note", "Clear Graph"]
              n178 = Bundle By Name(cluster=w667, "Concat Data"="Concat Data") -> (w666:T25)
            }
            frame 48 {
              w673 = T14[] [] items=["Main", "Init Files", "Init", "Unused", "Save As", "Start Profile", "Check Step Time", "Alarm", "Alarm Dismiss", "Run Step", "Stop Profile", "Cycle Reset", "Time Reset", "Time Reset All", "Time Set", "Tare CTs", "Save Profile", "Open Profile", "Get Profiles", "Update Screen", "Update Controls", "Save App Config", "Write Outputs", "Disable Background", "Enable Background", "Get/Release Control", "Log Fuel Change", "Fuel Change Popup", "Read Inputs", "Remote Timer Reset", "Controller Change", "Get Alarms", "Init Alarms", "Save Alarms", "Voltage Selection", "Set Watlow Temp 1", "Set Watlow Temp 2", "Get Pressure", "Write Tare Pressure", "Adjust Controls", "Reinit ADC", "Write Initial Times", "Write Pumps Present", "HMI Command", "Save Pump Times", "Check Pump Stop Time", "Save LS App Config", "Init Data File", "Reset LS Cycles", "Reset Anomalies", "Reset Opens", "Save LS Data", "Save LS Test Data", "Check Serial Numbers", "Main Tab", "Allow Data Note", "Resume Profile", "Pause Profile", "Allow Pause Note", "Clear Graph"]
              n179 = Bundle By Name(cluster=w672, "WebDAV Push"="WebDAV Push") -> (w671:T25)
            }
            frame 49 {
              w680 = T14[] [enum."Save App Config", enum."Write Outputs"] items=["Main", "Init Files", "Init", "Unused", "Save As", "Start Profile", "Check Step Time", "Alarm", "Alarm Dismiss", "Run Step", "Stop Profile", "Cycle Reset", "Time Reset", "Time Reset All", "Time Set", "Tare CTs", "Save Profile", "Open Profile", "Get Profiles", "Update Screen", "Update Controls", "Save App Config", "Write Outputs", "Disable Background", "Enable Background", "Get/Release Control", "Log Fuel Change", "Fuel Change Popup", "Read Inputs", "Remote Timer Reset", "Controller Change", "Get Alarms", "Init Alarms", "Save Alarms", "Voltage Selection", "Set Watlow Temp 1", "Set Watlow Temp 2", "Get Pressure", "Write Tare Pressure", "Adjust Controls", "Reinit ADC", "Write Initial Times", "Write Pumps Present", "HMI Command", "Save Pump Times", "Check Pump Stop Time", "Save LS App Config", "Init Data File", "Reset LS Cycles", "Reset Anomalies", "Reset Opens", "Save LS Data", "Save LS Test Data", "Check Serial Numbers", "Main Tab", "Allow Data Note", "Resume Profile", "Pause Profile", "Allow Pause Note", "Clear Graph"]
              n180 = Unbundle By Name(w677) -> ("App Config.Cycle Threshold:"=w675:dbl)
              n181 = Not Equal?(x=w675, y="Cycle Threshold:") -> (x != y?=w676:bool)
              n182 = Bundle By Name(cluster=w679, "App Config.Cycle Threshold:"="Cycle Threshold:") -> (w678:T25)
            }
            frame 50 {
              w687 = T14[] [enum."Save App Config", enum."Write Outputs"] items=["Main", "Init Files", "Init", "Unused", "Save As", "Start Profile", "Check Step Time", "Alarm", "Alarm Dismiss", "Run Step", "Stop Profile", "Cycle Reset", "Time Reset", "Time Reset All", "Time Set", "Tare CTs", "Save Profile", "Open Profile", "Get Profiles", "Update Screen", "Update Controls", "Save App Config", "Write Outputs", "Disable Background", "Enable Background", "Get/Release Control", "Log Fuel Change", "Fuel Change Popup", "Read Inputs", "Remote Timer Reset", "Controller Change", "Get Alarms", "Init Alarms", "Save Alarms", "Voltage Selection", "Set Watlow Temp 1", "Set Watlow Temp 2", "Get Pressure", "Write Tare Pressure", "Adjust Controls", "Reinit ADC", "Write Initial Times", "Write Pumps Present", "HMI Command", "Save Pump Times", "Check Pump Stop Time", "Save LS App Config", "Init Data File", "Reset LS Cycles", "Reset Anomalies", "Reset Opens", "Save LS Data", "Save LS Test Data", "Check Serial Numbers", "Main Tab", "Allow Data Note", "Resume Profile", "Pause Profile", "Allow Pause Note", "Clear Graph"]
              n183 = Unbundle By Name(w684) -> ("App Config.Cycle Pts to Avg:"=w682:i32)
              n184 = Not Equal?(x=w682, y="Cycle Pts to Avg:") -> (x != y?=w683:bool)
              n185 = Bundle By Name(cluster=w686, "App Config.Cycle Pts to Avg:"="Cycle Pts to Avg:") -> (w685:T25)
            }
            frame 51 {
              w694 = T14[] [enum."Save App Config", enum."Write Outputs"] items=["Main", "Init Files", "Init", "Unused", "Save As", "Start Profile", "Check Step Time", "Alarm", "Alarm Dismiss", "Run Step", "Stop Profile", "Cycle Reset", "Time Reset", "Time Reset All", "Time Set", "Tare CTs", "Save Profile", "Open Profile", "Get Profiles", "Update Screen", "Update Controls", "Save App Config", "Write Outputs", "Disable Background", "Enable Background", "Get/Release Control", "Log Fuel Change", "Fuel Change Popup", "Read Inputs", "Remote Timer Reset", "Controller Change", "Get Alarms", "Init Alarms", "Save Alarms", "Voltage Selection", "Set Watlow Temp 1", "Set Watlow Temp 2", "Get Pressure", "Write Tare Pressure", "Adjust Controls", "Reinit ADC", "Write Initial Times", "Write Pumps Present", "HMI Command", "Save Pump Times", "Check Pump Stop Time", "Save LS App Config", "Init Data File", "Reset LS Cycles", "Reset Anomalies", "Reset Opens", "Save LS Data", "Save LS Test Data", "Check Serial Numbers", "Main Tab", "Allow Data Note", "Resume Profile", "Pause Profile", "Allow Pause Note", "Clear Graph"]
              n186 = Unbundle By Name(w691) -> ("App Config.Step Threshold:"=w689:dbl)
              n187 = Not Equal?(x=w689, y="Step Threshold:") -> (x != y?=w690:bool)
              n188 = Bundle By Name(cluster=w693, "App Config.Step Threshold:"="Step Threshold:") -> (w692:T25)
            }
            frame 52 {
              w701 = T14[] [enum."Save App Config", enum."Write Outputs"] items=["Main", "Init Files", "Init", "Unused", "Save As", "Start Profile", "Check Step Time", "Alarm", "Alarm Dismiss", "Run Step", "Stop Profile", "Cycle Reset", "Time Reset", "Time Reset All", "Time Set", "Tare CTs", "Save Profile", "Open Profile", "Get Profiles", "Update Screen", "Update Controls", "Save App Config", "Write Outputs", "Disable Background", "Enable Background", "Get/Release Control", "Log Fuel Change", "Fuel Change Popup", "Read Inputs", "Remote Timer Reset", "Controller Change", "Get Alarms", "Init Alarms", "Save Alarms", "Voltage Selection", "Set Watlow Temp 1", "Set Watlow Temp 2", "Get Pressure", "Write Tare Pressure", "Adjust Controls", "Reinit ADC", "Write Initial Times", "Write Pumps Present", "HMI Command", "Save Pump Times", "Check Pump Stop Time", "Save LS App Config", "Init Data File", "Reset LS Cycles", "Reset Anomalies", "Reset Opens", "Save LS Data", "Save LS Test Data", "Check Serial Numbers", "Main Tab", "Allow Data Note", "Resume Profile", "Pause Profile", "Allow Pause Note", "Clear Graph"]
              n189 = Unbundle By Name(w698) -> ("App Config.Normal Steps:"=w696:u32)
              n190 = Not Equal?(x=w696, y="Normal Steps:") -> (x != y?=w697:bool)
              n191 = Bundle By Name(cluster=w700, "App Config.Normal Steps:"="Normal Steps:") -> (w699:T25)
            }
            frame 53 {
              w710 = T14[] [enum."Main Tab"] items=["Main", "Init Files", "Init", "Unused", "Save As", "Start Profile", "Check Step Time", "Alarm", "Alarm Dismiss", "Run Step", "Stop Profile", "Cycle Reset", "Time Reset", "Time Reset All", "Time Set", "Tare CTs", "Save Profile", "Open Profile", "Get Profiles", "Update Screen", "Update Controls", "Save App Config", "Write Outputs", "Disable Background", "Enable Background", "Get/Release Control", "Log Fuel Change", "Fuel Change Popup", "Read Inputs", "Remote Timer Reset", "Controller Change", "Get Alarms", "Init Alarms", "Save Alarms", "Voltage Selection", "Set Watlow Temp 1", "Set Watlow Temp 2", "Get Pressure", "Write Tare Pressure", "Adjust Controls", "Reinit ADC", "Write Initial Times", "Write Pumps Present", "HMI Command", "Save Pump Times", "Check Pump Stop Time", "Save LS App Config", "Init Data File", "Reset LS Cycles", "Reset Anomalies", "Reset Opens", "Save LS Data", "Save LS Test Data", "Check Serial Numbers", "Main Tab", "Allow Data Note", "Resume Profile", "Pause Profile", "Allow Pause Note", "Clear Graph"]
              n192 = Unbundle By Name(w715) -> ("Main Tab"=w712:T9)
              n193 = local read "Main Tab"() -> (w711:T9)
              n194 = local read "Position"() -> (w704:i32)
              n195 = local read "Pause"() -> (w706:bool)
              n196 = feedback-in #1(w704) -> ()
              n197 = feedback #1(w704) -> (w705:i32)
              n198 = feedback #2(w706) -> (w707:bool)
              n199 = feedback-in #2(w706) -> ()
              n200 = Not Equal?(x=w712, y=w711) -> (x != y?=w709:bool)
              n201 = Not Equal?(x=w705, y=w704) -> (x != y?=w703:bool)
              n202 = Greater?(x=w707, y=w706) -> (0:w702:bool)
              n203 = Compound Arithmetic op=OR(w709, w703, w702) -> (w708:bool)
              n204 = case shown="True" w708 {
                frame False {
                }
                frame True {
                  n205 = property on="Waveform Chart" class="WFChart (strict)"("History Data"=dbl[] []) -> ()  [unwired: 2 in, 2 out]
                }
              }
              n206 = Bundle By Name(cluster=w714, "Main Tab"=w711) -> (w713:T25)
            }
            frame 54 {
              w720 = T14[] [enum."Save LS App Config", enum."Write Outputs"] items=["Main", "Init Files", "Init", "Unused", "Save As", "Start Profile", "Check Step Time", "Alarm", "Alarm Dismiss", "Run Step", "Stop Profile", "Cycle Reset", "Time Reset", "Time Reset All", "Time Set", "Tare CTs", "Save Profile", "Open Profile", "Get Profiles", "Update Screen", "Update Controls", "Save App Config", "Write Outputs", "Disable Background", "Enable Background", "Get/Release Control", "Log Fuel Change", "Fuel Change Popup", "Read Inputs", "Remote Timer Reset", "Controller Change", "Get Alarms", "Init Alarms", "Save Alarms", "Voltage Selection", "Set Watlow Temp 1", "Set Watlow Temp 2", "Get Pressure", "Write Tare Pressure", "Adjust Controls", "Reinit ADC", "Write Initial Times", "Write Pumps Present", "HMI Command", "Save Pump Times", "Check Pump Stop Time", "Save LS App Config", "Init Data File", "Reset LS Cycles", "Reset Anomalies", "Reset Opens", "Save LS Data", "Save LS Test Data", "Check Serial Numbers", "Main Tab", "Allow Data Note", "Resume Profile", "Pause Profile", "Allow Pause Note", "Clear Graph"]
              n207 = Unbundle By Name(w723) -> ("LS App Config.LS Power (Freq):"=w719:dbl)
              n208 = Not Equal?(x=w719, y="LS Cycle Time (ms):") -> (x != y?=w717:bool)
              n209 = Bundle By Name(cluster=w722, "LS App Config.LS Power (Freq):"="LS Cycle Time (ms):") -> (w721:T25)
            }
            frame 55 {
              w727 = T14[] [enum."Save LS App Config", enum."Write Outputs"] items=["Main", "Init Files", "Init", "Unused", "Save As", "Start Profile", "Check Step Time", "Alarm", "Alarm Dismiss", "Run Step", "Stop Profile", "Cycle Reset", "Time Reset", "Time Reset All", "Time Set", "Tare CTs", "Save Profile", "Open Profile", "Get Profiles", "Update Screen", "Update Controls", "Save App Config", "Write Outputs", "Disable Background", "Enable Background", "Get/Release Control", "Log Fuel Change", "Fuel Change Popup", "Read Inputs", "Remote Timer Reset", "Controller Change", "Get Alarms", "Init Alarms", "Save Alarms", "Voltage Selection", "Set Watlow Temp 1", "Set Watlow Temp 2", "Get Pressure", "Write Tare Pressure", "Adjust Controls", "Reinit ADC", "Write Initial Times", "Write Pumps Present", "HMI Command", "Save Pump Times", "Check Pump Stop Time", "Save LS App Config", "Init Data File", "Reset LS Cycles", "Reset Anomalies", "Reset Opens", "Save LS Data", "Save LS Test Data", "Check Serial Numbers", "Main Tab", "Allow Data Note", "Resume Profile", "Pause Profile", "Allow Pause Note", "Clear Graph"]
              n210 = Unbundle By Name(w730) -> ("LS App Config.LS Power (Duty):"=w726:dbl)
              n211 = Not Equal?(x=w726, y="LS On Time (ms):") -> (x != y?=w725:bool)
              n212 = Bundle By Name(cluster=w729, "LS App Config.LS Power (Duty):"="LS On Time (ms):") -> (w728:T25)
            }
            frame 56 {
              w736 = T14[] [enum."Save LS App Config", enum."Write Outputs"] items=["Main", "Init Files", "Init", "Unused", "Save As", "Start Profile", "Check Step Time", "Alarm", "Alarm Dismiss", "Run Step", "Stop Profile", "Cycle Reset", "Time Reset", "Time Reset All", "Time Set", "Tare CTs", "Save Profile", "Open Profile", "Get Profiles", "Update Screen", "Update Controls", "Save App Config", "Write Outputs", "Disable Background", "Enable Background", "Get/Release Control", "Log Fuel Change", "Fuel Change Popup", "Read Inputs", "Remote Timer Reset", "Controller Change", "Get Alarms", "Init Alarms", "Save Alarms", "Voltage Selection", "Set Watlow Temp 1", "Set Watlow Temp 2", "Get Pressure", "Write Tare Pressure", "Adjust Controls", "Reinit ADC", "Write Initial Times", "Write Pumps Present", "HMI Command", "Save Pump Times", "Check Pump Stop Time", "Save LS App Config", "Init Data File", "Reset LS Cycles", "Reset Anomalies", "Reset Opens", "Save LS Data", "Save LS Test Data", "Check Serial Numbers", "Main Tab", "Allow Data Note", "Resume Profile", "Pause Profile", "Allow Pause Note", "Clear Graph"]
              n213 = Unbundle By Name(w739) -> ("LS App Config.Bank 1 Present"=w735:T2)
              n214 = Not Equal?(x=w735, y="Bank 1") -> (x != y?=w733:T2)
              n215 = Cluster To Array(cluster=w733) -> (array=w732:bool[])
              n216 = Or Array Elements(Boolean array=w732) -> (logical OR=w731:bool)
              n217 = Bundle By Name(cluster=w738, "LS App Config.Bank 1 Present"="Bank 1") -> (w737:T25)
            }
            frame 57 {
              w745 = T14[] [enum."Save LS App Config", enum."Write Outputs"] items=["Main", "Init Files", "Init", "Unused", "Save As", "Start Profile", "Check Step Time", "Alarm", "Alarm Dismiss", "Run Step", "Stop Profile", "Cycle Reset", "Time Reset", "Time Reset All", "Time Set", "Tare CTs", "Save Profile", "Open Profile", "Get Profiles", "Update Screen", "Update Controls", "Save App Config", "Write Outputs", "Disable Background", "Enable Background", "Get/Release Control", "Log Fuel Change", "Fuel Change Popup", "Read Inputs", "Remote Timer Reset", "Controller Change", "Get Alarms", "Init Alarms", "Save Alarms", "Voltage Selection", "Set Watlow Temp 1", "Set Watlow Temp 2", "Get Pressure", "Write Tare Pressure", "Adjust Controls", "Reinit ADC", "Write Initial Times", "Write Pumps Present", "HMI Command", "Save Pump Times", "Check Pump Stop Time", "Save LS App Config", "Init Data File", "Reset LS Cycles", "Reset Anomalies", "Reset Opens", "Save LS Data", "Save LS Test Data", "Check Serial Numbers", "Main Tab", "Allow Data Note", "Resume Profile", "Pause Profile", "Allow Pause Note", "Clear Graph"]
              n218 = Unbundle By Name(w748) -> ("LS App Config.Bank 2 Present"=w744:T1)
              n219 = Not Equal?(x=w744, y="Bank 2") -> (x != y?=w743:T1)
              n220 = Cluster To Array(cluster=w743) -> (array=w742:bool[])
              n221 = Or Array Elements(Boolean array=w742) -> (logical OR=w741:bool)
              n222 = Bundle By Name(cluster=w747, "LS App Config.Bank 2 Present"="Bank 2") -> (w746:T25)
            }
            frame 58 {
              w752 = T14[] [enum."Init Data File", enum."Save LS App Config"] items=["Main", "Init Files", "Init", "Unused", "Save As", "Start Profile", "Check Step Time", "Alarm", "Alarm Dismiss", "Run Step", "Stop Profile", "Cycle Reset", "Time Reset", "Time Reset All", "Time Set", "Tare CTs", "Save Profile", "Open Profile", "Get Profiles", "Update Screen", "Update Controls", "Save App Config", "Write Outputs", "Disable Background", "Enable Background", "Get/Release Control", "Log Fuel Change", "Fuel Change Popup", "Read Inputs", "Remote Timer Reset", "Controller Change", "Get Alarms", "Init Alarms", "Save Alarms", "Voltage Selection", "Set Watlow Temp 1", "Set Watlow Temp 2", "Get Pressure", "Write Tare Pressure", "Adjust Controls", "Reinit ADC", "Write Initial Times", "Write Pumps Present", "HMI Command", "Save Pump Times", "Check Pump Stop Time", "Save LS App Config", "Init Data File", "Reset LS Cycles", "Reset Anomalies", "Reset Opens", "Save LS Data", "Save LS Test Data", "Check Serial Numbers", "Main Tab", "Allow Data Note", "Resume Profile", "Pause Profile", "Allow Pause Note", "Clear Graph"]
              n223 = Unbundle By Name(w755) -> ("LS App Config.Data File Name:"=w751:string)
              n224 = Not Equal?(x=w751, y="Data File Name:") -> (x != y?=w750:bool)
              n225 = Bundle By Name(cluster=w754, "LS App Config.Data File Name:"="Data File Name:") -> (w753:T25)
            }
            frame 59 {
              w759 = T14[] [enum."Save LS App Config"] items=["Main", "Init Files", "Init", "Unused", "Save As", "Start Profile", "Check Step Time", "Alarm", "Alarm Dismiss", "Run Step", "Stop Profile", "Cycle Reset", "Time Reset", "Time Reset All", "Time Set", "Tare CTs", "Save Profile", "Open Profile", "Get Profiles", "Update Screen", "Update Controls", "Save App Config", "Write Outputs", "Disable Background", "Enable Background", "Get/Release Control", "Log Fuel Change", "Fuel Change Popup", "Read Inputs", "Remote Timer Reset", "Controller Change", "Get Alarms", "Init Alarms", "Save Alarms", "Voltage Selection", "Set Watlow Temp 1", "Set Watlow Temp 2", "Get Pressure", "Write Tare Pressure", "Adjust Controls", "Reinit ADC", "Write Initial Times", "Write Pumps Present", "HMI Command", "Save Pump Times", "Check Pump Stop Time", "Save LS App Config", "Init Data File", "Reset LS Cycles", "Reset Anomalies", "Reset Opens", "Save LS Data", "Save LS Test Data", "Check Serial Numbers", "Main Tab", "Allow Data Note", "Resume Profile", "Pause Profile", "Allow Pause Note", "Clear Graph"]
              n226 = Unbundle By Name(w762) -> ("LS App Config.Record Bursts"=w758:bool)
              n227 = Not Equal?(x=w758, y="Record During Profile") -> (x != y?=w757:bool)
              n228 = Bundle By Name(cluster=w761, "LS App Config.Record Bursts"="Record During Profile") -> (w760:T25)
            }
            frame 60 {
              w766 = T14[] [enum."Save LS App Config"] items=["Main", "Init Files", "Init", "Unused", "Save As", "Start Profile", "Check Step Time", "Alarm", "Alarm Dismiss", "Run Step", "Stop Profile", "Cycle Reset", "Time Reset", "Time Reset All", "Time Set", "Tare CTs", "Save Profile", "Open Profile", "Get Profiles", "Update Screen", "Update Controls", "Save App Config", "Write Outputs", "Disable Background", "Enable Background", "Get/Release Control", "Log Fuel Change", "Fuel Change Popup", "Read Inputs", "Remote Timer Reset", "Controller Change", "Get Alarms", "Init Alarms", "Save Alarms", "Voltage Selection", "Set Watlow Temp 1", "Set Watlow Temp 2", "Get Pressure", "Write Tare Pressure", "Adjust Controls", "Reinit ADC", "Write Initial Times", "Write Pumps Present", "HMI Command", "Save Pump Times", "Check Pump Stop Time", "Save LS App Config", "Init Data File", "Reset LS Cycles", "Reset Anomalies", "Reset Opens", "Save LS Data", "Save LS Test Data", "Check Serial Numbers", "Main Tab", "Allow Data Note", "Resume Profile", "Pause Profile", "Allow Pause Note", "Clear Graph"]
              n229 = Unbundle By Name(w769) -> ("LS App Config.RecInterval(s)"=w765:i32)
              n230 = Not Equal?(x=w765, y="Interval Between\nRecordings (s):") -> (x != y?=w764:bool)
              n231 = Bundle By Name(cluster=w768, "LS App Config.RecInterval(s)"="Interval Between\nRecordings (s):") -> (w767:T25)
            }
            frame 61 {
              w773 = T14[] [enum."Save LS App Config"] items=["Main", "Init Files", "Init", "Unused", "Save As", "Start Profile", "Check Step Time", "Alarm", "Alarm Dismiss", "Run Step", "Stop Profile", "Cycle Reset", "Time Reset", "Time Reset All", "Time Set", "Tare CTs", "Save Profile", "Open Profile", "Get Profiles", "Update Screen", "Update Controls", "Save App Config", "Write Outputs", "Disable Background", "Enable Background", "Get/Release Control", "Log Fuel Change", "Fuel Change Popup", "Read Inputs", "Remote Timer Reset", "Controller Change", "Get Alarms", "Init Alarms", "Save Alarms", "Voltage Selection", "Set Watlow Temp 1", "Set Watlow Temp 2", "Get Pressure", "Write Tare Pressure", "Adjust Controls", "Reinit ADC", "Write Initial Times", "Write Pumps Present", "HMI Command", "Save Pump Times", "Check Pump Stop Time", "Save LS App Config", "Init Data File", "Reset LS Cycles", "Reset Anomalies", "Reset Opens", "Save LS Data", "Save LS Test Data", "Check Serial Numbers", "Main Tab", "Allow Data Note", "Resume Profile", "Pause Profile", "Allow Pause Note", "Clear Graph"]
              n232 = Unbundle By Name(w776) -> ("LS App Config.RecDuration(s)"=w772:i32)
              n233 = Not Equal?(x=w772, y="Recording\nDuration (s):") -> (x != y?=w771:bool)
              n234 = Bundle By Name(cluster=w775, "LS App Config.RecDuration(s)"="Recording\nDuration (s):") -> (w774:T25)
            }
            frame 62 {
              w780 = T14[] [enum."Save LS App Config"] items=["Main", "Init Files", "Init", "Unused", "Save As", "Start Profile", "Check Step Time", "Alarm", "Alarm Dismiss", "Run Step", "Stop Profile", "Cycle Reset", "Time Reset", "Time Reset All", "Time Set", "Tare CTs", "Save Profile", "Open Profile", "Get Profiles", "Update Screen", "Update Controls", "Save App Config", "Write Outputs", "Disable Background", "Enable Background", "Get/Release Control", "Log Fuel Change", "Fuel Change Popup", "Read Inputs", "Remote Timer Reset", "Controller Change", "Get Alarms", "Init Alarms", "Save Alarms", "Voltage Selection", "Set Watlow Temp 1", "Set Watlow Temp 2", "Get Pressure", "Write Tare Pressure", "Adjust Controls", "Reinit ADC", "Write Initial Times", "Write Pumps Present", "HMI Command", "Save Pump Times", "Check Pump Stop Time", "Save LS App Config", "Init Data File", "Reset LS Cycles", "Reset Anomalies", "Reset Opens", "Save LS Data", "Save LS Test Data", "Check Serial Numbers", "Main Tab", "Allow Data Note", "Resume Profile", "Pause Profile", "Allow Pause Note", "Clear Graph"]
              n235 = Unbundle By Name(w783) -> ("LS App Config.RecFrequeny (Hz)"=w779:i32)
              n236 = Not Equal?(x=w779, y="Recording\nFrequency (Hz):") -> (x != y?=w778:bool)
              n237 = Bundle By Name(cluster=w782, "LS App Config.RecFrequeny (Hz)"="Recording\nFrequency (Hz):") -> (w781:T25)
            }
            frame 63 {
              w787 = T14[] [enum."Save LS App Config", enum."Write Outputs"] items=["Main", "Init Files", "Init", "Unused", "Save As", "Start Profile", "Check Step Time", "Alarm", "Alarm Dismiss", "Run Step", "Stop Profile", "Cycle Reset", "Time Reset", "Time Reset All", "Time Set", "Tare CTs", "Save Profile", "Open Profile", "Get Profiles", "Update Screen", "Update Controls", "Save App Config", "Write Outputs", "Disable Background", "Enable Background", "Get/Release Control", "Log Fuel Change", "Fuel Change Popup", "Read Inputs", "Remote Timer Reset", "Controller Change", "Get Alarms", "Init Alarms", "Save Alarms", "Voltage Selection", "Set Watlow Temp 1", "Set Watlow Temp 2", "Get Pressure", "Write Tare Pressure", "Adjust Controls", "Reinit ADC", "Write Initial Times", "Write Pumps Present", "HMI Command", "Save Pump Times", "Check Pump Stop Time", "Save LS App Config", "Init Data File", "Reset LS Cycles", "Reset Anomalies", "Reset Opens", "Save LS Data", "Save LS Test Data", "Check Serial Numbers", "Main Tab", "Allow Data Note", "Resume Profile", "Pause Profile", "Allow Pause Note", "Clear Graph"]
              n238 = Unbundle By Name(w790) -> ("LS App Config.DetectionMode"=w786:i32)
              n239 = Not Equal?(x=w786, y="Detection Mode:") -> (x != y?=w785:bool)
              n240 = case shown="True" w785 {
                tunnel: "Detection Mode:" -> [_ w791]
                frame False {
                }
                frame True {
                  n241 = case shown="0, Default" w791 {
                    frame 0, Default {
                      n242 = local write "Live Data Tab"(enum32{"Page 1", "Page 2", "Page 3"}."Page 2" ("Live Data Tab")) -> ()
                    }
                    frame 1 {
                      n243 = local write "Live Data Tab"(enum32{"Page 1", "Page 2", "Page 3"}."Page 3" ("Live Data Tab")) -> ()
                    }
                  }
                }
              }
              n244 = Bundle By Name(cluster=w789, "LS App Config.DetectionMode"="Detection Mode:") -> (w788:T25)
            }
            frame 64 {
              w799 = T14[] [enum."Check Serial Numbers", enum."Save LS App Config"] items=["Main", "Init Files", "Init", "Unused", "Save As", "Start Profile", "Check Step Time", "Alarm", "Alarm Dismiss", "Run Step", "Stop Profile", "Cycle Reset", "Time Reset", "Time Reset All", "Time Set", "Tare CTs", "Save Profile", "Open Profile", "Get Profiles", "Update Screen", "Update Controls", "Save App Config", "Write Outputs", "Disable Background", "Enable Background", "Get/Release Control", "Log Fuel Change", "Fuel Change Popup", "Read Inputs", "Remote Timer Reset", "Controller Change", "Get Alarms", "Init Alarms", "Save Alarms", "Voltage Selection", "Set Watlow Temp 1", "Set Watlow Temp 2", "Get Pressure", "Write Tare Pressure", "Adjust Controls", "Reinit ADC", "Write Initial Times", "Write Pumps Present", "HMI Command", "Save Pump Times", "Check Pump Stop Time", "Save LS App Config", "Init Data File", "Reset LS Cycles", "Reset Anomalies", "Reset Opens", "Save LS Data", "Save LS Test Data", "Check Serial Numbers", "Main Tab", "Allow Data Note", "Resume Profile", "Pause Profile", "Allow Pause Note", "Clear Graph"]
              n245 = Unbundle By Name(w802) -> ("LS App Config.Serial Numbers"=w798:string[])
              n246 = Cluster To Array(cluster="LS Serial Numbers") -> (array=w796:string[])
              n247 = Not Equal?(x=w798, y=w796) -> (x != y?=w795:bool[])
              n248 = Or Array Elements(Boolean array=w795) -> (logical OR=w794:bool)
              n249 = Bundle By Name(cluster=w801, "LS App Config.Serial Numbers"=w796) -> (w800:T25)
            }
            frame 65 {
              w806 = T14[] [enum."Write Outputs"] items=["Main", "Init Files", "Init", "Unused", "Save As", "Start Profile", "Check Step Time", "Alarm", "Alarm Dismiss", "Run Step", "Stop Profile", "Cycle Reset", "Time Reset", "Time Reset All", "Time Set", "Tare CTs", "Save Profile", "Open Profile", "Get Profiles", "Update Screen", "Update Controls", "Save App Config", "Write Outputs", "Disable Background", "Enable Background", "Get/Release Control", "Log Fuel Change", "Fuel Change Popup", "Read Inputs", "Remote Timer Reset", "Controller Change", "Get Alarms", "Init Alarms", "Save Alarms", "Voltage Selection", "Set Watlow Temp 1", "Set Watlow Temp 2", "Get Pressure", "Write Tare Pressure", "Adjust Controls", "Reinit ADC", "Write Initial Times", "Write Pumps Present", "HMI Command", "Save Pump Times", "Check Pump Stop Time", "Save LS App Config", "Init Data File", "Reset LS Cycles", "Reset Anomalies", "Reset Opens", "Save LS Data", "Save LS Test Data", "Check Serial Numbers", "Main Tab", "Allow Data Note", "Resume Profile", "Pause Profile", "Allow Pause Note", "Clear Graph"]
              n250 = Unbundle By Name(w809) -> ("Bank 1 State:"=w805:u16)
              n251 = Not Equal?(x=w805, y="Bank 1 Power State:") -> (x != y?=w803:bool)
              n252 = Bundle By Name(cluster=w808, "Bank 1 State:"="Bank 1 Power State:") -> (w807:T25)
            }
            frame 66 {
              w813 = T14[] [enum."Write Outputs"] items=["Main", "Init Files", "Init", "Unused", "Save As", "Start Profile", "Check Step Time", "Alarm", "Alarm Dismiss", "Run Step", "Stop Profile", "Cycle Reset", "Time Reset", "Time Reset All", "Time Set", "Tare CTs", "Save Profile", "Open Profile", "Get Profiles", "Update Screen", "Update Controls", "Save App Config", "Write Outputs", "Disable Background", "Enable Background", "Get/Release Control", "Log Fuel Change", "Fuel Change Popup", "Read Inputs", "Remote Timer Reset", "Controller Change", "Get Alarms", "Init Alarms", "Save Alarms", "Voltage Selection", "Set Watlow Temp 1", "Set Watlow Temp 2", "Get Pressure", "Write Tare Pressure", "Adjust Controls", "Reinit ADC", "Write Initial Times", "Write Pumps Present", "HMI Command", "Save Pump Times", "Check Pump Stop Time", "Save LS App Config", "Init Data File", "Reset LS Cycles", "Reset Anomalies", "Reset Opens", "Save LS Data", "Save LS Test Data", "Check Serial Numbers", "Main Tab", "Allow Data Note", "Resume Profile", "Pause Profile", "Allow Pause Note", "Clear Graph"]
              n253 = Unbundle By Name(w816) -> ("Bank 2 State:"=w812:u16)
              n254 = Not Equal?(x=w812, y="Bank 2 Power State:") -> (x != y?=w811:bool)
              n255 = Bundle By Name(cluster=w815, "Bank 2 State:"="Bank 2 Power State:") -> (w814:T25)
            }
            frame 67 {
              w819 = T14[] [enum."Reset LS Cycles"] items=["Main", "Init Files", "Init", "Unused", "Save As", "Start Profile", "Check Step Time", "Alarm", "Alarm Dismiss", "Run Step", "Stop Profile", "Cycle Reset", "Time Reset", "Time Reset All", "Time Set", "Tare CTs", "Save Profile", "Open Profile", "Get Profiles", "Update Screen", "Update Controls", "Save App Config", "Write Outputs", "Disable Background", "Enable Background", "Get/Release Control", "Log Fuel Change", "Fuel Change Popup", "Read Inputs", "Remote Timer Reset", "Controller Change", "Get Alarms", "Init Alarms", "Save Alarms", "Voltage Selection", "Set Watlow Temp 1", "Set Watlow Temp 2", "Get Pressure", "Write Tare Pressure", "Adjust Controls", "Reinit ADC", "Write Initial Times", "Write Pumps Present", "HMI Command", "Save Pump Times", "Check Pump Stop Time", "Save LS App Config", "Init Data File", "Reset LS Cycles", "Reset Anomalies", "Reset Opens", "Save LS Data", "Save LS Test Data", "Check Serial Numbers", "Main Tab", "Allow Data Note", "Resume Profile", "Pause Profile", "Allow Pause Note", "Clear Graph"]
            }
            frame 68 {
              w822 = T14[] [enum."Reset Anomalies"] items=["Main", "Init Files", "Init", "Unused", "Save As", "Start Profile", "Check Step Time", "Alarm", "Alarm Dismiss", "Run Step", "Stop Profile", "Cycle Reset", "Time Reset", "Time Reset All", "Time Set", "Tare CTs", "Save Profile", "Open Profile", "Get Profiles", "Update Screen", "Update Controls", "Save App Config", "Write Outputs", "Disable Background", "Enable Background", "Get/Release Control", "Log Fuel Change", "Fuel Change Popup", "Read Inputs", "Remote Timer Reset", "Controller Change", "Get Alarms", "Init Alarms", "Save Alarms", "Voltage Selection", "Set Watlow Temp 1", "Set Watlow Temp 2", "Get Pressure", "Write Tare Pressure", "Adjust Controls", "Reinit ADC", "Write Initial Times", "Write Pumps Present", "HMI Command", "Save Pump Times", "Check Pump Stop Time", "Save LS App Config", "Init Data File", "Reset LS Cycles", "Reset Anomalies", "Reset Opens", "Save LS Data", "Save LS Test Data", "Check Serial Numbers", "Main Tab", "Allow Data Note", "Resume Profile", "Pause Profile", "Allow Pause Note", "Clear Graph"]
            }
            frame 69 {
              w825 = T14[] [enum."Reset Opens"] items=["Main", "Init Files", "Init", "Unused", "Save As", "Start Profile", "Check Step Time", "Alarm", "Alarm Dismiss", "Run Step", "Stop Profile", "Cycle Reset", "Time Reset", "Time Reset All", "Time Set", "Tare CTs", "Save Profile", "Open Profile", "Get Profiles", "Update Screen", "Update Controls", "Save App Config", "Write Outputs", "Disable Background", "Enable Background", "Get/Release Control", "Log Fuel Change", "Fuel Change Popup", "Read Inputs", "Remote Timer Reset", "Controller Change", "Get Alarms", "Init Alarms", "Save Alarms", "Voltage Selection", "Set Watlow Temp 1", "Set Watlow Temp 2", "Get Pressure", "Write Tare Pressure", "Adjust Controls", "Reinit ADC", "Write Initial Times", "Write Pumps Present", "HMI Command", "Save Pump Times", "Check Pump Stop Time", "Save LS App Config", "Init Data File", "Reset LS Cycles", "Reset Anomalies", "Reset Opens", "Save LS Data", "Save LS Test Data", "Check Serial Numbers", "Main Tab", "Allow Data Note", "Resume Profile", "Pause Profile", "Allow Pause Note", "Clear Graph"]
            }
            frame 70 {
              w827 = T14[] [enum."Init Data File", enum."Save LS App Config"] items=["Main", "Init Files", "Init", "Unused", "Save As", "Start Profile", "Check Step Time", "Alarm", "Alarm Dismiss", "Run Step", "Stop Profile", "Cycle Reset", "Time Reset", "Time Reset All", "Time Set", "Tare CTs", "Save Profile", "Open Profile", "Get Profiles", "Update Screen", "Update Controls", "Save App Config", "Write Outputs", "Disable Background", "Enable Background", "Get/Release Control", "Log Fuel Change", "Fuel Change Popup", "Read Inputs", "Remote Timer Reset", "Controller Change", "Get Alarms", "Init Alarms", "Save Alarms", "Voltage Selection", "Set Watlow Temp 1", "Set Watlow Temp 2", "Get Pressure", "Write Tare Pressure", "Adjust Controls", "Reinit ADC", "Write Initial Times", "Write Pumps Present", "HMI Command", "Save Pump Times", "Check Pump Stop Time", "Save LS App Config", "Init Data File", "Reset LS Cycles", "Reset Anomalies", "Reset Opens", "Save LS Data", "Save LS Test Data", "Check Serial Numbers", "Main Tab", "Allow Data Note", "Resume Profile", "Pause Profile", "Allow Pause Note", "Clear Graph"]
              n256 = Unbundle By Name(w830) -> ("day of month"=w829:i32)
              n257 = Get Date/Time In Seconds() -> (seconds since 1Jan1904=w833:timestamp)
              n258 = Seconds To Date/Time(time stamp (now)=w833) -> (date time rec=w834:T46)  [unwired: 1 in]
              n259 = Unbundle By Name(w834) -> ("day of month"=w826:i32)
              n260 = Not Equal?(x=w829, y=w826) -> (x != y?=w828:bool)
              n261 = Bundle By Name(cluster=w832, "day of month"=w826) -> (w831:T25)
            }
            frame 71 {
              w835 = T14[] [enum."Save App Config", enum."Write Outputs"] items=["Main", "Init Files", "Init", "Unused", "Save As", "Start Profile", "Check Step Time", "Alarm", "Alarm Dismiss", "Run Step", "Stop Profile", "Cycle Reset", "Time Reset", "Time Reset All", "Time Set", "Tare CTs", "Save Profile", "Open Profile", "Get Profiles", "Update Screen", "Update Controls", "Save App Config", "Write Outputs", "Disable Background", "Enable Background", "Get/Release Control", "Log Fuel Change", "Fuel Change Popup", "Read Inputs", "Remote Timer Reset", "Controller Change", "Get Alarms", "Init Alarms", "Save Alarms", "Voltage Selection", "Set Watlow Temp 1", "Set Watlow Temp 2", "Get Pressure", "Write Tare Pressure", "Adjust Controls", "Reinit ADC", "Write Initial Times", "Write Pumps Present", "HMI Command", "Save Pump Times", "Check Pump Stop Time", "Save LS App Config", "Init Data File", "Reset LS Cycles", "Reset Anomalies", "Reset Opens", "Save LS Data", "Save LS Test Data", "Check Serial Numbers", "Main Tab", "Allow Data Note", "Resume Profile", "Pause Profile", "Allow Pause Note", "Clear Graph"]
              n262 = Unbundle By Name(w840) -> ("App Config.Anomaly Threshold:"=w841:dbl)
              n263 = Not Equal?(x=w841, y="Anomaly Threshold:") -> (x != y?=w837:bool)
              n264 = Bundle By Name(cluster=w839, "App Config.Anomaly Threshold:"="Anomaly Threshold:") -> (w838:T25)
            }
            frame 72 {
              w842 = T14[] [enum."Save LS App Config"] items=["Main", "Init Files", "Init", "Unused", "Save As", "Start Profile", "Check Step Time", "Alarm", "Alarm Dismiss", "Run Step", "Stop Profile", "Cycle Reset", "Time Reset", "Time Reset All", "Time Set", "Tare CTs", "Save Profile", "Open Profile", "Get Profiles", "Update Screen", "Update Controls", "Save App Config", "Write Outputs", "Disable Background", "Enable Background", "Get/Release Control", "Log Fuel Change", "Fuel Change Popup", "Read Inputs", "Remote Timer Reset", "Controller Change", "Get Alarms", "Init Alarms", "Save Alarms", "Voltage Selection", "Set Watlow Temp 1", "Set Watlow Temp 2", "Get Pressure", "Write Tare Pressure", "Adjust Controls", "Reinit ADC", "Write Initial Times", "Write Pumps Present", "HMI Command", "Save Pump Times", "Check Pump Stop Time", "Save LS App Config", "Init Data File", "Reset LS Cycles", "Reset Anomalies", "Reset Opens", "Save LS Data", "Save LS Test Data", "Check Serial Numbers", "Main Tab", "Allow Data Note", "Resume Profile", "Pause Profile", "Allow Pause Note", "Clear Graph"]
              n265 = Unbundle By Name(w847) -> ("LS App Config.Record Constant"=w848:bool)
              n266 = Not Equal?(x=w848, y="Record Constant") -> (x != y?=w844:bool)
              n267 = Bundle By Name(cluster=w846, "LS App Config.Record Constant"="Record Constant") -> (w845:T25)
            }
            frame 73 {
              w851 = T14[] [] items=["Main", "Init Files", "Init", "Unused", "Save As", "Start Profile", "Check Step Time", "Alarm", "Alarm Dismiss", "Run Step", "Stop Profile", "Cycle Reset", "Time Reset", "Time Reset All", "Time Set", "Tare CTs", "Save Profile", "Open Profile", "Get Profiles", "Update Screen", "Update Controls", "Save App Config", "Write Outputs", "Disable Background", "Enable Background", "Get/Release Control", "Log Fuel Change", "Fuel Change Popup", "Read Inputs", "Remote Timer Reset", "Controller Change", "Get Alarms", "Init Alarms", "Save Alarms", "Voltage Selection", "Set Watlow Temp 1", "Set Watlow Temp 2", "Get Pressure", "Write Tare Pressure", "Adjust Controls", "Reinit ADC", "Write Initial Times", "Write Pumps Present", "HMI Command", "Save Pump Times", "Check Pump Stop Time", "Save LS App Config", "Init Data File", "Reset LS Cycles", "Reset Anomalies", "Reset Opens", "Save LS Data", "Save LS Test Data", "Check Serial Numbers", "Main Tab", "Allow Data Note", "Resume Profile", "Pause Profile", "Allow Pause Note", "Clear Graph"]
              n268 = call "LS Data Global.vi"() -> ("Recording Out"=→"Recording":bool, "Transferring Out"=→"Transferring":bool)  [unwired: 12 in, 2 out]
            }
            frame 74 {
              w855 = T14[] [] items=["Main", "Init Files", "Init", "Unused", "Save As", "Start Profile", "Check Step Time", "Alarm", "Alarm Dismiss", "Run Step", "Stop Profile", "Cycle Reset", "Time Reset", "Time Reset All", "Time Set", "Tare CTs", "Save Profile", "Open Profile", "Get Profiles", "Update Screen", "Update Controls", "Save App Config", "Write Outputs", "Disable Background", "Enable Background", "Get/Release Control", "Log Fuel Change", "Fuel Change Popup", "Read Inputs", "Remote Timer Reset", "Controller Change", "Get Alarms", "Init Alarms", "Save Alarms", "Voltage Selection", "Set Watlow Temp 1", "Set Watlow Temp 2", "Get Pressure", "Write Tare Pressure", "Adjust Controls", "Reinit ADC", "Write Initial Times", "Write Pumps Present", "HMI Command", "Save Pump Times", "Check Pump Stop Time", "Save LS App Config", "Init Data File", "Reset LS Cycles", "Reset Anomalies", "Reset Opens", "Save LS Data", "Save LS Test Data", "Check Serial Numbers", "Main Tab", "Allow Data Note", "Resume Profile", "Pause Profile", "Allow Pause Note", "Clear Graph"]
            }
            frame 75 {
              w860 = T14[] [enum."Save LS App Config", enum."Write Outputs"] items=["Main", "Init Files", "Init", "Unused", "Save As", "Start Profile", "Check Step Time", "Alarm", "Alarm Dismiss", "Run Step", "Stop Profile", "Cycle Reset", "Time Reset", "Time Reset All", "Time Set", "Tare CTs", "Save Profile", "Open Profile", "Get Profiles", "Update Screen", "Update Controls", "Save App Config", "Write Outputs", "Disable Background", "Enable Background", "Get/Release Control", "Log Fuel Change", "Fuel Change Popup", "Read Inputs", "Remote Timer Reset", "Controller Change", "Get Alarms", "Init Alarms", "Save Alarms", "Voltage Selection", "Set Watlow Temp 1", "Set Watlow Temp 2", "Get Pressure", "Write Tare Pressure", "Adjust Controls", "Reinit ADC", "Write Initial Times", "Write Pumps Present", "HMI Command", "Save Pump Times", "Check Pump Stop Time", "Save LS App Config", "Init Data File", "Reset LS Cycles", "Reset Anomalies", "Reset Opens", "Save LS Data", "Save LS Test Data", "Check Serial Numbers", "Main Tab", "Allow Data Note", "Resume Profile", "Pause Profile", "Allow Pause Note", "Clear Graph"]
              n269 = Unbundle By Name(w862) -> ("LS App Config.Bias Resistances"=w861:dbl[])
              n270 = Not Equal?(x=w861, y="Bias Resistances") -> (x != y?=w858:bool[])
              n271 = Or Array Elements(Boolean array=w858) -> (logical OR=w857:bool)
              n272 = Bundle By Name(cluster=w864, "LS App Config.Bias Resistances"="Bias Resistances") -> (w863:T25)
            }
            frame 76 {
              w867 = T14[] [enum."Save LS App Config", enum."Write Outputs"] items=["Main", "Init Files", "Init", "Unused", "Save As", "Start Profile", "Check Step Time", "Alarm", "Alarm Dismiss", "Run Step", "Stop Profile", "Cycle Reset", "Time Reset", "Time Reset All", "Time Set", "Tare CTs", "Save Profile", "Open Profile", "Get Profiles", "Update Screen", "Update Controls", "Save App Config", "Write Outputs", "Disable Background", "Enable Background", "Get/Release Control", "Log Fuel Change", "Fuel Change Popup", "Read Inputs", "Remote Timer Reset", "Controller Change", "Get Alarms", "Init Alarms", "Save Alarms", "Voltage Selection", "Set Watlow Temp 1", "Set Watlow Temp 2", "Get Pressure", "Write Tare Pressure", "Adjust Controls", "Reinit ADC", "Write Initial Times", "Write Pumps Present", "HMI Command", "Save Pump Times", "Check Pump Stop Time", "Save LS App Config", "Init Data File", "Reset LS Cycles", "Reset Anomalies", "Reset Opens", "Save LS Data", "Save LS Test Data", "Check Serial Numbers", "Main Tab", "Allow Data Note", "Resume Profile", "Pause Profile", "Allow Pause Note", "Clear Graph"]
              n273 = Unbundle By Name(w869) -> ("LS App Config.Voltage(T)/Resistance(F)"=w868:bool)
              n274 = Not Equal?(x=w868, y="Voltage(T)/Resistance(F)") -> (x != y?=w866:bool)
              n275 = Bundle By Name(cluster=w871, "LS App Config.Voltage(T)/Resistance(F)"="Voltage(T)/Resistance(F)") -> (w870:T25)
            }
            frame 77 {
              w875 = T14[] [enum."Pause Profile", enum."Save LS Data"] items=["Main", "Init Files", "Init", "Unused", "Save As", "Start Profile", "Check Step Time", "Alarm", "Alarm Dismiss", "Run Step", "Stop Profile", "Cycle Reset", "Time Reset", "Time Reset All", "Time Set", "Tare CTs", "Save Profile", "Open Profile", "Get Profiles", "Update Screen", "Update Controls", "Save App Config", "Write Outputs", "Disable Background", "Enable Background", "Get/Release Control", "Log Fuel Change", "Fuel Change Popup", "Read Inputs", "Remote Timer Reset", "Controller Change", "Get Alarms", "Init Alarms", "Save Alarms", "Voltage Selection", "Set Watlow Temp 1", "Set Watlow Temp 2", "Get Pressure", "Write Tare Pressure", "Adjust Controls", "Reinit ADC", "Write Initial Times", "Write Pumps Present", "HMI Command", "Save Pump Times", "Check Pump Stop Time", "Save LS App Config", "Init Data File", "Reset LS Cycles", "Reset Anomalies", "Reset Opens", "Save LS Data", "Save LS Test Data", "Check Serial Numbers", "Main Tab", "Allow Data Note", "Resume Profile", "Pause Profile", "Allow Pause Note", "Clear Graph"]
              w874 = T14[] [enum."Voltage Selection", enum."Resume Profile"] items=["Main", "Init Files", "Init", "Unused", "Save As", "Start Profile", "Check Step Time", "Alarm", "Alarm Dismiss", "Run Step", "Stop Profile", "Cycle Reset", "Time Reset", "Time Reset All", "Time Set", "Tare CTs", "Save Profile", "Open Profile", "Get Profiles", "Update Screen", "Update Controls", "Save App Config", "Write Outputs", "Disable Background", "Enable Background", "Get/Release Control", "Log Fuel Change", "Fuel Change Popup", "Read Inputs", "Remote Timer Reset", "Controller Change", "Get Alarms", "Init Alarms", "Save Alarms", "Voltage Selection", "Set Watlow Temp 1", "Set Watlow Temp 2", "Get Pressure", "Write Tare Pressure", "Adjust Controls", "Reinit ADC", "Write Initial Times", "Write Pumps Present", "HMI Command", "Save Pump Times", "Check Pump Stop Time", "Save LS App Config", "Init Data File", "Reset LS Cycles", "Reset Anomalies", "Reset Opens", "Save LS Data", "Save LS Test Data", "Check Serial Numbers", "Main Tab", "Allow Data Note", "Resume Profile", "Pause Profile", "Allow Pause Note", "Clear Graph"]
              # "T:Pause\nF:Resume"
              n276 = Unbundle By Name(w878) -> ("Pause Test"=w877:bool)
              n277 = Not Equal?(x=w877, y="pb.Pause/Resume") -> (x != y?=w876:bool)
              n278 = Select(t=w875, s="pb.Pause/Resume", f=w874) -> (s? t:f=w872:T14[])
              n279 = Bundle By Name(cluster=w880, "Pause Test"="pb.Pause/Resume") -> (w879:T25)
            }
            frame 78 {
              w881 = T14[] [enum."Save App Config", enum."Write Outputs"] items=["Main", "Init Files", "Init", "Unused", "Save As", "Start Profile", "Check Step Time", "Alarm", "Alarm Dismiss", "Run Step", "Stop Profile", "Cycle Reset", "Time Reset", "Time Reset All", "Time Set", "Tare CTs", "Save Profile", "Open Profile", "Get Profiles", "Update Screen", "Update Controls", "Save App Config", "Write Outputs", "Disable Background", "Enable Background", "Get/Release Control", "Log Fuel Change", "Fuel Change Popup", "Read Inputs", "Remote Timer Reset", "Controller Change", "Get Alarms", "Init Alarms", "Save Alarms", "Voltage Selection", "Set Watlow Temp 1", "Set Watlow Temp 2", "Get Pressure", "Write Tare Pressure", "Adjust Controls", "Reinit ADC", "Write Initial Times", "Write Pumps Present", "HMI Command", "Save Pump Times", "Check Pump Stop Time", "Save LS App Config", "Init Data File", "Reset LS Cycles", "Reset Anomalies", "Reset Opens", "Save LS Data", "Save LS Test Data", "Check Serial Numbers", "Main Tab", "Allow Data Note", "Resume Profile", "Pause Profile", "Allow Pause Note", "Clear Graph"]
              n280 = Unbundle By Name(w885) -> ("App Config.Bank 1 Offset"=w884:dbl)
              n281 = Not Equal?(x=w884, y="Bank 1 Voltage Offset:") -> (x != y?=w883:bool)
              n282 = Bundle By Name(cluster=w887, "App Config.Bank 1 Offset"="Bank 1 Voltage Offset:") -> (w886:T25)
            }
            frame 79 {
              w889 = T14[] [enum."Save App Config", enum."Write Outputs"] items=["Main", "Init Files", "Init", "Unused", "Save As", "Start Profile", "Check Step Time", "Alarm", "Alarm Dismiss", "Run Step", "Stop Profile", "Cycle Reset", "Time Reset", "Time Reset All", "Time Set", "Tare CTs", "Save Profile", "Open Profile", "Get Profiles", "Update Screen", "Update Controls", "Save App Config", "Write Outputs", "Disable Background", "Enable Background", "Get/Release Control", "Log Fuel Change", "Fuel Change Popup", "Read Inputs", "Remote Timer Reset", "Controller Change", "Get Alarms", "Init Alarms", "Save Alarms", "Voltage Selection", "Set Watlow Temp 1", "Set Watlow Temp 2", "Get Pressure", "Write Tare Pressure", "Adjust Controls", "Reinit ADC", "Write Initial Times", "Write Pumps Present", "HMI Command", "Save Pump Times", "Check Pump Stop Time", "Save LS App Config", "Init Data File", "Reset LS Cycles", "Reset Anomalies", "Reset Opens", "Save LS Data", "Save LS Test Data", "Check Serial Numbers", "Main Tab", "Allow Data Note", "Resume Profile", "Pause Profile", "Allow Pause Note", "Clear Graph"]
              n283 = Unbundle By Name(w892) -> ("App Config.Bank 2 Offset"=w891:dbl)
              n284 = Not Equal?(x=w891, y="Bank 2 Voltage Offset:") -> (x != y?=w890:bool)
              n285 = Bundle By Name(cluster=w894, "App Config.Bank 2 Offset"="Bank 2 Voltage Offset:") -> (w893:T25)
            }
          }
        }
        n286 = Tick Count (ms)() -> (millisecond timer value=w87:u32)
        n287 = Subtract(x=w87, y=w89) -> (x-y=w86:u32)
        n288 = Subtract(x=w87, y=w88) -> (x-y=w85:u32)
        n289 = Greater?(x=w86, y=u32 100) -> (0:w81:bool)
        n290 = Greater?(x=w85, y=u32 1000) -> (0:w80:bool)
        n291 = disable-structure shown="Enabled" {
          disable-tunnel: [w103 w104] -> w79
          frame Disabled {
            w103 = T14[] [enum."Update Screen", enum."Save LS Data"] items=["Main", "Init Files", "Init", "Unused", "Save As", "Start Profile", "Check Step Time", "Alarm", "Alarm Dismiss", "Run Step", "Stop Profile", "Cycle Reset", "Time Reset", "Time Reset All", "Time Set", "Tare CTs", "Save Profile", "Open Profile", "Get Profiles", "Update Screen", "Update Controls", "Save App Config", "Write Outputs", "Disable Background", "Enable Background", "Get/Release Control", "Log Fuel Change", "Fuel Change Popup", "Read Inputs", "Remote Timer Reset", "Controller Change", "Get Alarms", "Init Alarms", "Save Alarms", "Voltage Selection", "Set Watlow Temp 1", "Set Watlow Temp 2", "Get Pressure", "Write Tare Pressure", "Adjust Controls", "Reinit ADC", "Write Initial Times", "Write Pumps Present", "HMI Command", "Save Pump Times", "Check Pump Stop Time", "Save LS App Config", "Init Data File", "Reset LS Cycles", "Reset Anomalies", "Reset Opens", "Save LS Data", "Save LS Test Data", "Check Serial Numbers", "Main Tab", "Allow Data Note", "Resume Profile", "Pause Profile", "Allow Pause Note", "Clear Graph"]
          }
          frame Enabled {
            w104 = T14[] [enum."Update Screen"] items=["Main", "Init Files", "Init", "Unused", "Save As", "Start Profile", "Check Step Time", "Alarm", "Alarm Dismiss", "Run Step", "Stop Profile", "Cycle Reset", "Time Reset", "Time Reset All", "Time Set", "Tare CTs", "Save Profile", "Open Profile", "Get Profiles", "Update Screen", "Update Controls", "Save App Config", "Write Outputs", "Disable Background", "Enable Background", "Get/Release Control", "Log Fuel Change", "Fuel Change Popup", "Read Inputs", "Remote Timer Reset", "Controller Change", "Get Alarms", "Init Alarms", "Save Alarms", "Voltage Selection", "Set Watlow Temp 1", "Set Watlow Temp 2", "Get Pressure", "Write Tare Pressure", "Adjust Controls", "Reinit ADC", "Write Initial Times", "Write Pumps Present", "HMI Command", "Save Pump Times", "Check Pump Stop Time", "Save LS App Config", "Init Data File", "Reset LS Cycles", "Reset Anomalies", "Reset Opens", "Save LS Data", "Save LS Test Data", "Check Serial Numbers", "Main Tab", "Allow Data Note", "Resume Profile", "Pause Profile", "Allow Pause Note", "Clear Graph"]
          }
        }
        n292 = case shown="True" w80 {
          tunnel: w90 -> [w105 w109]
          tunnel: w79 -> [_ w108]
          tunnel: [w105 w106] -> w91
          frame False {
          }
          frame True {
            n293 = Insert Into Array(array=w109, index=0, new element=w108) -> (w106:T14[])
          }
        }
        n294 = disable-structure shown="Disabled" {
          frame Disabled {
          }
          frame Enabled {
          }
        }
        n295 = case shown="True" w81 {
          tunnel: w91 -> [w110 w114]
          tunnel: Sequence_States."Read Inputs" -> [_ w113]
          tunnel: [w110 w111] -> w94
          frame False {
          }
          frame True {
            n296 = Insert Into Array(array=w114, index=0, new element=w113) -> (w111:T14[])
          }
        }
        n297 = case shown="True" w82 {
          tunnel: w94 -> [w115 w119]
          tunnel: Sequence_States."Check Step Time" -> [_ w118]
          tunnel: [w115 w116] -> w95
          frame False {
          }
          frame True {
            n298 = Insert Into Array(array=w119, index=0, new element=w118) -> (w116:T14[])
          }
        }
        n299 = case shown="True" w97 {
          tunnel: w95 -> [w120 w124]
          tunnel: w98 -> [_ w123]
          tunnel: [w120 w121] -> w96
          frame False {
          }
          frame True {
            n300 = Insert Into Array(array=w124, index=0, new element=w123) -> (w121:T14[])
          }
        }
      }
      frame "Init Files" {
        w936 = T14[] [enum."Write Tare Pressure", enum."Write Initial Times", enum."Write Pumps Present"] items=["Main", "Init Files", "Init", "Unused", "Save As", "Start Profile", "Check Step Time", "Alarm", "Alarm Dismiss", "Run Step", "Stop Profile", "Cycle Reset", "Time Reset", "Time Reset All", "Time Set", "Tare CTs", "Save Profile", "Open Profile", "Get Profiles", "Update Screen", "Update Controls", "Save App Config", "Write Outputs", "Disable Background", "Enable Background", "Get/Release Control", "Log Fuel Change", "Fuel Change Popup", "Read Inputs", "Remote Timer Reset", "Controller Change", "Get Alarms", "Init Alarms", "Save Alarms", "Voltage Selection", "Set Watlow Temp 1", "Set Watlow Temp 2", "Get Pressure", "Write Tare Pressure", "Adjust Controls", "Reinit ADC", "Write Initial Times", "Write Pumps Present", "HMI Command", "Save Pump Times", "Check Pump Stop Time", "Save LS App Config", "Init Data File", "Reset LS Cycles", "Reset Anomalies", "Reset Opens", "Save LS Data", "Save LS Test Data", "Check Serial Numbers", "Main Tab", "Allow Data Note", "Resume Profile", "Pause Profile", "Allow Pause Note", "Clear Graph"]
        w945 = dbl[][] [[0.0, 11.0, 0.0, 0.0, 0.0], [0.0, 11.0, 0.0, 0.0, 0.0], [0.0, 11.0, 0.0, 0.0, 0.0], [0.0, 11.0, 0.0, 0.0, 0.0], [0.0, 11.0, 0.0, 0.0, 0.0], [0.0, 11.0, 0.0, 0.0, 0.0], [0.0, 1.0, 0.0, 0.0, 0.0], [0.0, 1.0, 0.0, 0.0, 0.0], [0.0, 1.0, 0.0, 0.0, 0.0], [0.0, 2.0, 0.0, 0.0, 0.0], [0.0, 1.0, 0.0, 0.0, 0.0], [0.0, 1.0, 0.0, 0.0, 0.0], [0.0, 1.0, 0.0, 0.0, 0.0], [0.0, 1.0, 0.0, 0.0, 0.0], [0.0, 1.0, 0.0, 0.0, 0.0], [0.0, 1.0, 0.0, 0.0, 0.0], [0.0, 1.0, 0.0, 0.0, 0.0], [0.0, 1.0, 0.0, 0.0, 0.0], [0.0, 1.0, 0.0, 0.0, 0.0], [0.0, 1.0, 0.0, 0.0, 0.0], [0.0, 1.0, 0.0, 0.0, 0.0], [0.0, 1.0, 0.0, 0.0, 0.0], [-60.0, 24.0, 0.0, 0.0, 0.0], [-60.0, 24.0, 0.0, 0.0, 0.0], [-60.0, 24.0, 0.0, 0.0, 0.0], [-60.0, 24.0, 0.0, 0.0, 0.0], [-60.0, 24.0, 0.0, 0.0, 0.0], [-60.0, 24.0, 0.0, 0.0, 0.0], [-660.0, 200.0, 0.0, 0.0, 0.0], [-660.0, 200.0, 0.0, 0.0, 0.0], [-258.5, 258.5, 0.0, 0.0, 0.0], [-258.5, 258.5, 0.0, 0.0, 0.0], [-258.5, 258.5, 0.0, 0.0, 0.0], [-258.5, 258.5, 0.0, 0.0, 0.0], [-258.5, 258.5, 0.0, 0.0, 0.0], [-258.5, 258.5, 0.0, 0.0, 0.0], [-150.0, 150.0, 0.0, 0.0, 0.0], [-150.0, 150.0, 0.0, 0.0, 0.0], [-150.0, 150.0, 0.0, 0.0, 0.0], [-150.0, 150.0, 0.0, 0.0, 0.0], [-150.0, 150.0, 0.0, 0.0, 0.0], [-150.0, 150.0, 0.0, 0.0, 0.0], [0.0, 1.0, 0.0, 0.0, 0.0], [0.0, 1.0, 0.0, 0.0, 0.0], [0.0, 1.0, 0.0, 0.0, 0.0], [0.0, 1.0, 0.0, 0.0, 0.0], [0.0, 1.0, 0.0, 0.0, 0.0], [0.0, 1.0, 0.0, 0.0, 0.0], [0.0, 11.0, 0.0, 0.0, 0.0], [0.0, 11.0, 0.0, 0.0, 0.0], [0.0, 11.0, 0.0, 0.0, 0.0], [0.0, 11.0, 0.0, 0.0, 0.0], [0.0, 11.0, 0.0, 0.0, 0.0], [0.0, 11.0, 0.0, 0.0, 0.0], [0.0, 0.0001, 0.0, 0.0, 0.0], [0.0, 0.0001, 0.0, 0.0, 0.0], [0.0, 0.0001, 0.0, 0.0, 0.0], [0.0, 0.0001, 0.0, 0.0, 0.0], [0.0, 0.0001, 0.0, 0.0, 0.0], [0.0, 0.0001, 0.0, 0.0, 0.0]]  # Cal Coefficients
        # "This is 10.30.189.0"
        n301 = Unbundle By Name(w954) -> ("App Config"=w939:T6, "LS App Config"=w915:T13)
        n302 = String To IP() -> (0:w949:u32)  [unwired: 1 in]
        n303 = Subtract(x=w949, y=u32 169786624) -> (x-y=w921:u32)
        n304 = Number To Decimal String(number=w921) -> (decimal integer string=w948:string)  [unwired: 1 in]
        n305 = call <vilib>:"Open Config Data.vi"("configuration file path"=path "c:/LS App Config.ini") -> ("error out"=w918:errorcluster, "file created?"=w916:bool, "refnum"=w917:T47)  [unwired: 8 in]
        n306 = case shown="False" w916 {
          tunnel: w918 -> [w972 w979]
          tunnel: w917 -> [w971 w980]
          tunnel: w915 -> [w970 w978]
          tunnel: [w970 w977] -> w903
          tunnel: [w966 w973] -> w914
          frame True {
            n307 = call "Read Write LS App Config.vi"("Write (F)"=TRUE, "Error IN"=w972, "LS App Config In"=w970, "Refnum in"=w971) -> ("Error OUT"=w967:errorcluster, "Refnum out"=w968:T47)  [unwired: 5 in, 1 out]
            n308 = call <vilib>:"Close Config Data.vi"("error in (no error)"=w967, "refnum"=w968) -> ("error out"=w966:errorcluster)  [unwired: 8 in, 1 out]
          }
          frame False {
            n309 = call "Read Write LS App Config.vi"("Error IN"=w979, "LS App Config In"=w978, "Refnum in"=w980) -> ("Error OUT"=w976:errorcluster, "LS App Config Out"=w977:T48, "Refnum out"=w975:T47)  [unwired: 6 in]
            n310 = call <vilib>:"Close Config Data.vi"("error in (no error)"=w976, "refnum"=w975) -> ("error out"=w974:errorcluster)  [unwired: 8 in, 1 out]
            n311 = call <vilib>:"Clear Errors.vi"("error in (no error)"=w974) -> ("error out"=w973:errorcluster)  [unwired: 5 in, 1 out]
          }
        }
        n312 = call <vilib>:"Open Config Data.vi"("error in (no error)"=w914, "configuration file path"=path "c:/App Config.ini") -> ("error out"=w961:errorcluster, "file created?"=w959:bool, "refnum"=w962:T47)  [unwired: 7 in]
        n313 = case shown="False" w959 {
          tunnel: w962 -> [w1011 w1016]
          tunnel: w961 -> [w1009 w1014]
          tunnel: w939 -> [w1006 w1013]
          tunnel: [w1007 w1013] -> w922
          tunnel: [w1005 w1015] -> w923
          frame False {
            # "Read App Config.ini"
            n314 = call "Read Write App Config.vi"("Error IN"=w1009, "App Config"=w1006, "Refnum in"=w1011) -> ("Error OUT"=w1008:errorcluster, "App Config OUT"=w1007:T6, "Refnum out"=w1010:T47)  [unwired: 6 in]
            n315 = call <vilib>:"Close Config Data.vi"("error in (no error)"=w1008, "refnum"=w1010) -> ("error out"=w1012:errorcluster)  [unwired: 8 in, 1 out]
            n316 = call <vilib>:"Clear Errors.vi"("error in (no error)"=w1012) -> ("error out"=w1005:errorcluster)  [unwired: 5 in, 1 out]
          }
          frame True {
            # "Doesn't exist, so create."
            n317 = call "Read Write App Config.vi"("Write (F)"=TRUE, "Error IN"=w1014, "App Config"=w1013, "Refnum in"=w1016) -> ("Error OUT"=w1018:errorcluster, "Refnum out"=w1019:T47)  [unwired: 5 in, 1 out]
            n318 = call <vilib>:"Close Config Data.vi"("error in (no error)"=w1018, "refnum"=w1019) -> ("error out"=w1015:errorcluster)  [unwired: 8 in, 1 out]
          }
        }
        n319 = Concatenate Strings("/c/" ("string"), w948, ".cal" ("string")) -> (w940:string)
        n320 = String To Path(string=w940) -> (path=w941:path)
        n321 = To Long Integer(number=w921) -> (32bit integer=w920:i32)
        n322 = Bundle By Name(cluster=w922, "Data Log Init.IP Last 3"=w920) -> (w900:T6)
        n323 = disable-structure shown="Disabled" {
          disable-tunnel: w900 -> [w963 _]
          frame Disabled {
            n324 = Unbundle By Name(w963) -> ("Data Log Init"=w964:T7)
            n325 = call "Data Logger Main.vi"("Data Logger Mode"=Data_Logger_Mode."Init", "Data Log Init"=w964) -> ()  [unwired: 18 in]
          }
          frame Enabled {
          }
        }
        n326 = Unbundle By Name(w900) -> ("Network Drive Password"=w897:string, "Network Drive IP"=w898:string)
        n327 = call "WebDAV address (global).vi"("Mode"=enum16{"Read", "Write"}."Write", "Network Drive Password"=w897, "Network Drive IP"=w898) -> ()  [unwired: 5 in, 2 out]
        n328 = call "Get Elapsed Times.vi"("Error In"=w923, "Path"=path "c:/ElapsedTimes" ("file (use dialog)")) -> ("Error Out"=w943:errorcluster, "Elapsed Times"=w955:dbl[])  [unwired: 8 in]
        n329 = Unbundle By Name(w900) -> ("Voltage Limits"=w926:T42, "Voltage Far PI"=w933:T43, "Voltage Mid PI"=w932:T44, "Voltage Close PI"=w931:T45, "Voltage Scale"=w930:cluster{"V_FFm":dbl, "V_FFb":dbl}, "Voltage Cutoffs"=w929:cluster{"V_MidCutoff":dbl, "V_CloseCutoff":dbl}, "Pressure Scale"=w928:cluster{"Pres_FFm":dbl, "Pres_FFb":dbl}, "Temp Format"=w925:i32, "Temp Tolerance"=w924:dbl)
        n330 = call <vilib>:"Clear Errors.vi"("error in (no error)"=w943) -> ("error out"=w944:errorcluster)  [unwired: 5 in, 1 out]
        n331 = Unbundle By Name(w900) -> ("Step Threshold:"=w908:dbl, "Anomaly Threshold:"=w907:dbl, "Normal Steps:"=w909:u32, "Bank 1 Offset"=w896:dbl, "Bank 2 Offset"=w895:dbl)
        n332 = call "Get Pressure Offsets.vi"("Error In"=w944, "Path"=path "c:/PressureOffsets" ("file (use dialog)")) -> ("Error Out"=w942:errorcluster, "Pressure Offsets"=w956:dbl[])  [unwired: 8 in]
        n333 = call <vilib>:"Clear Errors.vi"("error in (no error)"=w942) -> ("error out"=w912:errorcluster)  [unwired: 5 in, 1 out]
        n334 = local write "Voltage Limits"(w926) -> ()
        n335 = local write "Far PI"(w933) -> ()
        n336 = local write "Mid PI"(w932) -> ()
        n337 = local write "Close PI"(w931) -> ()
        n338 = local write "Voltage Scale"(w930) -> ()
        n339 = local write "Cutoffs"(w929) -> ()
        n340 = local write "Pressure Scale"(w928) -> ()
        n341 = local write "Thermocouple"(w925) -> ()
        n342 = local write "Temp Tolerance"(w924) -> ()
        n343 = call "Get Initial LS Data.vi"("Error In"=w912, "Path"=path "c:/Monitored Statistics") -> ("Error Out"=w911:errorcluster, "Initial LS Data"=w901:T15)  [unwired: 8 in]
        n344 = local write "Step Threshold:"(w908) -> ()
        n345 = local write "Anomaly Threshold:"(w907) -> ()
        n346 = local write "Normal Steps:"(w909) -> ()
        n347 = local write "Bank 1 Voltage Offset:"(w896) -> ()
        n348 = local write "Bank 2 Voltage Offset:"(w895) -> ()
        n349 = call <vilib>:"Clear Errors.vi"("error in (no error)"=w911) -> ("error out"=w910:errorcluster)  [unwired: 5 in, 1 out]
        n350 = call "Get Cal Coefficients.vi"("Error In"=w910, "Path"=w941) -> ("Error"=w951:bool, "Cal Coefficients"=w952:dbl[][])  [unwired: 7 in, 1 out]
        n351 = case shown="False" w951 {
          tunnel: w952 -> [_ w984]
          tunnel: [w981 w983] -> w927
          tunnel: w945 -> [w981 w982]
          frame True {
          }
          frame False {
            n352 = for {
              tunnel: w984 -> [w986] mode=indexing
              shift-right: [w987] -> w983
              shift-left: w982 -> [w988]
              i -> [w985]
              n353 = Index Array(array=w986) -> (element #1=w999:dbl, element #2=w998:dbl, element #3=w997:dbl, element #4=w993:dbl, element #5=w992:dbl)  [unwired: 5 in]
              n354 = Equal To 0?(x=w999) -> (x = 0?=w996:bool)
              n355 = Equal To 0?(x=w998) -> (x = 0?=w995:bool)
              n356 = Equal To 0?(x=w997) -> (x = 0?=w994:bool)
              n357 = Equal To 0?(x=w993) -> (x = 0?=w991:bool)
              n358 = Equal To 0?(x=w992) -> (x = 0?=w990:bool)
              n359 = Compound Arithmetic op=AND(w996, w995, w994, w991, w990) -> (w989:bool)
              n360 = case shown="False" w989 {
                tunnel: w988 -> [w1003 w1004]
                tunnel: [w1002 w1004] -> w987
                tunnel: w986 -> [w1001 _]
                tunnel: w985 -> [w1000 _]
                frame False {
                  n361 = Replace Array Subset(array=w1003, new element=w1001, index (row)=w1000) -> (w1002:dbl[][])  [unwired: 1 in]
                }
                frame True {
                }
              }
            }
          }
        }
        n362 = call "PI with FF.vi"("Cutoffs"=w929, "FFcluster"=w930, "ClosePIcluster"=w931, "MidPIcluster"=w932, "FarPIcluster"=w933, "LimitCluster"=w926, "Init (F)"=TRUE) -> ()  [unwired: 8 in, 1 out]
        n363 = call "Handle Profile Resume Info.vi"("Read(F)/Write(T)"=FALSE) -> ("Current Step Out"=w906:i32, "Step Time Left Out"=w905:dbl)  [unwired: 13 in]
        n364 = Insert Into Array(array=w935, index=0, new element=w936) -> (w937:T14[])
        n365 = Bundle By Name(cluster=w954, "App Config"=w900, "Initial Times"=w955, "Pressure Offsets"=w956, "CalArray"=w927, "Initial LS Data"=w901, "LS App Config"=w903, "Current Step"=w906, "Step Time Left"=w905) -> (w953:T25)
        n366 = local write "Step:"(w906) -> ()
        n367 = local write "Time Left:"(w905) -> ()
        n368 = call "LS Data Global.vi"("Mode"=T28."Write Init Data", "Initial LS Data In"=w901) -> ()  [unwired: 10 in, 4 out]
      }
      frame "Init" {
        w1034 = TRUE ("Visible")
        w1022 = T31."Enabled" ("Disabled")
        w1042 = u16 0 items=["0 - Off", "1 - On", "2 - Pulsing"] ("Bank 1 Power State:")
        w1026 = FALSE ("Running?")
        w1064 = T14[] [enum."Get Profiles", enum."Enable Background", enum."Get/Release Control", enum."Get Pressure", enum."Get Alarms", enum."Set Watlow Temp 1", enum."Set Watlow Temp 2", enum."Update Controls", enum."Controller Change", enum."Stop Profile"] items=["Main", "Init Files", "Init", "Unused", "Save As", "Start Profile", "Check Step Time", "Alarm", "Alarm Dismiss", "Run Step", "Stop Profile", "Cycle Reset", "Time Reset", "Time Reset All", "Time Set", "Tare CTs", "Save Profile", "Open Profile", "Get Profiles", "Update Screen", "Update Controls", "Save App Config", "Write Outputs", "Disable Background", "Enable Background", "Get/Release Control", "Log Fuel Change", "Fuel Change Popup", "Read Inputs", "Remote Timer Reset", "Controller Change", "Get Alarms", "Init Alarms", "Save Alarms", "Voltage Selection", "Set Watlow Temp 1", "Set Watlow Temp 2", "Get Pressure", "Write Tare Pressure", "Adjust Controls", "Reinit ADC", "Write Initial Times", "Write Pumps Present", "HMI Command", "Save Pump Times", "Check Pump Stop Time", "Save LS App Config", "Init Data File", "Reset LS Cycles", "Reset Anomalies", "Reset Opens", "Save LS Data", "Save LS Test Data", "Check Serial Numbers", "Main Tab", "Allow Data Note", "Resume Profile", "Pause Profile", "Allow Pause Note", "Clear Graph"]
        # "This solves an issue where location wouldn't\nshow up in the built version."
        n369 = Unbundle By Name(w1080) -> ("App Config.Profiles Path"=w1070:path, "App Config.Watlow Present"=w1072:bool, "App Config.Temp 1"=w1079:dbl, "App Config.Temp 2"=w1078:dbl, "App Config.Location"=w1071:string, "LS App Config.Record Bursts"=w1039:bool, "LS App Config.RecInterval(s)"=w1060:i32, "LS App Config.RecDuration(s)"=w1059:i32, "LS App Config.RecFrequeny (Hz)"=w1058:i32, "App Config.CA Number"=w1040:string, "LS App Config.Data File Name:"=w1021:string, "LS App Config.Serial Numbers"=w1024:string[], "LS App Config.DetectionMode"=w1027:i32)
        "Location:" <- w1071
        n370 = case shown="1" w1027 {
          frame 0, Default {
            n371 = local write "Live Data Tab"(enum32{"Page 1", "Page 2", "Page 3"}."Page 2" ("Live Data Tab")) -> ()
          }
          frame 1 {
            n372 = local write "Live Data Tab"(enum32{"Page 1", "Page 2", "Page 3"}."Page 3" ("Live Data Tab")) -> ()
          }
        }
        n373 = call "Init FPGA.vi"("FPGA Ref"=w1036) -> ("error out"=w1076:errorcluster, "FPGA Ref Out"=w1077:T26)  [unwired: 9 in]
        n374 = call "Watlow Global.vi"("Write (F)"=TRUE, "Watlow Present"=w1072) -> ()  [unwired: 9 in, 1 out]
        n375 = disable-structure shown="Enabled" {
          disable-tunnel: w1077 -> [w1111 _]
          disable-tunnel: w1076 -> [w1110 w1112]
          disable-tunnel: [w1109 w1112] -> w1075
          frame Disabled {
            n376 = call "Init ADCs.vi"("Error IN"=w1110, "FPGA Ref"=w1111) -> ("error out"=w1109:errorcluster)  [unwired: 7 in, 2 out]
          }
          frame Enabled {
          }
        }
        n377 = local write "Main Tab"(T9."Main" ("Main Tab")) -> ()
        n378 = local write "pb.Run Profile"(FALSE ("pb.Run Profile")) -> ()
        n379 = local write "Bank 1 Power State:"(w1042) -> ()
        n380 = local write "Bank 2 Power State:"(w1042) -> ()
        n381 = property on="Location:" class="Str"("Text.Text"=w1071) -> ()  [unwired: 2 in, 2 out]
        n382 = local write "Tank 1 Temp Cmd:"(w1079) -> ()
        n383 = local write "Tank 2 Temp Cmd:"(w1078) -> ()
        n384 = flat-sequence {
          tunnel: w1075 -> [_]
          tunnel: w1074 -> [w1113]
          frame #0 {
            n385 = Set Occurrence(w1113) -> ()
          }
        }
        n386 = Empty String/Path?(string/path=w1040) -> (empty?=w1028:bool)
        n387 = Empty String/Path?(string/path=w1021) -> (empty?=w1041:bool)
        n388 = call <vilib>:"Check if File or Folder Exists.vi"("path"=path "u:/CA Numbers" ("base path")) -> ("error out"=w1055:errorcluster, "file or folder exists?"=w1057:bool, "dup path"=w1056:path)  [unwired: 8 in]
        n389 = Or(x=w1028, y=w1041) -> (x .or. y?=w1033:bool)
        n390 = case shown="False" w1057 {
          tunnel: w1056 -> [w1106 w1108]
          tunnel: w1055 -> [w1105 w1107]
          tunnel: [w1104 w1108] -> w1053
          tunnel: [w1103 w1107] -> w1048
          frame False {
            n391 = Create Folder(path (use dialog)=w1106, error in=w1105) -> (created path=w1104:path, error out=w1103:errorcluster)  [unwired: 1 in, 1 out]
          }
          frame True {
          }
        }
        n392 = call <vilib>:"Check if File or Folder Exists.vi"("path"=w1070) -> ("file or folder exists?"=w1084:bool, "dup path"=w1083:path)  [unwired: 8 in, 1 out]
        n393 = Build Path(base path=w1053, name or relative path=w1040) -> (appended path=w1050:path)
        n394 = case shown="False" w1084 {
          tunnel: w1083 -> [w1114 _]
          frame False {
            n395 = Create Folder(path (use dialog)=w1114) -> ()  [unwired: 2 in, 3 out]
          }
          frame True {
          }
        }
        n396 = call <vilib>:"Check if File or Folder Exists.vi"("error in (no error)"=w1048, "path"=w1050) -> ("error out"=w1052:errorcluster, "file or folder exists?"=w1029:bool, "dup path"=w1051:path)  [unwired: 7 in]
        n397 = Or(x=w1029, y=w1028) -> (x .or. y?=w1030:bool)
        n398 = case shown="False" w1033 {
          tunnel: w1039 -> [w1088 _]
          tunnel: [w1088 FALSE ("Record")] -> w1035
          tunnel: [T31."Enabled" ("Disabled") T31."Disabled and Grayed Out" ("Disabled")] -> w1038
          frame False {
            # "Valid File"
          }
          frame True {
            # "Invalid File"
          }
        }
        n399 = local write "pb.Pause/Resume"(TRUE) -> ()
        n400 = case shown="False" w1030 {
          tunnel: w1051 -> [w1100 w1102]
          tunnel: w1052 -> [w1099 w1101]
          tunnel: [w1098 w1102] -> w1049
          tunnel: [w1097 w1101] -> w1044
          frame False {
            n401 = Create Folder(path (use dialog)=w1100, error in=w1099) -> (created path=w1098:path, error out=w1097:errorcluster)  [unwired: 1 in, 1 out]
          }
          frame True {
          }
        }
        n402 = Build Path(base path=w1049, name or relative path=w1021) -> (appended path=w1045:path)
        n403 = property on="Data File Name:" class="Str"("Visible"=w1034, "DisabledEnum"=w1022) -> ()  [unwired: 2 in, 2 out]
        n404 = property on="pb.Pause/Resume" class="Bool (strict)"("DisabledEnum"=w1022) -> ()  [unwired: 2 in, 2 out]
        n405 = call <vilib>:"Check if File or Folder Exists.vi"("error in (no error)"=w1044, "path"=w1045) -> ("error out"=w1046:errorcluster, "file or folder exists?"=w1032:bool, "dup path"=w1047:path)  [unwired: 7 in]
        n406 = Or(x=w1032, y=w1033) -> (x .or. y?=w1031:bool)
        n407 = case shown="False" w1031 {
          tunnel: w1047 -> [w1094 w1096]
          tunnel: w1046 -> [w1093 w1095]
          tunnel: [w1091 w1096] -> w1037
          tunnel: [w1092 w1095] -> w1043
          frame False {
            n408 = Create Folder(path (use dialog)=w1094, error in=w1093) -> (created path=w1091:path, error out=w1092:errorcluster)  [unwired: 1 in, 1 out]
          }
          frame True {
          }
        }
        n409 = property on="Record During Profile" class="Bool (strict)"("Value"=w1035, "DisabledEnum"=w1038) -> ()  [unwired: 2 in, 2 out]
        n410 = property on="pb.Run Profile" class="Bool (strict)"("Visible"=w1034, "DisabledEnum"=w1022) -> ()  [unwired: 2 in, 2 out]
        n411 = Bundle(cluster=T30 {"Running?"=FALSE, "Profile Record"=FALSE, "RecordInterval"=0, "RecordDuration"=0, "RecordFreq"=0, "Data Filepath"=path "", "Hr Record"=FALSE, "Serial Numbers"=[]} ("LS Cluster In"), "Running?"=w1026, "Profile Record"=w1035, "RecordInterval"=w1060, "RecordDuration"=w1059, "RecordFreq"=w1058, "Data Filepath"=w1037, "Hr Record"=w1026, "Serial Numbers"=w1024) -> (w1061:T30)
        n412 = call "Controller List.vi"() -> ("Controller List OUT"=w1069:T22[])  [unwired: 11 in]
        n413 = call "LS Data Global.vi"("Mode"=T28."Main Writes", "LS Cluster In"=w1061) -> ()  [unwired: 10 in, 4 out]
        n414 = Bundle By Name(cluster=w1080, "Alarm Config Path"=path "c:/Alarm Config", "Fuel Log Path"=path "u:/Fuel Change Log.csv", "Tank CMDs.Temp 1 CMD"=w1079, "Tank CMDs.Temp 2 CMD"=w1078, "Controller List"=w1069, "LS Data Filepath"=w1037, "pb.Run Profile"=w1026, "LS App Config.Record Bursts"=w1035) -> (w1081:T25)
        n415 = call <vilib>:"Clear Errors.vi"("error in (no error)"=w1043) -> ()  [unwired: 5 in, 2 out]
        n416 = Insert Into Array(array=w1065, index=0, new element=w1064) -> (w1062:T14[])
      }
      frame "Unused" {
      }
      frame "Get Alarms" {
        n417 = Unbundle By Name(w1124) -> ("Alarm Config"=w1125:T10, "Alarm Config Path"=w1122:path)
        n418 = call <vilib>:"Check if File or Folder Exists.vi"("path"=w1122) -> ("file or folder exists?"=w1127:bool, "dup path"=w1126:path)  [unwired: 8 in, 1 out]
        n419 = case shown="False" w1127 {
          tunnel: w1126 -> [w1132 w1139]
          tunnel: w1125 -> [_ w1137]
          tunnel: [T10 {"Alarms:"=[{"Description:"="PS/E-Stop/Float Switch", "Enabled:"=TRUE, "Data Index:"=9, "Data Type:"="Tank", "Low Limit:"=5.0, "High Limit:"=20.0, "Trip Time:"=1000, "Profile Sync:"=FALSE}, {"Description:"="Voltage (pump or ctrl)", "Enabled:"=TRUE, "Data Index:"=0, "Data Type:"="Pump", "Low Limit:"=12.0, "High Limit:"=17.0, "Trip Time:"=3000, "Profile Sync:"=TRUE}, {"Description:"="Pump Current", "Enabled:"=TRUE, "Data Index:"=10, "Data Type:"="Pump", "Low Limit:"=0.0, "High Limit:"=22.0, "Trip Time:"=1000, "Profile Sync:"=TRUE}, {"Description:"="Pump Speed", "Enabled:"=TRUE, "Data Index:"=16, "Data Type:"="Pump", "Low Limit:"=0.0, "High Limit:"=10000.0, "Trip Time:"=1000, "Profile Sync:"=TRUE}, {"Description:"="Controller Current", "Enabled:"=TRUE, "Data Index:"=22, "Data Type:"="Pump", "Low Limit:"=0.0, "High Limit:"=20.0, "Trip Time:"=1000, "Profile Sync:"=TRUE}, {"Description:"="Pump Pressure", "Enabled:"=TRUE, "Data Index:"=30, "Data Type:"="Pump", "Low Limit:"=550.0, "High Limit:"=750.0, "Trip Time:"=1000, "Profile Sync:"=TRUE}, {"Description:"="Pump Flow", "Enabled:"=FALSE, "Data Index:"=36, "Data Type:"="Pump", "Low Limit:"=0.0, "High Limit:"=400.0, "Trip Time:"=1000, "Profile Sync:"=TRUE}, {"Description:"="Tank Temperature 1", "Enabled:"=FALSE, "Data Index:"=28, "Data Type:"="Tank", "Low Limit:"=-50.0, "High Limit:"=0.0, "Trip Time:"=10000, "Profile Sync:"=FALSE}, {"Description:"="Tank Temperature 2", "Enabled:"=FALSE, "Data Index:"=29, "Data Type:"="Tank", "Low Limit:"=0.0, "High Limit:"=70.0, "Trip Time:"=10000, "Profile Sync:"=FALSE}], "Profile Sync:"={"Trip Time:"=2000, "Consecutive Trips:"=5}} ("Alarm Config") w1135] -> w1118
          tunnel: [w1129 w1134] -> w1117
          frame False {
            w1129 = T14[] [enum."Init Alarms", enum."Save Alarms"] items=["Main", "Init Files", "Init", "Unused", "Save As", "Start Profile", "Check Step Time", "Alarm", "Alarm Dismiss", "Run Step", "Stop Profile", "Cycle Reset", "Time Reset", "Time Reset All", "Time Set", "Tare CTs", "Save Profile", "Open Profile", "Get Profiles", "Update Screen", "Update Controls", "Save App Config", "Write Outputs", "Disable Background", "Enable Background", "Get/Release Control", "Log Fuel Change", "Fuel Change Popup", "Read Inputs", "Remote Timer Reset", "Controller Change", "Get Alarms", "Init Alarms", "Save Alarms", "Voltage Selection", "Set Watlow Temp 1", "Set Watlow Temp 2", "Get Pressure", "Write Tare Pressure", "Adjust Controls", "Reinit ADC", "Write Initial Times", "Write Pumps Present", "HMI Command", "Save Pump Times", "Check Pump Stop Time", "Save LS App Config", "Init Data File", "Reset LS Cycles", "Reset Anomalies", "Reset Opens", "Save LS Data", "Save LS Test Data", "Check Serial Numbers", "Main Tab", "Allow Data Note", "Resume Profile", "Pause Profile", "Allow Pause Note", "Clear Graph"]
            n420 = Open/Create/Replace File(file path (use dialog)=w1132, operation (0:open)=T32."create") -> (refnum out=w1131:refnum<file>, error out=w1130:errorcluster)  [unwired: 4 in, 1 out]
            n421 = Close File(refnum=w1131, error in=w1130) -> ()  [unwired: 2 out]
          }
          frame True {
            w1134 = T14[] [enum."Init Alarms"] items=["Main", "Init Files", "Init", "Unused", "Save As", "Start Profile", "Check Step Time", "Alarm", "Alarm Dismiss", "Run Step", "Stop Profile", "Cycle Reset", "Time Reset", "Time Reset All", "Time Set", "Tare CTs", "Save Profile", "Open Profile", "Get Profiles", "Update Screen", "Update Controls", "Save App Config", "Write Outputs", "Disable Background", "Enable Background", "Get/Release Control", "Log Fuel Change", "Fuel Change Popup", "Read Inputs", "Remote Timer Reset", "Controller Change", "Get Alarms", "Init Alarms", "Save Alarms", "Voltage Selection", "Set Watlow Temp 1", "Set Watlow Temp 2", "Get Pressure", "Write Tare Pressure", "Adjust Controls", "Reinit ADC", "Write Initial Times", "Write Pumps Present", "HMI Command", "Save Pump Times", "Check Pump Stop Time", "Save LS App Config", "Init Data File", "Reset LS Cycles", "Reset Anomalies", "Reset Opens", "Save LS Data", "Save LS Test Data", "Check Serial Numbers", "Main Tab", "Allow Data Note", "Resume Profile", "Pause Profile", "Allow Pause Note", "Clear Graph"]
            n422 = Read from Text File(file (use dialog)=w1139) -> (refnum out=w1136:refnum<file>, text=w1138:string)  [unwired: 3 in, 2 out]
            n423 = Close File(refnum=w1136) -> ()  [unwired: 1 in, 2 out]
            n424 = Unflatten From JSON(JSON string=w1138, type and defaults=w1137) -> (value=w1135:T10)  [unwired: 5 in, 1 out]
          }
        }
        n425 = Bundle By Name(cluster=w1124, "Alarm Config"=w1118) -> (w1123:T25)
        n426 = local write "Alarm Config"(w1118) -> ()
        n427 = Insert Into Array(array=w1119, index=0, new element=w1117) -> (w1120:T14[])
      }
      frame "Init Alarms" {
        # "Initialize alarm arrays."
        n428 = Unbundle By Name(w1146) -> ("Alarm Config.Alarms:"=w1148:T11[])
        n429 = for {
          tunnel: w1148 -> [w1155] mode=indexing
          shift-right: [w1151] -> w1142
          shift-left: 0 -> [w1150]
          n430 = Unbundle By Name(w1155) -> ("Data Type:"=w1154:string, "Enabled:"=w1153:bool)
          n431 = case shown="\"Pump\", Default" w1154 {
            tunnel: [6 1] -> w1152
            frame "Pump", Default {
            }
            frame "Tank" {
            }
          }
          n432 = case shown="True" w1153 {
            tunnel: w1152 -> [_ w1159]
            tunnel: [w1156 w1158] -> w1151
            tunnel: w1150 -> [w1156 w1157]
            frame False {
            }
            frame True {
              n433 = Add(x=w1159, y=w1157) -> (x+y=w1158:i32)
            }
          }
        }
        n434 = Tick Count (ms)() -> (millisecond timer value=w1143:u32)
        n435 = Initialize Array(0, w1142) -> (w1141:i32[])
        n436 = Initialize Array(w1143, w1142) -> (w1140:u32[])
        n437 = Bundle By Name(cluster=w1146, "Trip Counters"=w1141, "Previous Times"=w1140, "Prev ON Times"=w1140) -> (w1145:T25)
      }
      frame "Save Alarms" {
        n438 = Unbundle By Name(w1165) -> ("Alarm Config Path"=w1163:path, "Alarm Config"=w1164:T10)
        n439 = Flatten To JSON(anything=w1164) -> (JSON string=w1162:string)  [unwired: 2 in, 1 out]
        n440 = Write to Text File(file (use dialog)=w1163, text=w1162) -> ()  [unwired: 2 in, 3 out]
      }
      frame "Get Profiles" {
        n441 = Unbundle By Name(w1174) -> ("App Config.Profiles Path"=w1175:path)
        n442 = List Folder(path=w1175) -> (filenames=w1172:string[], error out=w1171:errorcluster)  [unwired: 3 in, 2 out]
        n443 = call <vilib>:"Clear Errors.vi"("error in (no error)"=w1171) -> ()  [unwired: 5 in, 2 out]
        n444 = property on="Profile Name:" class="CmbBox"("Strings[]"=w1172) -> ()  [unwired: 2 in, 2 out]
        n445 = Bundle By Name(cluster=w1174, "Profiles"=w1172) -> (w1173:T25)
        n446 = Insert Into Array(array=w1168, index=0, new element=Sequence_States."Open Profile") -> (w1167:T14[])
      }
      frame "Open Profile" {
        w1177 = T14[] [enum."Update Screen", enum."Save App Config"] items=["Main", "Init Files", "Init", "Unused", "Save As", "Start Profile", "Check Step Time", "Alarm", "Alarm Dismiss", "Run Step", "Stop Profile", "Cycle Reset", "Time Reset", "Time Reset All", "Time Set", "Tare CTs", "Save Profile", "Open Profile", "Get Profiles", "Update Screen", "Update Controls", "Save App Config", "Write Outputs", "Disable Background", "Enable Background", "Get/Release Control", "Log Fuel Change", "Fuel Change Popup", "Read Inputs", "Remote Timer Reset", "Controller Change", "Get Alarms", "Init Alarms", "Save Alarms", "Voltage Selection", "Set Watlow Temp 1", "Set Watlow Temp 2", "Get Pressure", "Write Tare Pressure", "Adjust Controls", "Reinit ADC", "Write Initial Times", "Write Pumps Present", "HMI Command", "Save Pump Times", "Check Pump Stop Time", "Save LS App Config", "Init Data File", "Reset LS Cycles", "Reset Anomalies", "Reset Opens", "Save LS Data", "Save LS Test Data", "Check Serial Numbers", "Main Tab", "Allow Data Note", "Resume Profile", "Pause Profile", "Allow Pause Note", "Clear Graph"]
        n447 = Unbundle By Name(w1189) -> ("App Config.Profiles Path"=w1191:path, "App Config.Current Profile"=w1190:string)
        n448 = Build Path(base path=w1191, name or relative path=w1190) -> (appended path=w1186:path)
        n449 = Read from Text File(file (use dialog)=w1186) -> (refnum out=w1184:refnum<file>, text=w1185:string, error out=w1183:errorcluster)  [unwired: 3 in, 1 out]
        n450 = Close File(refnum=w1184, error in=w1183) -> (error out=w1182:errorcluster)  [unwired: 1 out]
        n451 = case shown="No Error" w1182 {
          tunnel: w1185 -> [w1193 _]
          tunnel: [w1194 string[][] []] -> w1176
          frame No Error {
            n452 = Spreadsheet String To Array(delimiter (Tab)=",", format string="%s", spreadsheet string=w1193, array type (2D Dbl)=string[][] []) -> (array=w1194:string[][])
          }
          frame Error {
          }
        }
        n453 = Array Size(array=w1176) -> (size(s)=w1187:i32[])
        n454 = Index Array(array=w1187) -> (element=w1181:i32)  [unwired: 1 in]
        n455 = Bundle By Name(cluster=w1189, "Profile"=w1176, "# of Steps"=w1181) -> (w1188:T25)
        n456 = Insert Into Array(array=w1179, index=0, new element=w1177) -> (w1178:T14[])
      }
      frame "Save Profile" {
        n457 = Unbundle By Name(w1203) -> ("App Config.Profiles Path"=w1207:path, "App Config.Current Profile"=w1205:string, "Profile"=w1206:string[][])
        n458 = Empty String/Path?(string/path=w1205) -> (empty?=w1204:bool)
        n459 = case shown="False" w1204 {
          tunnel: w1207 -> [w1211 _]
          tunnel: w1205 -> [w1210 _]
          tunnel: w1206 -> [w1209 _]
          tunnel: [w1208 string[][] [] ("Profile OUT")] -> w1200
          frame False {
            n460 = call "Save Profile.vi"("Profile"=w1209, "Current Profile"=w1210, "Profiles Path"=w1211) -> ("Profile OUT"=w1208:string[][])  [unwired: 8 in]
          }
          frame True {
          }
        }
        n461 = Array Size(array=w1200) -> (size(s)=w1201:i32[])
        n462 = Index Array(array=w1201) -> (element=w1199:i32)  [unwired: 1 in]
        n463 = Bundle By Name(cluster=w1203, "Profile"=w1200, "# of Steps"=w1199) -> (w1202:T25)
      }
      frame "Start Profile" {
        w1217 = TRUE ("Running?")
        w1231 = T14[] [enum."Init Alarms", enum."Check Step Time"] items=["Main", "Init Files", "Init", "Unused", "Save As", "Start Profile", "Check Step Time", "Alarm", "Alarm Dismiss", "Run Step", "Stop Profile", "Cycle Reset", "Time Reset", "Time Reset All", "Time Set", "Tare CTs", "Save Profile", "Open Profile", "Get Profiles", "Update Screen", "Update Controls", "Save App Config", "Write Outputs", "Disable Background", "Enable Background", "Get/Release Control", "Log Fuel Change", "Fuel Change Popup", "Read Inputs", "Remote Timer Reset", "Controller Change", "Get Alarms", "Init Alarms", "Save Alarms", "Voltage Selection", "Set Watlow Temp 1", "Set Watlow Temp 2", "Get Pressure", "Write Tare Pressure", "Adjust Controls", "Reinit ADC", "Write Initial Times", "Write Pumps Present", "HMI Command", "Save Pump Times", "Check Pump Stop Time", "Save LS App Config", "Init Data File", "Reset LS Cycles", "Reset Anomalies", "Reset Opens", "Save LS Data", "Save LS Test Data", "Check Serial Numbers", "Main Tab", "Allow Data Note", "Resume Profile", "Pause Profile", "Allow Pause Note", "Clear Graph"]
        w1234 = 0 ("Current Step")
        w1228 = T31."Disabled" ("Disabled")
        n464 = Unbundle By Name(w1218) -> ("LS App Config.Record Bursts"=w1226:bool, "LS App Config.RecInterval(s)"=w1225:i32, "LS App Config.RecDuration(s)"=w1224:i32, "LS App Config.RecFrequeny (Hz)"=w1223:i32, "LS Data Filepath"=w1222:path, "LS App Config.Record Constant"=w1220:bool, "LS App Config.Serial Numbers"=w1219:string[])
        n465 = Bundle(cluster=T30 {"Running?"=FALSE, "Profile Record"=FALSE, "RecordInterval"=0, "RecordDuration"=0, "RecordFreq"=0, "Data Filepath"=path "", "Hr Record"=FALSE, "Serial Numbers"=[]} ("LS Cluster In"), "Running?"=w1217, "Profile Record"=w1226, "RecordInterval"=w1225, "RecordDuration"=w1224, "RecordFreq"=w1223, "Data Filepath"=w1222, "Hr Record"=w1220, "Serial Numbers"=w1219) -> (w1227:T30)
        n466 = disable-structure shown="Enabled" {
          disable-tunnel: "Data Log Enabled" -> [w1241 _]
          disable-tunnel: w1218 -> [w1240 _]
          frame Disabled {
            n467 = case shown="True" w1241 {
              tunnel: w1240 -> [_ w1248]
              frame False {
              }
              frame True {
                n468 = Unbundle By Name(w1248) -> ("App Config"=w1247:T6, "Profile"=w1246:string[][], "App Config.Controller Type:"=w1245:T3, "Tank CMDs"=w1243:T19)
                n469 = Format Into String(w1245) -> (resulting string=w1244:string)  [unwired: 3 in, 1 out]
                n470 = Bundle By Name(cluster=T33 {"App Config"={"Location"="", "Profiles Path"=path "", "Current Profile"="", "CA Number"="", "Cycles Completed"=0, "Controller Type:"=enum."Kuhnke", "Stagger Time (ms)"=0, "Tank 1 Fuel"="", "Tank 2 Fuel"="", "Serial Numbers"={"Position 1 SN"="", "Position 2 SN"="", "Poaition 3 SN"="", "Position 4 SN"="", "Position 5 SN"="", "Position 6 SN"=""}, "Pumps Present"={"Pump 1"=FALSE, "Pump 2"=FALSE, "Pump 3"=FALSE, "Pump 4"=FALSE, "Pump 5"=FALSE, "Pump 6"=FALSE}, "VoltCtrlRef"="", "VoltageSelect"=FALSE, "Watlow Present"=FALSE, "Temp 1"=0.0, "Temp 2"=0.0, "V_Run PI?"=FALSE, "Voltage Limits"={"V_Step"=0.0, "V_CmdMax"=0.0, "V_CmdMin"=0.0}, "Voltage Far PI"={"V_FarSlew"=0.0, "V_FarKp"=0.0, "V_FarKi"=0.0}, "Voltage Mid PI"={"V_MidSlew"=0.0, "V_MidKp"=0.0, "V_MidKi"=0.0}, "Voltage Close PI"={"V_CloseSlew"=0.0, "V_CloseKp"=0.0, "V_CloseKi"=0.0}, "Voltage Scale"={"V_FFm"=0.0, "V_FFb"=0.0}, "Voltage Cutoffs"={"V_MidCutoff"=0.0, "V_CloseCutoff"=0.0}, "Pressure Scale"={"Pres_FFm"=0.0, "Pres_FFb"=0.0}, "Temp Format"=0, "Temp Tolerance"=0.0, "Target Voltage"=0.0, "Target Pressure"=0.0, "Data Log Init"={"Data Path"=path "", "Data Log Rate (S/s)"=0, "AKLH Rate (Hours/S)"=0.0, "Sync Time Offset (min)"=0, "IP Last 3"=0, "WebDAV IP"=""}, "Email Handler IP"="", "ADC Check"=FALSE, "3 Pump Tank"=FALSE, "Cycle Threshold:"=0.0, "Cycle Pts to Avg:"=0, "Anomaly Threshold:"=0.0, "Normal Steps:"=0, "Step Threshold:"=0.0, "Network Drive IP"="", "Network Drive Password"="", "Bank 1 Offset"=0.0, "Bank 2 Offset"=0.0}, "Profile"=[], "Controller Type"="", "Tank CMDs"={"PS CMD"=0.0, "Press CMD"=0.0, "Temp 1 CMD"=0.0, "Temp 2 CMD"=0.0}} ("Data Log Start"), "App Config"=w1247, "Profile"=w1246, "Controller Type"=w1244, "Tank CMDs"=w1243) -> (w1249:T33)
                n471 = call "Data Logger Main.vi"("Data Logger Mode"=Data_Logger_Mode."Start", "Data Log Start"=w1249) -> ()  [unwired: 18 in]
              }
            }
          }
          frame Enabled {
          }
        }
        n472 = call "LS Data Global.vi"("Mode"=T28."Main Writes", "LS Cluster In"=w1227) -> ()  [unwired: 10 in, 4 out]
        n473 = local write "pb.Pause/Resume"(FALSE) -> ()
        n474 = property on="Bank 1" class="Clust (strict)"("DisabledEnum"=w1228) -> ()  [unwired: 2 in, 2 out]
        n475 = property on="Bank 2" class="Clust (strict)"("DisabledEnum"=w1228) -> ()  [unwired: 2 in, 2 out]
        n476 = property on="Live Data Tab" class="TabCtl (strict)"("DisabledEnum"=w1228) -> ()  [unwired: 2 in, 2 out]
        n477 = property on="Pump Timers Tab" class="TabCtl (strict)"("DisabledEnum"=w1228) -> ()  [unwired: 2 in, 2 out]
        n478 = Get Date/Time In Seconds() -> (seconds since 1Jan1904=w1237:timestamp)
        n479 = To Double Precision Float(number=w1237) -> (double precision float=w1236:dbl)
        n480 = Bundle By Name(cluster=w1218, "Recording"="Data Log Enabled", "Run Profile"=TRUE, "Step Start Time"=w1236, "Last Profile Time"=w1236, "Step Time"=0.0, "Current Step"=w1234, "Stagger Counter"=w1234, "pb.Run Profile"=w1217, "ARactive"=FALSE) -> (w1239:T25)
        n481 = local write "ARclock"(0 ("ARclock")) -> ()
        n482 = Insert Into Array(array=w1233, index=0, new element=w1231) -> (w1232:T14[])
      }
      frame "Resume Profile" {
        w1272 = TRUE ("Running?")
        w1285 = T14[] [enum."Init Alarms", enum."Run Step", enum."Check Step Time"] items=["Main", "Init Files", "Init", "Unused", "Save As", "Start Profile", "Check Step Time", "Alarm", "Alarm Dismiss", "Run Step", "Stop Profile", "Cycle Reset", "Time Reset", "Time Reset All", "Time Set", "Tare CTs", "Save Profile", "Open Profile", "Get Profiles", "Update Screen", "Update Controls", "Save App Config", "Write Outputs", "Disable Background", "Enable Background", "Get/Release Control", "Log Fuel Change", "Fuel Change Popup", "Read Inputs", "Remote Timer Reset", "Controller Change", "Get Alarms", "Init Alarms", "Save Alarms", "Voltage Selection", "Set Watlow Temp 1", "Set Watlow Temp 2", "Get Pressure", "Write Tare Pressure", "Adjust Controls", "Reinit ADC", "Write Initial Times", "Write Pumps Present", "HMI Command", "Save Pump Times", "Check Pump Stop Time", "Save LS App Config", "Init Data File", "Reset LS Cycles", "Reset Anomalies", "Reset Opens", "Save LS Data", "Save LS Test Data", "Check Serial Numbers", "Main Tab", "Allow Data Note", "Resume Profile", "Pause Profile", "Allow Pause Note", "Clear Graph"]
        w1283 = T31."Disabled" ("Disabled")
        # "New Step should be False so this is the only way to get Step Start Time set correctly"
        # "Time this step has ran"
        # "Removed writing the Current Step as it is already correct"
        # "Added Run Step"
        n483 = Unbundle By Name(w1273) -> ("Profile"=w1260:string[][], "Current Step"=w1261:i32, "Step Time Left"=w1256:dbl, "LS App Config.Record Bursts"=w1281:bool, "LS App Config.RecInterval(s)"=w1280:i32, "LS App Config.RecDuration(s)"=w1279:i32, "LS App Config.RecFrequeny (Hz)"=w1278:i32, "LS Data Filepath"=w1277:path, "LS App Config.Record Constant"=w1275:bool, "LS App Config.Serial Numbers"=w1274:string[])
        n484 = local read "Data Log Enabled"() -> (w1269:bool)
        n485 = Bundle(cluster=T30 {"Running?"=FALSE, "Profile Record"=FALSE, "RecordInterval"=0, "RecordDuration"=0, "RecordFreq"=0, "Data Filepath"=path "", "Hr Record"=FALSE, "Serial Numbers"=[]} ("LS Cluster In"), "Running?"=w1272, "Profile Record"=w1281, "RecordInterval"=w1280, "RecordDuration"=w1279, "RecordFreq"=w1278, "Data Filepath"=w1277, "Hr Record"=w1275, "Serial Numbers"=w1274) -> (w1282:T30)
        n486 = Decrement(x=w1261) -> (x-1=w1262:i32)
        n487 = Index Array(array=w1260, index (row)=w1262) -> (element=w1259:string[])  [unwired: 1 in]
        n488 = call "LS Data Global.vi"("Mode"=enum16{"Read", "Engine Writes", "Main Writes"}."Main Writes", "LS Cluster In"=w1282) -> ()  [unwired: 10 in, 4 out]
        n489 = Delete From Array(array=w1259, length=1, index=0 ("length")) -> (array with subset deleted=w1265:string[])  [unwired: 1 out]
        n490 = Fract/Exp String To Number(string=w1265) -> (number=w1258:dbl[])  [unwired: 3 in, 1 out]
        n491 = Delete From Array(array=w1258, length=1, index=0 ("length")) -> (deleted portion=w1268:dbl[])  [unwired: 1 out]
        n492 = Index Array(array=w1268) -> (element=w1257:dbl)  [unwired: 1 in]
        n493 = Subtract(x=w1257, y=w1256) -> (x-y=w1255:dbl)
        n494 = local write "pb.Pause/Resume"(FALSE) -> ()
        n495 = property on="Bank 1" class="Clust (strict)"("DisabledEnum"=w1283) -> ()  [unwired: 2 in, 2 out]
        n496 = property on="Bank 2" class="Clust (strict)"("DisabledEnum"=w1283) -> ()  [unwired: 2 in, 2 out]
        n497 = property on="Live Data Tab" class="TabCtl (strict)"("DisabledEnum"=w1283) -> ()  [unwired: 2 in, 2 out]
        n498 = property on="Pump Timers Tab" class="TabCtl (strict)"("DisabledEnum"=w1283) -> ()  [unwired: 2 in, 2 out]
        n499 = Get Date/Time In Seconds() -> (seconds since 1Jan1904=w1289:timestamp)
        n500 = To Double Precision Float(number=w1289) -> (double precision float=w1253:dbl)
        n501 = Subtract(x=w1253, y=w1255) -> (x-y=w1254:dbl)
        n502 = Bundle By Name(cluster=w1273, "Recording"=w1269, "Run Profile"=TRUE, "Step Start Time"=w1254, "Last Profile Time"=w1253, "Step Time"=w1257, "Stagger Counter"=0 ("Current Step"), "pb.Run Profile"=w1272, "ARactive"=FALSE) -> (w1291:T25)
        n503 = local write "ARclock"(0 ("ARclock")) -> ()
        n504 = Insert Into Array(array=w1287, index=0, new element=w1285) -> (w1286:T14[])
      }
      frame "Check Step Time" {
        w1295 = 10 ("y")
        # "Time elapsed since\nstart of step."
        n505 = Unbundle By Name(w1323) -> ("ProfileMinute"=w1298:i32, "Step Start Time"=w1325:dbl, "Step Time"=w1324:dbl, "Current Step"=w1321:i32, "App Config.Stagger Time (ms)"=w1306:i32, "Stagger Counter"=w1312:i32)
        n506 = Get Date/Time In Seconds() -> (seconds since 1Jan1904=w1301:timestamp)
        n507 = Increment(x=w1312) -> (x+1=w1307:i32)
        n508 = To Double Precision Float(number=w1301) -> (double precision float=w1320:dbl)
        n509 = Multiply(x=w1306, y=w1307) -> (x*y=w1318:i32)
        n510 = Subtract(x=w1320, y=w1325) -> (x-y=w1317:dbl)
        n511 = Seconds To Date/Time(time stamp (now)=w1301) -> (date time rec=w1300:T46)  [unwired: 1 in]
        n512 = To Double Precision Float(number=w1318) -> (double precision float=w1311:dbl)
        n513 = Unbundle By Name(w1300) -> ("minute"=w1297:i32)
        n514 = Divide(x=w1311, y=1000.0) -> (x/y=w1309:dbl)
        n515 = Not Equal To 0?(x=w1306) -> (x != 0?=w1305:bool)
        n516 = Greater Or Equal?(x=w1317, y=w1309) -> (x >= y?=w1316:bool)
        n517 = Less Or Equal?(x=w1312, y=4) -> (x <= y?=w1314:bool)
        n518 = Subtract(x=w1324, y=w1317) -> (x-y=w1302:dbl)
        n519 = Compound Arithmetic op=AND(w1316, w1314, w1305) -> (w1313:bool)
        n520 = Less Or Equal To 0?(x=w1302) -> (x <= 0?=w1308:bool)
        n521 = Quotient & Remainder(x=w1298, y=w1295) -> (floor(x/y)=w1293:i32)  [unwired: 1 out]
        n522 = Quotient & Remainder(x=w1297, y=w1295) -> (floor(x/y)=w1294:i32)  [unwired: 1 out]
        n523 = case shown="False" w1308 {
          tunnel: [w1335 w1343] -> w1296
          tunnel: w1321 -> [w1336 w1345]
          tunnel: [w1336 w1344] -> w1303
          tunnel: [w1332 0 ("Stagger Counter")] -> w1319
          tunnel: w1313 -> [w1334 _]
          tunnel: w1312 -> [w1333 _]
          tunnel: w1304 -> [w1331 _]
          frame False {
            # "There's time left.  Update screen."
            n524 = case shown="True" w1334 {
              tunnel: [w1337 w1341] -> w1335
              tunnel: w1333 -> [w1338 w1340]
              tunnel: [w1338 w1339] -> w1332
              tunnel: w1331 -> [w1337 _]
              frame False {
              }
              frame True {
                w1341 = T14[] [enum."Run Step"] items=["Main", "Init Files", "Init", "Unused", "Save As", "Start Profile", "Check Step Time", "Alarm", "Alarm Dismiss", "Run Step", "Stop Profile", "Cycle Reset", "Time Reset", "Time Reset All", "Time Set", "Tare CTs", "Save Profile", "Open Profile", "Get Profiles", "Update Screen", "Update Controls", "Save App Config", "Write Outputs", "Disable Background", "Enable Background", "Get/Release Control", "Log Fuel Change", "Fuel Change Popup", "Read Inputs", "Remote Timer Reset", "Controller Change", "Get Alarms", "Init Alarms", "Save Alarms", "Voltage Selection", "Set Watlow Temp 1", "Set Watlow Temp 2", "Get Pressure", "Write Tare Pressure", "Adjust Controls", "Reinit ADC", "Write Initial Times", "Write Pumps Present", "HMI Command", "Save Pump Times", "Check Pump Stop Time", "Save LS App Config", "Init Data File", "Reset LS Cycles", "Reset Anomalies", "Reset Opens", "Save LS Data", "Save LS Test Data", "Check Serial Numbers", "Main Tab", "Allow Data Note", "Resume Profile", "Pause Profile", "Allow Pause Note", "Clear Graph"]
                n525 = Increment(x=w1340) -> (x+1=w1339:i32)
              }
            }
          }
          frame True {
            w1343 = T14[] [enum."Run Step"] items=["Main", "Init Files", "Init", "Unused", "Save As", "Start Profile", "Check Step Time", "Alarm", "Alarm Dismiss", "Run Step", "Stop Profile", "Cycle Reset", "Time Reset", "Time Reset All", "Time Set", "Tare CTs", "Save Profile", "Open Profile", "Get Profiles", "Update Screen", "Update Controls", "Save App Config", "Write Outputs", "Disable Background", "Enable Background", "Get/Release Control", "Log Fuel Change", "Fuel Change Popup", "Read Inputs", "Remote Timer Reset", "Controller Change", "Get Alarms", "Init Alarms", "Save Alarms", "Voltage Selection", "Set Watlow Temp 1", "Set Watlow Temp 2", "Get Pressure", "Write Tare Pressure", "Adjust Controls", "Reinit ADC", "Write Initial Times", "Write Pumps Present", "HMI Command", "Save Pump Times", "Check Pump Stop Time", "Save LS App Config", "Init Data File", "Reset LS Cycles", "Reset Anomalies", "Reset Opens", "Save LS Data", "Save LS Test Data", "Check Serial Numbers", "Main Tab", "Allow Data Note", "Resume Profile", "Pause Profile", "Allow Pause Note", "Clear Graph"]
            # "No time left.  Go to next step."
            n526 = Increment(x=w1345) -> (x+1=w1344:i32)
          }
        }
        n527 = Not Equal?(x=w1293, y=w1294) -> (x != y?=w1299:bool)
        n528 = case shown="True" w1299 {
          tunnel: w1296 -> [w1326 w1330]
          tunnel: [w1326 w1329] -> w1292
          frame False {
          }
          frame True {
            n529 = Insert Into Array(array=w1330, index=0, new element=Sequence_States."Save LS Data") -> (w1329:T14[])
          }
        }
        n530 = Bundle By Name(cluster=w1323, "ProfileMinute"=w1297, "Last Profile Time"=w1320, "Step Time Left"=w1302, "New Step"=w1308, "Current Step"=w1303, "Stagger Counter"=w1319) -> (w1322:T25)
      }
      frame "Run Step" {
        w1367 = T14[] [enum."Write Outputs", enum."Read Inputs", enum."Update Screen"] items=["Main", "Init Files", "Init", "Unused", "Save As", "Start Profile", "Check Step Time", "Alarm", "Alarm Dismiss", "Run Step", "Stop Profile", "Cycle Reset", "Time Reset", "Time Reset All", "Time Set", "Tare CTs", "Save Profile", "Open Profile", "Get Profiles", "Update Screen", "Update Controls", "Save App Config", "Write Outputs", "Disable Background", "Enable Background", "Get/Release Control", "Log Fuel Change", "Fuel Change Popup", "Read Inputs", "Remote Timer Reset", "Controller Change", "Get Alarms", "Init Alarms", "Save Alarms", "Voltage Selection", "Set Watlow Temp 1", "Set Watlow Temp 2", "Get Pressure", "Write Tare Pressure", "Adjust Controls", "Reinit ADC", "Write Initial Times", "Write Pumps Present", "HMI Command", "Save Pump Times", "Check Pump Stop Time", "Save LS App Config", "Init Data File", "Reset LS Cycles", "Reset Anomalies", "Reset Opens", "Save LS Data", "Save LS Test Data", "Check Serial Numbers", "Main Tab", "Allow Data Note", "Resume Profile", "Pause Profile", "Allow Pause Note", "Clear Graph"]
        n531 = Unbundle By Name(w1349) -> ("Profile"=w1379:string[][], "Current Step"=w1378:i32, "# of Steps"=w1377:i32, "App Config.Cycles Completed"=w1376:u32, "App Config.Pumps Present"=w1368:T8, "New Step"=w1383:bool, "Step Start Time"=w1382:dbl)
        n532 = Unbundle By Name(w1349) -> ("Run Profile"=w1348:bool, "LS App Config.Record Bursts"=w1357:bool, "LS App Config.RecInterval(s)"=w1356:i32, "LS App Config.RecDuration(s)"=w1355:i32, "LS App Config.RecFrequeny (Hz)"=w1354:i32, "LS Data Filepath"=w1353:path, "LS App Config.Serial Numbers"=w1351:string[])  [unwired: 1 out]
        n533 = call "Run Step.vi"("Profile"=w1379, "Current Step in"=w1378, "# of Steps"=w1377, "Cycles Completed in"=w1376, "Pumps Present"=w1368) -> ("Bank1State"=w1362:u16, "Bank2State"=w1361:u16, "Record"=w1346:bool, "LS Freq"=w1360:dbl, "LS Duty"=w1359:dbl, "PS Cmd"=w1375:dbl, "Press Cmd"=w1374:dbl, "Ignition Relays"=w1373:T8, "Current Step out"=w1372:i32, "Cycles Completed out"=w1371:u32, "Step Time"=w1370:dbl, "Controller CMDs"=w1369:dbl[], "Power Relays"=w1347:T8)  [unwired: 10 in]
        n534 = Bundle(cluster=T30 {"Running?"=FALSE, "Profile Record"=FALSE, "RecordInterval"=0, "RecordDuration"=0, "RecordFreq"=0, "Data Filepath"=path "", "Hr Record"=FALSE, "Serial Numbers"=[]} ("LS Cluster In"), "Running?"=w1348, "Profile Record"=w1357, "RecordInterval"=w1356, "RecordDuration"=w1355, "RecordFreq"=w1354, "Data Filepath"=w1353, "Hr Record"=w1346, "Serial Numbers"=w1351) -> (w1358:T30)
        n535 = call "LS Data Global.vi"("Mode"=enum16{"Read", "Engine Writes", "Main Writes"}."Main Writes", "LS Cluster In"=w1358) -> ()  [unwired: 10 in, 4 out]
        n536 = local write "Bank 1 Power State:"(w1362) -> ()
        n537 = local write "Bank 2 Power State:"(w1361) -> ()
        n538 = local write "LS Cycle Time (ms):"(w1360) -> ()
        n539 = local write "LS On Time (ms):"(w1359) -> ()
        n540 = case shown="False" w1383 {
          tunnel: [w1393 w1394] -> w1366
          tunnel: w1382 -> [w1393 _]
          tunnel: w1369 -> [_ _]
          frame False {
          }
          frame True {
            n541 = Get Date/Time In Seconds() -> (seconds since 1Jan1904=w1395:timestamp)
            n542 = To Double Precision Float(number=w1395) -> (double precision float=w1394:dbl)
          }
        }
        n543 = Insert Into Array(array=w1380, index=0, new element=w1367) -> (w1365:T14[])
        n544 = flat-sequence {
          tunnel: w1366 -> [_]
          frame #0 {
            n545 = Tick Count (ms)() -> (millisecond timer value=w1392:u32)
            n546 = feedback #3() -> (w1391:u32)  [unwired: 1 in]
            n547 = feedback-in #3(w1392) -> ()
            n548 = Subtract(x=w1392, y=w1391) -> (x-y=→"Run Step (ms)":u32)
          }
        }
        n549 = case shown="True" "Stop Time Enable" {
          tunnel: w1365 -> [w1385 w1387]
          tunnel: [w1385 w1386] -> w1364
          frame False {
          }
          frame True {
            w1389 = T14[] [enum."Check Pump Stop Time"] items=["Main", "Init Files", "Init", "Unused", "Save As", "Start Profile", "Check Step Time", "Alarm", "Alarm Dismiss", "Run Step", "Stop Profile", "Cycle Reset", "Time Reset", "Time Reset All", "Time Set", "Tare CTs", "Save Profile", "Open Profile", "Get Profiles", "Update Screen", "Update Controls", "Save App Config", "Write Outputs", "Disable Background", "Enable Background", "Get/Release Control", "Log Fuel Change", "Fuel Change Popup", "Read Inputs", "Remote Timer Reset", "Controller Change", "Get Alarms", "Init Alarms", "Save Alarms", "Voltage Selection", "Set Watlow Temp 1", "Set Watlow Temp 2", "Get Pressure", "Write Tare Pressure", "Adjust Controls", "Reinit ADC", "Write Initial Times", "Write Pumps Present", "HMI Command", "Save Pump Times", "Check Pump Stop Time", "Save LS App Config", "Init Data File", "Reset LS Cycles", "Reset Anomalies", "Reset Opens", "Save LS Data", "Save LS Test Data", "Check Serial Numbers", "Main Tab", "Allow Data Note", "Resume Profile", "Pause Profile", "Allow Pause Note", "Clear Graph"]
            n550 = Insert Into Array(array=w1387, index=0, new element=w1389) -> (w1386:T14[])
          }
        }
        n551 = Bundle By Name(cluster=w1349, "Bank 1 State:"=w1362, "Bank 2 State:"=w1361, "LS App Config.LS Power (Freq):"=w1360, "LS App Config.LS Power (Duty):"=w1359, "Tank CMDs.PS CMD"=w1375, "Tank CMDs.Press CMD"=w1374, "Ignition Relay"=w1373, "Current Step"=w1372, "App Config.Cycles Completed"=w1371, "Step Time"=w1370, "Controller CMDs"=w1369, "Power Relay"=w1347, "Step Start Time"=w1366) -> (w1384:T25)
      }
      frame "Write Outputs" {
        w1404 = fxp<+/-,28,17> 0.0 ("Step Threshold")
        w1398 = 40000.0 ("x")
        w1432 = T14[] [] items=["Main", "Init Files", "Init", "Unused", "Save As", "Start Profile", "Check Step Time", "Alarm", "Alarm Dismiss", "Run Step", "Stop Profile", "Cycle Reset", "Time Reset", "Time Reset All", "Time Set", "Tare CTs", "Save Profile", "Open Profile", "Get Profiles", "Update Screen", "Update Controls", "Save App Config", "Write Outputs", "Disable Background", "Enable Background", "Get/Release Control", "Log Fuel Change", "Fuel Change Popup", "Read Inputs", "Remote Timer Reset", "Controller Change", "Get Alarms", "Init Alarms", "Save Alarms", "Voltage Selection", "Set Watlow Temp 1", "Set Watlow Temp 2", "Get Pressure", "Write Tare Pressure", "Adjust Controls", "Reinit ADC", "Write Initial Times", "Write Pumps Present", "HMI Command", "Save Pump Times", "Check Pump Stop Time", "Save LS App Config", "Init Data File", "Reset LS Cycles", "Reset Anomalies", "Reset Opens", "Save LS Data", "Save LS Test Data", "Check Serial Numbers", "Main Tab", "Allow Data Note", "Resume Profile", "Pause Profile", "Allow Pause Note", "Clear Graph"]
        # "T:Anomalies     F:Opens"
        n552 = Unbundle By Name(w1446) -> ("App Config.Pumps Present"=w1452:T8, "Controller Config.Controller Name"=w1453:T3, "Controller Config.Frequency"=w1451:i32, "Controller CMDs"=w1450:dbl[], "Stagger Counter"=w1449:i32, "App Config.Stagger Time (ms)"=w1448:i32, "Run Profile"=w1447:bool, "Power Relay"=w1437:T8, "Ignition Relay"=w1436:T8, "Tank CMDs"=w1439:T19, "App Config"=w1438:T6, "Voltage Enable"=w1435:bool, "App Config.V_Run PI?"=w1443:bool, "Tank CMDs.PS CMD"=w1441:dbl, "Tank Data.PS Actual (V):"=w1442:dbl, "App Config.VoltCtrlRef"=w1440:string, "LS App Config.Bank 1 Present"=w1431:T2, "LS App Config.Bank 2 Present"=w1430:T1, "LS App Config.DetectionMode"=w1416:i32, "Bank 1 State:"=w1423:u16, "Bank 2 State:"=w1426:u16, "LS App Config.LS Power (Freq):"=w1400:dbl, "LS App Config.LS Power (Duty):"=w1425:dbl, "App Config.Normal Steps:"=w1410:u32, "App Config.Anomaly Threshold:"=w1407:dbl, "App Config.Step Threshold:"=w1408:dbl, "LS App Config.Bias Resistances"=w1403:dbl[], "LS App Config.Voltage(T)/Resistance(F)"=w1402:bool, "App Config.Bank 1 Offset"=w1397:dbl, "App Config.Bank 2 Offset"=w1396:dbl)
        n553 = Cluster To Array(cluster=w1431) -> (array=w1419:bool[])
        n554 = Cluster To Array(cluster=w1430) -> (array=w1421:bool[])
        n555 = Equal To 0?(x=w1416) -> (x = 0?=w1415:bool)
        n556 = Multiply(x=w1398, y=w1400) -> (x*y=w1399:dbl)
        n557 = case shown="2" w1423 {
          tunnel: [FALSE FALSE TRUE] -> w1422
          tunnel: [FALSE TRUE FALSE] -> w1411
          frame 0, Default {
            # "Off"
          }
          frame 1 {
            # "On"
          }
          frame 2 {
            # "Pulsing"
          }
        }
        n558 = case shown="2" w1426 {
          tunnel: [FALSE FALSE TRUE] -> w1424
          tunnel: [FALSE TRUE FALSE] -> w1412
          frame 0, Default {
            # "Off"
          }
          frame 1 {
            # "On"
          }
          frame 2 {
            # "Pulsing"
          }
        }
        n559 = disable-structure shown="Enabled" {
          disable-tunnel: w1453 -> [w1485 _]
          disable-tunnel: w1452 -> [w1484 _]
          disable-tunnel: w1451 -> [w1483 _]
          disable-tunnel: w1450 -> [w1482 w1514]
          disable-tunnel: w1449 -> [w1481 _]
          disable-tunnel: w1448 -> [w1480 _]
          disable-tunnel: w1447 -> [w1479 _]
          disable-tunnel: [w1478 w1514] -> w1444
          disable-tunnel: w1443 -> [w1477 _]
          disable-tunnel: w1442 -> [w1476 _]
          disable-tunnel: w1409 -> [w1474 _]
          disable-tunnel: w1441 -> [w1472 _]
          disable-tunnel: w1440 -> [w1471 _]
          disable-tunnel: w1439 -> [w1470 _]
          disable-tunnel: w1438 -> [w1469 _]
          disable-tunnel: w1437 -> [w1468 _]
          disable-tunnel: w1436 -> [w1467 _]
          disable-tunnel: w1435 -> [w1466 _]
          frame Disabled {
            n560 = call "Power Supply Global.vi"("Closed Loop"=w1477, "PS Global Mode"=Power_Supply_Global_Mode."Write Setpoint", "PS Cmd"=w1472, "PS Voltage"=w1476, "VoltCtrlRef"=w1471) -> ()  [unwired: 6 in, 5 out]
            n561 = disable-structure shown="Enabled" {
              disable-tunnel: w1474 -> [w1492 w1493]
              disable-tunnel: [w1491 w1493] -> w1473
              disable-tunnel: w1470 -> [w1490 _]
              disable-tunnel: w1469 -> [w1489 _]
              disable-tunnel: w1468 -> [w1488 _]
              disable-tunnel: w1467 -> [w1487 _]
              disable-tunnel: w1466 -> [w1486 _]
              frame Disabled {
                n562 = call "Write FPGA Outputs.vi"("FPGA Ref"=w1492, "Tank CMDs"=w1490, "App Config"=w1489, "Power Relay"=w1488, "Ignition Relay"=w1487, "Voltage Enable"=w1486) -> ("FPGA Ref OUT"=w1491:T26)  [unwired: 13 in]
              }
              frame Enabled {
              }
            }
            n563 = case shown="\"Kuhnke\", \"Helbako BLDC\", \"PSA\", Default" w1485 {
              selector: w1485 -> [_ w1505]
              tunnel: w1473 -> [w1500 _]
              tunnel: w1484 -> [_ w1509]
              tunnel: w1483 -> [w1499 _]
              tunnel: w1482 -> [w1498 w1507]
              tunnel: w1481 -> [w1497 _]
              tunnel: w1480 -> [w1496 _]
              tunnel: w1479 -> [w1495 _]
              tunnel: [w1494 w1507] -> w1478
              tunnel: w1468 -> [_ w1504]
              tunnel: w1467 -> [_ w1503]
              frame "Kuhnke", "Helbako BLDC", "PSA", Default {
                n564 = call "Write PWM Outputs.vi"("FPGE Ref"=w1500, "Frequency"=w1499, "Controller CMDs IN"=w1498, "Stagger Counter"=w1497, "Stagger Time (ms)"=w1496, "Run Profile"=w1495) -> ("Controller CMDs OUT"=w1494:dbl[])  [unwired: 13 in]
              }
              frame "Conti".."Hella BLDC Pressure" {
                n565 = Cluster To Array(cluster=w1509) -> (array=w1502:bool[])
                n566 = Search 1D Array(1D array=w1502, element=TRUE) -> (index of element=w1508:i32)  [unwired: 1 in]
                n567 = Less Than 0?(x=w1508) -> (x < 0?=w1513:bool)
                n568 = Select(t=0, s=w1513, f=w1508) -> (s? t:f=w1511:i32)
                n569 = Index Array(array=w1507, index=w1511) -> (element=w1501:dbl)
                n570 = call "CAN Global.vi"("Controller Type:"=w1505, "Write (F)"=TRUE, "CAN Cmd"=w1501, "Power Relay"=w1504, "Ignition Relay"=w1503) -> ()  [unwired: 7 in, 4 out]
              }
            }
          }
          frame Enabled {
          }
        }
        n571 = Multiply(x=w1398, y=w1425) -> (x*y=w1429:dbl)
        n572 = To Unsigned Long Integer(number=w1399) -> (unsigned 32bit integer=w1427:u32)
        n573 = To Long Integer(number=w1429) -> (32bit integer=w1428:i32)
        n574 = Insert Into Array(array=w1421, index=0, new element=w1419) -> (w1418:bool[])
        n575 = Not(x=w1415) -> (.not. x?=w1414:bool)
        n576 = And(x=w1418, y=w1415) -> (x .and. y?=w1417:bool[])
        n577 = And(x=w1418, y=w1414) -> (x .and. y?=w1413:bool[])
        n578 = To Fixed-Point(fixed-point type=w1404, number=w1407) -> (fixed-point=w1405:fxp<+/-,28,17>)
        n579 = To Fixed-Point(fixed-point type=w1404, number=w1408) -> (fixed-point=w1406:fxp<+/-,28,17>)
        n580 = xnode "Read/Write Control"("FPGA VI Reference In"=w1409, "Enable Readings"=w1418, "Enable Cycles"=w1417, "Enable Anomalies"=w1417, "Enable Opens"=w1413, "Bank1(Pulse/Const)"=w1422, "Bank1Const(On/Off)"=w1411, "Bank2(Pulse/Const)"=w1424, "Bank2Const(On/Off)"=w1412, "PWM Period (Ticks)"=w1427, "Duty (Ticks)"=w1428, "Normal Steps"=w1410, "Anomaly Threshold"=w1405, "Step Threshold"=w1406, "Resistance In"=w1403, "V(T)/R(F)"=w1402, "B1offset"=w1397, "B2offset"=w1396) -> ()  [unwired: 1 in, 2 out]
        n581 = Bundle By Name(cluster=w1446, "Controller CMDs"=w1444) -> (w1445:T25)
        n582 = Insert Into Array(array=w1401, index=0, new element=w1432) -> (w1433:T14[])
      }
      frame "Read Inputs" {
        w1518 = FALSE ("WebDAV Push")
        n583 = Unbundle By Name(w1564) -> ("Concat Data"=w1519:bool, "WebDAV Push"=w1529:bool, "Current Step"=w1528:i32, "Step Time Left"=w1527:dbl, "Run Profile"=w1547:bool, "Controller Config"=w1542:T22, "Trip Counters"=w1557:i32[], "Previous Times"=w1556:u32[], "Prev ON Times"=w1555:u32[], "Alarm Config"=w1558:T10, "Alarm Message 2"=w1551:string, "Alarm Message 1"=w1552:string, "Alarm Latch"=w1553:bool, "App Config.Pumps Present"=w1540:T8, "Power Relay"=w1559:T8, "Controller CMDs"=w1543:dbl[], "App Config"=w1544:T6, "Tank CMDs"=w1545:T19, "Time/Date"=w1548:string, "Run Profile"=w1541:bool, "Recording"=w1550:bool, "Power Relay"=w1546:T8, "App Config.ADC Check"=w1521:bool, "Initial LS Data"=w1516:T15)
        n584 = Cluster To Array(cluster=w1540) -> (array=w1525:bool[])
        n585 = call "Tank Data Global.vi"() -> ("Tank Data OUT"=w1563:dbl[], "Pump Data"=w1531:T17, "Tank Data"=w1530:T23, "Record Time (sec)"=w1520:dbl)  [unwired: 12 in]
        n586 = disable-structure shown="Enabled" {
          disable-tunnel: w1517 -> [w1574 _]
          disable-tunnel: w1545 -> [w1573 _]
          disable-tunnel: w1544 -> [w1572 _]
          disable-tunnel: w1543 -> [w1571 _]
          disable-tunnel: w1542 -> [w1570 _]
          disable-tunnel: w1541 -> [w1569 _]
          disable-tunnel: w1530 -> [w1568 _]
          disable-tunnel: [w1567 _] -> w1526
          disable-tunnel: w1525 -> [w1566 _]
          disable-tunnel: [w1565 _] -> w1523
          frame Disabled {
            n587 = call "Enable Timers.vi"("FPGA Ref"=w1574, "Tank Data"=w1568, "Tank CMDs"=w1573, "App Config"=w1572, "Controller CMDs"=w1571, "Controller Config"=w1570, "Run Profile"=w1569, "Pumps Present"=w1566) -> ("In Spec"=w1567:bool[], "Reset ADCs"=w1565:bool)  [unwired: 18 in]
          }
          frame Enabled {
          }
        }
        n588 = call "Evaluate Alarms.vi"("In Test"=w1547, "Controller"=w1542, "Alarm Config"=w1558, "Data"=w1563, "Pumps Present"=w1525, "Trip Counter"=w1557, "Previous Times"=w1556, "Manual CMDs"=w1543, "Prev ON Times"=w1555) -> ("Trip Counter OUT"=w1562:i32[], "Previous Times OUT"=w1561:u32[], "Alarm Tripped"=w1533:bool, "Prev ON Times OUT"=w1560:u32[], "Alarm Message 1"=w1538:string, "Alarm Message 2"=w1537:string)  [unwired: 13 in]
        n589 = call "RPi HMI Com.vi"("Pump Data"=w1531, "Tank Data"=w1530, "Power Relays"=w1559, "Pump CMDs"=w1543, "App Config"=w1544, "Tank CMDs"=w1545, "Alarm"=w1553, "RPi HMI Mode"=RPi_HMI_Mode."Write Data", "In Test"=w1541, "Alarm Message 1"=w1552, "Controller Config"=w1542, "Alarm Message 2"=w1551, "Recording"=w1550, "Pumps Present"=w1525, "Time/Date"=w1548) -> ()  [unwired: 4 in, 1 out]
        n590 = call "Freeze PID.vi"("Run Profile"=w1541, "Controller CMDs"=w1543, "Controller Config"=w1542, "Power Relay"=w1546) -> ()  [unwired: 12 in]
        n591 = call "Data Logger Global.vi"("WebDAV Push"=w1529, "In Spec"=w1526, "Current Step"=w1528, "Step Time Left"=w1527, "Pump Data"=w1531, "Tank Data"=w1530, "Concat Data"=w1519, "Record Time (sec)"=w1520, "Write (F)"=TRUE) -> ()  [unwired: 3 in, 8 out]
        n592 = call "Get LS Data.vi"("Initial LS Data"=w1516, "FPGA Ref"=w1517) -> ("LS Data"=w1515:T15)  [unwired: 9 in]
        n593 = flat-sequence {
          frame #0 {
            n594 = Tick Count (ms)() -> (millisecond timer value=w1577:u32)
            n595 = feedback #4() -> (w1576:u32)  [unwired: 1 in]
            n596 = feedback-in #4(w1577) -> ()
            n597 = Subtract(x=w1577, y=w1576) -> (x-y=→"Read Inputs (ms)":u32)
          }
        }
        n598 = And(x=w1523, y=w1521) -> (x .and. y?=w1522:bool)
        n599 = case shown="True" w1522 {
          tunnel: w1549 -> [w1583 w1587]
          tunnel: [w1583 w1586] -> w1535
          frame False {
          }
          frame True {
            n600 = Insert Into Array(array=w1587, index=0, new element=Sequence_States."Reinit ADC" ("new element/subarray")) -> (w1586:T14[])
          }
        }
        n601 = Tick Count (ms)() -> (millisecond timer value=w1524:u32)
        n602 = call "Get Time and Date.vi"() -> ("Time/Date"=w1536:string)  [unwired: 11 in]
        n603 = case shown="True" w1533 {
          tunnel: w1535 -> [w1578 w1582]
          tunnel: [w1578 w1581] -> w1534
          frame False {
          }
          frame True {
            w1579 = T14[] [enum."Stop Profile", enum."Update Screen", enum."Disable Background", enum."Alarm"] items=["Main", "Init Files", "Init", "Unused", "Save As", "Start Profile", "Check Step Time", "Alarm", "Alarm Dismiss", "Run Step", "Stop Profile", "Cycle Reset", "Time Reset", "Time Reset All", "Time Set", "Tare CTs", "Save Profile", "Open Profile", "Get Profiles", "Update Screen", "Update Controls", "Save App Config", "Write Outputs", "Disable Background", "Enable Background", "Get/Release Control", "Log Fuel Change", "Fuel Change Popup", "Read Inputs", "Remote Timer Reset", "Controller Change", "Get Alarms", "Init Alarms", "Save Alarms", "Voltage Selection", "Set Watlow Temp 1", "Set Watlow Temp 2", "Get Pressure", "Write Tare Pressure", "Adjust Controls", "Reinit ADC", "Write Initial Times", "Write Pumps Present", "HMI Command", "Save Pump Times", "Check Pump Stop Time", "Save LS App Config", "Init Data File", "Reset LS Cycles", "Reset Anomalies", "Reset Opens", "Save LS Data", "Save LS Test Data", "Check Serial Numbers", "Main Tab", "Allow Data Note", "Resume Profile", "Pause Profile", "Allow Pause Note", "Clear Graph"]
            n604 = Insert Into Array(array=w1582, index=0, new element=w1579) -> (w1581:T14[])
          }
        }
        n605 = Bundle By Name(cluster=w1564, "Inputs Timer"=w1524, "Pump Data"=w1531, "Tank Data"=w1530, "Trip Counters"=w1562, "Previous Times"=w1561, "Alarm Latch"=w1533, "Prev ON Times"=w1560, "Alarm Message 1"=w1538, "Alarm Message 2"=w1537, "Time/Date"=w1536, "WebDAV Push"=w1518, "Concat Data"=w1518, "LS Data"=w1515) -> (w1539:T25)
      }
      frame "Update Screen" {
        # "Backup current step and time left every ten run minutes and at the start of every new step"
        n606 = Unbundle By Name(w1611) -> ("App Config.Cycles Completed"=→"Cycles Completed:":u32, "Current Step"=w1596:i32, "Step Time Left"=w1597:dbl, "Time/Date"=→"Time/Date":string, "Recording"=→"Recording":bool, "Pump Data"=w1613:T17, "Tank Data"=w1612:T23, "LS Data"=w1608:T15, "ARtime"=w1592:dbl, "ARactive"=w1595:bool, "Run Profile"=w1593:bool)
        "Step:" <- w1596
        "Time Left:" <- w1597
        n607 = Unbundle(w1613) -> ("Voltages"=→"Voltages":dbl[], "PumpCurrent"=→"PumpCurrent":dbl[], "Speed"=→"Speed":dbl[], "ControllerCurrent"=→"ControllerCurrent":dbl[], "Pressure"=→"Pressure":dbl[], "Flow"=→"Flow":dbl[], "Elapsed Time (Display)"=→"Elapsed Time:":dbl[], "Avg Pressure"=→"Avg Press:":dbl, "Avg Speed"=→"Ave. Speed":dbl)  [unwired: 1 out]
        n608 = Unbundle(w1612) -> ("PS Actual (V):"=→"PS Actual (V):":dbl, "Temp1"=→"Temp1":dbl, "Temp2"=→"Temp2":dbl)
        n609 = Unbundle(w1608) -> ("Total Cycles"=→"Total Cycles":u32[], "Steps"=→"Steps":u32[], "Anomalies Total"=→"Anomalies Total":i32[], "Cycles"=→"Cycles":u32[], "Anomalies/Cycle"=→"Anomalies/Cycle":i32[], "Anomalies (Last Cycle)"=→"Anomalies (Last Cycle)":i32[], "Opens"=→"Opens":i32[])
        n610 = case shown="True" w1593 {
          tunnel: [w1656 w1659] -> w1589
          tunnel: w1631 -> [w1656 w1658]
          frame False {
          }
          frame True {
            w1657 = T14[] [enum."Save Pump Times", enum."Update Controls"] items=["Main", "Init Files", "Init", "Unused", "Save As", "Start Profile", "Check Step Time", "Alarm", "Alarm Dismiss", "Run Step", "Stop Profile", "Cycle Reset", "Time Reset", "Time Reset All", "Time Set", "Tare CTs", "Save Profile", "Open Profile", "Get Profiles", "Update Screen", "Update Controls", "Save App Config", "Write Outputs", "Disable Background", "Enable Background", "Get/Release Control", "Log Fuel Change", "Fuel Change Popup", "Read Inputs", "Remote Timer Reset", "Controller Change", "Get Alarms", "Init Alarms", "Save Alarms", "Voltage Selection", "Set Watlow Temp 1", "Set Watlow Temp 2", "Get Pressure", "Write Tare Pressure", "Adjust Controls", "Reinit ADC", "Write Initial Times", "Write Pumps Present", "HMI Command", "Save Pump Times", "Check Pump Stop Time", "Save LS App Config", "Init Data File", "Reset LS Cycles", "Reset Anomalies", "Reset Opens", "Save LS Data", "Save LS Test Data", "Check Serial Numbers", "Main Tab", "Allow Data Note", "Resume Profile", "Pause Profile", "Allow Pause Note", "Clear Graph"]
            n611 = Insert Into Array(array=w1658, index=0, new element=w1657) -> (w1659:T14[])
          }
        }
        n612 = Compound Arithmetic op=AND(w1595, invert w1593) -> (w1594:bool)
        n613 = Quotient & Remainder(x=w1597, y=600.0) -> (floor(x/y)=w1598:dbl)  [unwired: 1 out]
        n614 = case shown="True" w1594 {
          selector: w1594 -> [w1637 _]
          tunnel: w1592 -> [_ w1646]
          tunnel: [w1637 w1638] -> w1591
          frame False {
          }
          frame True {
            n615 = Get Date/Time In Seconds() -> (seconds since 1Jan1904=w1648:timestamp)
            n616 = To Double Precision Float(number=w1648) -> (double precision float=w1647:dbl)
            n617 = Subtract(x=w1647, y=w1646) -> (x-y=w1644:dbl)
            n618 = To Long Integer(number=w1644) -> (32bit integer=w1643:i32)
            n619 = Subtract(x="ARtiming", y=w1643) -> (x-y=w1642:i32)
            n620 = Less Or Equal To 0?(x=w1642) -> (x <= 0?=w1639:bool)
            n621 = Select(t=0, s=w1639, f=w1642) -> (s? t:f=→"ARclock":i32)
            n622 = Not(x=w1639) -> (.not. x?=w1638:bool)
            n623 = case shown="False" w1638 {
              selector: w1638 -> [_ w1649]
              frame True {
              }
              frame False {
                n624 = property on="pb.Pause/Resume" class="Bool (strict)"("Val(Sgnl)"=w1649) -> ()  [unwired: 2 in, 2 out]
              }
            }
          }
        }
        n625 = feedback #5(w1598) -> (w1599:dbl)
        n626 = feedback-in #5(w1598) -> ()
        n627 = Not Equal?(x=w1599, y=w1598) -> (x != y?=w1590:bool)
        n628 = flat-sequence {
          frame #0 {
            n629 = Tick Count (ms)() -> (millisecond timer value=w1655:u32)
            n630 = feedback #6() -> (w1654:u32)  [unwired: 1 in]
            n631 = feedback-in #6(w1655) -> ()
            n632 = Subtract(x=w1655, y=w1654) -> (x-y=→"Update Screen (ms)":u32)
          }
        }
        n633 = call "App Global.vi"() -> ("CPU Usage OUT"=→"CPU Usage:":dbl, "Login OUT"=w1614:bool)  [unwired: 9 in, 1 out]
        n634 = case shown="True" w1590 {
          tunnel: w1597 -> [_ w1651]
          tunnel: w1596 -> [_ w1652]
          frame False {
          }
          frame True {
            n635 = call "Handle Profile Resume Info.vi"("Read(F)/Write(T)"=TRUE ("Write(T)/Read(F)"), "Current Step In"=w1652, "Step Time Left In"=w1651) -> ()  [unwired: 11 in, 2 out]
          }
        }
        n636 = local write "Login"(w1614) -> ()
        n637 = Tick Count (ms)() -> (millisecond timer value=w1609:u32)
        n638 = case shown="True" w1590 {
          tunnel: [w1632 w1635] -> w1588
          tunnel: w1589 -> [w1632 w1634]
          frame False {
          }
          frame True {
            w1633 = T14[] [enum."Save LS Data"] items=["Main", "Init Files", "Init", "Unused", "Save As", "Start Profile", "Check Step Time", "Alarm", "Alarm Dismiss", "Run Step", "Stop Profile", "Cycle Reset", "Time Reset", "Time Reset All", "Time Set", "Tare CTs", "Save Profile", "Open Profile", "Get Profiles", "Update Screen", "Update Controls", "Save App Config", "Write Outputs", "Disable Background", "Enable Background", "Get/Release Control", "Log Fuel Change", "Fuel Change Popup", "Read Inputs", "Remote Timer Reset", "Controller Change", "Get Alarms", "Init Alarms", "Save Alarms", "Voltage Selection", "Set Watlow Temp 1", "Set Watlow Temp 2", "Get Pressure", "Write Tare Pressure", "Adjust Controls", "Reinit ADC", "Write Initial Times", "Write Pumps Present", "HMI Command", "Save Pump Times", "Check Pump Stop Time", "Save LS App Config", "Init Data File", "Reset LS Cycles", "Reset Anomalies", "Reset Opens", "Save LS Data", "Save LS Test Data", "Check Serial Numbers", "Main Tab", "Allow Data Note", "Resume Profile", "Pause Profile", "Allow Pause Note", "Clear Graph"]
            n639 = Insert Into Array(array=w1634, index=0, new element=w1633) -> (w1635:T14[])
          }
        }
        n640 = Bundle By Name(cluster=w1611, "Screen Timer"=w1609, "ARactive"=w1591) -> (w1610:T25)
      }
      frame "Update Controls" {
        w1685 = bool[] [FALSE, FALSE, FALSE, FALSE, FALSE, FALSE] ("pb.Resets")
        w1686 = T14[] [] items=["Main", "Init Files", "Init", "Unused", "Save As", "Start Profile", "Check Step Time", "Alarm", "Alarm Dismiss", "Run Step", "Stop Profile", "Cycle Reset", "Time Reset", "Time Reset All", "Time Set", "Tare CTs", "Save Profile", "Open Profile", "Get Profiles", "Update Screen", "Update Controls", "Save App Config", "Write Outputs", "Disable Background", "Enable Background", "Get/Release Control", "Log Fuel Change", "Fuel Change Popup", "Read Inputs", "Remote Timer Reset", "Controller Change", "Get Alarms", "Init Alarms", "Save Alarms", "Voltage Selection", "Set Watlow Temp 1", "Set Watlow Temp 2", "Get Pressure", "Write Tare Pressure", "Adjust Controls", "Reinit ADC", "Write Initial Times", "Write Pumps Present", "HMI Command", "Save Pump Times", "Check Pump Stop Time", "Save LS App Config", "Init Data File", "Reset LS Cycles", "Reset Anomalies", "Reset Opens", "Save LS Data", "Save LS Test Data", "Check Serial Numbers", "Main Tab", "Allow Data Note", "Resume Profile", "Pause Profile", "Allow Pause Note", "Clear Graph"]
        n641 = Unbundle By Name(w1688) -> ("App Config.Stagger Time (ms)"=w1697:i32, "Profile"=w1698:string[][], "App Config.Current Profile"=w1693:string, "App Config.CA Number"=w1692:string, "App Config.Controller Type:"=w1699:T3, "App Config.Pumps Present"=w1689:T8, "App Config.Tank 1 Fuel"=w1696:string, "App Config.Tank 2 Fuel"=w1695:string, "App Config.Serial Numbers"=w1694:T41, "App Config.Target Voltage"=w1691:dbl, "App Config.Target Pressure"=w1690:dbl, "Email Alarms Disabled"=w1684:bool, "Run Profile"=w1683:bool, "Recording"=w1682:bool, "Tank CMDs.Press CMD"=w1681:dbl, "Controller CMDs"=w1680:dbl[], "Tank CMDs.PS CMD"=w1679:dbl, "Power Relay"=w1678:T8, "Ignition Relay"=w1663:T8, "WebDAV Push"=w1662:bool, "Concat Data"=w1661:bool, "LS App Config.LS Power (Freq):"=w1667:dbl, "LS App Config.LS Power (Duty):"=w1666:dbl, "LS App Config.Bank 1 Present"=w1665:T2, "LS App Config.Bank 2 Present"=w1664:T1, "LS App Config.Data File Name:"=w1668:string, "LS App Config.Record Bursts"=w1677:bool, "LS App Config.RecInterval(s)"=w1676:i32, "LS App Config.RecDuration(s)"=w1675:i32, "LS App Config.RecFrequeny (Hz)"=w1674:i32, "LS App Config.DetectionMode"=w1673:i32, "LS App Config.Serial Numbers"=w1672:string[], "Bank 1 State:"=w1670:u16, "Bank 2 State:"=w1669:u16)
        n642 = Array To Cluster(array=w1672) -> (cluster=w1671:T49)
        n643 = local write "LS Cycle Time (ms):"(w1667) -> ()
        n644 = local write "LS On Time (ms):"(w1666) -> ()
        n645 = local write "Bank 1"(w1665) -> ()
        n646 = local write "Bank 2"(w1664) -> ()
        n647 = local write "Data File Name:"(w1668) -> ()
        n648 = local write "Record During Profile"(w1677) -> ()
        n649 = local write "Interval Between\nRecordings (s):"(w1676) -> ()
        n650 = local write "Recording\nDuration (s):"(w1675) -> ()
        n651 = local write "Recording\nFrequency (Hz):"(w1674) -> ()
        n652 = local write "Detection Mode:"(w1673) -> ()
        n653 = local write "LS Serial Numbers"(w1671) -> ()
        n654 = local write "Bank 1 Power State:"(w1670) -> ()
        n655 = local write "Bank 2 Power State:"(w1669) -> ()
        n656 = local write "pb.Run Profile"(w1683) -> ()
        n657 = local write "Recording"(w1682) -> ()
        n658 = local write "PressureCMD"(w1681) -> ()
        n659 = local write "Controller\nCMD"(w1680) -> ()
        n660 = local write "Power Supply Cmd:"(w1679) -> ()
        n661 = local write "Power Relay"(w1678) -> ()
        n662 = local write "Ignition Relay"(w1663) -> ()
        n663 = local write "WebDAV Push"(w1662) -> ()
        n664 = local write "Concat Data"(w1661) -> ()
        n665 = local write "pb.Resets"(w1685) -> ()
        n666 = local write "pb.Sets"(w1685) -> ()
        n667 = case shown="False" w1683 {
          tunnel: w1699 -> [w1713 _]
          tunnel: w1698 -> [w1712 _]
          tunnel: w1697 -> [w1711 _]
          tunnel: w1696 -> [w1710 _]
          tunnel: w1695 -> [w1709 _]
          tunnel: w1694 -> [w1708 _]
          tunnel: w1693 -> [w1707 _]
          tunnel: w1692 -> [w1706 _]
          tunnel: w1691 -> [w1705 _]
          tunnel: w1690 -> [w1704 _]
          tunnel: w1689 -> [w1703 _]
          tunnel: w1684 -> [w1702 _]
          frame False {
            n668 = local write "Stagger Time (ms):"(w1711) -> ()
            n669 = local write "Profile:"(w1712) -> ()
            n670 = local write "Profile Name:"(w1707) -> ()
            n671 = local write "CA Number:"(w1706) -> ()
            n672 = local write "Controller Type:"(w1713) -> ()
            n673 = local write "Pumps Present"(w1703) -> ()
            n674 = local write "Tank 1 Fuel Type:"(w1710) -> ()
            n675 = local write "Tank 2 Fuel Type:"(w1709) -> ()
            n676 = local write "Serial Numbers"(w1708) -> ()
            n677 = local write "Target Voltage:"(w1705) -> ()
            n678 = local write "Target Pressure:"(w1704) -> ()
            n679 = local write "Disable Alarm Email"(w1702) -> ()
            "Email Alarms Disabled" <- w1702
          }
          frame True {
          }
        }
        n680 = Insert Into Array(array=w1700, index=0, new element=w1686) -> (w1701:T14[])
      }
      frame "Check Pump Stop Time" {
        n681 = Unbundle By Name(w1723) -> ("Pump Data.Elapsed Time"=w1715:dbl[], "App Config.Pumps Present"=w1717:T8)
        n682 = Cluster To Array(cluster=w1717) -> (array=w1716:bool[])
        n683 = for {
          tunnel: w1716 -> [w1724] mode=indexing
          tunnel: w1715 -> [w1725] mode=indexing
          tunnel: [w1725] -> w1714 mode=indexing if=w1724
        }
        n684 = Array Max & Min(array=w1714) -> (min value=w1722:dbl)  [unwired: 3 out]
        n685 = Greater?(x=w1722, y="Stop Time:") -> (0:w1718:bool)
        n686 = case shown="True" w1718 {
          tunnel: w1720 -> [w1726 w1728]
          tunnel: [w1726 w1727] -> w1719
          frame False {
          }
          frame True {
            w1729 = T14[] [enum."Stop Profile"] items=["Main", "Init Files", "Init", "Unused", "Save As", "Start Profile", "Check Step Time", "Alarm", "Alarm Dismiss", "Run Step", "Stop Profile", "Cycle Reset", "Time Reset", "Time Reset All", "Time Set", "Tare CTs", "Save Profile", "Open Profile", "Get Profiles", "Update Screen", "Update Controls", "Save App Config", "Write Outputs", "Disable Background", "Enable Background", "Get/Release Control", "Log Fuel Change", "Fuel Change Popup", "Read Inputs", "Remote Timer Reset", "Controller Change", "Get Alarms", "Init Alarms", "Save Alarms", "Voltage Selection", "Set Watlow Temp 1", "Set Watlow Temp 2", "Get Pressure", "Write Tare Pressure", "Adjust Controls", "Reinit ADC", "Write Initial Times", "Write Pumps Present", "HMI Command", "Save Pump Times", "Check Pump Stop Time", "Save LS App Config", "Init Data File", "Reset LS Cycles", "Reset Anomalies", "Reset Opens", "Save LS Data", "Save LS Test Data", "Check Serial Numbers", "Main Tab", "Allow Data Note", "Resume Profile", "Pause Profile", "Allow Pause Note", "Clear Graph"]
            n687 = Insert Into Array(array=w1728, index=0, new element=w1729) -> (w1727:T14[])
          }
        }
      }
      frame "Stop Profile" {
        w1743 = u16 0 items=["0 - Off", "1 - On", "2 - Pulsing"] ("Bank 1 Power State:")
        w1742 = FALSE ("Running?")
        w1754 = T14[] [enum."Write Outputs", enum."Update Controls"] items=["Main", "Init Files", "Init", "Unused", "Save As", "Start Profile", "Check Step Time", "Alarm", "Alarm Dismiss", "Run Step", "Stop Profile", "Cycle Reset", "Time Reset", "Time Reset All", "Time Set", "Tare CTs", "Save Profile", "Open Profile", "Get Profiles", "Update Screen", "Update Controls", "Save App Config", "Write Outputs", "Disable Background", "Enable Background", "Get/Release Control", "Log Fuel Change", "Fuel Change Popup", "Read Inputs", "Remote Timer Reset", "Controller Change", "Get Alarms", "Init Alarms", "Save Alarms", "Voltage Selection", "Set Watlow Temp 1", "Set Watlow Temp 2", "Get Pressure", "Write Tare Pressure", "Adjust Controls", "Reinit ADC", "Write Initial Times", "Write Pumps Present", "HMI Command", "Save Pump Times", "Check Pump Stop Time", "Save LS App Config", "Init Data File", "Reset LS Cycles", "Reset Anomalies", "Reset Opens", "Save LS Data", "Save LS Test Data", "Check Serial Numbers", "Main Tab", "Allow Data Note", "Resume Profile", "Pause Profile", "Allow Pause Note", "Clear Graph"]
        w1759 = T8 {"Pump 1"=FALSE, "Pump 2"=FALSE, "Pump 3"=FALSE, "Pump 4"=FALSE, "Pump 5"=FALSE, "Pump 6"=FALSE} ("Power Relay")
        n688 = Unbundle By Name(w1758) -> ("Controller Config.Stop Command"=w1757:dbl, "LS App Config.Record Bursts"=w1748:bool, "LS App Config.RecInterval(s)"=w1747:i32, "LS App Config.RecDuration(s)"=w1746:i32, "LS App Config.RecFrequeny (Hz)"=w1745:i32, "LS Data Filepath"=w1744:path, "LS App Config.Record Constant"=w1739:bool, "LS App Config.Serial Numbers"=w1738:string[], "Login"=w1741:bool, "Current Step"=w1734:i32, "Step Time Left"=w1733:dbl)
        n689 = call "Handle Profile Resume Info.vi"("Read(F)/Write(T)"=TRUE, "Current Step In"=w1734, "Step Time Left In"=w1733) -> ()  [unwired: 11 in, 2 out]
        n690 = Bundle(cluster=T30 {"Running?"=FALSE, "Profile Record"=FALSE, "RecordInterval"=0, "RecordDuration"=0, "RecordFreq"=0, "Data Filepath"=path "", "Hr Record"=FALSE, "Serial Numbers"=[]} ("LS Cluster In"), "Running?"=w1742, "Profile Record"=w1748, "RecordInterval"=w1747, "RecordDuration"=w1746, "RecordFreq"=w1745, "Data Filepath"=w1744, "Hr Record"=w1739, "Serial Numbers"=w1738) -> (w1749:T30)
        n691 = call "LS Data Global.vi"("Mode"=enum16{"Read", "Engine Writes", "Main Writes"}."Main Writes", "LS Cluster In"=w1749) -> ()  [unwired: 10 in, 4 out]
        n692 = case shown="True" w1741 {
          frame False {
          }
          frame True {
            w1765 = T31."Enabled" ("Disabled")
            n693 = property on="Bank 1" class="Clust (strict)"("DisabledEnum"=w1765) -> ()  [unwired: 2 in, 2 out]
            n694 = property on="Bank 2" class="Clust (strict)"("DisabledEnum"=w1765) -> ()  [unwired: 2 in, 2 out]
            n695 = property on="Live Data Tab" class="TabCtl (strict)"("DisabledEnum"=w1765) -> ()  [unwired: 2 in, 2 out]
            n696 = property on="Pump Timers Tab" class="TabCtl (strict)"("DisabledEnum"=w1765) -> ()  [unwired: 2 in, 2 out]
          }
        }
        n697 = disable-structure shown="Disabled" {
          frame Disabled {
            n698 = call "Data Logger Main.vi"("Data Logger Mode"=Data_Logger_Mode."Stop") -> ()  [unwired: 19 in]
          }
          frame Enabled {
          }
        }
        n699 = local write "Stop Time Enable"(FALSE ("Stop Time Enable")) -> ()
        n700 = Initialize Array(w1757, 6 ("dimension size")) -> (w1755:dbl[])
        n701 = local write "pb.Pause/Resume"(TRUE) -> ()
        n702 = local write "Bank 1 Power State:"(w1743) -> ()
        n703 = local write "Bank 2 Power State:"(w1743) -> ()
        n704 = Bundle By Name(cluster=w1758, "pb.Run Profile"=w1742, "Run Profile"=FALSE, "Controller CMDs"=w1755, "Power Relay"=w1759, "Ignition Relay"=w1759, "Tank CMDs.Press CMD"=0.0, "Recording"=FALSE, "Bank 1 State:"=w1743, "Bank 2 State:"=w1743, "ARactive"=FALSE) -> (w1752:T25)
        n705 = local write "ARclock"(0 ("ARclock")) -> ()
        n706 = Insert Into Array(array=w1762, index=0, new element=w1754) -> (w1761:T14[])
      }
      frame "Pause Profile" {
        w1779 = u16 0 items=["0 - Off", "1 - On", "2 - Pulsing"] ("Bank 1 Power State:")
        w1778 = FALSE ("Running?")
        w1790 = T14[] [enum."Write Outputs", enum."Update Controls"] items=["Main", "Init Files", "Init", "Unused", "Save As", "Start Profile", "Check Step Time", "Alarm", "Alarm Dismiss", "Run Step", "Stop Profile", "Cycle Reset", "Time Reset", "Time Reset All", "Time Set", "Tare CTs", "Save Profile", "Open Profile", "Get Profiles", "Update Screen", "Update Controls", "Save App Config", "Write Outputs", "Disable Background", "Enable Background", "Get/Release Control", "Log Fuel Change", "Fuel Change Popup", "Read Inputs", "Remote Timer Reset", "Controller Change", "Get Alarms", "Init Alarms", "Save Alarms", "Voltage Selection", "Set Watlow Temp 1", "Set Watlow Temp 2", "Get Pressure", "Write Tare Pressure", "Adjust Controls", "Reinit ADC", "Write Initial Times", "Write Pumps Present", "HMI Command", "Save Pump Times", "Check Pump Stop Time", "Save LS App Config", "Init Data File", "Reset LS Cycles", "Reset Anomalies", "Reset Opens", "Save LS Data", "Save LS Test Data", "Check Serial Numbers", "Main Tab", "Allow Data Note", "Resume Profile", "Pause Profile", "Allow Pause Note", "Clear Graph"]
        w1795 = T8 {"Pump 1"=FALSE, "Pump 2"=FALSE, "Pump 3"=FALSE, "Pump 4"=FALSE, "Pump 5"=FALSE, "Pump 6"=FALSE} ("Power Relay")
        n707 = disable-structure shown="Disabled" {
          frame Disabled {
            n708 = call "Data Logger Main.vi"("Data Logger Mode"=Data_Logger_Mode."Stop") -> ()  [unwired: 19 in]
          }
          frame Enabled {
          }
        }
        n709 = Unbundle By Name(w1794) -> ("Controller Config.Stop Command"=w1793:dbl, "LS App Config.Record Bursts"=w1784:bool, "LS App Config.RecInterval(s)"=w1783:i32, "LS App Config.RecDuration(s)"=w1782:i32, "LS App Config.RecFrequeny (Hz)"=w1781:i32, "LS Data Filepath"=w1780:path, "LS App Config.Record Constant"=w1775:bool, "LS App Config.Serial Numbers"=w1774:string[], "Login"=w1777:bool, "Current Step"=w1770:i32, "Step Time Left"=w1769:dbl, "Run Profile"=w1768:bool)
        n710 = call "Handle Profile Resume Info.vi"("Read(F)/Write(T)"=TRUE, "Current Step In"=w1770, "Step Time Left In"=w1769) -> ()  [unwired: 11 in, 2 out]
        n711 = Bundle(cluster=T30 {"Running?"=FALSE, "Profile Record"=FALSE, "RecordInterval"=0, "RecordDuration"=0, "RecordFreq"=0, "Data Filepath"=path "", "Hr Record"=FALSE, "Serial Numbers"=[]} ("LS Cluster In"), "Running?"=w1778, "Profile Record"=w1784, "RecordInterval"=w1783, "RecordDuration"=w1782, "RecordFreq"=w1781, "Data Filepath"=w1780, "Hr Record"=w1775, "Serial Numbers"=w1774) -> (w1785:T30)
        n712 = call "LS Data Global.vi"("Mode"=enum16{"Read", "Engine Writes", "Main Writes"}."Main Writes", "LS Cluster In"=w1785) -> ()  [unwired: 10 in, 4 out]
        n713 = case shown="True" w1777 {
          frame False {
          }
          frame True {
            w1801 = T31."Enabled" ("Disabled")
            n714 = property on="Bank 1" class="Clust (strict)"("DisabledEnum"=w1801) -> ()  [unwired: 2 in, 2 out]
            n715 = property on="Bank 2" class="Clust (strict)"("DisabledEnum"=w1801) -> ()  [unwired: 2 in, 2 out]
            n716 = property on="Live Data Tab" class="TabCtl (strict)"("DisabledEnum"=w1801) -> ()  [unwired: 2 in, 2 out]
            n717 = property on="Pump Timers Tab" class="TabCtl (strict)"("DisabledEnum"=w1801) -> ()  [unwired: 2 in, 2 out]
          }
        }
        n718 = local write "Stop Time Enable"(FALSE ("Stop Time Enable")) -> ()
        n719 = Initialize Array(w1793, 6 ("dimension size")) -> (w1791:dbl[])
        n720 = local write "pb.Pause/Resume"(TRUE) -> ()
        n721 = local write "Bank 1 Power State:"(w1779) -> ()
        n722 = local write "Bank 2 Power State:"(w1779) -> ()
        n723 = Get Date/Time In Seconds() -> (seconds since 1Jan1904=w1767:timestamp)
        n724 = To Double Precision Float(number=w1767) -> (double precision float=w1766:dbl)
        n725 = Bundle By Name(cluster=w1794, "pb.Run Profile"=w1778, "Run Profile"=FALSE, "Controller CMDs"=w1791, "Power Relay"=w1795, "Ignition Relay"=w1795, "Tank CMDs.Press CMD"=0.0, "Recording"=FALSE, "Bank 1 State:"=w1779, "Bank 2 State:"=w1779, "ARactive"=w1768, "ARtime"=w1766) -> (w1788:T25)
        n726 = Insert Into Array(array=w1798, index=0, new element=w1790) -> (w1797:T14[])
      }
      frame "Save As" {
        n727 = property on="Save As Tab" class="TabCtl (strict)"("Visible"=TRUE) -> (error out=w1806:errorcluster)  [unwired: 2 in, 1 out]
        n728 = while {
          tunnel: ["pb.Save As OK"] -> w1812
          tunnel: w1806 -> [_]
          stop <- w1814 stop-if-true
          n729 = Wait (ms)(milliseconds to wait=u32 10) -> ()  [unwired: 1 out]
          n730 = Or(x="pb.Save As OK", y="pb.Save As Cancel") -> (x .or. y?=w1814:bool)
        }
        n731 = Unbundle By Name(w1810) -> ("App Config.Profiles Path"=w1811:path, "Profile"=w1808:string[][])
        n732 = case shown="True" w1812 {
          tunnel: w1811 -> [_ w1822]
          tunnel: [w1817 w1819] -> w1803
          tunnel: w1810 -> [w1818 w1824]
          tunnel: [w1818 w1823] -> w1809
          tunnel: w1808 -> [_ w1821]
          frame False {
            w1817 = T14[] [enum."Enable Background"] items=["Main", "Init Files", "Init", "Unused", "Save As", "Start Profile", "Check Step Time", "Alarm", "Alarm Dismiss", "Run Step", "Stop Profile", "Cycle Reset", "Time Reset", "Time Reset All", "Time Set", "Tare CTs", "Save Profile", "Open Profile", "Get Profiles", "Update Screen", "Update Controls", "Save App Config", "Write Outputs", "Disable Background", "Enable Background", "Get/Release Control", "Log Fuel Change", "Fuel Change Popup", "Read Inputs", "Remote Timer Reset", "Controller Change", "Get Alarms", "Init Alarms", "Save Alarms", "Voltage Selection", "Set Watlow Temp 1", "Set Watlow Temp 2", "Get Pressure", "Write Tare Pressure", "Adjust Controls", "Reinit ADC", "Write Initial Times", "Write Pumps Present", "HMI Command", "Save Pump Times", "Check Pump Stop Time", "Save LS App Config", "Init Data File", "Reset LS Cycles", "Reset Anomalies", "Reset Opens", "Save LS Data", "Save LS Test Data", "Check Serial Numbers", "Main Tab", "Allow Data Note", "Resume Profile", "Pause Profile", "Allow Pause Note", "Clear Graph"]
          }
          frame True {
            w1819 = T14[] [enum."Enable Background", enum."Get Profiles"] items=["Main", "Init Files", "Init", "Unused", "Save As", "Start Profile", "Check Step Time", "Alarm", "Alarm Dismiss", "Run Step", "Stop Profile", "Cycle Reset", "Time Reset", "Time Reset All", "Time Set", "Tare CTs", "Save Profile", "Open Profile", "Get Profiles", "Update Screen", "Update Controls", "Save App Config", "Write Outputs", "Disable Background", "Enable Background", "Get/Release Control", "Log Fuel Change", "Fuel Change Popup", "Read Inputs", "Remote Timer Reset", "Controller Change", "Get Alarms", "Init Alarms", "Save Alarms", "Voltage Selection", "Set Watlow Temp 1", "Set Watlow Temp 2", "Get Pressure", "Write Tare Pressure", "Adjust Controls", "Reinit ADC", "Write Initial Times", "Write Pumps Present", "HMI Command", "Save Pump Times", "Check Pump Stop Time", "Save LS App Config", "Init Data File", "Reset LS Cycles", "Reset Anomalies", "Reset Opens", "Save LS Data", "Save LS Test Data", "Check Serial Numbers", "Main Tab", "Allow Data Note", "Resume Profile", "Pause Profile", "Allow Pause Note", "Clear Graph"]
            n733 = call "Save Profile.vi"("Profile"=w1821, "Current Profile"="New Profile Name:", "Profiles Path"=w1822) -> ()  [unwired: 8 in, 1 out]
            n734 = Bundle By Name(cluster=w1824, "App Config.Current Profile"="New Profile Name:") -> (w1823:T25)
          }
        }
        n735 = Insert Into Array(array=w1805, index=0, new element=w1803) -> (w1804:T14[])
      }
      frame "Save App Config" {
        n736 = Unbundle By Name(w1836) -> ("App Config"=w1827:T6)
        n737 = Unbundle By Name(w1827) -> ("Cycle Threshold:"=w1826:dbl, "Cycle Pts to Avg:"=w1825:i32)
        n738 = disable-structure shown="Disabled" {
          disable-tunnel: w1828 -> [w1840 _]
          disable-tunnel: w1826 -> [w1839 _]
          disable-tunnel: w1825 -> [w1838 _]
          frame Disabled {
            n739 = xnode "Read/Write Control"("FPGA VI Reference In"=w1840, "Cycle Threshold"=w1839, "Points to Avg"=w1838) -> ()  [unwired: 1 in, 2 out]
          }
          frame Enabled {
          }
        }
        n740 = call <vilib>:"Open Config Data.vi"("create file if necessary (T)"=TRUE, "configuration file path"=path "c:/App Config.ini") -> ("error out"=w1830:errorcluster, "refnum"=w1834:T47)  [unwired: 7 in, 1 out]
        n741 = call "Read Write App Config.vi"("Write (F)"=TRUE, "Error IN"=w1830, "App Config"=w1827, "Refnum in"=w1834) -> ("Error OUT"=w1832:errorcluster, "Refnum out"=w1833:T47)  [unwired: 5 in, 1 out]
        n742 = call <vilib>:"Close Config Data.vi"("error in (no error)"=w1832, "refnum"=w1833) -> ()  [unwired: 8 in, 2 out]
      }
      frame "Save LS App Config" {
        n743 = Unbundle By Name(w1868) -> ("LS App Config"=w1850:T13, "pb.Run Profile"=w1861:bool, "LS App Config.Record Bursts"=w1846:bool, "LS App Config.RecInterval(s)"=w1860:i32, "LS App Config.RecDuration(s)"=w1859:i32, "LS App Config.RecFrequeny (Hz)"=w1858:i32, "LS Data Filepath"=w1856:path, "LS App Config.Record Constant"=w1847:bool, "LS App Config.Serial Numbers"=w1851:string[], "App Config.CA Number"=w1849:string, "LS App Config.Data File Name:"=w1848:string)
        n744 = Empty String/Path?(string/path=w1849) -> (empty?=w1854:bool)
        n745 = Empty String/Path?(string/path=w1848) -> (empty?=w1853:bool)
        n746 = call <vilib>:"Open Config Data.vi"("create file if necessary (T)"=TRUE, "configuration file path"=path "c:/LS App Config.ini") -> ("error out"=w1863:errorcluster, "refnum"=w1866:T47)  [unwired: 7 in, 1 out]
        n747 = Bundle By Name(cluster=T30 {"Running?"=FALSE, "Profile Record"=FALSE, "RecordInterval"=0, "RecordDuration"=0, "RecordFreq"=0, "Data Filepath"=path "", "Hr Record"=FALSE, "Serial Numbers"=[]} ("LS Cluster In"), "Running?"=w1861, "Profile Record"=w1846, "RecordInterval"=w1860, "RecordDuration"=w1859, "RecordFreq"=w1858, "Data Filepath"=w1856, "Hr Record"=w1847, "Serial Numbers"=w1851) -> (w1857:T30)
        n748 = Or(x=w1854, y=w1853) -> (x .or. y?=w1852:bool)
        n749 = call "Read Write LS App Config.vi"("Write (F)"=TRUE, "Error IN"=w1863, "LS App Config In"=w1850, "Refnum in"=w1866) -> ("Error OUT"=w1864:errorcluster, "Refnum out"=w1865:T47)  [unwired: 5 in, 1 out]
        n750 = case shown="False" w1852 {
          tunnel: w1847 -> [w1871 _]
          tunnel: w1846 -> [w1872 _]
          tunnel: [w1874 FALSE ("Record During Profile")] -> w1843
          tunnel: [w1873 T31."Disabled and Grayed Out" ("Disabled")] -> w1845
          tunnel: [w1876 FALSE ("Record During Profile")] -> w1842
          tunnel: [w1875 T31."Disabled and Grayed Out" ("Disabled")] -> w1844
          frame False {
            # "Valid file"
            n751 = And(x=w1872, y=w1871) -> (x .and. y?=w1877:bool)
            n752 = case shown="False" w1877 {
              tunnel: [w1878 FALSE] -> w1876
              tunnel: [w1882 T31."Enabled" ("Disabled")] -> w1875
              tunnel: [w1883 FALSE] -> w1874
              tunnel: [w1879 T31."Enabled" ("Disabled")] -> w1873
              tunnel: w1872 -> [w1878 _]
              tunnel: w1871 -> [w1883 _]
              frame False {
                n753 = Select(t=T31."Disabled and Grayed Out" ("Disabled"), s=w1883, f=T31."Enabled" ("Disabled")) -> (s? t:f=w1882:T31)
                n754 = Select(t=T31."Disabled and Grayed Out" ("Disabled"), s=w1878, f=T31."Enabled" ("Disabled")) -> (s? t:f=w1879:T31)
              }
              frame True {
                # "Reset allowing new selection"
                # "Error! - Cannot have both saves active"
              }
            }
          }
          frame True {
            # "Missing Data File Name/CA Number\nCannot Save"
          }
        }
        n755 = call <vilib>:"Close Config Data.vi"("error in (no error)"=w1864, "refnum"=w1865) -> ()  [unwired: 8 in, 2 out]
        n756 = call "LS Data Global.vi"("Mode"=enum16{"Read", "Engine Writes", "Main Writes"}."Main Writes", "LS Cluster In"=w1857) -> ()  [unwired: 10 in, 4 out]
        n757 = property on="Record During Profile" class="Bool (strict)"("Value"=w1842, "DisabledEnum"=w1844) -> ()  [unwired: 2 in, 2 out]
        n758 = property on="Record Constant" class="Bool (strict)"("Value"=w1843, "DisabledEnum"=w1845) -> ()  [unwired: 2 in, 2 out]
      }
      frame "Save Pump Times" {
        n759 = Unbundle By Name(w1898) -> ("Pump Data.Elapsed Time"=w1897:dbl[])
        n760 = Array Size(array=w1897) -> (size(s)=w1896:i32)
        n761 = Equal?(x=w1896, y=6) -> (x = y?=w1894:bool)
        n762 = case shown="True" w1894 {
          tunnel: w1897 -> [_ w1901]
          frame False {
          }
          frame True {
            n763 = Write to Binary File(file (use dialog)=path "c:/ElapsedTimes", data=w1901) -> (refnum out=w1902:refnum<file>, error out=w1903:errorcluster)  [unwired: 4 in, 1 out]
            n764 = Close File(refnum=w1902, error in=w1903) -> ()  [unwired: 2 out]
          }
        }
      }
      frame "Disable Background" {
        w1904 = T31."Disabled and Grayed Out" ("Disabled")
        n765 = property on="Main Tab" class="TabCtl (strict)"("DisabledEnum"=w1904) -> ()  [unwired: 2 in, 2 out]
        n766 = property on="pb.Stop Profile" class="Bool"("DisabledEnum"=w1904) -> ()  [unwired: 2 in, 2 out]
        n767 = property on="Monitoring Tab" class="TabCtl (strict)"("DisabledEnum"=w1904) -> ()  [unwired: 2 in, 2 out]
        n768 = property on="Title Tab" class="TabCtl (strict)"("DisabledEnum"=w1904) -> ()  [unwired: 2 in, 2 out]
        n769 = property on="CPU Usage:" class="DigNum (strict)"("DisabledEnum"=w1904) -> ()  [unwired: 2 in, 2 out]
        n770 = property on="Pump Timers Tab" class="TabCtl (strict)"("DisabledEnum"=w1904) -> ()  [unwired: 2 in, 2 out]
        n771 = property on="Live Data Tab" class="TabCtl (strict)"("DisabledEnum"=w1904) -> ()  [unwired: 2 in, 2 out]
      }
      frame "Enable Background" {
        w1907 = FALSE ("Visible")
        w1908 = T31."Enabled" ("Disabled")
        n772 = disable-structure shown="Enabled" {
          disable-tunnel: w1910 -> [w1913 w1915]
          frame Disabled {
            n773 = xnode "Read/Write Control"("FPGA VI Reference In"=w1913, "Timer Resets"=bool[] [FALSE, FALSE, FALSE, FALSE, FALSE, FALSE] ("array")) -> ()  [unwired: 1 in, 2 out]
          }
          frame Enabled {
            w1914 = bool[] [FALSE, FALSE, FALSE, FALSE, FALSE, FALSE, FALSE, FALSE, FALSE, FALSE, FALSE, FALSE] ("Opens Resets")
            n774 = xnode "Read/Write Control"("FPGA VI Reference In"=w1915, "Opens Resets"=w1914, "Anomaly Resets"=w1914, "Cycle Resets"=w1914) -> ()  [unwired: 1 in, 2 out]
          }
        }
        n775 = property on="Save As Tab" class="TabCtl (strict)"("Visible"=w1907) -> ()  [unwired: 2 in, 2 out]
        n776 = property on="Reset Tab" class="TabCtl (strict)"("Visible"=w1907) -> ()  [unwired: 2 in, 2 out]
        n777 = property on="Set Time Tab" class="TabCtl (strict)"("Visible"=w1907) -> ()  [unwired: 2 in, 2 out]
        n778 = property on="Alarm Tab" class="TabCtl (strict)"("Visible"=w1907) -> ()  [unwired: 2 in, 2 out]
        n779 = property on="Fuel Change Tab" class="TabCtl (strict)"("Visible"=w1907) -> ()  [unwired: 2 in, 2 out]
        n780 = property on="Note Tab" class="TabCtl (strict)"("Visible"=w1907) -> ()  [unwired: 2 in, 2 out]
        n781 = property on="Main Tab" class="TabCtl (strict)"("DisabledEnum"=w1908) -> ()  [unwired: 2 in, 2 out]
        n782 = property on="pb.Stop Profile" class="Bool"("DisabledEnum"=w1908) -> ()  [unwired: 2 in, 2 out]
        n783 = property on="Monitoring Tab" class="TabCtl (strict)"("DisabledEnum"=w1908) -> ()  [unwired: 2 in, 2 out]
        n784 = property on="Title Tab" class="TabCtl (strict)"("DisabledEnum"=w1908) -> ()  [unwired: 2 in, 2 out]
        n785 = property on="CPU Usage:" class="DigNum (strict)"("DisabledEnum"=w1908) -> ()  [unwired: 2 in, 2 out]
        n786 = property on="Alarm Tab" class="TabCtl (strict)"("DisabledEnum"=w1908) -> ()  [unwired: 2 in, 2 out]
        n787 = property on="Pump Timers Tab" class="TabCtl (strict)"("DisabledEnum"=w1908) -> ()  [unwired: 2 in, 2 out]
        n788 = property on="Live Data Tab" class="TabCtl (strict)"("DisabledEnum"=w1908) -> ()  [unwired: 2 in, 2 out]
      }
      frame "Cycle Reset".."Time Reset All", "Reset LS Cycles".."Reset Opens" {
        w1923 = T14[] [enum."Enable Background", enum."Write Initial Times"] items=["Main", "Init Files", "Init", "Unused", "Save As", "Start Profile", "Check Step Time", "Alarm", "Alarm Dismiss", "Run Step", "Stop Profile", "Cycle Reset", "Time Reset", "Time Reset All", "Time Set", "Tare CTs", "Save Profile", "Open Profile", "Get Profiles", "Update Screen", "Update Controls", "Save App Config", "Write Outputs", "Disable Background", "Enable Background", "Get/Release Control", "Log Fuel Change", "Fuel Change Popup", "Read Inputs", "Remote Timer Reset", "Controller Change", "Get Alarms", "Init Alarms", "Save Alarms", "Voltage Selection", "Set Watlow Temp 1", "Set Watlow Temp 2", "Get Pressure", "Write Tare Pressure", "Adjust Controls", "Reinit ADC", "Write Initial Times", "Write Pumps Present", "HMI Command", "Save Pump Times", "Check Pump Stop Time", "Save LS App Config", "Init Data File", "Reset LS Cycles", "Reset Anomalies", "Reset Opens", "Save LS Data", "Save LS Test Data", "Check Serial Numbers", "Main Tab", "Allow Data Note", "Resume Profile", "Pause Profile", "Allow Pause Note", "Clear Graph"]
        n789 = property on="Reset Tab" class="TabCtl (strict)"("Visible"=TRUE) -> (error out=w1919:errorcluster)  [unwired: 2 in, 1 out]
        n790 = while {
          tunnel: ["pb.Reset OK"] -> w1921
          tunnel: w1919 -> [_]
          stop <- w1997 stop-if-true
          n791 = Wait (ms)(milliseconds to wait=u32 10) -> ()  [unwired: 1 out]
          n792 = Or(x="pb.Reset Cancel", y="pb.Reset OK") -> (x .or. y?=w1997:bool)
        }
        n793 = disable-structure shown="Enabled" {
          disable-tunnel: [w1937 w1967] -> w1917
          disable-tunnel: w1928 -> [w1936 w1965]
          disable-tunnel: w1927 -> [w1935 w1963]
          disable-tunnel: w1926 -> [w1934 w1966]
          disable-tunnel: w1921 -> [w1933 w1964]
          frame Disabled {
            n794 = Unbundle By Name(w1935) -> ("pb.Resets"=w1932:bool[], "Initial Times"=w1929:dbl[])
            n795 = Search 1D Array(1D array=w1932, element=TRUE) -> (index of element=w1930:i32)  [unwired: 1 in]
            n796 = case shown="True" w1933 {
              tunnel: [w1938 w1944] -> w1937
              tunnel: w1935 -> [w1938 w1943]
              tunnel: w1930 -> [_ w1942]
              tunnel: w1929 -> [_ w1941]
              tunnel: w1936 -> [_ w1940]
              tunnel: w1934 -> [_ w1939]
              frame False {
              }
              frame True {
                n797 = case shown="\"Time Reset\"" w1939 {
                  tunnel: w1943 -> [w1947 w1957 w1962]
                  tunnel: [w1946 w1956 w1961] -> w1944
                  tunnel: w1942 -> [_ w1952 _]
                  tunnel: w1941 -> [_ w1955 _]
                  tunnel: w1940 -> [_ w1950 w1960]
                  frame "Cycle Reset", Default {
                    n798 = Bundle By Name(cluster=w1947, "App Config.Cycles Completed"=u32 0) -> (w1946:T25)
                  }
                  frame "Time Reset" {
                    n799 = Replace Array Subset(array=w1955, new element=0.0 ("new element/subarray"), index=w1952) -> (w1948:dbl[])
                    n800 = Replace Array Subset(array=bool[] [FALSE, FALSE, FALSE, FALSE, FALSE, FALSE], new element=TRUE ("new element/subarray"), index=w1952) -> (w1953:bool[])
                    n801 = xnode "Read/Write Control"("FPGA VI Reference In"=w1950, "Timer Resets"=w1953) -> ()  [unwired: 1 in, 2 out]
                    n802 = Bundle By Name(cluster=w1957, "Initial Times"=w1948) -> (w1956:T25)
                  }
                  frame "Time Reset All" {
                    n803 = xnode "Read/Write Control"("FPGA VI Reference In"=w1960, "Timer Resets"=bool[] [TRUE, TRUE, TRUE, TRUE, TRUE, TRUE] ("array")) -> ()  [unwired: 1 in, 2 out]
                    n804 = Bundle By Name(cluster=w1962, "Initial Times"=dbl[] [0.0, 0.0, 0.0, 0.0, 0.0, 0.0] ("Intitial Times")) -> (w1961:T25)
                  }
                }
              }
            }
          }
          frame Enabled {
            n805 = case shown="True" w1964 {
              tunnel: [w1968 w1972] -> w1967
              tunnel: w1963 -> [w1968 w1971]
              tunnel: w1965 -> [_ w1970]
              tunnel: w1966 -> [_ w1969]
              frame False {
              }
              frame True {
                n806 = case shown="\"Reset Anomalies\"" w1969 {
                  tunnel: w1971 -> [w1976 w1984 w1991 w1995]
                  tunnel: [w1975 w1983 w1990 w1995] -> w1972
                  tunnel: w1970 -> [w1974 w1982 w1989 _]
                  frame "Reset LS Cycles" {
                    n807 = flat-sequence {
                      tunnel: w1974 -> [w1978]
                      frame #0 {
                        n808 = xnode "Read/Write Control"("FPGA VI Reference In"=w1978, "Cycle Resets"=bool[] [TRUE, TRUE, TRUE, TRUE, TRUE, TRUE, TRUE, TRUE, TRUE, TRUE, TRUE, TRUE] ("Opens Resets")) -> ()  [unwired: 1 in, 2 out]
                      }
                      frame #1 {
                        n809 = Wait (ms)(milliseconds to wait=u32 5) -> ()  [unwired: 1 out]
                      }
                    }
                    n810 = Bundle By Name(cluster=w1976, "Initial LS Data.Total Cycles"=u32[] [0, 0, 0, 0, 0, 0, 0, 0, 0, 0, 0, 0]) -> (w1975:T25)
                  }
                  frame "Reset Anomalies" {
                    w1980 = i32[] [0, 0, 0, 0, 0, 0, 0, 0, 0, 0, 0, 0] ("Initial LS Data.Anomalies (Last Cycle)")
                    w1981 = u32[] [0, 0, 0, 0, 0, 0, 0, 0, 0, 0, 0, 0] ("Initial LS Data.Steps")
                    n811 = flat-sequence {
                      tunnel: w1982 -> [w1986]
                      frame #0 {
                        n812 = xnode "Read/Write Control"("FPGA VI Reference In"=w1986, "Anomaly Resets"=bool[] [TRUE, TRUE, TRUE, TRUE, TRUE, TRUE, TRUE, TRUE, TRUE, TRUE, TRUE, TRUE] ("Opens Resets")) -> ()  [unwired: 1 in, 2 out]
                      }
                      frame #1 {
                        n813 = Wait (ms)(milliseconds to wait=u32 5) -> ()  [unwired: 1 out]
                      }
                    }
                    n814 = Bundle By Name(cluster=w1984, "Initial LS Data.Steps"=w1981, "Initial LS Data.Anomalies Total"=w1980, "Initial LS Data.Cycles"=w1981, "Initial LS Data.Anomalies/Cycle"=w1980, "Initial LS Data.Anomalies (Last Cycle)"=w1980) -> (w1983:T25)
                  }
                  frame "Reset Opens" {
                    n815 = flat-sequence {
                      tunnel: w1989 -> [w1993]
                      frame #0 {
                        n816 = xnode "Read/Write Control"("FPGA VI Reference In"=w1993, "Opens Resets"=bool[] [TRUE, TRUE, TRUE, TRUE, TRUE, TRUE, TRUE, TRUE, TRUE, TRUE, TRUE, TRUE]) -> ()  [unwired: 1 in, 2 out]
                      }
                      frame #1 {
                        n817 = Wait (ms)(milliseconds to wait=u32 5) -> ()  [unwired: 1 out]
                      }
                    }
                    n818 = Bundle By Name(cluster=w1991, "Initial LS Data.Opens"=i32[] [0, 0, 0, 0, 0, 0, 0, 0, 0, 0, 0, 0]) -> (w1990:T25)
                  }
                  frame Default {
                  }
                }
              }
            }
          }
        }
        n819 = Unbundle By Name(w1917) -> ("Initial LS Data"=w1916:T15)
        n820 = call "LS Data Global.vi"("Mode"=T28."Write Init Data", "Initial LS Data In"=w1916) -> ()  [unwired: 10 in, 4 out]
        n821 = Insert Into Array(array=w1925, index=0, new element=w1923) -> (w1924:T14[])
      }
      frame "Alarm" {
        w2009 = T14[] [] items=["Main", "Init Files", "Init", "Unused", "Save As", "Start Profile", "Check Step Time", "Alarm", "Alarm Dismiss", "Run Step", "Stop Profile", "Cycle Reset", "Time Reset", "Time Reset All", "Time Set", "Tare CTs", "Save Profile", "Open Profile", "Get Profiles", "Update Screen", "Update Controls", "Save App Config", "Write Outputs", "Disable Background", "Enable Background", "Get/Release Control", "Log Fuel Change", "Fuel Change Popup", "Read Inputs", "Remote Timer Reset", "Controller Change", "Get Alarms", "Init Alarms", "Save Alarms", "Voltage Selection", "Set Watlow Temp 1", "Set Watlow Temp 2", "Get Pressure", "Write Tare Pressure", "Adjust Controls", "Reinit ADC", "Write Initial Times", "Write Pumps Present", "HMI Command", "Save Pump Times", "Check Pump Stop Time", "Save LS App Config", "Init Data File", "Reset LS Cycles", "Reset Anomalies", "Reset Opens", "Save LS Data", "Save LS Test Data", "Check Serial Numbers", "Main Tab", "Allow Data Note", "Resume Profile", "Pause Profile", "Allow Pause Note", "Clear Graph"]
        n822 = Unbundle By Name(w2000) -> ("Alarm Message 1"=w2005:string, "Alarm Message 2"=w2012:string, "App Config.Location"=w2013:string, "App Config.Email Handler IP"=w2002:string, "Email Alarms Disabled"=w2001:bool)
        n823 = Format Into String(format string="%s\n\n%s", w2005, w2012) -> (resulting string=w2010:string)  [unwired: 2 in, 1 out]
        n824 = Concatenate Strings(w2013, " ALARM!" ("string")) -> (w2011:string)
        n825 = case shown="False" w2001 {
          tunnel: w2011 -> [w2016 _]
          tunnel: w2010 -> [w2015 _]
          tunnel: w2002 -> [w2014 _]
          frame False {
            n826 = flat-sequence {
              tunnel: w2016 -> [w2020]
              tunnel: w2015 -> [w2019]
              tunnel: w2014 -> [w2017]
              frame #0 {
                n827 = call "Email to Handler.vi"("Email Mode"=Email_Mode."Trigger Email", "Email Handler IP"=w2017, "Message:"=w2019, "Subject:"=w2020) -> ()  [unwired: 8 in]
              }
              frame #1 {
                n828 = call "Email Global.vi"("Write (F)"=TRUE, "Send Email"=TRUE) -> ()  [unwired: 9 in, 1 out]
              }
            }
          }
          frame True {
          }
        }
        n829 = flat-sequence {
          tunnel: w2010 -> [w2023]
          frame #0 {
            "Alarm Message" <- w2023
          }
          frame #1 {
            n830 = property on="Alarm Tab" class="TabCtl (strict)"("Visible"=TRUE) -> ()  [unwired: 2 in, 2 out]
          }
        }
        n831 = Insert Into Array(array=w2007, index=0, new element=w2009) -> (w2006:T14[])
      }
      frame "Alarm Dismiss" {
        w2031 = T14[] [enum."Enable Background"] items=["Main", "Init Files", "Init", "Unused", "Save As", "Start Profile", "Check Step Time", "Alarm", "Alarm Dismiss", "Run Step", "Stop Profile", "Cycle Reset", "Time Reset", "Time Reset All", "Time Set", "Tare CTs", "Save Profile", "Open Profile", "Get Profiles", "Update Screen", "Update Controls", "Save App Config", "Write Outputs", "Disable Background", "Enable Background", "Get/Release Control", "Log Fuel Change", "Fuel Change Popup", "Read Inputs", "Remote Timer Reset", "Controller Change", "Get Alarms", "Init Alarms", "Save Alarms", "Voltage Selection", "Set Watlow Temp 1", "Set Watlow Temp 2", "Get Pressure", "Write Tare Pressure", "Adjust Controls", "Reinit ADC", "Write Initial Times", "Write Pumps Present", "HMI Command", "Save Pump Times", "Check Pump Stop Time", "Save LS App Config", "Init Data File", "Reset LS Cycles", "Reset Anomalies", "Reset Opens", "Save LS Data", "Save LS Test Data", "Check Serial Numbers", "Main Tab", "Allow Data Note", "Resume Profile", "Pause Profile", "Allow Pause Note", "Clear Graph"]
        n832 = Bundle By Name(cluster=w2027, "Alarm Latch"=FALSE) -> (w2026:T25)
        n833 = Insert Into Array(array=w2029, index=0, new element=w2031) -> (w2028:T14[])
      }
      frame "Time Set" {
        w2035 = T14[] [enum."Enable Background", enum."Write Initial Times"] items=["Main", "Init Files", "Init", "Unused", "Save As", "Start Profile", "Check Step Time", "Alarm", "Alarm Dismiss", "Run Step", "Stop Profile", "Cycle Reset", "Time Reset", "Time Reset All", "Time Set", "Tare CTs", "Save Profile", "Open Profile", "Get Profiles", "Update Screen", "Update Controls", "Save App Config", "Write Outputs", "Disable Background", "Enable Background", "Get/Release Control", "Log Fuel Change", "Fuel Change Popup", "Read Inputs", "Remote Timer Reset", "Controller Change", "Get Alarms", "Init Alarms", "Save Alarms", "Voltage Selection", "Set Watlow Temp 1", "Set Watlow Temp 2", "Get Pressure", "Write Tare Pressure", "Adjust Controls", "Reinit ADC", "Write Initial Times", "Write Pumps Present", "HMI Command", "Save Pump Times", "Check Pump Stop Time", "Save LS App Config", "Init Data File", "Reset LS Cycles", "Reset Anomalies", "Reset Opens", "Save LS Data", "Save LS Test Data", "Check Serial Numbers", "Main Tab", "Allow Data Note", "Resume Profile", "Pause Profile", "Allow Pause Note", "Clear Graph"]
        n834 = disable-structure shown="Disabled" {
          disable-tunnel: [w2049 w2067] -> w2038
          disable-tunnel: w2037 -> [w2048 w2067]
          disable-tunnel: w2036 -> [w2041 _]
          frame Disabled {
            n835 = Unbundle By Name(w2048) -> ("pb.Sets"=w2047:bool[], "Initial Times"=w2042:dbl[], "Pump Data.Elapsed Time"=w2045:dbl[])
            n836 = Search 1D Array(1D array=w2047, element=TRUE) -> (index of element=w2044:i32)  [unwired: 1 in]
            n837 = Index Array(array=w2045, index=w2044) -> (element=w2043:dbl)
            n838 = local write "New Time"(w2043) -> ()
            n839 = property on="Set Time Tab" class="TabCtl (strict)"("Visible"=TRUE) -> (error out=w2039:errorcluster)  [unwired: 2 in, 1 out]
            n840 = while {
              tunnel: ["pb.Set Time OK"] -> w2050
              tunnel: w2043 -> [_]
              tunnel: w2039 -> [_]
              stop <- w2053 stop-if-true
              n841 = Wait (ms)(milliseconds to wait=u32 10) -> ()  [unwired: 1 out]
              n842 = Or(x="pb.Set Time Cancel", y="pb.Set Time OK") -> (x .or. y?=w2053:bool)
            }
            n843 = case shown="True" w2050 {
              tunnel: w2048 -> [w2055 w2061]
              tunnel: [w2055 w2060] -> w2049
              tunnel: w2044 -> [_ w2057]
              tunnel: w2042 -> [_ w2059]
              tunnel: w2041 -> [_ w2058]
              frame False {
              }
              frame True {
                n844 = xnode "Read/Write Control"("FPGA VI Reference In"=w2058) -> ("FPGA VI Reference Out"=w2064:T26, "Timer Resets"=w2065)  [unwired: 1 in, 1 out]
                n845 = Replace Array Subset(array=w2059, new element="New Time", index=w2057) -> (w2066:dbl[])
                n846 = Replace Array Subset(array=w2065, new element=TRUE ("new element/subarray"), index=w2057) -> (w2063:bool[])
                n847 = Bundle By Name(cluster=w2061, "Initial Times"=w2066) -> (w2060:T25)
                n848 = xnode "Read/Write Control"("FPGA VI Reference In"=w2064, "Timer Resets"=w2063) -> ()  [unwired: 1 in, 2 out]
              }
            }
          }
          frame Enabled {
          }
        }
        n849 = Insert Into Array(array=w2033, index=0, new element=w2035) -> (w2032:T14[])
      }
      frame "Remote Timer Reset" {
        w2071 = T14[] [enum."Write Initial Times"] items=["Main", "Init Files", "Init", "Unused", "Save As", "Start Profile", "Check Step Time", "Alarm", "Alarm Dismiss", "Run Step", "Stop Profile", "Cycle Reset", "Time Reset", "Time Reset All", "Time Set", "Tare CTs", "Save Profile", "Open Profile", "Get Profiles", "Update Screen", "Update Controls", "Save App Config", "Write Outputs", "Disable Background", "Enable Background", "Get/Release Control", "Log Fuel Change", "Fuel Change Popup", "Read Inputs", "Remote Timer Reset", "Controller Change", "Get Alarms", "Init Alarms", "Save Alarms", "Voltage Selection", "Set Watlow Temp 1", "Set Watlow Temp 2", "Get Pressure", "Write Tare Pressure", "Adjust Controls", "Reinit ADC", "Write Initial Times", "Write Pumps Present", "HMI Command", "Save Pump Times", "Check Pump Stop Time", "Save LS App Config", "Init Data File", "Reset LS Cycles", "Reset Anomalies", "Reset Opens", "Save LS Data", "Save LS Test Data", "Check Serial Numbers", "Main Tab", "Allow Data Note", "Resume Profile", "Pause Profile", "Allow Pause Note", "Clear Graph"]
        n850 = disable-structure shown="Disabled" {
          disable-tunnel: w2074 -> [w2080 _]
          frame Disabled {
            n851 = xnode "Read/Write Control"("FPGA VI Reference In"=w2080, "Timer Resets"=bool[] [TRUE, TRUE, TRUE, TRUE, TRUE, TRUE] ("pb.Resets")) -> ("FPGA VI Reference Out"=w2078:T26)  [unwired: 1 in, 1 out]
            n852 = flat-sequence {
              tunnel: w2078 -> [w2081]
              tunnel: [w2081] -> w2077
              frame #0 {
                n853 = Wait (ms)(milliseconds to wait=u32 20) -> ()  [unwired: 1 out]
              }
            }
            n854 = xnode "Read/Write Control"("FPGA VI Reference In"=w2077, "Timer Resets"=bool[] [FALSE, FALSE, FALSE, FALSE, FALSE, FALSE] ("pb.Resets")) -> ()  [unwired: 1 in, 2 out]
          }
          frame Enabled {
          }
        }
        n855 = Bundle By Name(cluster=w2073, "Initial Times"=dbl[] [0.0, 0.0, 0.0, 0.0, 0.0, 0.0] ("Intitial Times")) -> (w2075:T25)
        n856 = Insert Into Array(array=w2068, index=0, new element=w2071) -> (w2069:T14[])
      }
      frame "Get/Release Control" {
        n857 = Unbundle By Name(w2087) -> ("Login"=w2085:bool)
        n858 = case shown="False" w2085 {
          tunnel: [T31."Disabled" ("Disabled") T31."Enabled" ("Disabled")] -> w2083
          frame False {
          }
          frame True {
          }
        }
        n859 = local write "Main Tab"(T9."Main" ("Main Tab")) -> ()
        n860 = property on="Main Tab" class="TabCtl (strict)"("DisabledEnum"=w2083) -> ()  [unwired: 2 in, 2 out]
        n861 = property on="Monitoring Tab" class="TabCtl (strict)"("DisabledEnum"=w2083) -> ()  [unwired: 2 in, 2 out]
        n862 = property on="Bank 1" class="Clust (strict)"("DisabledEnum"=w2083) -> ()  [unwired: 2 in, 2 out]
        n863 = property on="Bank 2" class="Clust (strict)"("DisabledEnum"=w2083) -> ()  [unwired: 2 in, 2 out]
        n864 = property on="Pump Timers Tab" class="TabCtl (strict)"("DisabledEnum"=w2083) -> ()  [unwired: 2 in, 2 out]
        n865 = property on="Live Data Tab" class="TabCtl (strict)"("DisabledEnum"=w2083) -> ()  [unwired: 2 in, 2 out]
        n866 = disable-structure shown="Disabled" {
          disable-tunnel: w2083 -> [w2088 _]
          frame Disabled {
            n867 = property on="pb.Stop Profile" class="Bool"("DisabledEnum"=w2088) -> ()  [unwired: 2 in, 2 out]
          }
          frame Enabled {
          }
        }
      }
      frame "Log Fuel Change" {
        n868 = Get Date/Time In Seconds() -> (seconds since 1Jan1904=w2096:timestamp)
        n869 = Unbundle By Name(w2098) -> ("Fuel Log Path"=w2095:path)
        n870 = Format Date/Time String(seconds (now)=w2096) -> (date/time string=w2094:string)  [unwired: 2 in]
        n871 = Build Array(w2094) -> (w2093:string[])
        n872 = call-poly <vilib>:"Write To Spreadsheet File.vi"("delimiter (\\t)"="," ("delimiter (\\t)"), "append to file? (new file:F)"=TRUE, "1D data"=w2093, "file path (dialog if empty)"=w2095) -> ()  [unwired: 4 in, 1 out]
      }
      frame "Fuel Change Popup" {
        w2099 = T14[] [enum."Enable Background"] items=["Main", "Init Files", "Init", "Unused", "Save As", "Start Profile", "Check Step Time", "Alarm", "Alarm Dismiss", "Run Step", "Stop Profile", "Cycle Reset", "Time Reset", "Time Reset All", "Time Set", "Tare CTs", "Save Profile", "Open Profile", "Get Profiles", "Update Screen", "Update Controls", "Save App Config", "Write Outputs", "Disable Background", "Enable Background", "Get/Release Control", "Log Fuel Change", "Fuel Change Popup", "Read Inputs", "Remote Timer Reset", "Controller Change", "Get Alarms", "Init Alarms", "Save Alarms", "Voltage Selection", "Set Watlow Temp 1", "Set Watlow Temp 2", "Get Pressure", "Write Tare Pressure", "Adjust Controls", "Reinit ADC", "Write Initial Times", "Write Pumps Present", "HMI Command", "Save Pump Times", "Check Pump Stop Time", "Save LS App Config", "Init Data File", "Reset LS Cycles", "Reset Anomalies", "Reset Opens", "Save LS Data", "Save LS Test Data", "Check Serial Numbers", "Main Tab", "Allow Data Note", "Resume Profile", "Pause Profile", "Allow Pause Note", "Clear Graph"]
        n873 = while {
          stop <- "pb.Fuel Change OK" stop-if-true
          n874 = property on="Fuel Change Tab" class="TabCtl (strict)"("Visible"=TRUE) -> ()  [unwired: 2 in, 2 out]
          n875 = Wait (ms)(milliseconds to wait=u32 20) -> ()  [unwired: 1 out]
        }
        n876 = Insert Into Array(array=w2103, index=0, new element=w2099) -> (w2102:T14[])
      }
      frame "Controller Change" {
        n877 = disable-structure shown="Enabled" {
          disable-tunnel: w2113 -> [w2116 _]
          disable-tunnel: w2112 -> [w2115 w2158]
          disable-tunnel: [w2114 w2158] -> w2111
          frame Disabled {
            n878 = flat-sequence {
              tunnel: [w2121] -> w2118
              tunnel: [w2141] -> w2117
              tunnel: [w2128] -> w2114
              tunnel: w2115 -> [w2129]
              tunnel: w2116 -> [w2136]
              tunnel: w2115 -> [w2140]
              tunnel: w2118 -> [w2157]
              tunnel: w2117 -> [w2150]
              frame #0 {
                w2125 = dbl[] [0.0, 0.0, 0.0, 0.0, 0.0, 0.0] ("ControllerCurrent")
                # "Not updating properly."
                # "Need to write this here as well in case a non-CAN\ncontroller is chosen (otherwise, most recent CAN\ncode will continue to execute)."
                n879 = Unbundle By Name(w2140) -> ("Controller List"=w2122:T24, "App Config.Controller Type:"=w2119:T3)
                n880 = Index Array(array=w2122, index=w2119) -> (element=w2124:T50)
                n881 = Unbundle By Name(w2124) -> ("Frequency"=w2126:i32, "CommSeg"=w2127:i32, "Controller?"=w2141:bool, "High Command"=w2131:dbl, "Low Command"=w2132:dbl, "Command Step"=w2133:dbl, "Invert PWM"=w2123:bool)
                n882 = Equal?(x=1, y=w2127) -> (x = y?=w2121:bool)
                n883 = case shown="False" w2121 {
                  tunnel: [w2145 fxp<+,32,16> 1.0 ("CommFactor")] -> w2138
                  tunnel: w2127 -> [w2146 _]
                  frame False {
                    n884 = case shown="10, Default" w2146 {
                      tunnel: [fxp<+,32,16> 4.0 ("CommFactor") fxp<+,32,16> 5.0 ("CommFactor")] -> w2145
                      frame 8 {
                      }
                      frame 10, Default {
                      }
                    }
                  }
                  frame True {
                  }
                }
                n885 = call "CAN Global.vi"("Controller Type:"=w2119, "Write (F)"=TRUE) -> ()  [unwired: 10 in, 4 out]
                n886 = property on="ControllerCurrent" class="Arr (strict)"("Value"=w2125) -> ()  [unwired: 2 in, 2 out]
                n887 = local write "ControllerCurrent"(w2125) -> ()
                n888 = Divide(x=40000000.0 ("40 MHz"), y=w2126) -> (x/y=w2135:dbl)
                n889 = To Unsigned Long Integer(number=w2135) -> (unsigned 32bit integer=w2130:u32)
                n890 = xnode "Read/Write Control"("FPGA VI Reference In"=w2136, "Brushless"=w2121, "CommFactor"=w2138, "RPMhyst"="RPMhyst", "PWM Period (Ticks)"=w2130, "InvertPWM?"=w2123) -> ()  [unwired: 1 in, 2 out]
                n891 = disable-structure shown="Disabled" {
                  disable-tunnel: w2133 -> [w2144 _]
                  disable-tunnel: w2132 -> [w2143 _]
                  disable-tunnel: w2131 -> [w2142 _]
                  frame Disabled {
                    n892 = property on="Numeric" class="DigNum (strict)"("Maximum"=w2142, "Minimum"=w2143, "Increment"=w2144) -> ()  [unwired: 2 in, 2 out]
                  }
                  frame Enabled {
                  }
                }
                n893 = Bundle By Name(cluster=w2129, "Controller Config"=w2124) -> (w2128:T25)
              }
              frame #1 {
                n894 = Select(t="Pump\nCurrent\n(RMS)" ("Label.Text"), s=w2157, f="Pump\nCurrent\n(DC)" ("Label.Text")) -> (s? t:f=w2152:string)
                n895 = Select(t=T31."Enabled" ("Disabled"), s=w2150, f=T31."Disabled and Grayed Out" ("Disabled")) -> (s? t:f=w2153:T31)
                n896 = property on="PumpCurrent" class="Arr (strict)"("Caption.Text"=w2152) -> ()  [unwired: 2 in, 2 out]
                n897 = property on="ControllerCurrent" class="Arr (strict)"("DisabledEnum"=w2153) -> ()  [unwired: 2 in, 2 out]
              }
            }
          }
          frame Enabled {
          }
        }
        n898 = Insert Into Array(array=w2110, index=0, new element=Sequence_States."Voltage Selection" ("new element/subarray")) -> (w2109:T14[])
      }
      frame "Voltage Selection" {
        # "Delete out controller voltage\nrows to make array correct size"
        n899 = Unbundle By Name(w2168) -> ("Controller Config.Controller?"=w2160:bool, "CalArray"=w2165:dbl[][])
        n900 = Delete From Array(array=w2165, length=6, index (row)=48) -> (deleted portion=w2161:dbl[][], array with subset deleted=w2162:dbl[][])  [unwired: 1 in]
        n901 = case shown="False" w2160 {
          tunnel: w2162 -> [w2172 w2175]
          tunnel: w2161 -> [_ w2174]
          tunnel: [w2172 w2173] -> w2159
          frame False {
            # "Voltage @ Pump\nNo Change"
          }
          frame True {
            # "Switch Voltage\ncoefficients to \nthe controller"
            n902 = for {
              tunnel: w2174 -> [w2178] mode=indexing
              shift-right: [w2177] -> w2173
              shift-left: w2175 -> [w2179]
              i -> [w2176]
              n903 = Replace Array Subset(array=w2179, new element=w2178, index (row)=w2176) -> (w2177:dbl[][])  [unwired: 1 in]
            }
          }
        }
        n904 = Select(t="Controller\nVoltage\n(V)" ("Caption.Text"), s=w2160, f="Pump\nVoltage\n(V)" ("Caption.Text")) -> (s? t:f=w2171:string)
        n905 = property on="Voltages" class="Arr (strict)"("Caption.Text"=w2171) -> ()  [unwired: 2 in, 2 out]
        n906 = call "Tank Data Global.vi"("Pump Data Mode"=Pump_Data_Mode."Write Cal", "Cal Coefficients"=w2159) -> ()  [unwired: 10 in, 4 out]
      }
      frame "Set Watlow Temp 1", "Set Watlow Temp 2" {
        n907 = Unbundle By Name(w2188) -> ("Tank CMDs.Temp 1 CMD"=w2187:dbl, "Tank CMDs.Temp 2 CMD"=w2186:dbl)
        n908 = To Single Precision Float(number=w2187) -> (single precision float=w2185:sgl)
        n909 = To Single Precision Float(number=w2186) -> (single precision float=w2184:sgl)
        n910 = case shown="\"Set Watlow Temp 2\"" w2183 {
          tunnel: [Modbus_Mode."Tank 1 Write" ("Modbus Mode") Modbus_Mode."Tank 2 Write" ("Modbus Mode")] -> w2182
          tunnel: [Modbus_Variable."Setpoint" ("Variable") Modbus_Variable."Setpoint" ("Variable")] -> w2181
          tunnel: [w2190 w2193] -> w2180
          tunnel: w2185 -> [w2190 _]
          tunnel: w2184 -> [_ w2193]
          frame "Set Watlow Temp 1", Default {
          }
          frame "Set Watlow Temp 2" {
          }
        }
        n911 = call "Watlow Modbus.vi"("Modbus Mode"=w2182, "Data Write"=w2180, "Variable"=w2181) -> ()  [unwired: 7 in, 2 out]
      }
      frame "Get Pressure" {
        w2212 = T14[] [enum."Write Tare Pressure"] items=["Main", "Init Files", "Init", "Unused", "Save As", "Start Profile", "Check Step Time", "Alarm", "Alarm Dismiss", "Run Step", "Stop Profile", "Cycle Reset", "Time Reset", "Time Reset All", "Time Set", "Tare CTs", "Save Profile", "Open Profile", "Get Profiles", "Update Screen", "Update Controls", "Save App Config", "Write Outputs", "Disable Background", "Enable Background", "Get/Release Control", "Log Fuel Change", "Fuel Change Popup", "Read Inputs", "Remote Timer Reset", "Controller Change", "Get Alarms", "Init Alarms", "Save Alarms", "Voltage Selection", "Set Watlow Temp 1", "Set Watlow Temp 2", "Get Pressure", "Write Tare Pressure", "Adjust Controls", "Reinit ADC", "Write Initial Times", "Write Pumps Present", "HMI Command", "Save Pump Times", "Check Pump Stop Time", "Save LS App Config", "Init Data File", "Reset LS Cycles", "Reset Anomalies", "Reset Opens", "Save LS Data", "Save LS Test Data", "Check Serial Numbers", "Main Tab", "Allow Data Note", "Resume Profile", "Pause Profile", "Allow Pause Note", "Clear Graph"]
        n912 = flat-sequence {
          tunnel: [w2216] -> w2204
          frame #0 {
            n913 = call "Tank Data Global.vi"("Pump Data Mode"=Pump_Data_Mode."Write Pressure Offsets", "Pressure Offsets"=dbl[] [0.0, 0.0, 0.0, 0.0, 0.0, 0.0]) -> ()  [unwired: 10 in, 4 out]
          }
          frame #1 {
            # "Wait for write to occur."
            n914 = Wait (ms)(milliseconds to wait=u32 500) -> ()  [unwired: 1 out]
          }
          frame #2 {
            n915 = call "Tank Data Global.vi"("Pump Data Mode"=Pump_Data_Mode."Read") -> ("Tank Data OUT"=w2216:dbl[])  [unwired: 11 in, 3 out]
          }
        }
        n916 = Array Subset(array=w2204, index=30, length=6) -> (w2196:dbl[])
        n917 = Bundle By Name(cluster=w2205, "Pressure Offsets"=w2196) -> (w2206:T25)
        n918 = To Double Precision Float(number=w2196) -> (double precision float=w2201:dbl[])
        n919 = Array To Spreadsheet String(delimiter (Tab)=",", array=w2201, 3:"%.2f" ("format string")) -> (spreadsheet string=w2199:string)
        n920 = Write to Text File(file (use dialog)=path "c:/PressureOffsets", text=w2199) -> (refnum out=w2198:refnum<file>, error out=w2197:errorcluster)  [unwired: 2 in, 1 out]
        n921 = Close File(refnum=w2198, error in=w2197) -> ()  [unwired: 2 out]
        n922 = Insert Into Array(array=w2210, index=0, new element=w2212) -> (w2209:T14[])
      }
      frame "Write Tare Pressure" {
        n923 = Unbundle By Name(w2220) -> ("Pressure Offsets"=w2218:dbl[])
        n924 = call "Tank Data Global.vi"("Pump Data Mode"=Pump_Data_Mode."Write Pressure Offsets", "Pressure Offsets"=w2218) -> ()  [unwired: 10 in, 4 out]
      }
      frame "Adjust Controls" {
        n925 = Unbundle By Name(w2229) -> ("App Config.Voltage Limits"=w2223:T42, "App Config.Voltage Far PI"=w2224:T43, "App Config.Voltage Mid PI"=w2225:T44, "App Config.Voltage Close PI"=w2226:T45, "App Config.Voltage Scale"=w2227:cluster{"V_FFm":dbl, "V_FFb":dbl}, "App Config.Voltage Cutoffs"=w2222:cluster{"V_MidCutoff":dbl, "V_CloseCutoff":dbl})
        n926 = call "PI with FF.vi"("Cutoffs"=w2222, "FFcluster"=w2227, "ClosePIcluster"=w2226, "MidPIcluster"=w2225, "FarPIcluster"=w2224, "LimitCluster"=w2223, "Init (F)"=TRUE) -> ()  [unwired: 8 in, 1 out]
      }
      frame "Reinit ADC" {
        n927 = call "Init FPGA.vi"("FPGA Ref"=w2233) -> ("error out"=w2231:errorcluster, "FPGA Ref Out"=w2232:T26)  [unwired: 9 in]
        n928 = feedback #7(0) -> (w2234:i32)
        "ADC Errors" <- w2234
        n929 = Increment(x=w2234) -> (x+1=w2235:i32)
        n930 = feedback-in #7(w2235) -> ()
        n931 = disable-structure shown="Disabled" {
          disable-tunnel: w2232 -> [w2240 _]
          disable-tunnel: w2231 -> [w2239 _]
          frame Disabled {
            n932 = call "Init ADCs.vi"("Error IN"=w2239, "FPGA Ref"=w2240) -> ()  [unwired: 7 in, 3 out]
          }
          frame Enabled {
          }
        }
      }
      frame "Write Initial Times" {
        w2244 = T14[] [enum."Read Inputs", enum."Save Pump Times"] items=["Main", "Init Files", "Init", "Unused", "Save As", "Start Profile", "Check Step Time", "Alarm", "Alarm Dismiss", "Run Step", "Stop Profile", "Cycle Reset", "Time Reset", "Time Reset All", "Time Set", "Tare CTs", "Save Profile", "Open Profile", "Get Profiles", "Update Screen", "Update Controls", "Save App Config", "Write Outputs", "Disable Background", "Enable Background", "Get/Release Control", "Log Fuel Change", "Fuel Change Popup", "Read Inputs", "Remote Timer Reset", "Controller Change", "Get Alarms", "Init Alarms", "Save Alarms", "Voltage Selection", "Set Watlow Temp 1", "Set Watlow Temp 2", "Get Pressure", "Write Tare Pressure", "Adjust Controls", "Reinit ADC", "Write Initial Times", "Write Pumps Present", "HMI Command", "Save Pump Times", "Check Pump Stop Time", "Save LS App Config", "Init Data File", "Reset LS Cycles", "Reset Anomalies", "Reset Opens", "Save LS Data", "Save LS Test Data", "Check Serial Numbers", "Main Tab", "Allow Data Note", "Resume Profile", "Pause Profile", "Allow Pause Note", "Clear Graph"]
        n933 = Unbundle By Name(w2246) -> ("Initial Times"=w2245:dbl[])
        n934 = call "Tank Data Global.vi"("Pump Data Mode"=Pump_Data_Mode."Write Initial Times", "Intitial Times"=w2245) -> ()  [unwired: 10 in, 4 out]
        n935 = Insert Into Array(array=w2242, index=0, new element=w2244) -> (w2241:T14[])
      }
      frame "Write Pumps Present" {
        w2263 = T14[] [enum."Write Outputs", enum."Update Controls"] items=["Main", "Init Files", "Init", "Unused", "Save As", "Start Profile", "Check Step Time", "Alarm", "Alarm Dismiss", "Run Step", "Stop Profile", "Cycle Reset", "Time Reset", "Time Reset All", "Time Set", "Tare CTs", "Save Profile", "Open Profile", "Get Profiles", "Update Screen", "Update Controls", "Save App Config", "Write Outputs", "Disable Background", "Enable Background", "Get/Release Control", "Log Fuel Change", "Fuel Change Popup", "Read Inputs", "Remote Timer Reset", "Controller Change", "Get Alarms", "Init Alarms", "Save Alarms", "Voltage Selection", "Set Watlow Temp 1", "Set Watlow Temp 2", "Get Pressure", "Write Tare Pressure", "Adjust Controls", "Reinit ADC", "Write Initial Times", "Write Pumps Present", "HMI Command", "Save Pump Times", "Check Pump Stop Time", "Save LS App Config", "Init Data File", "Reset LS Cycles", "Reset Anomalies", "Reset Opens", "Save LS Data", "Save LS Test Data", "Check Serial Numbers", "Main Tab", "Allow Data Note", "Resume Profile", "Pause Profile", "Allow Pause Note", "Clear Graph"]
        # "Power and Ignition relays can only turn of if pumps are present."
        n936 = Unbundle By Name(w2252) -> ("App Config.Pumps Present"=w2255:T8, "Power Relay"=w2259:T8, "Ignition Relay"=w2258:T8)
        n937 = Cluster To Array(cluster=w2255) -> (array=w2248:bool[])
        n938 = Cluster To Array(cluster=w2259) -> (array=w2257:bool[])
        n939 = Cluster To Array(cluster=w2258) -> (array=w2256:bool[])
        n940 = call "Tank Data Global.vi"("Pump Data Mode"=Pump_Data_Mode."Write Pumps Present", "Pumps Present"=w2248) -> ()  [unwired: 10 in, 4 out]
        n941 = And(x=w2257, y=w2248) -> (x .and. y?=w2254:bool[])
        n942 = And(x=w2256, y=w2248) -> (x .and. y?=w2253:bool[])
        n943 = Array To Cluster(array=w2254) -> (cluster=w2250:T51)
        n944 = Array To Cluster(array=w2253) -> (cluster=w2249:T51)
        n945 = Bundle By Name(cluster=w2252, "Power Relay"=w2250, "Ignition Relay"=w2249) -> (w2251:T25)
        n946 = Insert Into Array(array=w2261, index=0, new element=w2263) -> (w2260:T14[])
      }
      frame "HMI Command" {
        w2266 = T14[] [] items=["Main", "Init Files", "Init", "Unused", "Save As", "Start Profile", "Check Step Time", "Alarm", "Alarm Dismiss", "Run Step", "Stop Profile", "Cycle Reset", "Time Reset", "Time Reset All", "Time Set", "Tare CTs", "Save Profile", "Open Profile", "Get Profiles", "Update Screen", "Update Controls", "Save App Config", "Write Outputs", "Disable Background", "Enable Background", "Get/Release Control", "Log Fuel Change", "Fuel Change Popup", "Read Inputs", "Remote Timer Reset", "Controller Change", "Get Alarms", "Init Alarms", "Save Alarms", "Voltage Selection", "Set Watlow Temp 1", "Set Watlow Temp 2", "Get Pressure", "Write Tare Pressure", "Adjust Controls", "Reinit ADC", "Write Initial Times", "Write Pumps Present", "HMI Command", "Save Pump Times", "Check Pump Stop Time", "Save LS App Config", "Init Data File", "Reset LS Cycles", "Reset Anomalies", "Reset Opens", "Save LS Data", "Save LS Test Data", "Check Serial Numbers", "Main Tab", "Allow Data Note", "Resume Profile", "Pause Profile", "Allow Pause Note", "Clear Graph"]
        n947 = flat-sequence {
          tunnel: [w2280] -> w2267
          frame #0 {
            n948 = call "RPi HMI Global.vi"("Mode"=HMI_Global_Mode."Reset Cmd") -> ()  [unwired: 10 in, 1 out]
          }
          frame #1 {
            n949 = call "RPi HMI Global.vi"("Mode"=HMI_Global_Mode."Read") -> ("HMI Cluster OUT"=w2280:T16)  [unwired: 10 in]
          }
        }
        n950 = Unbundle By Name(w2267) -> ("Power Relays"=w2276:T8, "Pump CMDs"=w2275:dbl[], "Tank CMDs.PS CMD"=w2274:dbl, "Tank CMDs.Press CMD"=w2273:dbl, "Tank CMDs.Temp 1 CMD"=w2272:dbl, "Tank CMDs.Temp 2 CMD"=w2271:dbl, "HMI Tog Buttons.Start Test"=w2270:bool)
        n951 = local write "Power Relay"(w2276) -> ()
        n952 = local write "Controller\nCMD"(w2275) -> ()
        n953 = local write "Power Supply Cmd:"(w2274) -> ()
        n954 = local write "PressureCMD"(w2273) -> ()
        n955 = local write "Tank 1 Temp Cmd:"(w2272) -> ()
        n956 = local write "Tank 2 Temp Cmd:"(w2271) -> ()
        n957 = local write "pb.Run Profile"(w2270) -> ()
        n958 = Insert Into Array(array=w2277, index=0, new element=w2266) -> (w2265:T14[])
        n959 = Bundle By Name(cluster=w2269, "HMI"=w2267) -> (w2268:T25)
      }
      frame "Init Data File" {
        n960 = Get Date/Time In Seconds() -> (seconds since 1Jan1904=w2283:timestamp)
        n961 = Unbundle By Name(w2297) -> ("App Config.CA Number"=w2292:string, "LS App Config.Data File Name:"=w2293:string, "LS App Config.Serial Numbers"=w2288:string[])
        n962 = Format Date/Time String(time format string (%c)="_%m%d%y.csv", seconds (now)=w2283) -> (date/time string=w2282:string)  [unwired: 1 in]
        n963 = Empty String/Path?(string/path=w2293) -> (empty?=w2291:bool)
        n964 = Empty String/Path?(string/path=w2292) -> (empty?=w2290:bool)
        n965 = call "Remove illegal file characters.vi"("Filename In"=w2292) -> ("Filename Out"=w2286:string)  [unwired: 10 in]
        n966 = call "Remove illegal file characters.vi"("Filename In"=w2293) -> ("Filename Out"=w2285:string)  [unwired: 10 in]
        n967 = Or(x=w2291, y=w2290) -> (x .or. y?=w2287:bool)
        n968 = Build Path(base path=path "u:/CA Numbers", name or relative path=w2286) -> (appended path=w2294:path)
        n969 = case shown="False" w2287 {
          tunnel: w2294 -> [_ w2304]
          tunnel: w2282 -> [_ w2303]
          tunnel: w2285 -> [_ w2302]
          tunnel: [path "" ("LS Data Filepath") w2301] -> w2289
          tunnel: w2288 -> [_ w2300]
          frame True {
          }
          frame False {
            n970 = disable-structure shown="Enabled" {
              disable-tunnel: w2304 -> [w2317 w2361]
              disable-tunnel: w2303 -> [_ w2356]
              disable-tunnel: w2302 -> [w2305 w2354]
              disable-tunnel: [w2308 w2349] -> w2301
              disable-tunnel: w2300 -> [w2306 w2347]
              frame Enabled {
                n971 = call <vilib>:"Check if File or Folder Exists.vi"("path"=w2317) -> ("error out"=w2314:errorcluster, "file or folder exists?"=w2315:bool, "dup path"=w2316:path)  [unwired: 8 in]
                n972 = case shown="False" w2315 {
                  tunnel: w2316 -> [w2344 w2345]
                  tunnel: w2314 -> [w2341 w2346]
                  tunnel: [w2342 w2346] -> _
                  tunnel: [w2343 w2345] -> w2313
                  frame False {
                    n973 = Create Folder(path (use dialog)=w2344, error in=w2341) -> (created path=w2343:path, error out=w2342:errorcluster)  [unwired: 1 in, 1 out]
                  }
                  frame True {
                  }
                }
                n974 = Build Path(base path=w2313, name or relative path=w2305) -> (appended path=w2312:path)
                n975 = call <vilib>:"Check if File or Folder Exists.vi"("path"=w2312) -> ("error out"=w2309:errorcluster, "file or folder exists?"=w2310:bool, "dup path"=w2311:path)  [unwired: 8 in]
                n976 = disable-structure shown="Enabled" {
                  disable-tunnel: w2311 -> [w2323 w2340]
                  disable-tunnel: w2310 -> [w2322 _]
                  disable-tunnel: w2309 -> [w2321 _]
                  disable-tunnel: [w2320 w2340] -> w2308
                  disable-tunnel: "Timestamp,Pos 1 Voltage,Pos 2 Voltage,Pos 3 Voltage,Pos 4 Voltage,Pos 5 Voltage,Pos 6 Voltage,Pos 7 Voltage,Pos 8 Voltage,Pos 9 Voltage,Pos 10 Voltage,Pos 11 Voltage,Pos 12 Voltage,PS Voltage,Bank 1 State,Bank 2 State\n" -> [w2319 _]
                  disable-tunnel: w2306 -> [w2318 _]
                  frame Disabled {
                    n977 = case shown="False" w2322 {
                      tunnel: w2323 -> [w2338 w2339]
                      tunnel: w2321 -> [w2337 _]
                      tunnel: [w2335 w2339] -> w2320
                      tunnel: w2319 -> [w2329 _]
                      tunnel: w2318 -> [w2325 _]
                      frame False {
                        n978 = Array To Spreadsheet String(delimiter (Tab)=",", array=w2325, 3:"%s" ("format string")) -> (spreadsheet string=w2324:string)
                        n979 = Open/Create/Replace File(file path (use dialog)=w2338, error in=w2337, operation (0:open)=T32."create") -> (refnum out=w2332:refnum<file>, error out=w2334:errorcluster)  [unwired: 3 in, 1 out]
                        n980 = Concatenate Strings("Serial Numbers," ("string"), w2324, w2329) -> (w2328:string)
                        n981 = Write to Text File(file (use dialog)=w2332, text=w2328, error in=w2334) -> (refnum out=w2331:refnum<file>, error out=w2333:errorcluster)  [unwired: 1 in, 1 out]
                        n982 = Close File(refnum=w2331, error in=w2333) -> (path=w2335:path)  [unwired: 1 out]
                      }
                      frame True {
                      }
                    }
                  }
                  frame Enabled {
                  }
                }
              }
              frame Disabled {
                n983 = call <vilib>:"Check if File or Folder Exists.vi"("path"=w2361) -> ("error out"=w2358:errorcluster, "file or folder exists?"=w2359:bool, "dup path"=w2360:path)  [unwired: 8 in]
                n984 = Concatenate Strings(w2354, w2356) -> (w2355:string)
                n985 = case shown="False" w2359 {
                  tunnel: w2360 -> [w2381 w2382]
                  tunnel: w2358 -> [w2378 w2383]
                  tunnel: [w2379 w2383] -> _
                  tunnel: [w2380 w2382] -> w2357
                  frame False {
                    n986 = Create Folder(path (use dialog)=w2381, error in=w2378) -> (created path=w2380:path, error out=w2379:errorcluster)  [unwired: 1 in, 1 out]
                  }
                  frame True {
                  }
                }
                n987 = Build Path(base path=w2357, name or relative path=w2355) -> (appended path=w2353:path)
                n988 = call <vilib>:"Check if File or Folder Exists.vi"("path"=w2353) -> ("error out"=w2350:errorcluster, "file or folder exists?"=w2351:bool, "dup path"=w2352:path)  [unwired: 8 in]
                n989 = case shown="False" w2351 {
                  tunnel: w2352 -> [w2376 w2377]
                  tunnel: w2350 -> [w2375 _]
                  tunnel: [w2373 w2377] -> w2349
                  tunnel: "Timestamp,Pos 1 Voltage,Pos 2 Voltage,Pos 3 Voltage,Pos 4 Voltage,Pos 5 Voltage,Pos 6 Voltage,Pos 7 Voltage,Pos 8 Voltage,Pos 9 Voltage,Pos 10 Voltage,Pos 11 Voltage,Pos 12 Voltage,PS Voltage,Bank 1 State,Bank 2 State\n" -> [w2367 _]
                  tunnel: w2347 -> [w2363 _]
                  frame False {
                    n990 = Array To Spreadsheet String(delimiter (Tab)=",", array=w2363, 3:"%s" ("format string")) -> (spreadsheet string=w2362:string)
                    n991 = Open/Create/Replace File(file path (use dialog)=w2376, error in=w2375, operation (0:open)=T32."create") -> (refnum out=w2370:refnum<file>, error out=w2372:errorcluster)  [unwired: 3 in, 1 out]
                    n992 = Concatenate Strings("Serial Numbers," ("string"), w2362, w2367) -> (w2366:string)
                    n993 = Write to Text File(file (use dialog)=w2370, text=w2366, error in=w2372) -> (refnum out=w2369:refnum<file>, error out=w2371:errorcluster)  [unwired: 1 in, 1 out]
                    n994 = Close File(refnum=w2369, error in=w2371) -> (path=w2373:path)  [unwired: 1 out]
                  }
                  frame True {
                  }
                }
              }
            }
          }
        }
        n995 = local write "CA Number:"(w2286) -> ()
        n996 = local write "Data File Name:"(w2285) -> ()
        n997 = Bundle By Name(cluster=w2297, "App Config.CA Number"=w2286, "LS App Config.Data File Name:"=w2285, "LS Data Filepath"=w2289) -> (w2296:T25)
      }
      frame "Save LS Data" {
        n998 = Unbundle By Name(w2387) -> ("LS App Config.DetectionMode"=w2384:i32, "LS Data"=w2385:T15)
        n999 = case shown="0, Default" w2384 {
          tunnel: w2385 -> [w2388 w2397]
          frame 0, Default {
            # "Anomalies"
            n1000 = Unbundle By Name(w2388) -> ("Anomalies Total"=w2389:i32[])
            n1001 = Array Size(array=w2389) -> (size(s)=w2390:i32)
            n1002 = case shown="12" w2390 {
              tunnel: w2388 -> [_ w2393]
              frame Default {
              }
              frame 12 {
                n1003 = Write to Binary File(file (use dialog)=path "c:/Monitored Statistics" ("Path"), data=w2393) -> (refnum out=w2392:refnum<file>, error out=w2391:errorcluster)  [unwired: 4 in, 1 out]
                n1004 = Close File(refnum=w2392, error in=w2391) -> ()  [unwired: 2 out]
              }
            }
          }
          frame 1 {
            # "Opens"
            n1005 = Unbundle By Name(w2397) -> ("Opens"=w2396:i32[])
            n1006 = Array Size(array=w2396) -> (size(s)=w2395:i32)
            n1007 = case shown="12" w2395 {
              tunnel: w2397 -> [_ w2400]
              frame Default {
              }
              frame 12 {
                n1008 = Write to Binary File(file (use dialog)=path "c:/Monitored Statistics" ("Path"), data=w2400) -> (refnum out=w2399:refnum<file>, error out=w2398:errorcluster)  [unwired: 4 in, 1 out]
                n1009 = Close File(refnum=w2399, error in=w2398) -> ()  [unwired: 2 out]
              }
            }
          }
        }
      }
      frame "Save LS Test Data" {
        n1010 = disable-structure shown="Enabled" {
          disable-tunnel: w2403 -> [w2412 _]
          frame Disabled {
            n1011 = Unbundle By Name(w2412) -> ("LS App Config.Serial Numbers"=w2409:string[], "LS Data"=w2410:T15, "App Config.CA Number"=w2405:string, "LS App Config.Data File Name:"=w2406:string, "LS App Config.DetectionMode"=w2411:i32)
            n1012 = Empty String/Path?(string/path=w2405) -> (empty?=w2408:bool)
            n1013 = Empty String/Path?(string/path=w2406) -> (empty?=w2407:bool)
            n1014 = Or(x=w2408, y=w2407) -> (x .or. y?=w2404:bool)
            n1015 = case shown="False" w2404 {
              tunnel: w2405 -> [_ w2421]
              tunnel: w2406 -> [_ w2420]
              tunnel: w2411 -> [_ w2416]
              tunnel: w2410 -> [_ w2414]
              tunnel: w2409 -> [_ w2413]
              frame True {
              }
              frame False {
                n1016 = Build Path(base path=path "u:/CA Numbers", name or relative path=w2421) -> (appended path=w2418:path)
                n1017 = List Folder(path=w2418) -> (filenames=w2419:string[])  [unwired: 3 in, 3 out]
                n1018 = while {
                  tunnel: w2420 -> [w2464]
                  tunnel: [w2462] -> w2417
                  shift-right: [w2461] -> _
                  shift-left: w2419 -> [w2461]
                  i -> [w2466]
                  stop <- w2459 stop-if-true
                  n1019 = Increment(x=w2466) -> (x+1=w2463:i32)
                  n1020 = Format Into String(format string="%s_Statistics%#f.csv", w2464, w2463) -> (resulting string=w2462:string)  [unwired: 2 in, 1 out]
                  n1021 = Search 1D Array(1D array=w2461, element=w2462) -> (index of element=w2460:i32)  [unwired: 1 in]
                  n1022 = Less Than 0?(x=w2460) -> (x < 0?=w2459:bool)
                }
                n1023 = Build Path(base path=w2418, name or relative path=w2417) -> (appended path=w2415:path)
                n1024 = case shown="1" w2416 {
                  tunnel: w2415 -> [_ w2424]
                  tunnel: w2414 -> [_ w2457]
                  tunnel: w2413 -> [_ w2456]
                  frame 0, Default {
                    # "Anomalies"
                  }
                  frame 1 {
                    # "Opens"
                    n1025 = Unbundle By Name(w2457) -> ("Opens"=w2455:i32[])
                    n1026 = Index Array(array=w2455) -> (element #1=w2442:i32, element #2=w2440:i32, element #3=w2439:i32, element #4=w2438:i32, element #5=w2437:i32, element #6=w2436:i32, element #7=w2435:i32, element #8=w2434:i32, element #9=w2433:i32, element #10=w2432:i32, element #11=w2431:i32, element #12=w2441:i32)  [unwired: 12 in]
                    n1027 = Index Array(array=w2456) -> (element #1=w2454:string, element #2=w2453:string, element #3=w2452:string, element #4=w2451:string, element #5=w2449:string, element #6=w2450:string, element #7=w2448:string, element #8=w2447:string, element #9=w2445:string, element #10=w2446:string, element #11=w2444:string, element #12=w2443:string)  [unwired: 12 in]
                    n1028 = Format Into String(format string=",Position 1,Position 2,Position 3,Position 4,Position 5,Position 6,Position 7,Position 8,Position 9,Position 10,Position 11,Position 12\nSerial Numbers,%s,%s,%s,%s,%s,%s,%s,%s,%s,%s,%s,%s\nOpens Detected,%f,%f,%f,%f,%f,%f,%f,%f,%f,%f,%f,%f", w2454, w2453, w2452, w2451, w2449, w2450, w2448, w2447, w2445, w2446, w2444, w2443, w2442, w2440, w2439, w2438, w2437, w2436, w2435, w2434, w2433, w2432, w2431, w2441) -> (resulting string=w2426:string, error out=w2425:errorcluster)  [unwired: 2 in]
                    n1029 = Open/Create/Replace File(file path (use dialog)=w2424, error in=w2425, operation (0:open)=T32."open or create") -> (refnum out=w2430:refnum<file>, error out=w2428:errorcluster)  [unwired: 3 in, 1 out]
                    n1030 = Write to Text File(file (use dialog)=w2430, text=w2426, error in=w2428) -> (refnum out=w2429:refnum<file>, error out=w2427:errorcluster)  [unwired: 1 in, 1 out]
                    n1031 = Close File(refnum=w2429, error in=w2427) -> ()  [unwired: 2 out]
                  }
                }
              }
            }
          }
          frame Enabled {
          }
        }
      }
      frame "Check Serial Numbers" {
        n1032 = Unbundle By Name(w2472) -> ("LS App Config.Serial Numbers"=w2468:string[])
        n1033 = for {
          tunnel: w2468 -> [w2474] mode=indexing
          tunnel: [w2473] -> w2467 mode=indexing
          n1034 = call "Remove illegal file characters.vi"("Filename In"=w2474) -> ("Filename Out"=w2473:string)  [unwired: 10 in]
        }
        n1035 = Array To Cluster(array=w2467) -> (cluster=w2469:T52)
        n1036 = Bundle By Name(cluster=w2472, "LS App Config.Serial Numbers"=w2467) -> (w2471:T25)
        n1037 = local write "LS Serial Numbers"(w2469) -> ()
      }
      frame "Main Tab" {
        # "Justin wants Start Test, Stop Test, and Data File Name always unlocked\n\nSo moved Data File Name to where it wouldn't sit on top of another\ncontrol on another page when I made it float like the stop button"
        n1038 = Unbundle By Name(w2478) -> ("Main Tab"=w2477:T9)
        n1039 = case shown="\"Main\"" w2477 {
          tunnel: [T31."Enabled" ("Disabled") T31."Disabled" ("Disabled")] -> w2476
          tunnel: [TRUE ("Visible") FALSE ("Visible")] -> w2475
          frame "Main" {
          }
          frame Default {
          }
        }
        n1040 = property on="pb.Run Profile" class="Bool (strict)"("Visible"=w2475, "DisabledEnum"=w2476) -> ()  [unwired: 2 in, 2 out]
        n1041 = property on="Data File Name:" class="Str"("Visible"=w2475, "DisabledEnum"=w2476) -> ()  [unwired: 2 in, 2 out]
      }
      frame "Allow Data Note" {
        w2485 = T14[] [enum."Enable Background"] items=["Main", "Init Files", "Init", "Unused", "Save As", "Start Profile", "Check Step Time", "Alarm", "Alarm Dismiss", "Run Step", "Stop Profile", "Cycle Reset", "Time Reset", "Time Reset All", "Time Set", "Tare CTs", "Save Profile", "Open Profile", "Get Profiles", "Update Screen", "Update Controls", "Save App Config", "Write Outputs", "Disable Background", "Enable Background", "Get/Release Control", "Log Fuel Change", "Fuel Change Popup", "Read Inputs", "Remote Timer Reset", "Controller Change", "Get Alarms", "Init Alarms", "Save Alarms", "Voltage Selection", "Set Watlow Temp 1", "Set Watlow Temp 2", "Get Pressure", "Write Tare Pressure", "Adjust Controls", "Reinit ADC", "Write Initial Times", "Write Pumps Present", "HMI Command", "Save Pump Times", "Check Pump Stop Time", "Save LS App Config", "Init Data File", "Reset LS Cycles", "Reset Anomalies", "Reset Opens", "Save LS Data", "Save LS Test Data", "Check Serial Numbers", "Main Tab", "Allow Data Note", "Resume Profile", "Pause Profile", "Allow Pause Note", "Clear Graph"]
        n1042 = disable-structure shown="Enabled" {
          disable-tunnel: w2484 -> [w2489 _]
          frame Disabled {
            n1043 = flat-sequence {
              tunnel: [w2500] -> w2493
              tunnel: [w2499] -> w2492
              tunnel: w2489 -> [w2498]
              tunnel: [w2497] -> w2491
              tunnel: w2493 -> [w2512]
              tunnel: w2492 -> [w2513]
              tunnel: w2491 -> [w2511]
              tunnel: [w2508] -> w2490
              tunnel: w2490 -> [w2529]
              frame #0 {
                w2494 = FALSE ("Visible")
                n1044 = property on="Note Tab" class="TabCtl (strict)"("Visible"=TRUE) -> ()  [unwired: 2 in, 2 out]
                n1045 = property on="Normal Steps:" class="DigNum (strict)"("Visible"=w2494) -> ()  [unwired: 2 in, 2 out]
                n1046 = property on="Step Threshold:" class="DigNum (strict)"("Visible"=w2494) -> ()  [unwired: 2 in, 2 out]
                n1047 = property on="Cycle Pts to Avg:" class="DigNum (strict)"("Visible"=w2494) -> ()  [unwired: 2 in, 2 out]
                n1048 = property on="Cycle Threshold:" class="DigNum (strict)"("Visible"=w2494) -> ()  [unwired: 2 in, 2 out]
                n1049 = property on="pb.Stop Profile" class="Bool"("Visible"=w2494) -> ()  [unwired: 2 in, 2 out]
                n1050 = property on="Data File Name:" class="Str"("Visible"=w2494) -> ()  [unwired: 2 in, 2 out]
                n1051 = property on="pb.Run Profile" class="Bool (strict)"("Visible"=w2494) -> ()  [unwired: 2 in, 2 out]
                n1052 = property on="Anomaly Threshold:" class="DigNum (strict)"("Visible"=w2494) -> ()  [unwired: 2 in, 2 out]
                n1053 = property on="Main Tab" class="TabCtl (strict)"("DisabledEnum"=T31."Enabled" ("Disabled")) -> ()  [unwired: 2 in, 2 out]
              }
              frame #1 {
                n1054 = while {
                  tunnel: ["pb.Note OK"] -> w2502
                  stop <- w2506 stop-if-true
                  n1055 = Wait (ms)(milliseconds to wait=u32 10) -> ()  [unwired: 1 out]
                  n1056 = local write "Main Tab"(T9."Configure" ("Main Tab")) -> ()
                  n1057 = Or(x="pb.Note Cancel", y="pb.Note OK") -> (x .or. y?=w2506:bool)
                }
                n1058 = Unbundle By Name(w2498) -> ("Login"=w2497:bool, "LS Data Filepath"=w2499:path, "LS App Config.Record Bursts"=w2501:bool)
                n1059 = And(x=w2501, y=w2502) -> (x .and. y?=w2500:bool)
              }
              frame #2 {
                n1060 = case shown="True" w2512 {
                  tunnel: w2513 -> [_ w2515]
                  frame False {
                  }
                  frame True {
                    n1061 = Open/Create/Replace File(file path (use dialog)=w2515, operation (0:open)=T32."open or create") -> (refnum out=w2523:refnum<file>, error out=w2524:errorcluster)  [unwired: 4 in, 1 out]
                    n1062 = Concatenate Strings("Note:,", "Stop Profile Note", "\n") -> (w2516:string)
                    n1063 = Set File Position(refnum=w2523, from (0:start)=enum16{"start", "end", "current"}."end", error in=w2524) -> (refnum out=w2527:refnum<file>, error out=w2526:errorcluster)  [unwired: 1 in]
                    n1064 = Write to Text File(file (use dialog)=w2527, text=w2516, error in=w2526) -> (refnum out=w2520:refnum<file>, error out=w2519:errorcluster)  [unwired: 1 in, 1 out]
                    n1065 = Close File(refnum=w2520, error in=w2519) -> (error out=w2521:errorcluster)  [unwired: 1 out]
                    n1066 = call <vilib>:"Clear Errors.vi"("error in (no error)"=w2521) -> ()  [unwired: 5 in, 2 out]
                  }
                }
                n1067 = Select(t=T31."Enabled" ("Disabled"), s=w2511, f=T31."Disabled" ("Disabled")) -> (s? t:f=w2508:T31)
              }
              frame #3 {
                w2528 = TRUE ("Visible")
                n1068 = local write "Stop Profile Note"("" ("Stop Profile Note")) -> ()
                n1069 = local write "Main Tab"(T9."Main" ("Main Tab")) -> ()
                n1070 = property on="Main Tab" class="TabCtl (strict)"("DisabledEnum"=w2529) -> ()  [unwired: 2 in, 2 out]
                n1071 = property on="Note Tab" class="TabCtl (strict)"("Visible"=FALSE) -> ()  [unwired: 2 in, 2 out]
                n1072 = property on="Normal Steps:" class="DigNum (strict)"("Visible"=w2528) -> ()  [unwired: 2 in, 2 out]
                n1073 = property on="Step Threshold:" class="DigNum (strict)"("Visible"=w2528) -> ()  [unwired: 2 in, 2 out]
                n1074 = property on="Cycle Pts to Avg:" class="DigNum (strict)"("Visible"=w2528) -> ()  [unwired: 2 in, 2 out]
                n1075 = property on="Cycle Threshold:" class="DigNum (strict)"("Visible"=w2528) -> ()  [unwired: 2 in, 2 out]
                n1076 = property on="pb.Stop Profile" class="Bool"("Visible"=w2528) -> ()  [unwired: 2 in, 2 out]
                n1077 = property on="Data File Name:" class="Str"("Visible"=w2528) -> ()  [unwired: 2 in, 2 out]
                n1078 = property on="pb.Run Profile" class="Bool (strict)"("Visible"=w2528) -> ()  [unwired: 2 in, 2 out]
                n1079 = property on="Anomaly Threshold:" class="DigNum (strict)"("Visible"=w2528) -> ()  [unwired: 2 in, 2 out]
              }
            }
          }
          frame Enabled {
          }
        }
        n1080 = Insert Into Array(array=w2488, index=0, new element=w2485) -> (w2487:T14[])
      }
    }
  }
  n1081 = flat-sequence {
    tunnel: w10 -> [_]
    tunnel: w3 -> [w2533]
    frame #0 {
      n1082 = disable-structure shown="Disabled" {
        disable-tunnel: w2533 -> [w2535 _]
        frame Disabled {
          n1083 = call "Data Loop.vi"("FPGA Ref"=w2535) -> ()  [unwired: 10 in, 1 out]
        }
        frame Enabled {
        }
      }
      n1084 = disable-structure shown="Disabled" {
        disable-tunnel: w2533 -> [w2534 _]
        frame Disabled {
          n1085 = call "Power Supply Loop.vi"("FPGA Ref"=w2534) -> ()  [unwired: 11 in]
          n1086 = call "Data Logger Loop.vi"() -> ()  [unwired: 20 in]
          n1087 = call "CAN Loop.vi"() -> ()  [unwired: 12 in]
        }
        frame Enabled {
        }
      }
      n1088 = call "Email Loop.vi"() -> ()  [unwired: 12 in]
      n1089 = disable-structure shown="Disabled" {
        frame Disabled {
          n1090 = call "Watlow Loop.vi"() -> ()  [unwired: 12 in]
        }
        frame Enabled {
        }
      }
      n1091 = call "App Loop.vi"() -> ()  [unwired: 12 in]
      n1092 = disable-structure shown="Disabled" {
        frame Disabled {
          n1093 = call "RPi HMI Loop.vi"() -> ()  [unwired: 20 in]
        }
        frame Enabled {
        }
      }
      n1094 = call "LS Data Loop.vi"("FPGA Ref"=w2533) -> ()  [unwired: 11 in]
    }
  }
  n1095 = while {
    tunnel: w3 -> [w2538]
    stop <- FALSE stop-if-true
    n1096 = local read "Main Tab"() -> (w2536:T9)
    n1097 = case shown="\"Live Graph\"" w2536 {
      tunnel: w2538 -> [_ w2541]
      frame Default {
        n1098 = Wait (ms)(milliseconds to wait=u32 10) -> ()  [unwired: 1 out]
      }
      frame "Live Graph" {
        n1099 = case shown="False" "Pause" {
          tunnel: w2541 -> [w2550 _]
          frame False {
            n1100 = xnode "Read/Write Control"("FPGA VI Reference In"=w2550) -> ("Anomaly Resamples"=w2544:fxp<+/-,28,17>[])  [unwired: 1 in, 2 out]
            n1101 = Decrement(x="Position") -> (x-1=w2547:i32)
            n1102 = In Range and Coerce(upper limit=12, x=w2547, lower limit=0) -> (coerced(x)=w2543:i32)  [unwired: 1 out]
            n1103 = Index Array(array=w2544, index=w2543) -> (element=→"Waveform Chart":fxp<+/-,28,17>)
            n1104 = Wait (ms)(milliseconds to wait=u32 1) -> ()  [unwired: 1 out]
          }
          frame True {
            n1105 = Wait (ms)(milliseconds to wait=u32 10) -> ()  [unwired: 1 out]
          }
        }
      }
    }
  }
